vi "Lab Panel V4.4.vi"() -> ()   [LabVIEW 2013]
uses:
  <vilib>/Platform/TimedLoop/XDataNode/timing_clust.ctl
  <vilib>/Platform/TimedLoop/XDataNode/nitl_modes.ctl
  <vilib>/Platform/TimedLoop/XDataNode/wakeup.ctl
  Global 1.vi
  <vilib>/platform/TimedLoop/XDataNode/XDataNode.xnode
  <vilib>/Platform/TimedLoop/XDataNode/XDNodeRunTimeDep.lvlib
panel:
  in  "ADMIN PAGE":bool
  out "TEMP update":bool
  out "AI update":bool
  in  "Tab Control 2":T1(tab)
  out "SIG LAB05-2":T2 {"PF" format="%.2f"; "AMPS" format="%.1f"}
  out "SIG LAB05-1":T2 {"PF" format="%.2f"; "AMPS" format="%.1f"}
  out "SIG LAB04-2":T2 {"PF" format="%.2f"; "AMPS" format="%.1f"}
  out "SIG LAB04-1":T2 {"PF" format="%.2f"; "AMPS" format="%.1f"}
  out "SIG LAB03-2":T2 {"PF" format="%.2f"; "AMPS" format="%.1f"}
  out "SIG LAB03-1":T2 {"PF" format="%.2f"; "AMPS" format="%.1f"}
  out "SIG LAB02-2":T2 {"PF" format="%.2f"; "AMPS" format="%.1f"}
  in  "RUN LAB01-1":bool
  in  "O/I  LAB05-1":bool
  in  "O/I  LAB05-2":bool
  in  "O/I  LAB04-1":bool
  in  "O/I  LAB04-2":bool
  in  "O/I  LAB02-1":bool
  in  "O/I  LAB02-2":bool
  in  "O/I  LAB01-2":bool
  in  "O/I  LAB01-1":bool
  in  "O/I  LAB03-1":bool
  in  "RUN LAB05-2":bool
  in  "RUN LAB05-1":bool
  in  "RUN LAB04-2":bool
  in  "RUN LAB04-1":bool
  in  "RUN LAB03-2":bool
  in  "RUN LAB03-1":bool
  in  "RUN LAB02-2":bool
  in  "RUN LAB02-1":bool
  in  "RUN LAB01-2":bool
  in  "SELECT LAB05-2":T3(radio)
  in  "SELECT LAB05-1":T3(radio)
  in  "SELECT LAB04-2":T3(radio)
  in  "SELECT LAB04-1":T3(radio)
  in  "SELECT LAB03-2":T3(radio)
  in  "SELECT LAB03-1":T3(radio)
  in  "SELECT LAB02-2":T3(radio)
  in  "SELECT LAB02-1":T3(radio)
  in  "SELECT LAB01-2":T3(radio)
  in  "SELECT LAB01-1":T3(radio)
  in  "O/I  LAB03-2":bool
  out "SIG LAB01-1":T2 {"PF" format="%.2f"; "AMPS" format="%.1f"}
  out "SIG LAB01-2":T2 {"PF" format="%.2f"; "AMPS" format="%.1f"}
  out "SIG LAB02-1":T2 {"PF" format="%.2f"; "AMPS" format="%.1f"}
  out "DISP LAB05-2":T4 {"MINS" format="%.2g"}
  out "DISP LAB05-1":T4 {"MINS" format="%.2g"}
  out "DISP LAB04-2":T4 {"MINS" format="%.2g"}
  out "DISP LAB04-1":T4 {"MINS" format="%.2g"}
  out "DISP LAB03-2":T4 {"MINS" format="%.2g"}
  out "DISP LAB03-1":T4 {"MINS" format="%.2g"}
  in  "SET LAB05-2":T5={"NAME"="", "DESCRIPTION"="", "CYCLES"=5.0, "T-RISE mins"=0.0, "T-RISE deg C"=0.0} {"CYCLES" min=5.0 step=1.0}
  in  "SET LAB05-1":T5={"NAME"="", "DESCRIPTION"="", "CYCLES"=5.0, "T-RISE mins"=0.0, "T-RISE deg C"=0.0} {"CYCLES" min=5.0 step=1.0}
  in  "SET LAB04-2":T5={"NAME"="", "DESCRIPTION"="", "CYCLES"=5.0, "T-RISE mins"=0.0, "T-RISE deg C"=0.0} {"CYCLES" min=5.0 step=1.0}
  in  "SET LAB04-1":T5={"NAME"="", "DESCRIPTION"="", "CYCLES"=5.0, "T-RISE mins"=0.0, "T-RISE deg C"=0.0} {"CYCLES" min=5.0 step=1.0}
  in  "SET LAB03-2":T5={"NAME"="", "DESCRIPTION"="", "CYCLES"=5.0, "T-RISE mins"=0.0, "T-RISE deg C"=0.0} {"CYCLES" min=5.0 step=1.0}
  in  "SET LAB03-1":T5={"NAME"="", "DESCRIPTION"="", "CYCLES"=5.0, "T-RISE mins"=0.0, "T-RISE deg C"=0.0} {"CYCLES" min=5.0 step=1.0}
  out "DISP LAB02-2":T4 {"MINS" format="%.2g"}
  out "DISP LAB02-1":T4 {"MINS" format="%.2g"}
  in  "SET LAB02-2":T5={"NAME"="", "DESCRIPTION"="", "CYCLES"=5.0, "T-RISE mins"=0.0, "T-RISE deg C"=0.0} {"CYCLES" min=5.0 step=1.0}
  in  "SET LAB02-1":T5={"NAME"="", "DESCRIPTION"="", "CYCLES"=5.0, "T-RISE mins"=0.0, "T-RISE deg C"=0.0} {"CYCLES" min=5.0 step=1.0}
  out "RESULT LAB05-2":bool
  out "RESULT LAB05-1":bool
  out "RESULT LAB04-2":bool
  out "RESULT LAB04-1":bool
  out "RESULT LAB03-2":bool
  out "RESULT LAB03-1":bool
  out "RESULT LAB02-2":bool
  out "RESULT LAB02-1":bool
  out "RESULT LAB01-2":bool
  out "RESULT LAB01-1":bool
  in  "SET LAB01-1":T5={"NAME"="", "DESCRIPTION"="", "CYCLES"=5.0, "T-RISE mins"=0.0, "T-RISE deg C"=0.0} {"CYCLES" min=5.0 step=1.0}
  in  "SET LAB01-2":T5={"NAME"="", "DESCRIPTION"="", "CYCLES"=5.0, "T-RISE mins"=0.0, "T-RISE deg C"=0.0} {"CYCLES" min=5.0 step=1.0}
  out "DISP LAB01-1":T4 {"MINS" format="%.2g"}
  out "DISP LAB01-2":T4 {"MINS" format="%.2f"}
  out "TEMP RISE LAB05-2":cluster{"TL":dbl, "TN":dbl}
  out "TEMP RISE LAB05-1":cluster{"TL":dbl, "TN":dbl}
  out "TEMP RISE LAB04-2":cluster{"TL":dbl, "TN":dbl}
  out "TEMP RISE LAB04-1":cluster{"TL":dbl, "TN":dbl}
  out "TEMP RISE LAB03-2":cluster{"TL":dbl, "TN":dbl}
  out "TEMP RISE LAB03-1":cluster{"TL":dbl, "TN":dbl}
  out "TEMP RISE LAB02-2":cluster{"TL":dbl, "TN":dbl}
  out "TEMP RISE LAB02-1":cluster{"TL":dbl, "TN":dbl}
  out "TEMP RISE LAB01-2":cluster{"TL":dbl, "TN":dbl}
  out "TEMP RISE LAB01-1":cluster{"TL":dbl, "TN":dbl}
  in  "JIG OFF TIME (S)":dbl=2.0 min=2.0 max=10.0 step=0.5 format="%.1g"
  in  "JIG ON TIME (S)":dbl=1.0 min=1.0 max=10.0 step=0.5 format="%.1g"
  out "JIG LAB05-2":bool
  out "JIG LAB05-1":bool
  out "JIG LAB04-2":bool
  out "JIG LAB04-1":bool
  out "JIG LAB03-2":bool
  out "JIG LAB03-1":bool
  out "JIG LAB02-2":bool
  out "JIG LAB02-1":bool
  out "JIG LAB01-2":bool
  out "JIG LAB01-1":bool
  out "TEMP START LAB01-1":cluster{"TL":dbl, "TN":dbl}
  out "TEMP START LAB02-1":cluster{"TL":dbl, "TN":dbl}
  out "TEMP START LAB03-1":cluster{"TL":dbl, "TN":dbl}
  out "TEMP START LAB04-1":cluster{"TL":dbl, "TN":dbl}
  out "TEMP START LAB01-2":cluster{"TL":dbl, "TN":dbl}
  out "TEMP START LAB02-2":cluster{"TL":dbl, "TN":dbl}
  out "TEMP START LAB03-2":cluster{"TL":dbl, "TN":dbl}
  out "TEMP START LAB04-2":cluster{"TL":dbl, "TN":dbl}
  out "TEMP START LAB05-2":cluster{"TL":dbl, "TN":dbl}
  out "TEMP START LAB05-1":cluster{"TL":dbl, "TN":dbl}
  in  "MAIL SETTINGS":T6
  out "MAIL REPORT":string
  in  "TO (string):":string
  in  "Send Mail Now":bool
  in  "Auto Mail Send":bool
  in  "Network Directory":path
  out "CAL LAB01":T7 {"2 (TN) cal" min=0.0 step=0.01 format="%.2f"; "2 (TL) cal" min=0.0 step=0.01 format="%.2f"; "2 (PF) cal" min=0.0 step=0.01 format="%.2f"; "2 (V) cal" min=0.0 step=0.01 format="%.2f"; "2 (A) cal" min=0.0 step=0.01 format="%.2f"; "1 (TN) cal" min=0.0 step=0.01 format="%.2f"; "1 (TL) cal" min=0.0 step=0.01 format="%.2f"; "1 (PF) cal" min=0.0 step=0.01 format="%.2f"; "1 (V) cal" min=0.0 step=0.01 format="%.2f"; "1  (A) cal" min=0.0 step=0.01 format="%.2f"}
  out "CAL LAB03":T7 {"2 (TN) cal" min=0.0 step=0.01 format="%.2f"; "2 (TL) cal" min=0.0 step=0.01 format="%.2f"; "2 (PF) cal" min=0.0 step=0.01 format="%.2f"; "2 (V) cal" min=0.0 step=0.01 format="%.2f"; "2 (A) cal" min=0.0 step=0.01 format="%.2f"; "1 (TN) cal" min=0.0 step=0.01 format="%.2f"; "1 (TL) cal" min=0.0 step=0.01 format="%.2f"; "1 (PF) cal" min=0.0 step=0.01 format="%.2f"; "1 (V) cal" min=0.0 step=0.01 format="%.2f"; "1  (A) cal" min=0.0 step=0.01 format="%.2f"}
  out "CAL LAB02":T8 {"2 (TN) cal" min=0.0 step=0.01 format="%.2f"; "2 (TL) cal" min=0.0 step=0.01 format="%.2f"; "2 (PF) cal" min=0.0 step=0.01 format="%.2f"; "2 (V) cal" min=0.0 step=0.01 format="%.2f"; "2 (A) cal" min=0.0 step=0.01 format="%.2f"; "1 (TN) cal" min=0.0 step=0.01 format="%.2f"; "1 (TL) cal" min=0.0 step=0.01 format="%.2f"; "1 (PF) cal" min=0.0 step=0.01 format="%.2f"; "1 (V) cal" min=0.0 step=0.01 format="%.2f"; "1 (A) cal" min=0.0 step=0.01 format="%.2f"}
  out "CAL LAB05":T7 {"2 (TN) cal" min=0.0 step=0.01 format="%.2f"; "2 (TL) cal" min=0.0 step=0.01 format="%.2f"; "2 (PF) cal" min=0.0 step=0.01 format="%.2f"; "2 (V) cal" min=0.0 step=0.01 format="%.2f"; "2 (A) cal" min=0.0 step=0.01 format="%.2f"; "1 (TN) cal" min=0.0 step=0.01 format="%.2f"; "1 (TL) cal" min=0.0 step=0.01 format="%.2f"; "1 (PF) cal" min=0.0 step=0.01 format="%.2f"; "1 (V) cal" min=0.0 step=0.01 format="%.2f"; "1  (A) cal" min=0.0 step=0.01 format="%.2f"}
  out "CAL LAB04":T7 {"2 (TN) cal" min=0.0 step=0.01 format="%.2f"; "2 (TL) cal" min=0.0 step=0.01 format="%.2f"; "2 (PF) cal" min=0.0 step=0.01 format="%.2f"; "2 (V) cal" min=0.0 step=0.01 format="%.2f"; "2 (A) cal" min=0.0 step=0.01 format="%.2f"; "1 (TN) cal" min=0.0 step=0.01 format="%.2f"; "1 (TL) cal" min=0.0 step=0.01 format="%.2f"; "1 (PF) cal" min=0.0 step=0.01 format="%.2f"; "1 (V) cal" min=0.0 step=0.01 format="%.2f"; "1  (A) cal" min=0.0 step=0.01 format="%.2f"}
  out "calibration file error out":errorcluster
  in  "CALIBRATE":bool
  out "ON L05-2":cluster{"amps":dbl, "volts":dbl, "pf":dbl}
  out "ON L05-1":cluster{"amps":dbl, "volts":dbl, "pf":dbl}
  out "FAIL LAB05-2":cluster{"LO":dbl, "HI":dbl}
  out "FAIL LAB05-1":cluster{"LO":dbl, "HI":dbl}
  out "FAIL LAB04-2":cluster{"LO":dbl, "HI":dbl}
  out "FAIL LAB04-1":cluster{"LO":dbl, "HI":dbl}
  out "FAIL LAB03-2":cluster{"LO":dbl, "HI":dbl}
  out "FAIL LAB03-1":cluster{"LO":dbl, "HI":dbl}
  out "FAIL LAB02-2":cluster{"LO":dbl, "HI":dbl}
  out "FAIL LAB02-1":cluster{"LO":dbl, "HI":dbl}
  out "FAIL LAB01-2":cluster{"LO":dbl, "HI":dbl}
  out "FAIL LAB01-1":cluster{"LO":dbl, "HI":dbl}
  out "ON L01-1":cluster{"amps":dbl, "volts":dbl, "pf":dbl}
  out "ON L01-2":cluster{"amps":dbl, "volts":dbl, "pf":dbl}
  out "ON L02-1":cluster{"amps":dbl, "volts":dbl, "pf":dbl}
  out "ON L02-2":cluster{"amps":dbl, "volts":dbl, "pf":dbl}
  out "ON L03-1":cluster{"amps":dbl, "volts":dbl, "pf":dbl}
  out "ON L03-2":cluster{"amps":dbl, "volts":dbl, "pf":dbl}
  out "ON L04-1":cluster{"amps":dbl, "volts":dbl, "pf":dbl}
  out "ON L04-2":cluster{"amps":dbl, "volts":dbl, "pf":dbl}
  out "TEST VOLTS CHART":T9(graph)
  in  "Select  Cycle":enum32{"ON CYCLE", "OFF CYCLE"}(radio)
  out "TEST AMPS CHART":T9(graph)
  in  "JIG TEST":T10
  in  "C drive data root dir":path
  out "run lab05-2":bool
  out "run lab05-1":bool
  out "run lab04-2":bool
  out "run lab04-1":bool
  out "run lab03-2":bool
  out "run lab03-1":bool
  out "run lab02-2":bool
  out "run lab02-1":bool
  out "run lab01-2":bool
  out "run lab01-1":bool
  out "stop2":bool
  in  "Tab Control":T11(tab)
  out "LAB01-2 (GRAPH)":dynamicdata(graph)
  out "LAB01-1 (GRAPH)":dynamicdata(graph)
  out "LAB02-2 (GRAPH)":dynamicdata(graph)
  out "LAB02-1 (GRAPH)":dynamicdata(graph)
  out "LAB03-2 (GRAPH)":dynamicdata(graph)
  out "LAB03-1 (GRAPH)":dynamicdata(graph)
  out "LAB04-2 (GRAPH)":dynamicdata(graph)
  out "LAB04-1 (GRAPH)":dynamicdata(graph)
  out "LAB05-2 (GRAPH)":dynamicdata(graph)
  out "LAB05-1 (GRAPH)":dynamicdata(graph)
  out "LAB05 TEMP":T12
  out "LAB04 TEMP":T12
  out "LAB02 TEMP":T12
  out "LAB01 TEMP":T12
  out "LAB03 TEMP":T12
  out "Analog Error Array":errorcluster[](array[cluster])
  out "AI loop time":dbl format="%.6g"
  out "loops":dbl
  in  "loop  delay(mS)":dbl
  out "on loops":dbl
  out "off loops":dbl
  out "jig cycle":dbl
  out "TDMS LAB01-1":refnum<k34>
  out "data file error":errorcluster
  out "TDMS LAB02-1":refnum<k34>
  out "TDMS LAB01-2":refnum<k34>
  out "TDMS LAB02-2":refnum<k34>
  out "TDMS LAB03-1":refnum<k34>
  out "TDMS LAB03-2":refnum<k34>
  out "TDMS LAB04-1":refnum<k34>
  out "TDMS LAB04-2":refnum<k34>
  out "TDMS LAB05-1":refnum<k34>
  out "TDMS LAB05-2":refnum<k34>
  out "mail control":string
  out "File Time Stamp":timestamp
  in  "stop":bool
  # "LAB01"
  # "LAB02"
  # "LAB05"
  # "LAB03"
  # "LAB04"
  # "LAB01"
  # "LAB02"
  # "LAB03"
  # "LAB04"
  # "LAB05"
  # "JIG SET"
  # "(Enter recipients address seperated by comma)"
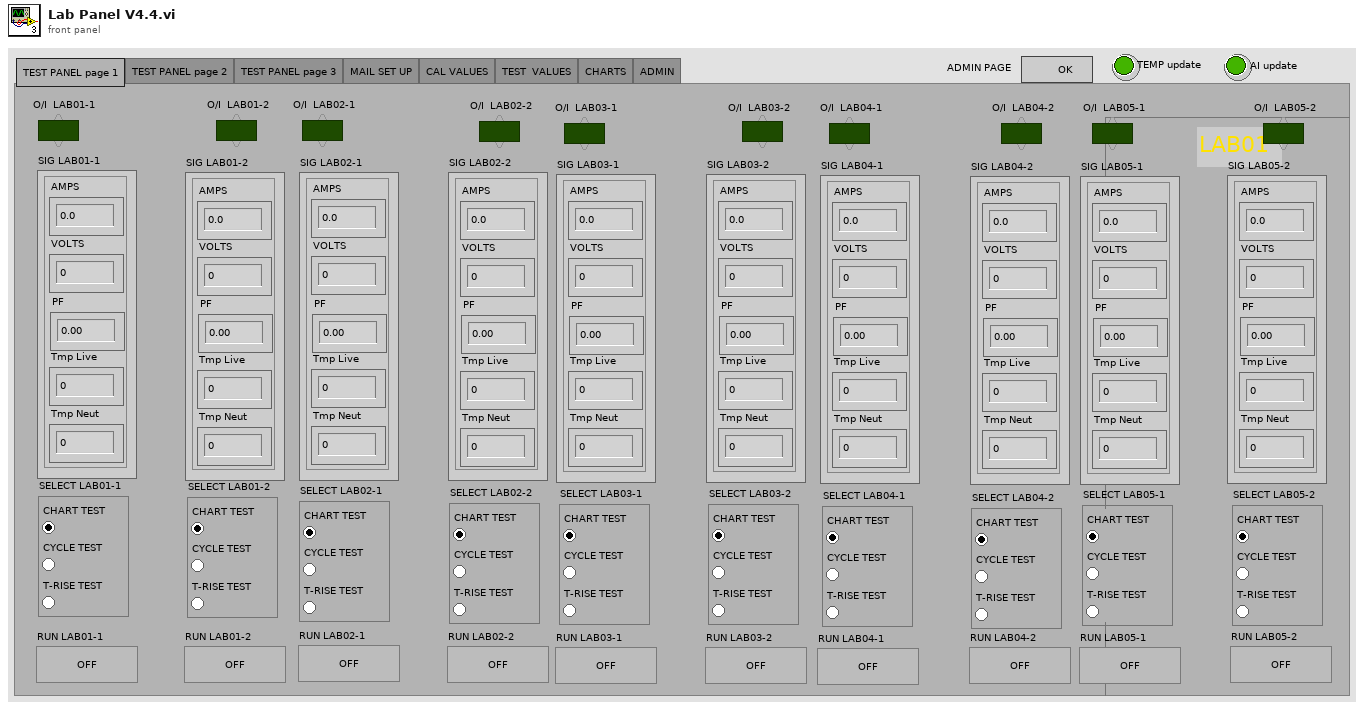
[diagram p1: front panel]
types:
  T1 = enum32{"TEST PANEL page 1", "TEST PANEL page 2", "TEST PANEL page 3", "MAIL SET UP", "CAL VALUES", "TEST  VALUES", "CHARTS", "ADMIN"}
  T2 = cluster{"AMPS":dbl, "VOLTS":dbl, "PF":dbl, "Tmp Live":dbl, "Tmp Neut":dbl}
  T3 = enum32{"CHART TEST", "CYCLE TEST", "T-RISE TEST"}
  T4 = cluster{"CYCLE":dbl, "MINS":dbl, "STATUS":string}
  T5 = cluster{"NAME":string, "DESCRIPTION":string, "CYCLES":dbl, "T-RISE mins":dbl, "T-RISE deg C":dbl}
  T6 = cluster{"OUT SERVER ADDRESS":string, "FROM ACCOUNT":string, "USER NAME":string, "PASSWORD":string, "TEST MAIL":bool, "TEST MAIL STATUS":string, "mail error":errorcluster}
  T7 = cluster{"1  (A) cal":dbl, "1 (V) cal":dbl, "1 (PF) cal":dbl, "1 (TL) cal":dbl, "1 (TN) cal":dbl, "2 (A) cal":dbl, "2 (V) cal":dbl, "2 (PF) cal":dbl, "2 (TL) cal":dbl, "2 (TN) cal":dbl}
  T8 = cluster{"1 (A) cal":dbl, "1 (V) cal":dbl, "1 (PF) cal":dbl, "1 (TL) cal":dbl, "1 (TN) cal":dbl, "2 (A) cal":dbl, "2 (V) cal":dbl, "2 (PF) cal":dbl, "2 (TL) cal":dbl, "2 (TN) cal":dbl}
  T9 = cluster{"AMPS":dbl, "AMPS":dbl, "AMPS":dbl, "AMPS":dbl, "AMPS":dbl, "AMPS":dbl, "AMPS":dbl, "AMPS":dbl, "AMPS":dbl, "AMPS":dbl}
  T10 = cluster{" LAB01-1":bool, " LAB01-2":bool, "LAB02-1":bool, " LAB02-2":bool, "LAB03-1":bool, "LAB03-2":bool, "LAB04-1":bool, "LAB04-2":bool, "LAB05-1":bool, "LAB05-2":bool}
  T11 = enum32{"LAB01", "LAB02", "LAB03", "LAB04", "LAB05", "TEMPERATURE", "ERROR"}
  T12 = cluster{"T1 Live":dbl, "T1 Neut":dbl, "T2 Live":dbl, "T2 Neut":dbl, "ID":dbl, "ER":dbl}
  T13 = enum8{"Enabled", "Disabled", "Disabled and Grayed Out"}
  T14 = typedef "XDNodeRunTimeDep.lvlib/timing_clust.ctl" = cluster{"Expected End [f-1]":u64, "Actual End [f-1]":u64, "Finished Late? [f-1]":bool, "Expected End [i-1]":u64, "Actual End [i-1]":u64, "Finished Late? [i-1]":bool, "Expected Start [i]":u64, "Actual Start [i]":u64, "Expected Start [f]":u64, "Actual Start [f]":u64, "Source Name":string, "Structure Name":string, "Period":i64, "Deadline":i64, "Offset":i64, "Start":i64, "Priority":i32, "Timeout":i32, "Mode":T15, "Wakeup Reason":T16, "Error":errorcluster, "Source Type":string, "Secondary Source Type":string, "Global End Time":u64, "Global Start Time":u64, "Frame Duration":u64, "Iteration Duration":u64, "Assigned CPU":i32, "I/O Scan Engine Mode":u32}
  T15 = typedef "XDNodeRunTimeDep.lvlib/nitl_modes.ctl" = enum32{"No Change", "Process missed periods, maintain original phase", "Discard missed periods, maintain original phase", "Process missed periods, ignore original phase", "Discard missed periods, ignore original phase"}
  T16 = typedef "XDNodeRunTimeDep.lvlib/wakeup.ctl" = enum32{"Normal", "Aborted", "Asynchronous wakeup", "Timing source error", "Timed loop error", "Timeout"}
  T17 = enum16{"open", "open or create", "create or replace", "create", "open (read-only)"}
  T18 = enum16{"open", "replace", "create", "open or create", "replace or create", "replace or create with confirmation"}
  T19 = cluster{"SET LAB01-1":cluster{"NAME":string, "DESCRIPTION":string, "CYCLES":dbl, "T-RISE mins":dbl, "T-RISE deg C":dbl}, "SET LAB01-2":cluster{"NAME":string, "DESCRIPTION":string, "CYCLES":dbl, "T-RISE mins":dbl, "T-RISE deg C":dbl}, "SET LAB02-1":cluster{"NAME":string, "DESCRIPTION":string, "CYCLES":dbl, "T-RISE mins":dbl, "T-RISE deg C":dbl}, "SET LAB02-2":cluster{"NAME":string, "DESCRIPTION":string, "CYCLES":dbl, "T-RISE mins":dbl, "T-RISE deg C":dbl}, "SET LAB03-1":cluster{"NAME":string, "DESCRIPTION":string, "CYCLES":dbl, "T-RISE mins":dbl, "T-RISE deg C":dbl}, "SET LAB03-2":cluster{"NAME":string, "DESCRIPTION":string, "CYCLES":dbl, "T-RISE mins":dbl, "T-RISE deg C":dbl}, "SET LAB04-1":cluster{"NAME":string, "DESCRIPTION":string, "CYCLES":dbl, "T-RISE mins":dbl, "T-RISE deg C":dbl}, "SET LAB04-2":cluster{"NAME":string, "DESCRIPTION":string, "CYCLES":dbl, "T-RISE mins":dbl, "T-RISE deg C":dbl}, "SET LAB05-1":cluster{"NAME":string, "DESCRIPTION":string, "CYCLES":dbl, "T-RISE mins":dbl, "T-RISE deg C":dbl}, "SET LAB05-2":cluster{"NAME":string, "DESCRIPTION":string, "CYCLES":dbl, "T-RISE mins":dbl, "T-RISE deg C":dbl}, "Network Directory":path, "C drive data root dir":path}
  T20 = cluster{"MAIL SETTINGS":cluster{"OUT SERVER ADDRESS":string, "FROM ACCOUNT":string, "USER NAME":string, "PASSWORD":string, "TEST MAIL":bool, "TEST MAIL STATUS":string, "mail error":errorcluster}, "Auto Mail Send":bool, string}
  T21 = cluster{"T1":dbl, "T2":dbl, "T3":dbl, "T4":dbl, "ID":dbl, "ER":dbl}
  T22 = cluster{"LAB01-1 (A)":dbl, "LAB01-1 (V)":dbl, "LAB01-1 (PF)":dbl, "LAB01-2 (A)":dbl, "LAB01-2 (V)":dbl, "LAB01-2 (PF)":dbl}
  T23 = cluster{"LAB02-1 (A)":dbl, "LAB02-1 (V)":dbl, "LAB02-1 (PF)":dbl, "LAB02-2 (A)":dbl, "LAB02-2 (V)":dbl, "LAB02-2 (PF)":dbl}
  T24 = cluster{"LAB03-1 (A)":dbl, "LAB03-1 (V)":dbl, "LAB03-1 (PF)":dbl, "LAB03-2 (A)":dbl, "LAB03-2 (V)":dbl, "LAB03-2 (PF)":dbl}
  T25 = cluster{"LAB04-1 (A)":dbl, "LAB04-1 (V)":dbl, "LAB04-1 (PF)":dbl, "LAB04-2 (A)":dbl, "LAB04-2 (V)":dbl, "LAB04-2 (PF)":dbl}
  T26 = cluster{"LAB05-1 (A)":dbl, "LAB05-1 (V)":dbl, "LAB05-1 (PF)":dbl, "LAB05-2 (A)":dbl, "LAB05-2 (V)":dbl, "LAB05-2 (PF)":dbl}
  T27 = cluster{"VOLTS":dbl, "VOLTS":dbl, "VOLTS":dbl, "VOLTS":dbl, "VOLTS":dbl, "VOLTS":dbl, "VOLTS":dbl, "VOLTS":dbl, "VOLTS":dbl, "VOLTS":dbl}
  T28 = cluster{"FAIL LAB01-1":cluster{"LO":dbl, "HI":dbl}, "SIG LAB01-1":cluster{"AMPS":dbl, "VOLTS":dbl, "PF":dbl, "Tmp Live":dbl, "Tmp Neut":dbl}, "TEMP START LAB01-1":cluster{"TL":dbl, "TN":dbl}, "DISP LAB01-1":cluster{"CYCLE":dbl, "MINS":dbl, "STATUS":string}, "SET LAB01-1":cluster{"NAME":string, "DESCRIPTION":string, "CYCLES":dbl, "T-RISE mins":dbl, "T-RISE deg C":dbl}, "TDMS LAB01-1":refnum<k34>}
  T29 = cluster{"FAIL LAB01-2":cluster{"LO":dbl, "HI":dbl}, "SIG LAB01-2":cluster{"AMPS":dbl, "VOLTS":dbl, "PF":dbl, "Tmp Live":dbl, "Tmp Neut":dbl}, "TEMP START LAB01-2":cluster{"TL":dbl, "TN":dbl}, "DISP LAB01-2":cluster{"CYCLE":dbl, "MINS":dbl, "STATUS":string}, "SET LAB01-2":cluster{"NAME":string, "DESCRIPTION":string, "CYCLES":dbl, "T-RISE mins":dbl, "T-RISE deg C":dbl}, "TDMS LAB01-2":refnum<k34>}
  T30 = cluster{"FAIL LAB02-1":cluster{"LO":dbl, "HI":dbl}, "SIG LAB02-1":cluster{"AMPS":dbl, "VOLTS":dbl, "PF":dbl, "Tmp Live":dbl, "Tmp Neut":dbl}, "TEMP START LAB02-1":cluster{"TL":dbl, "TN":dbl}, "DISP LAB02-1":cluster{"CYCLE":dbl, "MINS":dbl, "STATUS":string}, "SET LAB02-1":cluster{"NAME":string, "DESCRIPTION":string, "CYCLES":dbl, "T-RISE mins":dbl, "T-RISE deg C":dbl}, "TDMS LAB02-1":refnum<k34>}
  T31 = cluster{"FAIL LAB02-2":cluster{"LO":dbl, "HI":dbl}, "SIG LAB02-2":cluster{"AMPS":dbl, "VOLTS":dbl, "PF":dbl, "Tmp Live":dbl, "Tmp Neut":dbl}, "TEMP START LAB02-2":cluster{"TL":dbl, "TN":dbl}, "DISP LAB02-2":cluster{"CYCLE":dbl, "MINS":dbl, "STATUS":string}, "SET LAB02-2":cluster{"NAME":string, "DESCRIPTION":string, "CYCLES":dbl, "T-RISE mins":dbl, "T-RISE deg C":dbl}, "TDMS LAB02-2":refnum<k34>}
  T32 = cluster{"FAIL LAB03-1":cluster{"LO":dbl, "HI":dbl}, "SIG LAB03-1":cluster{"AMPS":dbl, "VOLTS":dbl, "PF":dbl, "Tmp Live":dbl, "Tmp Neut":dbl}, "TEMP START LAB03-1":cluster{"TL":dbl, "TN":dbl}, "DISP LAB03-1":cluster{"CYCLE":dbl, "MINS":dbl, "STATUS":string}, "SET LAB03-1":cluster{"NAME":string, "DESCRIPTION":string, "CYCLES":dbl, "T-RISE mins":dbl, "T-RISE deg C":dbl}, "TDMS LAB03-1":refnum<k34>}
  T33 = cluster{"FAIL LAB03-2":cluster{"LO":dbl, "HI":dbl}, "SIG LAB03-2":cluster{"AMPS":dbl, "VOLTS":dbl, "PF":dbl, "Tmp Live":dbl, "Tmp Neut":dbl}, "TEMP START LAB03-2":cluster{"TL":dbl, "TN":dbl}, "DISP LAB03-2":cluster{"CYCLE":dbl, "MINS":dbl, "STATUS":string}, "SET LAB03-2":cluster{"NAME":string, "DESCRIPTION":string, "CYCLES":dbl, "T-RISE mins":dbl, "T-RISE deg C":dbl}, "TDMS LAB03-2":refnum<k34>}
  T34 = cluster{"FAIL LAB04-1":cluster{"LO":dbl, "HI":dbl}, "SIG LAB04-1":cluster{"AMPS":dbl, "VOLTS":dbl, "PF":dbl, "Tmp Live":dbl, "Tmp Neut":dbl}, "TEMP START LAB04-1":cluster{"TL":dbl, "TN":dbl}, "DISP LAB04-1":cluster{"CYCLE":dbl, "MINS":dbl, "STATUS":string}, "SET LAB04-1":cluster{"NAME":string, "DESCRIPTION":string, "CYCLES":dbl, "T-RISE mins":dbl, "T-RISE deg C":dbl}, "TDMS LAB04-1":refnum<k34>}
  T35 = cluster{"FAIL LAB04-2":cluster{"LO":dbl, "HI":dbl}, "SIG LAB04-2":cluster{"AMPS":dbl, "VOLTS":dbl, "PF":dbl, "Tmp Live":dbl, "Tmp Neut":dbl}, "TEMP START LAB04-2":cluster{"TL":dbl, "TN":dbl}, "DISP LAB04-2":cluster{"CYCLE":dbl, "MINS":dbl, "STATUS":string}, "SET LAB04-2":cluster{"NAME":string, "DESCRIPTION":string, "CYCLES":dbl, "T-RISE mins":dbl, "T-RISE deg C":dbl}, "TDMS LAB04-2":refnum<k34>}
  T36 = cluster{"FAIL LAB05-1":cluster{"LO":dbl, "HI":dbl}, "SIG LAB05-1":cluster{"AMPS":dbl, "VOLTS":dbl, "PF":dbl, "Tmp Live":dbl, "Tmp Neut":dbl}, "TEMP START LAB05-1":cluster{"TL":dbl, "TN":dbl}, "DISP LAB05-1":cluster{"CYCLE":dbl, "MINS":dbl, "STATUS":string}, "SET LAB05-1":cluster{"NAME":string, "DESCRIPTION":string, "CYCLES":dbl, "T-RISE mins":dbl, "T-RISE deg C":dbl}, "TDMS LAB05-1":refnum<k34>}
  T37 = cluster{"FAIL LAB05-2":cluster{"LO":dbl, "HI":dbl}, "SIG LAB05-2":cluster{"AMPS":dbl, "VOLTS":dbl, "PF":dbl, "Tmp Live":dbl, "Tmp Neut":dbl}, "TEMP START LAB05-2":cluster{"TL":dbl, "TN":dbl}, "DISP LAB05-2":cluster{"CYCLE":dbl, "MINS":dbl, "STATUS":string}, "SET LAB05-2":cluster{"NAME":string, "DESCRIPTION":string, "CYCLES":dbl, "T-RISE mins":dbl, "T-RISE deg C":dbl}, "TDMS LAB05-2":refnum<k34>}
  T38 = cluster{"MAIL SETTINGS":cluster{"OUT SERVER ADDRESS":string, "FROM ACCOUNT":string, "USER NAME":string, "PASSWORD":string, "TEST MAIL":bool, "TEST MAIL STATUS":string, "mail error":errorcluster}, "Auto Mail Send":bool, "TO (string):":string}
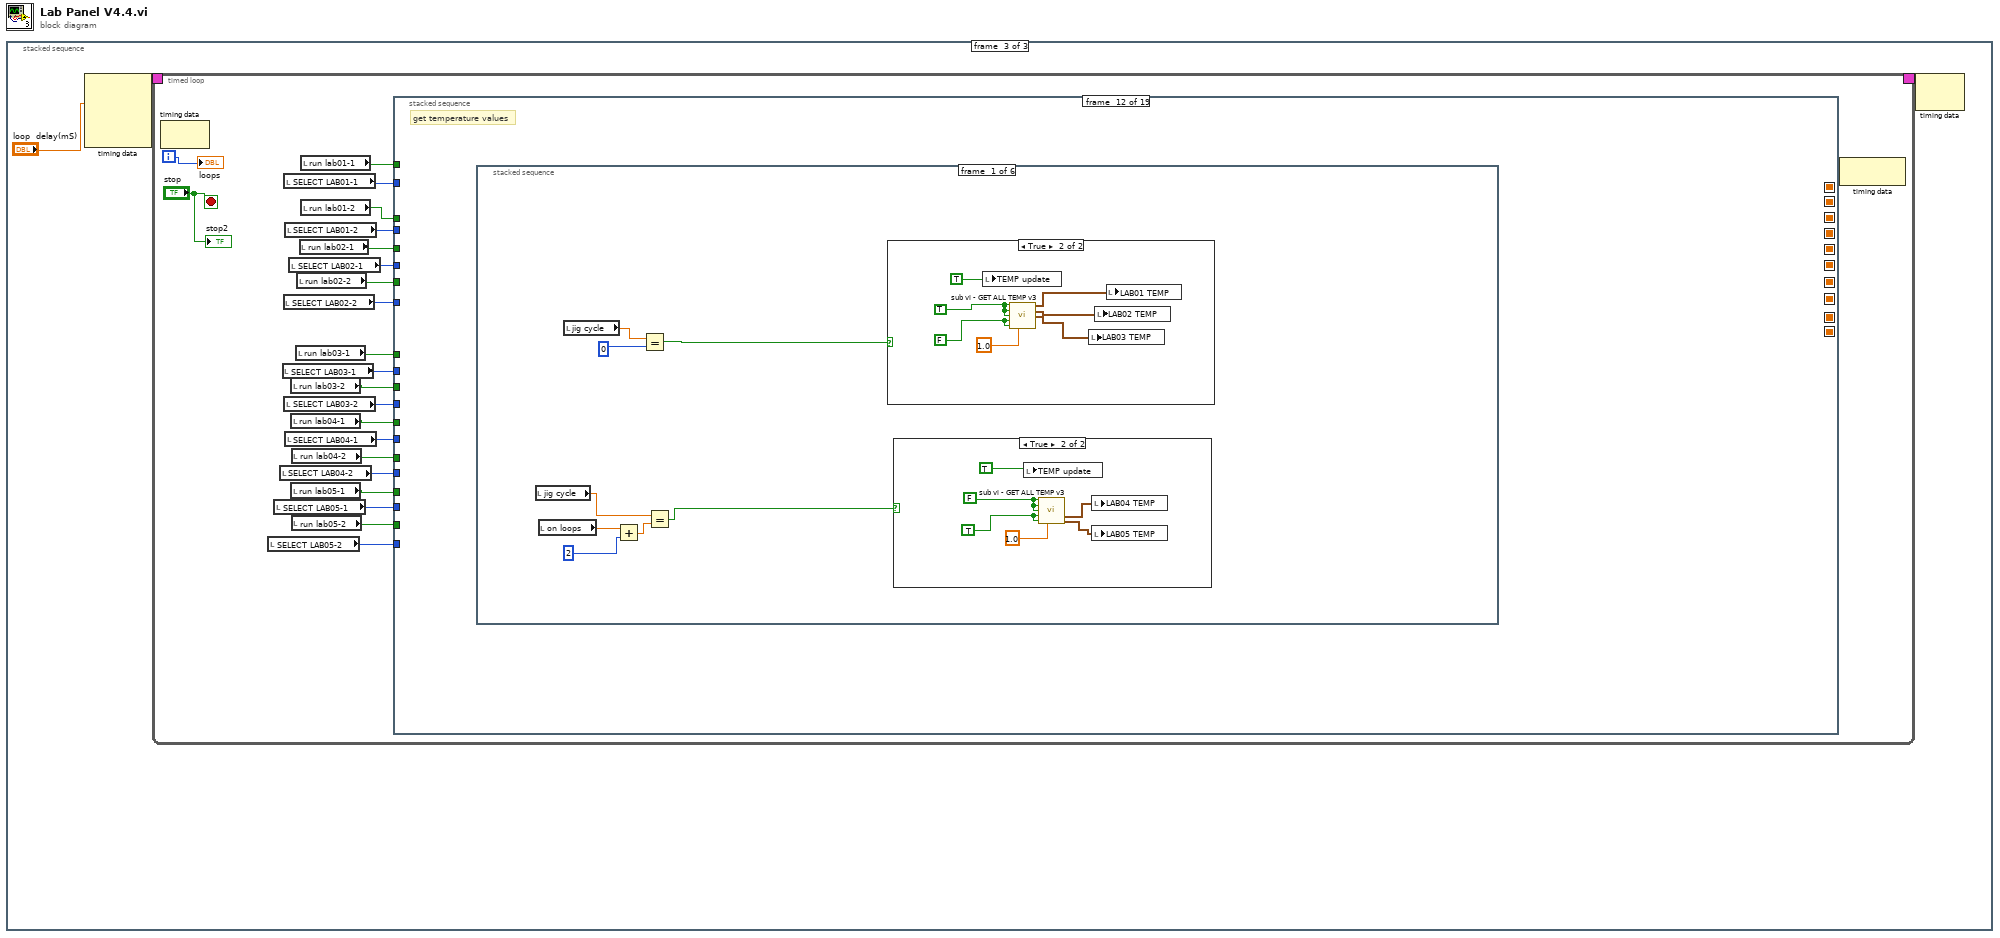
[diagram p0: block diagram]
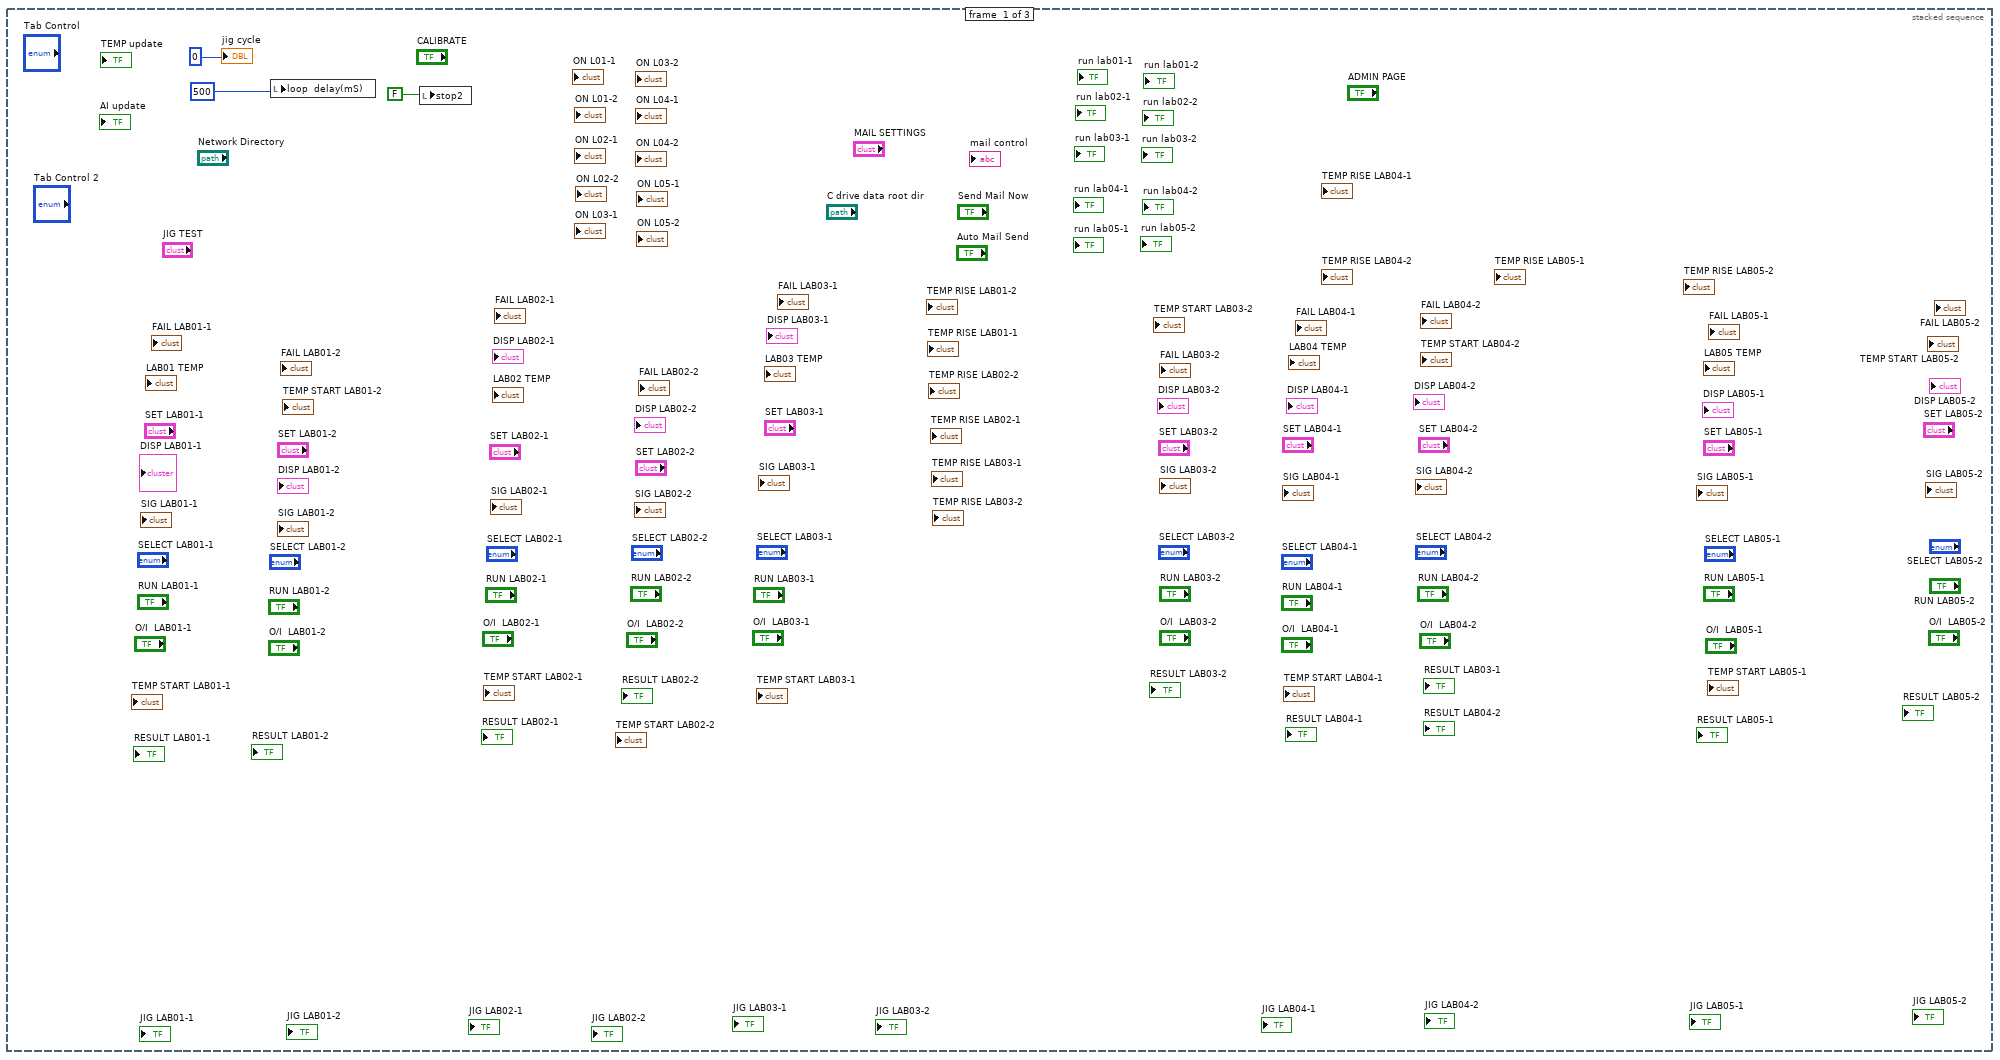
[diagram p2: hidden frame]
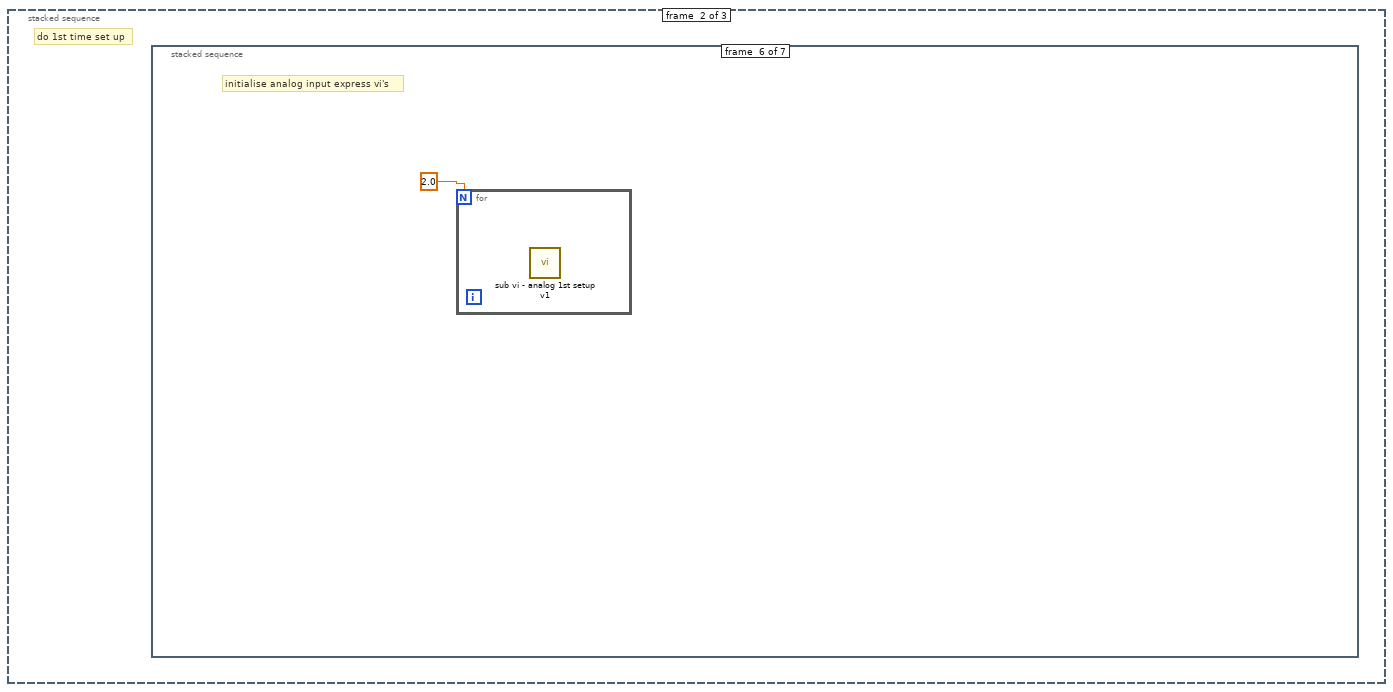
[diagram p3: hidden frame]
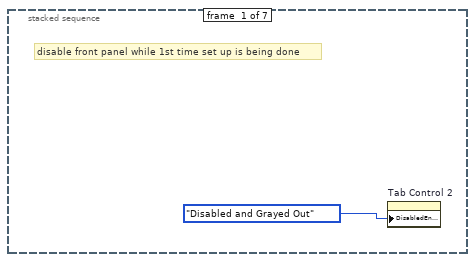
[diagram p4: hidden frame]
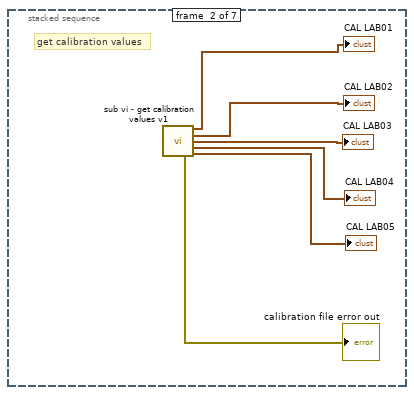
[diagram p5: hidden frame]
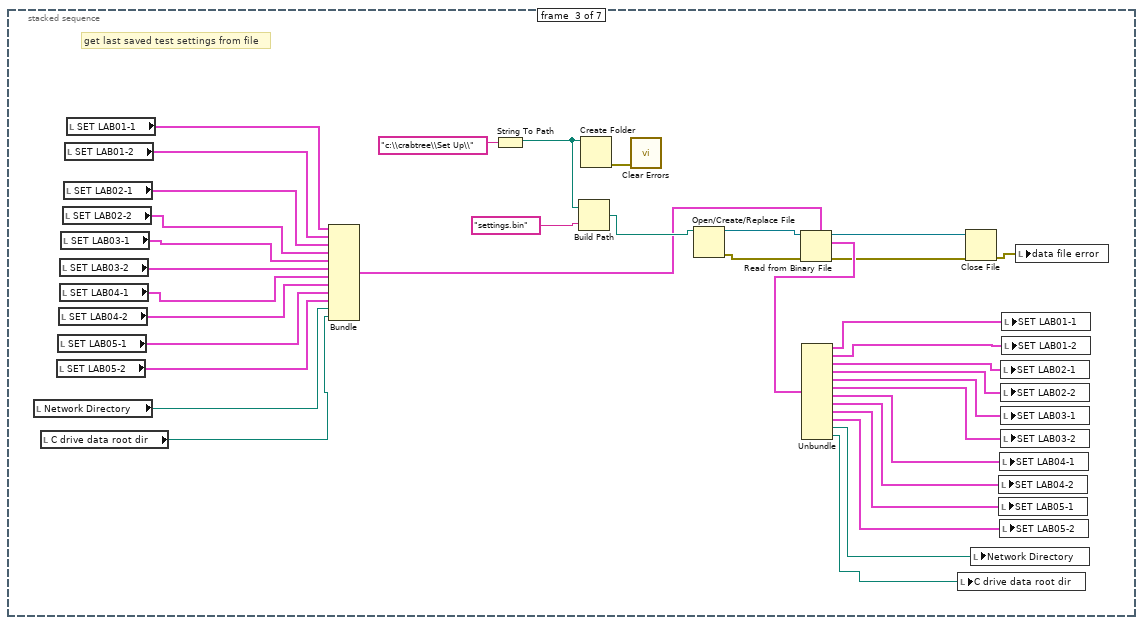
[diagram p6: hidden frame]
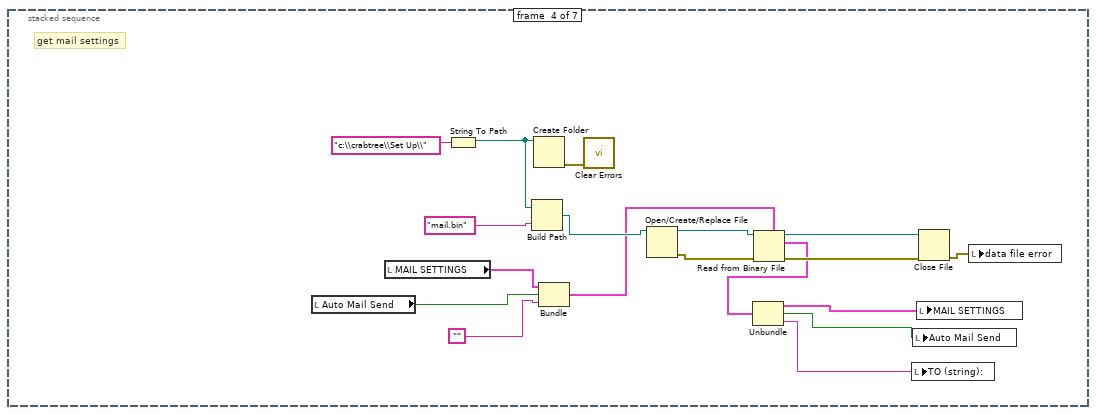
[diagram p7: hidden frame]
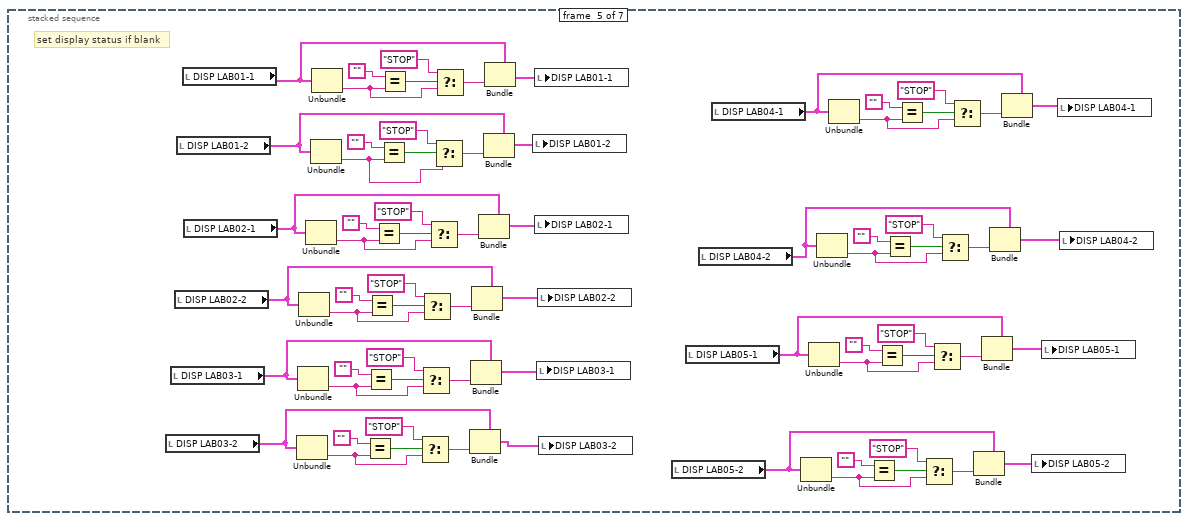
[diagram p8: hidden frame]
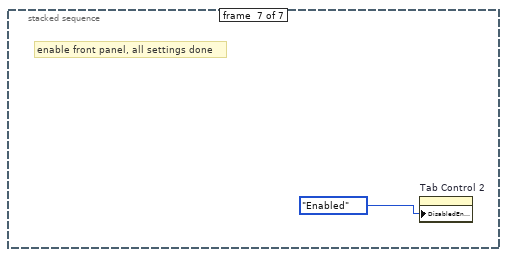
[diagram p9: hidden frame]
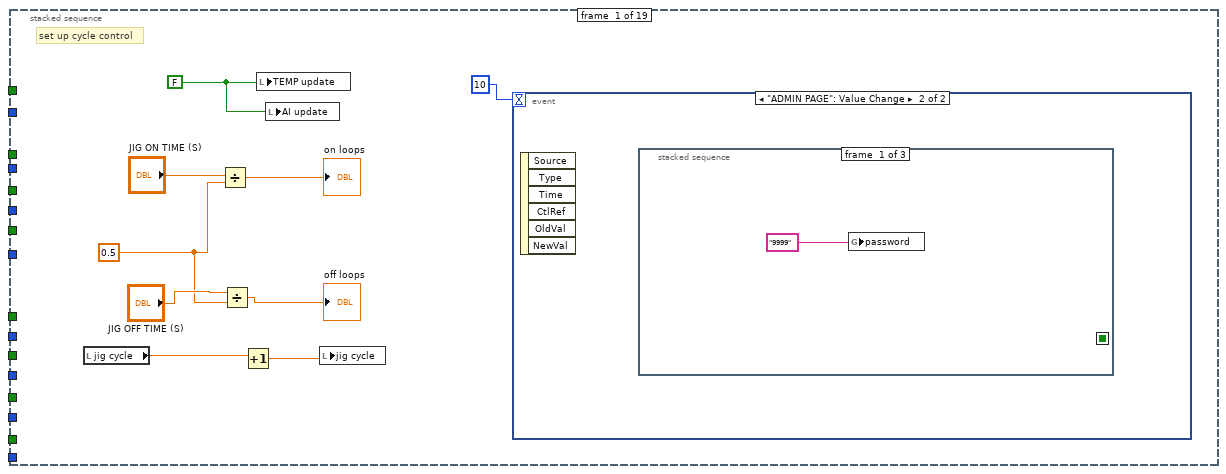
[diagram p10: hidden frame]
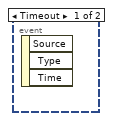
[diagram p11: hidden frame]
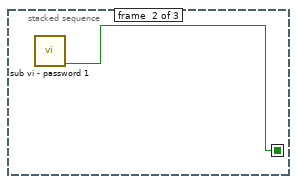
[diagram p12: hidden frame]
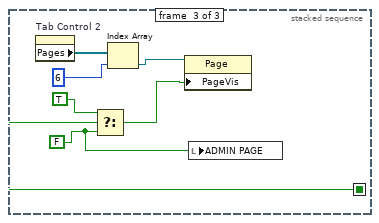
[diagram p13: hidden frame]
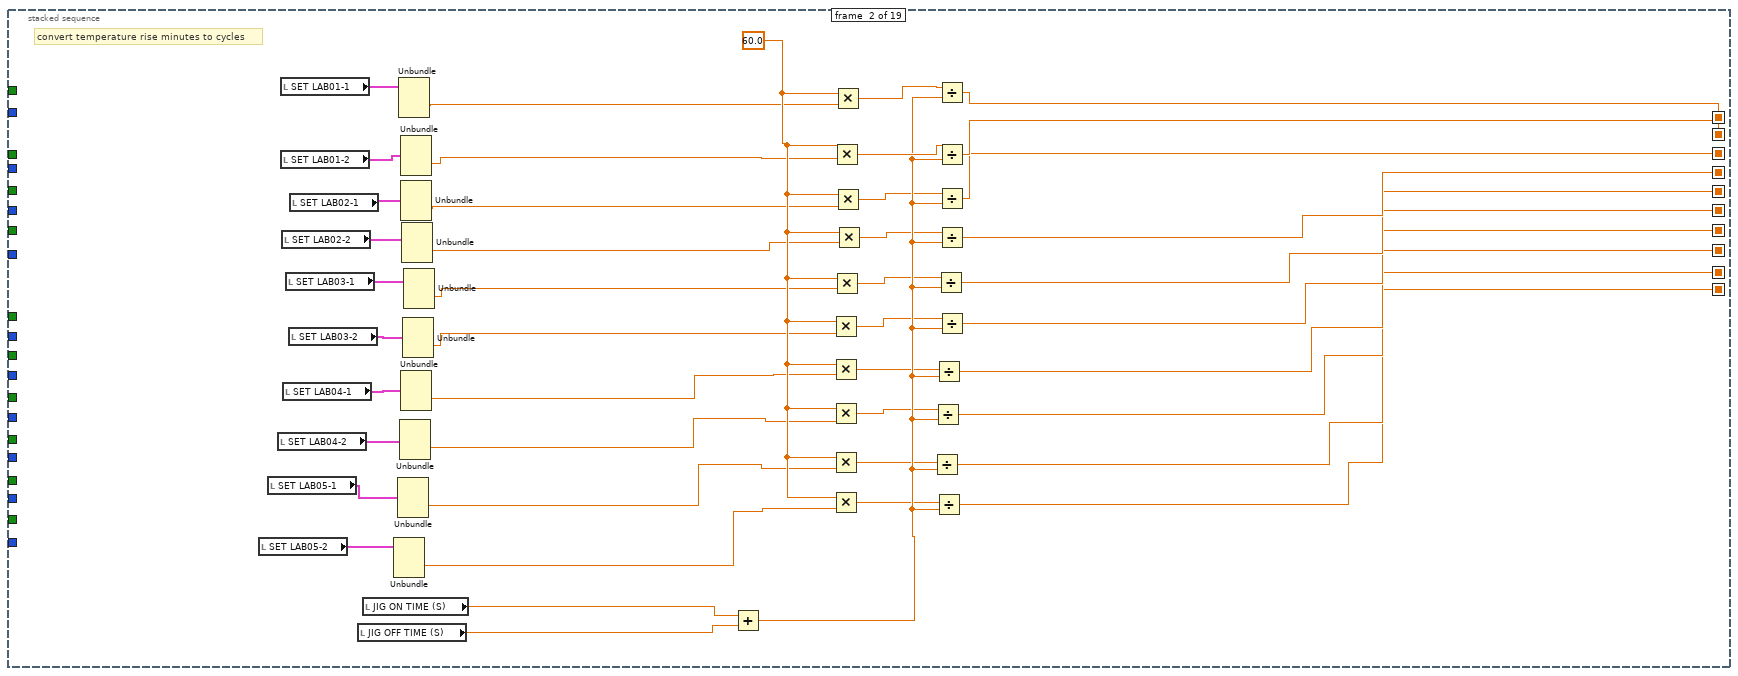
[diagram p14: hidden frame]
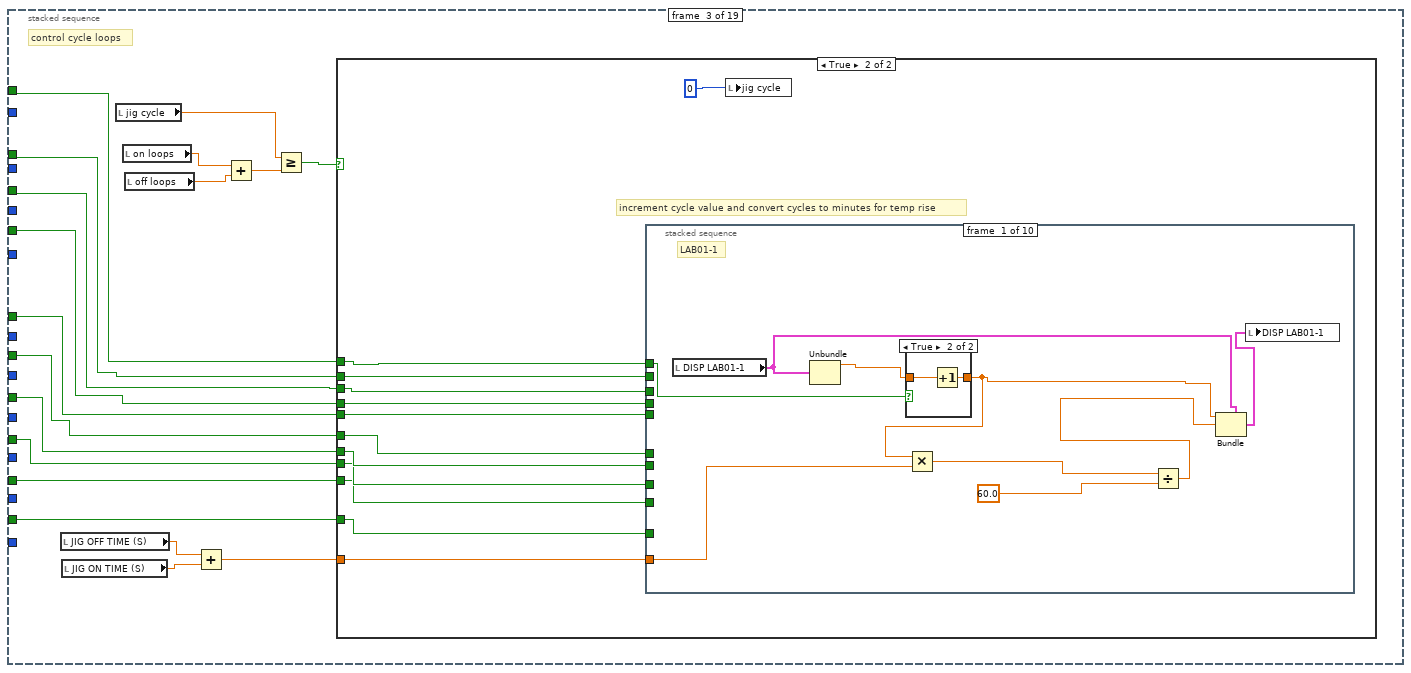
[diagram p15: hidden frame]
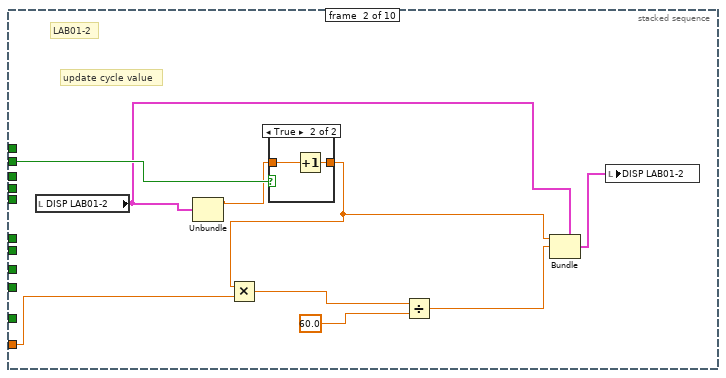
[diagram p18: hidden frame]
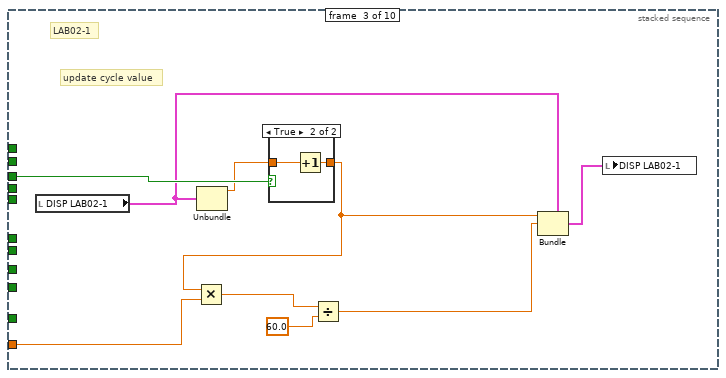
[diagram p20: hidden frame]
diagram:
  n1 = stacked-sequence {
    frame #0 {
      n2 = local write "loop  delay(mS)"(500) -> ()
      n3 = local write "stop2"(FALSE) -> ()
      "jig cycle" <- 0
    }
    frame #1 {
      # "do 1st time set up"
      n4 = stacked-sequence {
        frame #0 {
          # "disable front panel while 1st time set up is being done"
          n5 = property on="Tab Control 2" class="TabCtl (strict)"("DisabledEnum"=T13."Disabled and Grayed Out" ("Disabled")) -> ()  [unwired: 2 in, 2 out]
        }
        frame #1 {
          # "get calibration values"
          n6 = call "sub vi - get calibration values v1.vi"() -> ("LAB01 (CAL)"=→"CAL LAB01":T7, "LAB02 (CAL)"=→"CAL LAB02":T8, "LAB03 (CAL)"=→"CAL LAB03":T7, "LAB04 (CAL)"=→"CAL LAB04":T7, "calibration file error out"=→"calibration file error out":errorcluster, "LAB05 (CAL)"=→"CAL LAB05":T7)  [unwired: 10 in]
        }
        frame #2 {
          # "get last saved test settings from file"
          n7 = local read "Network Directory"() -> (w13:path)
          n8 = local read "C drive data root dir"() -> (w11:path)
          n9 = local read "SET LAB05-2"() -> (w43:T5)
          n10 = local read "SET LAB05-1"() -> (w44:T5)
          n11 = local read "SET LAB04-2"() -> (w45:T5)
          n12 = local read "SET LAB03-2"() -> (w42:T5)
          n13 = local read "SET LAB04-1"() -> (w46:T5)
          n14 = local read "SET LAB03-1"() -> (w41:T5)
          n15 = local read "SET LAB02-2"() -> (w40:T5)
          n16 = local read "SET LAB02-1"() -> (w39:T5)
          n17 = local read "SET LAB01-2"() -> (w38:T5)
          n18 = local read "SET LAB01-1"() -> (w37:T5)
          n19 = Bundle("SET LAB01-1"=w37, "SET LAB01-2"=w38, "SET LAB02-1"=w39, "SET LAB02-2"=w40, "SET LAB03-1"=w41, "SET LAB03-2"=w42, "SET LAB04-1"=w46, "SET LAB04-2"=w45, "SET LAB05-1"=w44, "SET LAB05-2"=w43, "Network Directory"=w13, "C drive data root dir"=w11) -> (w30:T19)  [unwired: 1 in]
          n20 = String To Path(string="c:\\crabtree\\Set Up\\") -> (path=w34:path)
          n21 = Build Path(base path=w34, name or relative path="settings.bin") -> (appended path=w32:path)
          n22 = Create Folder(path (use dialog)=w34) -> (error out=w36:errorcluster)  [unwired: 2 in, 2 out]
          n23 = call <vilib>:"Clear Errors.vi"("error in (no error)"=w36) -> ()  [unwired: 6 in, 1 out]
          n24 = Open/Create/Replace File(file path (use dialog)=w32) -> (refnum out=w29:refnum<file>, error out=w31:errorcluster)  [unwired: 5 in, 1 out]
          n25 = Read from Binary File(5:w30, 8:w31, 11:w29) -> (0:w26:errorcluster, 2:w28:T19, 3:w27:refnum<file>)  [unwired: 3 in, 1 out]
          n26 = Unbundle(w28) -> ("SET LAB01-1"=w24:T5, "SET LAB01-2"=w23:T5, "SET LAB02-1"=w22:T5, "SET LAB02-2"=w21:T5, "SET LAB03-1"=w20:T5, "SET LAB03-2"=w19:T5, "SET LAB04-1"=w18:T5, "SET LAB04-2"=w17:T5, "SET LAB05-1"=w16:T5, "SET LAB05-2"=w15:T5, "Network Directory"=w14:path, "C drive data root dir"=w12:path)
          n27 = local write "C drive data root dir"(w12) -> ()
          n28 = Close File(refnum=w27, error in=w26) -> (error out=w25:errorcluster)  [unwired: 1 out]
          n29 = local write "Network Directory"(w14) -> ()
          n30 = local write "SET LAB04-2"(w17) -> ()
          n31 = local write "SET LAB05-1"(w16) -> ()
          n32 = local write "SET LAB04-1"(w18) -> ()
          n33 = local write "SET LAB05-2"(w15) -> ()
          n34 = local write "SET LAB02-1"(w22) -> ()
          n35 = local write "SET LAB02-2"(w21) -> ()
          n36 = local write "SET LAB03-1"(w20) -> ()
          n37 = local write "SET LAB03-2"(w19) -> ()
          n38 = local write "SET LAB01-1"(w24) -> ()
          n39 = local write "SET LAB01-2"(w23) -> ()
          n40 = local write "data file error"(w25) -> ()
        }
        frame #3 {
          # "get mail settings"
          n41 = local read "Auto Mail Send"() -> (w50:bool)
          n42 = local read "MAIL SETTINGS"() -> (w54:T6)
          n43 = String To Path(string="c:\\crabtree\\Set Up\\") -> (path=w62:path)
          n44 = Build Path(base path=w62, name or relative path="mail.bin") -> (appended path=w60:path)
          n45 = Create Folder(path (use dialog)=w62) -> (error out=w64:errorcluster)  [unwired: 2 in, 2 out]
          n46 = Bundle("MAIL SETTINGS"=w54, "Auto Mail Send"=w50, "") -> (w53:T20)  [unwired: 1 in]
          n47 = call <vilib>:"Clear Errors.vi"("error in (no error)"=w64) -> ()  [unwired: 6 in, 1 out]
          n48 = Open/Create/Replace File(file path (use dialog)=w60) -> (refnum out=w58:refnum<file>, error out=w59:errorcluster)  [unwired: 5 in, 1 out]
          n49 = Read from Binary File(5:w53, 8:w59, 11:w58) -> (0:w56:errorcluster, 2:w52:T20, 3:w57:refnum<file>)  [unwired: 3 in, 1 out]
          n50 = Unbundle(w52) -> ("MAIL SETTINGS"=w51:T6, "Auto Mail Send"=w49:bool, w48:string)
          n51 = local write "TO (string):"(w48) -> ()
          n52 = local write "Auto Mail Send"(w49) -> ()
          n53 = local write "MAIL SETTINGS"(w51) -> ()
          n54 = Close File(refnum=w57, error in=w56) -> (error out=w55:errorcluster)  [unwired: 1 out]
          n55 = local write "data file error"(w55) -> ()
        }
        frame #4 {
          # "set display status if blank"
          n56 = local read "DISP LAB03-2"() -> (w94:T4)
          n57 = local read "DISP LAB03-1"() -> (w101:T4)
          n58 = local read "DISP LAB02-2"() -> (w108:T4)
          n59 = local read "DISP LAB01-2"() -> (w121:T4)
          n60 = local read "DISP LAB01-1"() -> (w130:T4)
          n61 = local read "DISP LAB02-1"() -> (w115:T4)
          n62 = Unbundle(w94) -> ("STATUS"=w96:string)  [unwired: 2 out]
          n63 = Unbundle(w101) -> ("STATUS"=w103:string)  [unwired: 2 out]
          n64 = Unbundle(w108) -> ("STATUS"=w110:string)  [unwired: 2 out]
          n65 = Unbundle(w115) -> ("STATUS"=w117:string)  [unwired: 2 out]
          n66 = Unbundle(w121) -> ("STATUS"=w124:string)  [unwired: 2 out]
          n67 = Unbundle(w130) -> ("STATUS"=w131:string)  [unwired: 2 out]
          n68 = Equal?(x="", y=w96) -> (x = y?=w98:bool)
          n69 = Equal?(x="", y=w103) -> (x = y?=w105:bool)
          n70 = Equal?(x="", y=w110) -> (x = y?=w112:bool)
          n71 = Equal?(x="", y=w117) -> (x = y?=w119:bool)
          n72 = Equal?(x="", y=w124) -> (x = y?=w126:bool)
          n73 = Equal?(x="", y=w131) -> (x = y?=w133:bool)
          n74 = Select(t="STOP", s=w98, f=w96) -> (s? t:f=w95:string)
          n75 = Select(t="STOP", s=w105, f=w103) -> (s? t:f=w102:string)
          n76 = Select(t="STOP", s=w112, f=w110) -> (s? t:f=w109:string)
          n77 = Select(t="STOP", s=w119, f=w117) -> (s? t:f=w116:string)
          n78 = Select(t="STOP", s=w126, f=w124) -> (s? t:f=w123:string)
          n79 = Select(t="STOP", s=w133, f=w131) -> (s? t:f=w129:string)
          n80 = Bundle(cluster=w94, "STATUS"=w95) -> (w93:T4)  [unwired: 2 in]
          n81 = Bundle(cluster=w101, "STATUS"=w102) -> (w100:T4)  [unwired: 2 in]
          n82 = Bundle(cluster=w108, "STATUS"=w109) -> (w107:T4)  [unwired: 2 in]
          n83 = Bundle(cluster=w115, "STATUS"=w116) -> (w114:T4)  [unwired: 2 in]
          n84 = Bundle(cluster=w121, "STATUS"=w123) -> (w122:T4)  [unwired: 2 in]
          n85 = Bundle(cluster=w130, "STATUS"=w129) -> (w128:T4)  [unwired: 2 in]
          n86 = local write "DISP LAB01-2"(w122) -> ()
          n87 = local write "DISP LAB01-1"(w128) -> ()
          n88 = local write "DISP LAB02-1"(w114) -> ()
          n89 = local write "DISP LAB03-1"(w100) -> ()
          n90 = local write "DISP LAB02-2"(w107) -> ()
          n91 = local write "DISP LAB03-2"(w93) -> ()
          n92 = local read "DISP LAB05-2"() -> (w66:T4)
          n93 = local read "DISP LAB05-1"() -> (w73:T4)
          n94 = local read "DISP LAB04-2"() -> (w75:T4)
          n95 = local read "DISP LAB04-1"() -> (w77:T4)
          n96 = Unbundle(w66) -> ("STATUS"=w68:string)  [unwired: 2 out]
          n97 = Unbundle(w73) -> ("STATUS"=w79:string)  [unwired: 2 out]
          n98 = Unbundle(w75) -> ("STATUS"=w84:string)  [unwired: 2 out]
          n99 = Unbundle(w77) -> ("STATUS"=w89:string)  [unwired: 2 out]
          n100 = Equal?(x="", y=w68) -> (x = y?=w70:bool)
          n101 = Equal?(x="", y=w79) -> (x = y?=w81:bool)
          n102 = Equal?(x="", y=w84) -> (x = y?=w86:bool)
          n103 = Equal?(x="", y=w89) -> (x = y?=w91:bool)
          n104 = Select(t="STOP", s=w70, f=w68) -> (s? t:f=w67:string)
          n105 = Select(t="STOP", s=w81, f=w79) -> (s? t:f=w78:string)
          n106 = Select(t="STOP", s=w86, f=w84) -> (s? t:f=w83:string)
          n107 = Select(t="STOP", s=w91, f=w89) -> (s? t:f=w88:string)
          n108 = Bundle(cluster=w66, "STATUS"=w67) -> (w65:T4)  [unwired: 2 in]
          n109 = Bundle(cluster=w73, "STATUS"=w78) -> (w72:T4)  [unwired: 2 in]
          n110 = Bundle(cluster=w75, "STATUS"=w83) -> (w74:T4)  [unwired: 2 in]
          n111 = Bundle(cluster=w77, "STATUS"=w88) -> (w76:T4)  [unwired: 2 in]
          n112 = local write "DISP LAB05-2"(w65) -> ()
          n113 = local write "DISP LAB05-1"(w72) -> ()
          n114 = local write "DISP LAB04-1"(w76) -> ()
          n115 = local write "DISP LAB04-2"(w74) -> ()
        }
        frame #5 {
          # "initialise analog input express vi's"
          n116 = for {
            N: 2.0 -> [_]
            n117 = call "sub vi - analog 1st setup v1.vi"() -> ()  [unwired: 11 in, 5 out]
          }
        }
        frame #6 {
          # "enable front panel, all settings done"
          n118 = property on="Tab Control 2" class="TabCtl (strict)"("DisabledEnum"=T13."Enabled" ("Disabled")) -> ()  [unwired: 2 in, 2 out]
        }
      }
    }
    frame #2 {
      n119 = node-c288("loop  delay(mS)") -> (w139:T14)  [unwired: 3 in]
      n120 = timed-loop {
        timing: w139 -> [_]
        timing-out: [_] -> w138
        i -> [w161]
        stop <- "stop" stop-if-true
        n121 = node-c288() -> ()  [unwired: 1 in, 1 out]
        n122 = local read "SELECT LAB05-2"() -> (w141:T3)
        n123 = local read "SELECT LAB05-1"() -> (w142:T3)
        n124 = local read "SELECT LAB04-2"() -> (w143:T3)
        n125 = local read "SELECT LAB03-1"() -> (w146:T3)
        n126 = local read "SELECT LAB02-2"() -> (w147:T3)
        n127 = local read "SELECT LAB01-1"() -> (w150:T3)
        n128 = local read "SELECT LAB03-2"() -> (w145:T3)
        n129 = local read "SELECT LAB01-2"() -> (w149:T3)
        n130 = local read "SELECT LAB04-1"() -> (w144:T3)
        n131 = local read "SELECT LAB02-1"() -> (w148:T3)
        n132 = local read "run lab03-2"() -> (w155:bool)
        n133 = local read "run lab04-1"() -> (w154:bool)
        n134 = local read "run lab05-1"() -> (w152:bool)
        n135 = local read "run lab04-2"() -> (w153:bool)
        n136 = local read "run lab05-2"() -> (w151:bool)
        n137 = local read "run lab03-1"() -> (w156:bool)
        n138 = local read "run lab02-2"() -> (w157:bool)
        n139 = local read "run lab02-1"() -> (w158:bool)
        n140 = local read "run lab01-1"() -> (w160:bool)
        n141 = local read "run lab01-2"() -> (w159:bool)
        n142 = stacked-sequence {
          seq-local: [_ w223 _ _ _ _ _ _ _ _ _ _ _ _ _ _ _ _ _] -> [_ _ _ _ _ w1758 _ _ _ _ _ _ _ _ _ _ _ _ _]
          seq-local: [_ w222 _ _ _ _ _ _ _ _ _ _ _ _ _ _ _ _ _] -> [_ _ _ _ _ w1757 _ _ _ _ _ _ _ _ _ _ _ _ _]
          seq-local: [_ w209 _ _ _ _ _ _ _ _ _ _ _ _ _ _ _ _ _] -> [_ _ _ _ _ w1756 _ _ _ _ _ _ _ _ _ _ _ _ _]
          seq-local: [_ w208 _ _ _ _ _ _ _ _ _ _ _ _ _ _ _ _ _] -> [_ _ _ _ _ w1755 _ _ _ _ _ _ _ _ _ _ _ _ _]
          seq-local: [_ w207 _ _ _ _ _ _ _ _ _ _ _ _ _ _ _ _ _] -> [_ _ _ _ _ w1754 _ _ _ _ _ _ _ _ _ _ _ _ _]
          seq-local: [_ w206 _ _ _ _ _ _ _ _ _ _ _ _ _ _ _ _ _] -> [_ _ _ _ _ w1753 _ _ _ _ _ _ _ _ _ _ _ _ _]
          seq-local: [_ w205 _ _ _ _ _ _ _ _ _ _ _ _ _ _ _ _ _] -> [_ _ _ _ _ w1752 _ _ _ _ _ _ _ _ _ _ _ _ _]
          seq-local: [_ w204 _ _ _ _ _ _ _ _ _ _ _ _ _ _ _ _ _] -> [_ _ _ _ _ w1751 _ _ _ _ _ _ _ _ _ _ _ _ _]
          seq-local: [_ w203 _ _ _ _ _ _ _ _ _ _ _ _ _ _ _ _ _] -> [_ _ _ _ _ w1750 _ _ _ _ _ _ _ _ _ _ _ _ _]
          seq-local: [_ w202 _ _ _ _ _ _ _ _ _ _ _ _ _ _ _ _ _] -> [_ _ _ _ _ w1749 _ _ _ _ _ _ _ _ _ _ _ _ _]
          tunnel: w160 -> [_ _ w239 w404 w1348 w1778 w2088 w2333 _ _ _ _ _ w2806 _ w3671 _ _ w3946]
          tunnel: w159 -> [_ _ w238 w402 w1347 w1777 w2089 w2332 _ _ _ _ _ w2805 _ w3669 _ _ w3945]
          tunnel: w158 -> [_ _ w237 w400 w1346 w1776 w2087 w2331 _ _ _ _ _ w2804 _ w3667 _ _ w3944]
          tunnel: w157 -> [_ _ w236 w398 w1345 w1775 w2086 w2330 _ _ _ _ _ w2803 _ w3665 _ _ w3943]
          tunnel: w156 -> [_ _ w235 w396 w1344 w1774 w2085 w2329 _ _ _ _ _ w2802 _ w3663 _ _ w3942]
          tunnel: w155 -> [_ _ w234 w394 w1343 w1773 w2084 w2328 _ _ _ _ _ w2801 _ w3661 _ _ w3941]
          tunnel: w154 -> [_ _ w233 w392 w1342 w1772 w2083 w2327 _ _ _ _ _ w2800 _ w3659 _ _ w3940]
          tunnel: w153 -> [_ _ w232 w390 w1341 w1771 w2082 w2326 _ _ _ _ _ w2799 _ w3657 _ _ w3939]
          tunnel: w152 -> [_ _ w231 w388 w1340 w1770 w2081 w2325 _ _ _ _ _ w2798 _ w3655 _ _ w3938]
          tunnel: w151 -> [_ _ w230 w386 w1339 w1769 w2080 w2324 _ _ _ _ _ w2797 _ w3653 _ _ w3937]
          tunnel: w150 -> [_ _ _ w403 w1338 w1768 _ _ _ _ _ _ _ _ _ w3673 _ _ _]
          tunnel: w149 -> [_ _ _ w401 w1337 w1767 _ _ _ _ _ _ _ _ _ w3668 _ _ _]
          tunnel: w148 -> [_ _ _ w399 w1336 w1766 _ _ _ _ _ _ _ _ _ w3666 _ _ _]
          tunnel: w147 -> [_ _ _ w397 w1335 w1765 _ _ _ _ _ _ _ _ _ w3664 _ _ _]
          tunnel: w146 -> [_ _ _ w395 w1334 w1764 _ _ _ _ _ _ _ _ _ w3662 _ _ _]
          tunnel: w145 -> [_ _ _ w393 w1333 w1763 _ _ _ _ _ _ _ _ _ w3660 _ _ _]
          tunnel: w144 -> [_ _ _ w391 w1332 w1762 _ _ _ _ _ _ _ _ _ w3658 _ _ _]
          tunnel: w143 -> [_ _ _ w389 w1331 w1761 _ _ _ _ _ _ _ _ _ w3656 _ _ _]
          tunnel: w142 -> [_ _ _ w387 w1330 w1760 _ _ _ _ _ _ _ _ _ w3654 _ _ _]
          tunnel: w141 -> [_ _ _ w385 w1329 w1759 _ _ _ _ _ _ _ _ _ w3652 _ _ _]
          frame #0 {
            w165 = FALSE
            w170 = 0.5
            # "set up cycle control"
            n143 = local read "jig cycle"() -> (w169:dbl)
            n144 = Divide(x="JIG ON TIME (S)", y=w170) -> (x/y=→"on loops":dbl)
            n145 = Divide(x="JIG OFF TIME (S)", y=w170) -> (x/y=→"off loops":dbl)
            n146 = Increment(x=w169) -> (x+1=w168:dbl)
            n147 = local write "TEMP update"(w165) -> ()
            n148 = local write "AI update"(w165) -> ()
            n149 = local write "jig cycle"(w168) -> ()
            n150 = event shown="[1] \"ADMIN PAGE\": Value Change" {
              selector: _ -> [_ _]
              dyn-events: _ -> [_ _]
              timeout: 10 -> [_ _]
              event Timeout {
                n151 = event-data() -> ()  [unwired: 1 in, 3 out]
              }
              event "ADMIN PAGE": Value Change {
                n152 = event-data() -> ()  [unwired: 1 in, 6 out]
                n153 = stacked-sequence {
                  seq-local: [_ w174 _] -> [_ _ w175]
                  frame #0 {
                    n154 = global write "Global 1.vi" "password"("9999") -> ()
                  }
                  frame #1 {
                    n155 = call "sub vi - password 1.vi"() -> ("RESULT"=w174:bool)  [unwired: 11 in]
                  }
                  frame #2 {
                    w177 = FALSE
                    n156 = property on="Tab Control 2" class="TabCtl (strict)"() -> ("Pages"=w181:refnum<vi>[])  [unwired: 2 in, 2 out]
                    n157 = Select(t=TRUE, s=w175, f=w177) -> (s? t:f=w176:bool)
                    n158 = Index Array(array=w181, index=6) -> (element=w179:refnum<vi>)
                    n159 = property class="Page"(reference=w179, "PageVis"=w176) -> ()  [unwired: 1 in, 2 out]
                    n160 = local write "ADMIN PAGE"(w177) -> ()
                  }
                }
              }
            }
          }
          frame #1 {
            w219 = 60.0
            # "convert temperature rise minutes to cycles"
            n161 = local read "SET LAB05-2"() -> (w183:T5)
            n162 = local read "SET LAB05-1"() -> (w185:T5)
            n163 = local read "SET LAB04-2"() -> (w187:T5)
            n164 = local read "SET LAB01-1"() -> (w201:T5)
            n165 = local read "SET LAB01-2"() -> (w199:T5)
            n166 = local read "SET LAB02-2"() -> (w195:T5)
            n167 = local read "SET LAB04-1"() -> (w189:T5)
            n168 = local read "SET LAB03-1"() -> (w193:T5)
            n169 = local read "SET LAB03-2"() -> (w191:T5)
            n170 = local read "SET LAB02-1"() -> (w197:T5)
            n171 = local read "JIG OFF TIME (S)"() -> (w224:dbl)
            n172 = local read "JIG ON TIME (S)"() -> (w225:dbl)
            n173 = Unbundle(w183) -> ("T-RISE mins"=w182:dbl)  [unwired: 4 out]
            n174 = Unbundle(w185) -> ("T-RISE mins"=w184:dbl)  [unwired: 4 out]
            n175 = Unbundle(w201) -> ("T-RISE mins"=w200:dbl)  [unwired: 4 out]
            n176 = Unbundle(w187) -> ("T-RISE mins"=w186:dbl)  [unwired: 4 out]
            n177 = Unbundle(w199) -> ("T-RISE mins"=w198:dbl)  [unwired: 4 out]
            n178 = Unbundle(w197) -> ("T-RISE mins"=w196:dbl)  [unwired: 4 out]
            n179 = Unbundle(w189) -> ("T-RISE mins"=w188:dbl)  [unwired: 4 out]
            n180 = Unbundle(w195) -> ("T-RISE mins"=w194:dbl)  [unwired: 4 out]
            n181 = Unbundle(w191) -> ("T-RISE mins"=w190:dbl)  [unwired: 4 out]
            n182 = Unbundle(w193) -> ("T-RISE mins"=w192:dbl)  [unwired: 4 out]
            n183 = Add(x=w225, y=w224) -> (x+y=w218:dbl)
            n184 = Multiply(x=w219, y=w190) -> (x*y=w214:dbl)
            n185 = Multiply(x=w219, y=w188) -> (x*y=w213:dbl)
            n186 = Multiply(x=w219, y=w186) -> (x*y=w212:dbl)
            n187 = Multiply(x=w219, y=w184) -> (x*y=w211:dbl)
            n188 = Multiply(x=w219, y=w182) -> (x*y=w210:dbl)
            n189 = Multiply(x=w219, y=w198) -> (x*y=w220:dbl)
            n190 = Multiply(x=w219, y=w192) -> (x*y=w215:dbl)
            n191 = Multiply(x=w219, y=w200) -> (x*y=w221:dbl)
            n192 = Multiply(x=w219, y=w196) -> (x*y=w217:dbl)
            n193 = Multiply(x=w219, y=w194) -> (x*y=w216:dbl)
            n194 = Divide(x=w211, y=w218) -> (x/y=w203:dbl)
            n195 = Divide(x=w212, y=w218) -> (x/y=w204:dbl)
            n196 = Divide(x=w213, y=w218) -> (x/y=w205:dbl)
            n197 = Divide(x=w210, y=w218) -> (x/y=w202:dbl)
            n198 = Divide(x=w215, y=w218) -> (x/y=w207:dbl)
            n199 = Divide(x=w221, y=w218) -> (x/y=w223:dbl)
            n200 = Divide(x=w220, y=w218) -> (x/y=w222:dbl)
            n201 = Divide(x=w217, y=w218) -> (x/y=w209:dbl)
            n202 = Divide(x=w216, y=w218) -> (x/y=w208:dbl)
            n203 = Divide(x=w214, y=w218) -> (x/y=w206:dbl)
          }
          frame #2 {
            # "control cycle loops"
            n204 = local read "JIG OFF TIME (S)"() -> (w228:dbl)
            n205 = local read "JIG ON TIME (S)"() -> (w227:dbl)
            n206 = local read "jig cycle"() -> (w241:dbl)
            n207 = local read "on loops"() -> (w243:dbl)
            n208 = local read "off loops"() -> (w242:dbl)
            n209 = Add(x=w228, y=w227) -> (x+y=w226:dbl)
            n210 = Add(x=w243, y=w242) -> (x+y=w229:dbl)
            n211 = Greater Or Equal?(x=w241, y=w229) -> (x >= y?=w240:bool)
            n212 = case shown="True" w240 {
              tunnel: w239 -> [_ w254]
              tunnel: w238 -> [_ w253]
              tunnel: w237 -> [_ w252]
              tunnel: w236 -> [_ w251]
              tunnel: w235 -> [_ w250]
              tunnel: w234 -> [_ w249]
              tunnel: w233 -> [_ w248]
              tunnel: w232 -> [_ w247]
              tunnel: w231 -> [_ w246]
              tunnel: w230 -> [_ w245]
              tunnel: w226 -> [_ w244]
              frame False {
              }
              frame True {
                # "increment cycle value and convert cycles to minutes for temp rise"
                n213 = stacked-sequence {
                  tunnel: w254 -> [w264 _ _ _ _ _ _ _ _ _]
                  tunnel: w253 -> [_ w276 _ _ _ _ _ _ _ _]
                  tunnel: w252 -> [_ _ w288 _ _ _ _ _ _ _]
                  tunnel: w251 -> [_ _ _ w300 _ _ _ _ _ _]
                  tunnel: w250 -> [_ _ _ _ w312 _ _ _ _ _]
                  tunnel: w249 -> [_ _ _ _ _ w324 _ _ _ _]
                  tunnel: w248 -> [_ _ _ _ _ _ w336 _ _ _]
                  tunnel: w247 -> [_ _ _ _ _ _ _ w348 _ _]
                  tunnel: w246 -> [_ _ _ _ _ _ _ _ w360 _]
                  tunnel: w245 -> [_ _ _ _ _ _ _ _ _ w372]
                  tunnel: w244 -> [w261 w273 w285 w297 w309 w321 w333 w345 w357 w369]
                  frame #0 {
                    # "LAB01-1"
                    n214 = local read "DISP LAB01-1"() -> (w259:T4)
                    n215 = Unbundle(w259) -> ("CYCLE"=w260:dbl)  [unwired: 2 out]
                    n216 = case shown="True" w264 {
                      tunnel: w260 -> [w265 w267]
                      tunnel: [w265 w266] -> w258
                      frame False {
                      }
                      frame True {
                        n217 = Increment(x=w267) -> (x+1=w266:dbl)
                      }
                    }
                    n218 = Multiply(x=w258, y=w261) -> (x*y=w262:dbl)
                    n219 = Divide(x=w262, y=60.0) -> (x/y=w257:dbl)
                    n220 = Bundle(cluster=w259, "CYCLE"=w258, "MINS"=w257) -> (w256:T4)  [unwired: 1 in]
                    n221 = local write "DISP LAB01-1"(w256) -> ()
                  }
                  frame #1 {
                    # "update cycle value"
                    # "LAB01-2"
                    n222 = local read "DISP LAB01-2"() -> (w271:T4)
                    n223 = Unbundle(w271) -> ("CYCLE"=w272:dbl)  [unwired: 2 out]
                    n224 = case shown="True" w276 {
                      tunnel: w272 -> [w277 w279]
                      tunnel: [w277 w278] -> w269
                      frame False {
                      }
                      frame True {
                        n225 = Increment(x=w279) -> (x+1=w278:dbl)
                      }
                    }
                    n226 = Multiply(x=w269, y=w273) -> (x*y=w274:dbl)
                    n227 = Divide(x=w274, y=60.0) -> (x/y=w268:dbl)
                    n228 = Bundle(cluster=w271, "CYCLE"=w269, "MINS"=w268) -> (w270:T4)  [unwired: 1 in]
                    n229 = local write "DISP LAB01-2"(w270) -> ()
                  }
                  frame #2 {
                    # "update cycle value"
                    # "LAB02-1"
                    n230 = local read "DISP LAB02-1"() -> (w283:T4)
                    n231 = Unbundle(w283) -> ("CYCLE"=w284:dbl)  [unwired: 2 out]
                    n232 = case shown="True" w288 {
                      tunnel: [w289 w291] -> w281
                      tunnel: w284 -> [w289 w290]
                      frame False {
                      }
                      frame True {
                        n233 = Increment(x=w290) -> (x+1=w291:dbl)
                      }
                    }
                    n234 = Multiply(x=w281, y=w285) -> (x*y=w286:dbl)
                    n235 = Divide(x=w286, y=60.0) -> (x/y=w280:dbl)
                    n236 = Bundle(cluster=w283, "CYCLE"=w281, "MINS"=w280) -> (w282:T4)  [unwired: 1 in]
                    n237 = local write "DISP LAB02-1"(w282) -> ()
                  }
                  frame #3 {
                    # "update cycle value"
                    # "LAB02-2"
                    n238 = local read "DISP LAB02-2"() -> (w295:T4)
                    n239 = Unbundle(w295) -> ("CYCLE"=w296:dbl)  [unwired: 2 out]
                    n240 = case shown="True" w300 {
                      tunnel: [w301 w303] -> w294
                      tunnel: w296 -> [w301 w302]
                      frame False {
                      }
                      frame True {
                        n241 = Increment(x=w302) -> (x+1=w303:dbl)
                      }
                    }
                    n242 = Multiply(x=w294, y=w297) -> (x*y=w298:dbl)
                    n243 = Divide(x=w298, y=60.0) -> (x/y=w293:dbl)
                    n244 = Bundle(cluster=w295, "CYCLE"=w294, "MINS"=w293) -> (w292:T4)  [unwired: 1 in]
                    n245 = local write "DISP LAB02-2"(w292) -> ()
                  }
                  frame #4 {
                    # "update cycle value"
                    # "LAB03-1"
                    n246 = local read "DISP LAB03-1"() -> (w307:T4)
                    n247 = Unbundle(w307) -> ("CYCLE"=w308:dbl)  [unwired: 2 out]
                    n248 = case shown="True" w312 {
                      tunnel: [w313 w315] -> w304
                      tunnel: w308 -> [w313 w314]
                      frame False {
                      }
                      frame True {
                        n249 = Increment(x=w314) -> (x+1=w315:dbl)
                      }
                    }
                    n250 = Multiply(x=w304, y=w309) -> (x*y=w310:dbl)
                    n251 = Divide(x=w310, y=60.0) -> (x/y=w305:dbl)
                    n252 = Bundle(cluster=w307, "CYCLE"=w304, "MINS"=w305) -> (w306:T4)  [unwired: 1 in]
                    n253 = local write "DISP LAB03-1"(w306) -> ()
                  }
                  frame #5 {
                    # "update cycle value"
                    # "LAB03-2"
                    n254 = local read "DISP LAB03-2"() -> (w319:T4)
                    n255 = Unbundle(w319) -> ("CYCLE"=w320:dbl)  [unwired: 2 out]
                    n256 = case shown="False" w324 {
                      tunnel: [w325 w327] -> w318
                      tunnel: w320 -> [w325 w326]
                      frame False {
                      }
                      frame True {
                        n257 = Increment(x=w326) -> (x+1=w327:dbl)
                      }
                    }
                    n258 = Multiply(x=w318, y=w321) -> (x*y=w322:dbl)
                    n259 = Divide(x=w322, y=60.0) -> (x/y=w317:dbl)
                    n260 = Bundle(cluster=w319, "CYCLE"=w318, "MINS"=w317) -> (w316:T4)  [unwired: 1 in]
                    n261 = local write "DISP LAB03-2"(w316) -> ()
                  }
                  frame #6 {
                    # "update cycle value"
                    # "LAB04-1"
                    n262 = local read "DISP LAB04-1"() -> (w331:T4)
                    n263 = Unbundle(w331) -> ("CYCLE"=w332:dbl)  [unwired: 2 out]
                    n264 = case shown="True" w336 {
                      tunnel: [w337 w339] -> w329
                      tunnel: w332 -> [w337 w338]
                      frame False {
                      }
                      frame True {
                        n265 = Increment(x=w338) -> (x+1=w339:dbl)
                      }
                    }
                    n266 = Multiply(x=w329, y=w333) -> (x*y=w334:dbl)
                    n267 = Divide(x=w334, y=60.0) -> (x/y=w328:dbl)
                    n268 = Bundle(cluster=w331, "CYCLE"=w329, "MINS"=w328) -> (w330:T4)  [unwired: 1 in]
                    n269 = local write "DISP LAB04-1"(w330) -> ()
                  }
                  frame #7 {
                    # "update cycle value"
                    # "LAB04-2"
                    n270 = local read "DISP LAB04-2"() -> (w343:T4)
                    n271 = Unbundle(w343) -> ("CYCLE"=w344:dbl)  [unwired: 2 out]
                    n272 = case shown="True" w348 {
                      tunnel: [w349 w351] -> w341
                      tunnel: w344 -> [w349 w350]
                      frame False {
                      }
                      frame True {
                        n273 = Increment(x=w350) -> (x+1=w351:dbl)
                      }
                    }
                    n274 = Multiply(x=w341, y=w345) -> (x*y=w347:dbl)
                    n275 = Divide(x=w347, y=60.0) -> (x/y=w340:dbl)
                    n276 = Bundle(cluster=w343, "CYCLE"=w341, "MINS"=w340) -> (w342:T4)  [unwired: 1 in]
                    n277 = local write "DISP LAB04-2"(w342) -> ()
                  }
                  frame #8 {
                    # "update cycle value"
                    # "LAB05-1"
                    n278 = local read "DISP LAB05-1"() -> (w355:T4)
                    n279 = Unbundle(w355) -> ("CYCLE"=w356:dbl)  [unwired: 2 out]
                    n280 = case shown="True" w360 {
                      tunnel: [w361 w363] -> w353
                      tunnel: w356 -> [w361 w362]
                      frame False {
                      }
                      frame True {
                        n281 = Increment(x=w362) -> (x+1=w363:dbl)
                      }
                    }
                    n282 = Multiply(x=w353, y=w357) -> (x*y=w358:dbl)
                    n283 = Divide(x=w358, y=60.0) -> (x/y=w352:dbl)
                    n284 = Bundle(cluster=w355, "CYCLE"=w353, "MINS"=w352) -> (w354:T4)  [unwired: 1 in]
                    n285 = local write "DISP LAB05-1"(w354) -> ()
                  }
                  frame #9 {
                    # "update cycle value"
                    # "LAB05-2"
                    n286 = local read "DISP LAB05-2"() -> (w368:T4)
                    n287 = Unbundle(w368) -> ("CYCLE"=w367:dbl)  [unwired: 2 out]
                    n288 = case shown="True" w372 {
                      tunnel: [w373 w375] -> w366
                      tunnel: w367 -> [w373 w374]
                      frame False {
                      }
                      frame True {
                        n289 = Increment(x=w374) -> (x+1=w375:dbl)
                      }
                    }
                    n290 = Multiply(x=w366, y=w369) -> (x*y=w370:dbl)
                    n291 = Divide(x=w370, y=60.0) -> (x/y=w365:dbl)
                    n292 = Bundle(cluster=w368, "CYCLE"=w366, "MINS"=w365) -> (w364:T4)  [unwired: 1 in]
                    n293 = local write "DISP LAB05-2"(w364) -> ()
                  }
                }
                n294 = local write "jig cycle"(0) -> ()
              }
            }
          }
          frame #3 {
            # "START & STOP test RUN switch change, start test if true and stop test if false"
            n295 = Get Date/Time In Seconds() -> (seconds since 1Jan1904=w383:timestamp)
            n296 = local read "C drive data root dir"() -> (w376:path)
            n297 = Format Date/Time String(time format string (%c)="%b\\%a%d", seconds (now)=w383) -> (date/time string=w407:string)  [unwired: 1 in]
            n298 = Format Date/Time String(time format string (%c)="%H%M", seconds (now)=w383) -> (date/time string=w405:string)  [unwired: 1 in]
            n299 = Format Date/Time String(time format string (%c)="LabPanel%Y", seconds (now)=w383) -> (date/time string=w382:string)  [unwired: 1 in]
            n300 = Path To String(path=w376) -> (string=w379:string)
            n301 = global write "Global 1.vi" "C drive root path"(w376) -> ()
            n302 = Concatenate Strings(w379, "\\") -> (w377:string)
            n303 = event shown="[2] \"RUN LAB01-2\": Value Change" {
              selector: _ -> [_ _ _ _ _ _ _ _ _ _ _]
              dyn-events: _ -> [_ _ _ _ _ _ _ _ _ _ _]
              timeout: 10 -> [_ _ _ _ _ _ _ _ _ _ _]
              tunnel: w377 -> [_ w415 w507 w599 w691 w783 w875 w967 w1059 w1151 w1243]
              tunnel: w407 -> [_ w414 w506 w598 w690 w782 w874 w966 w1058 w1150 w1242]
              tunnel: w405 -> [_ w412 w505 w597 w689 w781 w873 w965 w1057 w1149 w1241]
              tunnel: w403 -> [_ w413 _ _ _ _ _ _ _ _ _]
              tunnel: w404 -> [_ _ _ _ _ _ _ _ _ _ _]
              tunnel: w402 -> [_ _ _ _ _ _ _ _ _ _ _]
              tunnel: w401 -> [_ _ w504 _ _ _ _ _ _ _ _]
              tunnel: w400 -> [_ _ _ _ _ _ _ _ _ _ _]
              tunnel: w399 -> [_ _ _ w596 _ _ _ _ _ _ _]
              tunnel: w398 -> [_ _ _ _ _ _ _ _ _ _ _]
              tunnel: w397 -> [_ _ _ _ w688 _ _ _ _ _ _]
              tunnel: w396 -> [_ _ _ _ _ _ _ _ _ _ _]
              tunnel: w395 -> [_ _ _ _ _ w780 _ _ _ _ _]
              tunnel: w394 -> [_ _ _ _ _ _ _ _ _ _ _]
              tunnel: w393 -> [_ _ _ _ _ _ w872 _ _ _ _]
              tunnel: w392 -> [_ _ _ _ _ _ _ _ _ _ _]
              tunnel: w391 -> [_ _ _ _ _ _ _ w964 _ _ _]
              tunnel: w390 -> [_ _ _ _ _ _ _ _ _ _ _]
              tunnel: w389 -> [_ _ _ _ _ _ _ _ w1056 _ _]
              tunnel: w388 -> [_ _ _ _ _ _ _ _ _ _ _]
              tunnel: w387 -> [_ _ _ _ _ _ _ _ _ w1148 _]
              tunnel: w386 -> [_ _ _ _ _ _ _ _ _ _ _]
              tunnel: w385 -> [_ _ _ _ _ _ _ _ _ _ w1240]
              tunnel: w382 -> [_ w411 w503 w595 w687 w779 w871 w963 w1055 w1147 w1239]
              tunnel: [_ w410 w502 w594 w686 w778 w870 w962 w1054 w1146 w1238] -> w380
              event Timeout {
                n304 = event-data() -> ()  [unwired: 1 in, 3 out]
              }
              event "RUN LAB01-1": Value Change {
                n305 = event-data() -> ("NewVal"=w409:bool)  [unwired: 1 in, 5 out]
                n306 = local write "run lab01-1"(w409) -> ()
                n307 = case shown="True" w409 {
                  tunnel: w415 -> [_ w448]
                  tunnel: w414 -> [_ w447]
                  tunnel: w413 -> [w417 w446]
                  tunnel: w412 -> [_ w445]
                  tunnel: w411 -> [_ w444]
                  tunnel: [w416 w443] -> w410
                  frame False {
                    # "stop test"
                    n308 = stacked-sequence {
                      tunnel: w417 -> [_ w429 _ _]
                      tunnel: [_ w421 _ _] -> w416
                      frame #0 {
                        n309 = local read "DISP LAB01-1"() -> (w420:T4)
                        n310 = Bundle(cluster=w420, "STATUS"="STOP") -> (w418:T4)  [unwired: 2 in]
                        n311 = local write "DISP LAB01-1"(w418) -> ()
                      }
                      frame #1 {
                        n312 = local read "DISP LAB01-1"() -> (w428:T4)
                        n313 = Unbundle(w428) -> ("CYCLE"=w426:dbl, "MINS"=w427:dbl)  [unwired: 1 out]
                        n314 = case shown="\"CYCLE TEST\"" w429 {
                          tunnel: w427 -> [_ _ w436]
                          tunnel: w426 -> [w434 w435 _]
                          tunnel: [w434 w435 w436] -> w425
                          frame "CHART TEST", Default {
                          }
                          frame "CYCLE TEST" {
                          }
                          frame "T-RISE TEST" {
                          }
                        }
                        n315 = local read "TDMS LAB01-1"() -> (w433:refnum<k34>)
                        n316 = Build Array("STOPPED") -> (w430:string[])
                        n317 = Build Array(w425) -> (w424:dbl[])
                        n318 = TDMS Write(0:w433, 5:"TEST RESULT", 7:w430, 9:w424) -> (4:w422:refnum<k34>, 15:w423:errorcluster)  [unwired: 2 in, 2 out]
                        n319 = TDMS Close(8:w423, 11:w422) -> (0:w421:errorcluster)  [unwired: 1 out]
                      }
                      frame #2 {
                        n320 = stacked-sequence {
                          tunnel: "LAB01-1" -> [w439 w441]
                          frame #0 {
                            n321 = call "sub vi - defrag tdms v1.vi"("panel id"=w439) -> ("error out"=w438:errorcluster)  [unwired: 10 in]
                            n322 = local write "data file error"(w438) -> ()
                          }
                          frame #1 {
                            n323 = call "Save data file to network drive v1.vi"("panel id"=w441) -> ("network file save error"=w440:errorcluster)  [unwired: 9 in, 1 out]
                            n324 = local write "RESULT LAB01-1"(FALSE) -> ()
                            n325 = local write "data file error"(w440) -> ()
                          }
                        }
                      }
                      frame #3 {
                      }
                    }
                  }
                  frame True {
                    # "start new test and create test file"
                    n326 = stacked-sequence {
                      seq-local: [w449 _ _ _ _] -> [_ w470 _ _ _]
                      tunnel: w448 -> [w454 _ _ _ _]
                      tunnel: w447 -> [w450 _ _ _ _]
                      tunnel: w446 -> [w464 _ _ _ _]
                      tunnel: w445 -> [w457 _ _ _ _]
                      tunnel: w444 -> [w452 _ _ _ _]
                      tunnel: [_ w471 _ _ _] -> w443
                      frame #0 {
                        w451 = "\\"
                        n327 = case shown="\"CHART TEST\", Default" w464 {
                          tunnel: ["L01-1-CHART TEST-" "L01-1-CYCLE TEST-" "L01-1-T-RISE TEST-"] -> w460
                          frame "CHART TEST", Default {
                          }
                          frame "CYCLE TEST" {
                          }
                          frame "T-RISE TEST" {
                          }
                        }
                        n328 = local read "SET LAB01-1"() -> (w459:T5)
                        n329 = Unbundle(w459) -> ("DESCRIPTION"=w458:string)  [unwired: 4 out]
                        n330 = Concatenate Strings(w454, "\\", w452, w451, w450, w451) -> (w461:string)
                        n331 = String To Path(string=w461) -> (path=w463:path)
                        n332 = Concatenate Strings(w461, w460, w458, "-", w457, ".tdms") -> (w449:string)
                        n333 = Create Folder(path (use dialog)=w463) -> (error out=w462:errorcluster)  [unwired: 2 in, 2 out]
                        n334 = call <vilib>:"Clear Errors.vi"("error in (no error)"=w462) -> ()  [unwired: 6 in, 1 out]
                        n335 = global write "Global 1.vi" "LAB01-1 FILE"(w449) -> ()
                      }
                      frame #1 {
                        n336 = String To Path(string=w470) -> (path=w468:path)
                        n337 = TDMS Open(5:FALSE, 6:FALSE, 10:T17."create or replace" ("operation (0:open)"), 11:w468) -> (0:w471:errorcluster, 3:→"TDMS LAB01-1":refnum<k34>)  [unwired: 3 in]
                      }
                      frame #2 {
                        n338 = local read "TDMS LAB01-1"() -> (w491:refnum<k34>)
                        n339 = local read "SET LAB01-1"() -> (w480:T5)
                        n340 = Build Array("Testers Name", "Description", "Set Test Cycles", "T-Rise minutes", "T-Rise Deg C") -> (w481:string[])
                        n341 = Unbundle(w480) -> ("NAME"=w479:string, "DESCRIPTION"=w478:string, "CYCLES"=w477:dbl, "T-RISE mins"=w476:dbl, "T-RISE deg C"=w475:dbl)
                        n342 = Number To Decimal String(number=w477) -> (decimal integer string=w490:string)  [unwired: 1 in]
                        n343 = Number To Decimal String(number=w476) -> (decimal integer string=w489:string)  [unwired: 1 in]
                        n344 = Number To Decimal String(number=w475) -> (decimal integer string=w488:string)  [unwired: 1 in]
                        n345 = Build Array(w479, w478, w490, w489, w488) -> (w487:string[])
                        n346 = TDMS Set Properties(5:w487, 7:w481, 11:w491) -> ()  [unwired: 3 in, 4 out]
                      }
                      frame #3 {
                        w492 = 0.0
                        n347 = local read "DISP LAB01-1"() -> (w495:T4)
                        n348 = Bundle(cluster=w495, "CYCLE"=w492, "MINS"=w492, "STATUS"="RUN") -> (w494:T4)
                        n349 = local write "DISP LAB01-1"(w494) -> ()
                      }
                      frame #4 {
                        n350 = local read "SIG LAB01-1"() -> (w498:T2)
                        n351 = local read "TEMP START LAB01-1"() -> (w500:cluster{"TL":dbl, "TN":dbl})
                        n352 = Unbundle(w498) -> ("Tmp Live"=w497:dbl, "Tmp Neut"=w496:dbl)  [unwired: 3 out]
                        n353 = Bundle(cluster=w500, "TL"=w497, "TN"=w496) -> (w499:cluster{"TL":dbl, "TN":dbl})
                        n354 = local write "TEMP START LAB01-1"(w499) -> ()
                      }
                    }
                  }
                }
              }
              event "RUN LAB01-2": Value Change {
                n355 = event-data() -> ("NewVal"=w501:bool)  [unwired: 1 in, 5 out]
                n356 = local write "run lab01-2"(w501) -> ()
                n357 = case shown="True" w501 {
                  tunnel: w507 -> [_ w540]
                  tunnel: w506 -> [_ w539]
                  tunnel: w504 -> [w509 w538]
                  tunnel: w505 -> [_ w537]
                  tunnel: w503 -> [_ w536]
                  tunnel: [w508 w535] -> w502
                  frame False {
                    # "stop test"
                    n358 = stacked-sequence {
                      tunnel: w509 -> [w518 _]
                      tunnel: [w510 _] -> w508
                      frame #0 {
                        n359 = local read "DISP LAB01-2"() -> (w517:T4)
                        n360 = Unbundle(w517) -> ("CYCLE"=w515:dbl, "MINS"=w516:dbl)  [unwired: 1 out]
                        n361 = case shown="\"CHART TEST\", Default" w518 {
                          tunnel: w516 -> [_ _ w525]
                          tunnel: w515 -> [w523 w524 _]
                          tunnel: [w523 w524 w525] -> w514
                          frame "CHART TEST", Default {
                          }
                          frame "CYCLE TEST" {
                          }
                          frame "T-RISE TEST" {
                          }
                        }
                        n362 = local read "TDMS LAB01-2"() -> (w522:refnum<k34>)
                        n363 = Build Array("STOPPED") -> (w519:string[])
                        n364 = Build Array(w514) -> (w513:dbl[])
                        n365 = TDMS Write(0:w522, 5:"TEST RESULT", 7:w519, 9:w513) -> (4:w511:refnum<k34>, 15:w512:errorcluster)  [unwired: 2 in, 2 out]
                        n366 = TDMS Close(8:w512, 11:w511) -> (0:w510:errorcluster)  [unwired: 1 out]
                      }
                      frame #1 {
                        n367 = local read "DISP LAB01-2"() -> (w529:T4)
                        n368 = stacked-sequence {
                          tunnel: "LAB01-2" -> [w531 w533]
                          frame #0 {
                            n369 = call "sub vi - defrag tdms v1.vi"("panel id"=w531) -> ("error out"=w530:errorcluster)  [unwired: 10 in]
                            n370 = local write "data file error"(w530) -> ()
                          }
                          frame #1 {
                            n371 = call "Save data file to network drive v1.vi"("panel id"=w533) -> ("network file save error"=w532:errorcluster)  [unwired: 9 in, 1 out]
                            n372 = local write "RESULT LAB01-2"(FALSE) -> ()
                            n373 = local write "data file error"(w532) -> ()
                          }
                        }
                        n374 = Bundle(cluster=w529, "STATUS"="STOP") -> (w527:T4)  [unwired: 2 in]
                        n375 = local write "DISP LAB01-2"(w527) -> ()
                      }
                    }
                  }
                  frame True {
                    # "start new test and create test file"
                    n376 = stacked-sequence {
                      seq-local: [w541 _ _ _ _] -> [_ w566 _ _ _]
                      tunnel: w540 -> [w546 _ _ _ _]
                      tunnel: w539 -> [w543 _ _ _ _]
                      tunnel: w538 -> [w556 _ _ _ _]
                      tunnel: w537 -> [w549 _ _ _ _]
                      tunnel: w536 -> [w544 _ _ _ _]
                      tunnel: [_ w560 _ _ _] -> w535
                      frame #0 {
                        w542 = "\\"
                        n377 = local read "SET LAB01-2"() -> (w551:T5)
                        n378 = case shown="\"CYCLE TEST\"" w556 {
                          tunnel: ["L01-2-CHART TEST-" "L01-2-CYCLE TEST-" "L01-2-T-RISE TEST-"] -> w552
                          frame "CHART TEST", Default {
                          }
                          frame "CYCLE TEST" {
                          }
                          frame "T-RISE TEST" {
                          }
                        }
                        n379 = Unbundle(w551) -> ("DESCRIPTION"=w550:string)  [unwired: 4 out]
                        n380 = Concatenate Strings(w546, "\\", w544, w542, w543, w542) -> (w553:string)
                        n381 = String To Path(string=w553) -> (path=w555:path)
                        n382 = Concatenate Strings(w553, w552, w550, "-", w549, ".tdms") -> (w541:string)
                        n383 = Create Folder(path (use dialog)=w555) -> (error out=w554:errorcluster)  [unwired: 2 in, 2 out]
                        n384 = global write "Global 1.vi" "LAB01-2 FILE"(w541) -> ()
                        n385 = call <vilib>:"Clear Errors.vi"("error in (no error)"=w554) -> ()  [unwired: 6 in, 1 out]
                      }
                      frame #1 {
                        n386 = String To Path(string=w566) -> (path=w561:path)
                        n387 = TDMS Open(5:FALSE, 6:FALSE, 10:T17."create or replace" ("operation (0:open)"), 11:w561) -> (0:w560:errorcluster, 3:→"TDMS LAB01-2":refnum<k34>)  [unwired: 3 in]
                      }
                      frame #2 {
                        n388 = local read "SET LAB01-2"() -> (w572:T5)
                        n389 = local read "TDMS LAB01-2"() -> (w583:refnum<k34>)
                        n390 = Build Array("Testers Name", "Description", "Set Test Cycles", "T-Rise minutes", "T-Rise Deg C") -> (w573:string[])
                        n391 = Unbundle(w572) -> ("NAME"=w571:string, "DESCRIPTION"=w570:string, "CYCLES"=w569:dbl, "T-RISE mins"=w568:dbl, "T-RISE deg C"=w567:dbl)
                        n392 = Number To Decimal String(number=w569) -> (decimal integer string=w582:string)  [unwired: 1 in]
                        n393 = Number To Decimal String(number=w568) -> (decimal integer string=w581:string)  [unwired: 1 in]
                        n394 = Number To Decimal String(number=w567) -> (decimal integer string=w580:string)  [unwired: 1 in]
                        n395 = Build Array(w571, w570, w582, w581, w580) -> (w579:string[])
                        n396 = TDMS Set Properties(5:w579, 7:w573, 11:w583) -> ()  [unwired: 3 in, 4 out]
                      }
                      frame #3 {
                        w585 = 0.0
                        n397 = local read "DISP LAB01-2"() -> (w587:T4)
                        n398 = Bundle(cluster=w587, "CYCLE"=w585, "MINS"=w585, "STATUS"="RUN") -> (w586:T4)
                        n399 = local write "DISP LAB01-2"(w586) -> ()
                      }
                      frame #4 {
                        n400 = local read "SIG LAB01-2"() -> (w590:T2)
                        n401 = local read "TEMP START LAB01-2"() -> (w592:cluster{"TL":dbl, "TN":dbl})
                        n402 = Unbundle(w590) -> ("Tmp Live"=w589:dbl, "Tmp Neut"=w588:dbl)  [unwired: 3 out]
                        n403 = Bundle(cluster=w592, "TL"=w589, "TN"=w588) -> (w591:cluster{"TL":dbl, "TN":dbl})
                        n404 = local write "TEMP START LAB01-2"(w591) -> ()
                      }
                    }
                  }
                }
              }
              event "RUN LAB02-1": Value Change {
                n405 = event-data() -> ("NewVal"=w593:bool)  [unwired: 1 in, 5 out]
                n406 = local write "run lab02-1"(w593) -> ()
                n407 = case shown="True" w593 {
                  tunnel: w599 -> [_ w632]
                  tunnel: w598 -> [_ w631]
                  tunnel: w596 -> [w601 w630]
                  tunnel: w597 -> [_ w629]
                  tunnel: w595 -> [_ w628]
                  tunnel: [w600 w627] -> w594
                  frame False {
                    # "stop test"
                    n408 = stacked-sequence {
                      tunnel: w601 -> [w610 _]
                      tunnel: [w602 _] -> w600
                      frame #0 {
                        n409 = local read "DISP LAB02-1"() -> (w609:T4)
                        n410 = Unbundle(w609) -> ("CYCLE"=w607:dbl, "MINS"=w608:dbl)  [unwired: 1 out]
                        n411 = case shown="\"CYCLE TEST\"" w610 {
                          tunnel: w608 -> [_ _ w617]
                          tunnel: w607 -> [w615 w616 _]
                          tunnel: [w615 w616 w617] -> w606
                          frame "CHART TEST", Default {
                          }
                          frame "CYCLE TEST" {
                          }
                          frame "T-RISE TEST" {
                          }
                        }
                        n412 = local read "TDMS LAB02-1"() -> (w614:refnum<k34>)
                        n413 = Build Array("STOPPED") -> (w611:string[])
                        n414 = Build Array(w606) -> (w605:dbl[])
                        n415 = TDMS Write(0:w614, 5:"TEST RESULT", 7:w611, 9:w605) -> (4:w603:refnum<k34>, 15:w604:errorcluster)  [unwired: 2 in, 2 out]
                        n416 = TDMS Close(8:w604, 11:w603) -> (0:w602:errorcluster)  [unwired: 1 out]
                      }
                      frame #1 {
                        n417 = local read "DISP LAB02-1"() -> (w621:T4)
                        n418 = stacked-sequence {
                          tunnel: "LAB02-1" -> [w623 w625]
                          frame #0 {
                            n419 = call "sub vi - defrag tdms v1.vi"("panel id"=w623) -> ("error out"=w622:errorcluster)  [unwired: 10 in]
                            n420 = local write "data file error"(w622) -> ()
                          }
                          frame #1 {
                            n421 = local write "RESULT LAB02-1"(FALSE) -> ()
                            n422 = call "Save data file to network drive v1.vi"("panel id"=w625) -> ("network file save error"=w624:errorcluster)  [unwired: 9 in, 1 out]
                            n423 = local write "data file error"(w624) -> ()
                          }
                        }
                        n424 = Bundle(cluster=w621, "STATUS"="STOP") -> (w619:T4)  [unwired: 2 in]
                        n425 = local write "DISP LAB02-1"(w619) -> ()
                      }
                    }
                  }
                  frame True {
                    # "start new test and create test file"
                    n426 = stacked-sequence {
                      seq-local: [w633 _ _ _ _] -> [_ w658 _ _ _]
                      tunnel: w632 -> [w638 _ _ _ _]
                      tunnel: w631 -> [w635 _ _ _ _]
                      tunnel: w630 -> [w648 _ _ _ _]
                      tunnel: w629 -> [w641 _ _ _ _]
                      tunnel: w628 -> [w636 _ _ _ _]
                      tunnel: [_ w652 _ _ _] -> w627
                      frame #0 {
                        w634 = "\\"
                        n427 = local read "SET LAB02-1"() -> (w643:T5)
                        n428 = case shown="\"CYCLE TEST\"" w648 {
                          tunnel: ["L02-1-CHART TEST-" "L02-1-CYCLE TEST-" "L02-1-T-RISE TEST-"] -> w644
                          frame "CHART TEST", Default {
                          }
                          frame "CYCLE TEST" {
                          }
                          frame "T-RISE TEST" {
                          }
                        }
                        n429 = Unbundle(w643) -> ("DESCRIPTION"=w642:string)  [unwired: 4 out]
                        n430 = Concatenate Strings(w638, "\\", w636, w634, w635, w634) -> (w645:string)
                        n431 = String To Path(string=w645) -> (path=w647:path)
                        n432 = Concatenate Strings(w645, w644, w642, "-", w641, ".tdms") -> (w633:string)
                        n433 = Create Folder(path (use dialog)=w647) -> (error out=w646:errorcluster)  [unwired: 2 in, 2 out]
                        n434 = global write "Global 1.vi" "LAB02-1 FILE"(w633) -> ()
                        n435 = call <vilib>:"Clear Errors.vi"("error in (no error)"=w646) -> ()  [unwired: 6 in, 1 out]
                      }
                      frame #1 {
                        n436 = String To Path(string=w658) -> (path=w653:path)
                        n437 = TDMS Open(5:FALSE, 6:FALSE, 10:T17."create or replace" ("operation (0:open)"), 11:w653) -> (0:w652:errorcluster, 3:→"TDMS LAB02-1":refnum<k34>)  [unwired: 3 in]
                      }
                      frame #2 {
                        n438 = local read "SET LAB02-1"() -> (w664:T5)
                        n439 = local read "TDMS LAB02-1"() -> (w675:refnum<k34>)
                        n440 = Build Array("Testers Name", "Description", "Set Test Cycles", "T-Rise minutes", "T-Rise Deg C") -> (w665:string[])
                        n441 = Unbundle(w664) -> ("NAME"=w663:string, "DESCRIPTION"=w662:string, "CYCLES"=w661:dbl, "T-RISE mins"=w660:dbl, "T-RISE deg C"=w659:dbl)
                        n442 = Number To Decimal String(number=w661) -> (decimal integer string=w674:string)  [unwired: 1 in]
                        n443 = Number To Decimal String(number=w660) -> (decimal integer string=w673:string)  [unwired: 1 in]
                        n444 = Number To Decimal String(number=w659) -> (decimal integer string=w672:string)  [unwired: 1 in]
                        n445 = Build Array(w663, w662, w674, w673, w672) -> (w671:string[])
                        n446 = TDMS Set Properties(5:w671, 7:w665, 11:w675) -> ()  [unwired: 3 in, 4 out]
                      }
                      frame #3 {
                        w677 = 0.0
                        n447 = local read "DISP LAB02-1"() -> (w679:T4)
                        n448 = Bundle(cluster=w679, "CYCLE"=w677, "MINS"=w677, "STATUS"="RUN") -> (w678:T4)
                        n449 = local write "DISP LAB02-1"(w678) -> ()
                      }
                      frame #4 {
                        n450 = local read "SIG LAB02-1"() -> (w682:T2)
                        n451 = local read "TEMP START LAB02-1"() -> (w684:cluster{"TL":dbl, "TN":dbl})
                        n452 = Unbundle(w682) -> ("Tmp Live"=w681:dbl, "Tmp Neut"=w680:dbl)  [unwired: 3 out]
                        n453 = Bundle(cluster=w684, "TL"=w681, "TN"=w680) -> (w683:cluster{"TL":dbl, "TN":dbl})
                        n454 = local write "TEMP START LAB02-1"(w683) -> ()
                      }
                    }
                  }
                }
              }
              event "RUN LAB02-2": Value Change {
                n455 = event-data() -> ("NewVal"=w685:bool)  [unwired: 1 in, 5 out]
                n456 = local write "run lab02-2"(w685) -> ()
                n457 = case shown="True" w685 {
                  tunnel: w691 -> [_ w724]
                  tunnel: w690 -> [_ w723]
                  tunnel: w688 -> [w693 w722]
                  tunnel: w689 -> [_ w721]
                  tunnel: w687 -> [_ w720]
                  tunnel: [w692 w719] -> w686
                  frame False {
                    # "stop test"
                    n458 = stacked-sequence {
                      tunnel: w693 -> [w702 _]
                      tunnel: [w694 _] -> w692
                      frame #0 {
                        n459 = local read "DISP LAB02-2"() -> (w701:T4)
                        n460 = Unbundle(w701) -> ("CYCLE"=w699:dbl, "MINS"=w700:dbl)  [unwired: 1 out]
                        n461 = case shown="\"CYCLE TEST\"" w702 {
                          tunnel: w700 -> [_ _ w709]
                          tunnel: w699 -> [w707 w708 _]
                          tunnel: [w707 w708 w709] -> w698
                          frame "CHART TEST", Default {
                          }
                          frame "CYCLE TEST" {
                          }
                          frame "T-RISE TEST" {
                          }
                        }
                        n462 = local read "TDMS LAB02-2"() -> (w706:refnum<k34>)
                        n463 = Build Array("STOPPED") -> (w703:string[])
                        n464 = Build Array(w698) -> (w697:dbl[])
                        n465 = TDMS Write(0:w706, 5:"TEST RESULT", 7:w703, 9:w697) -> (4:w695:refnum<k34>, 15:w696:errorcluster)  [unwired: 2 in, 2 out]
                        n466 = TDMS Close(8:w696, 11:w695) -> (0:w694:errorcluster)  [unwired: 1 out]
                      }
                      frame #1 {
                        n467 = local read "DISP LAB02-2"() -> (w713:T4)
                        n468 = stacked-sequence {
                          tunnel: "LAB02-2" -> [w715 w717]
                          frame #0 {
                            n469 = call "sub vi - defrag tdms v1.vi"("panel id"=w715) -> ("error out"=w714:errorcluster)  [unwired: 10 in]
                            n470 = local write "data file error"(w714) -> ()
                          }
                          frame #1 {
                            n471 = call "Save data file to network drive v1.vi"("panel id"=w717) -> ("network file save error"=w716:errorcluster)  [unwired: 9 in, 1 out]
                            n472 = local write "RESULT LAB02-2"(FALSE) -> ()
                            n473 = local write "data file error"(w716) -> ()
                          }
                        }
                        n474 = Bundle(cluster=w713, "STATUS"="STOP") -> (w711:T4)  [unwired: 2 in]
                        n475 = local write "DISP LAB02-2"(w711) -> ()
                      }
                    }
                  }
                  frame True {
                    # "start new test and create test file"
                    n476 = stacked-sequence {
                      seq-local: [w725 _ _ _ _] -> [_ w750 _ _ _]
                      tunnel: w724 -> [w730 _ _ _ _]
                      tunnel: w723 -> [w727 _ _ _ _]
                      tunnel: w722 -> [w740 _ _ _ _]
                      tunnel: w721 -> [w733 _ _ _ _]
                      tunnel: w720 -> [w728 _ _ _ _]
                      tunnel: [_ w744 _ _ _] -> w719
                      frame #0 {
                        w726 = "\\"
                        n477 = local read "SET LAB02-2"() -> (w735:T5)
                        n478 = case shown="\"CYCLE TEST\"" w740 {
                          tunnel: ["L02-2-CHART TEST-" "L02-2-CYCLE TEST-" "L02-2-T-RISE TEST-"] -> w736
                          frame "CHART TEST", Default {
                          }
                          frame "CYCLE TEST" {
                          }
                          frame "T-RISE TEST" {
                          }
                        }
                        n479 = Unbundle(w735) -> ("DESCRIPTION"=w734:string)  [unwired: 4 out]
                        n480 = Concatenate Strings(w730, "\\", w728, w726, w727, w726) -> (w737:string)
                        n481 = String To Path(string=w737) -> (path=w739:path)
                        n482 = Concatenate Strings(w737, w736, w734, "-", w733, ".tdms") -> (w725:string)
                        n483 = Create Folder(path (use dialog)=w739) -> (error out=w738:errorcluster)  [unwired: 2 in, 2 out]
                        n484 = global write "Global 1.vi" "LAB02-2 FILE"(w725) -> ()
                        n485 = call <vilib>:"Clear Errors.vi"("error in (no error)"=w738) -> ()  [unwired: 6 in, 1 out]
                      }
                      frame #1 {
                        n486 = String To Path(string=w750) -> (path=w745:path)
                        n487 = TDMS Open(5:FALSE, 6:FALSE, 10:T17."create or replace" ("operation (0:open)"), 11:w745) -> (0:w744:errorcluster, 3:→"TDMS LAB02-2":refnum<k34>)  [unwired: 3 in]
                      }
                      frame #2 {
                        n488 = local read "SET LAB02-2"() -> (w756:T5)
                        n489 = local read "TDMS LAB02-2"() -> (w767:refnum<k34>)
                        n490 = Build Array("Testers Name", "Description", "Set Test Cycles", "T-Rise minutes", "T-Rise Deg C") -> (w757:string[])
                        n491 = Unbundle(w756) -> ("NAME"=w755:string, "DESCRIPTION"=w754:string, "CYCLES"=w753:dbl, "T-RISE mins"=w752:dbl, "T-RISE deg C"=w751:dbl)
                        n492 = Number To Decimal String(number=w753) -> (decimal integer string=w766:string)  [unwired: 1 in]
                        n493 = Number To Decimal String(number=w752) -> (decimal integer string=w765:string)  [unwired: 1 in]
                        n494 = Number To Decimal String(number=w751) -> (decimal integer string=w764:string)  [unwired: 1 in]
                        n495 = Build Array(w755, w754, w766, w765, w764) -> (w763:string[])
                        n496 = TDMS Set Properties(5:w763, 7:w757, 11:w767) -> ()  [unwired: 3 in, 4 out]
                      }
                      frame #3 {
                        w769 = 0.0
                        n497 = local read "DISP LAB02-2"() -> (w771:T4)
                        n498 = Bundle(cluster=w771, "CYCLE"=w769, "MINS"=w769, "STATUS"="RUN") -> (w770:T4)
                        n499 = local write "DISP LAB02-2"(w770) -> ()
                      }
                      frame #4 {
                        n500 = local read "SIG LAB02-2"() -> (w774:T2)
                        n501 = local read "TEMP START LAB02-2"() -> (w776:cluster{"TL":dbl, "TN":dbl})
                        n502 = Unbundle(w774) -> ("Tmp Live"=w773:dbl, "Tmp Neut"=w772:dbl)  [unwired: 3 out]
                        n503 = Bundle(cluster=w776, "TL"=w773, "TN"=w772) -> (w775:cluster{"TL":dbl, "TN":dbl})
                        n504 = local write "TEMP START LAB02-2"(w775) -> ()
                      }
                    }
                  }
                }
              }
              event "RUN LAB03-1": Value Change {
                n505 = event-data() -> ("NewVal"=w777:bool)  [unwired: 1 in, 5 out]
                n506 = local write "run lab03-1"(w777) -> ()
                n507 = case shown="True" w777 {
                  tunnel: w783 -> [_ w816]
                  tunnel: w782 -> [_ w815]
                  tunnel: w780 -> [w785 w814]
                  tunnel: w781 -> [_ w813]
                  tunnel: w779 -> [_ w812]
                  tunnel: [w784 w811] -> w778
                  frame False {
                    # "stop test"
                    n508 = stacked-sequence {
                      tunnel: w785 -> [w794 _]
                      tunnel: [w786 _] -> w784
                      frame #0 {
                        n509 = local read "DISP LAB03-1"() -> (w793:T4)
                        n510 = Unbundle(w793) -> ("CYCLE"=w791:dbl, "MINS"=w792:dbl)  [unwired: 1 out]
                        n511 = case shown="\"CYCLE TEST\"" w794 {
                          tunnel: w792 -> [_ _ w801]
                          tunnel: w791 -> [w799 w800 _]
                          tunnel: [w799 w800 w801] -> w790
                          frame "CHART TEST", Default {
                          }
                          frame "CYCLE TEST" {
                          }
                          frame "T-RISE TEST" {
                          }
                        }
                        n512 = local read "TDMS LAB03-1"() -> (w798:refnum<k34>)
                        n513 = Build Array("STOPPED") -> (w795:string[])
                        n514 = Build Array(w790) -> (w789:dbl[])
                        n515 = TDMS Write(0:w798, 5:"TEST RESULT", 7:w795, 9:w789) -> (4:w787:refnum<k34>, 15:w788:errorcluster)  [unwired: 2 in, 2 out]
                        n516 = TDMS Close(8:w788, 11:w787) -> (0:w786:errorcluster)  [unwired: 1 out]
                      }
                      frame #1 {
                        n517 = local read "DISP LAB03-1"() -> (w805:T4)
                        n518 = stacked-sequence {
                          tunnel: "LAB03-1" -> [w807 w809]
                          frame #0 {
                            n519 = call "sub vi - defrag tdms v1.vi"("panel id"=w807) -> ("error out"=w806:errorcluster)  [unwired: 10 in]
                            n520 = local write "data file error"(w806) -> ()
                          }
                          frame #1 {
                            n521 = call "Save data file to network drive v1.vi"("panel id"=w809) -> ("network file save error"=w808:errorcluster)  [unwired: 9 in, 1 out]
                            n522 = local write "RESULT LAB03-1"(FALSE) -> ()
                            n523 = local write "data file error"(w808) -> ()
                          }
                        }
                        n524 = Bundle(cluster=w805, "STATUS"="STOP") -> (w803:T4)  [unwired: 2 in]
                        n525 = local write "DISP LAB03-1"(w803) -> ()
                      }
                    }
                  }
                  frame True {
                    # "start new test and create test file"
                    n526 = stacked-sequence {
                      seq-local: [w817 _ _ _ _] -> [_ w842 _ _ _]
                      tunnel: w816 -> [w822 _ _ _ _]
                      tunnel: w815 -> [w819 _ _ _ _]
                      tunnel: w814 -> [w832 _ _ _ _]
                      tunnel: w813 -> [w825 _ _ _ _]
                      tunnel: w812 -> [w820 _ _ _ _]
                      tunnel: [_ w836 _ _ _] -> w811
                      frame #0 {
                        w818 = "\\"
                        n527 = local read "SET LAB03-1"() -> (w827:T5)
                        n528 = case shown="\"T-RISE TEST\"" w832 {
                          tunnel: ["L03-1-CHART TEST-" "L03-1-CYCLE TEST-" "L03-1-T-RISE TEST-"] -> w828
                          frame "CHART TEST", Default {
                          }
                          frame "CYCLE TEST" {
                          }
                          frame "T-RISE TEST" {
                          }
                        }
                        n529 = Unbundle(w827) -> ("DESCRIPTION"=w826:string)  [unwired: 4 out]
                        n530 = Concatenate Strings(w822, "\\", w820, w818, w819, w818) -> (w829:string)
                        n531 = String To Path(string=w829) -> (path=w831:path)
                        n532 = Concatenate Strings(w829, w828, w826, "-", w825, ".tdms") -> (w817:string)
                        n533 = Create Folder(path (use dialog)=w831) -> (error out=w830:errorcluster)  [unwired: 2 in, 2 out]
                        n534 = global write "Global 1.vi" "LAB03-1 FILE"(w817) -> ()
                        n535 = call <vilib>:"Clear Errors.vi"("error in (no error)"=w830) -> ()  [unwired: 6 in, 1 out]
                      }
                      frame #1 {
                        n536 = String To Path(string=w842) -> (path=w837:path)
                        n537 = TDMS Open(5:FALSE, 6:FALSE, 10:T17."create or replace" ("operation (0:open)"), 11:w837) -> (0:w836:errorcluster, 3:→"TDMS LAB03-1":refnum<k34>)  [unwired: 3 in]
                      }
                      frame #2 {
                        n538 = local read "SET LAB03-1"() -> (w848:T5)
                        n539 = local read "TDMS LAB03-1"() -> (w859:refnum<k34>)
                        n540 = Build Array("Testers Name", "Description", "Set Test Cycles", "T-Rise minutes", "T-Rise Deg C") -> (w849:string[])
                        n541 = Unbundle(w848) -> ("NAME"=w847:string, "DESCRIPTION"=w846:string, "CYCLES"=w845:dbl, "T-RISE mins"=w844:dbl, "T-RISE deg C"=w843:dbl)
                        n542 = Number To Decimal String(number=w845) -> (decimal integer string=w858:string)  [unwired: 1 in]
                        n543 = Number To Decimal String(number=w844) -> (decimal integer string=w857:string)  [unwired: 1 in]
                        n544 = Number To Decimal String(number=w843) -> (decimal integer string=w856:string)  [unwired: 1 in]
                        n545 = Build Array(w847, w846, w858, w857, w856) -> (w855:string[])
                        n546 = TDMS Set Properties(5:w855, 7:w849, 11:w859) -> ()  [unwired: 3 in, 4 out]
                      }
                      frame #3 {
                        w861 = 0.0
                        n547 = local read "DISP LAB03-1"() -> (w863:T4)
                        n548 = Bundle(cluster=w863, "CYCLE"=w861, "MINS"=w861, "STATUS"="RUN") -> (w862:T4)
                        n549 = local write "DISP LAB03-1"(w862) -> ()
                      }
                      frame #4 {
                        n550 = local read "SIG LAB03-1"() -> (w866:T2)
                        n551 = local read "TEMP START LAB03-1"() -> (w868:cluster{"TL":dbl, "TN":dbl})
                        n552 = Unbundle(w866) -> ("Tmp Live"=w865:dbl, "Tmp Neut"=w864:dbl)  [unwired: 3 out]
                        n553 = Bundle(cluster=w868, "TL"=w865, "TN"=w864) -> (w867:cluster{"TL":dbl, "TN":dbl})
                        n554 = local write "TEMP START LAB03-1"(w867) -> ()
                      }
                    }
                  }
                }
              }
              event "RUN LAB03-2": Value Change {
                n555 = event-data() -> ("NewVal"=w869:bool)  [unwired: 1 in, 5 out]
                n556 = local write "run lab03-2"(w869) -> ()
                n557 = case shown="True" w869 {
                  tunnel: w875 -> [_ w908]
                  tunnel: w874 -> [_ w907]
                  tunnel: w872 -> [w877 w906]
                  tunnel: w873 -> [_ w905]
                  tunnel: w871 -> [_ w904]
                  tunnel: [w876 w903] -> w870
                  frame False {
                    # "stop test"
                    n558 = stacked-sequence {
                      tunnel: w877 -> [w886 _]
                      tunnel: [w878 _] -> w876
                      frame #0 {
                        n559 = local read "DISP LAB03-2"() -> (w885:T4)
                        n560 = Unbundle(w885) -> ("CYCLE"=w883:dbl, "MINS"=w884:dbl)  [unwired: 1 out]
                        n561 = case shown="\"CYCLE TEST\"" w886 {
                          tunnel: w884 -> [_ _ w893]
                          tunnel: w883 -> [w891 w892 _]
                          tunnel: [w891 w892 w893] -> w882
                          frame "CHART TEST", Default {
                          }
                          frame "CYCLE TEST" {
                          }
                          frame "T-RISE TEST" {
                          }
                        }
                        n562 = local read "TDMS LAB03-2"() -> (w890:refnum<k34>)
                        n563 = Build Array("STOPPED") -> (w887:string[])
                        n564 = Build Array(w882) -> (w881:dbl[])
                        n565 = TDMS Write(0:w890, 5:"TEST RESULT", 7:w887, 9:w881) -> (4:w879:refnum<k34>, 15:w880:errorcluster)  [unwired: 2 in, 2 out]
                        n566 = TDMS Close(8:w880, 11:w879) -> (0:w878:errorcluster)  [unwired: 1 out]
                      }
                      frame #1 {
                        n567 = local read "DISP LAB03-2"() -> (w897:T4)
                        n568 = stacked-sequence {
                          tunnel: "LAB03-2" -> [w899 w901]
                          frame #0 {
                            n569 = call "sub vi - defrag tdms v1.vi"("panel id"=w899) -> ("error out"=w898:errorcluster)  [unwired: 10 in]
                            n570 = local write "data file error"(w898) -> ()
                          }
                          frame #1 {
                            n571 = call "Save data file to network drive v1.vi"("panel id"=w901) -> ("network file save error"=w900:errorcluster)  [unwired: 9 in, 1 out]
                            n572 = local write "RESULT LAB03-2"(FALSE) -> ()
                            n573 = local write "data file error"(w900) -> ()
                          }
                        }
                        n574 = Bundle(cluster=w897, "STATUS"="STOP") -> (w895:T4)  [unwired: 2 in]
                        n575 = local write "DISP LAB03-2"(w895) -> ()
                      }
                    }
                  }
                  frame True {
                    # "start new test and create test file"
                    n576 = stacked-sequence {
                      seq-local: [w909 _ _ _ _] -> [_ w934 _ _ _]
                      tunnel: w908 -> [w914 _ _ _ _]
                      tunnel: w907 -> [w911 _ _ _ _]
                      tunnel: w906 -> [w924 _ _ _ _]
                      tunnel: w905 -> [w917 _ _ _ _]
                      tunnel: w904 -> [w912 _ _ _ _]
                      tunnel: [_ w928 _ _ _] -> w903
                      frame #0 {
                        w910 = "\\"
                        n577 = local read "SET LAB03-2"() -> (w919:T5)
                        n578 = case shown="\"T-RISE TEST\"" w924 {
                          tunnel: ["L03-2-CHART TEST-" "L03-2-CYCLE TEST-" "L03-2-T-RISE TEST-"] -> w920
                          frame "CHART TEST", Default {
                          }
                          frame "CYCLE TEST" {
                          }
                          frame "T-RISE TEST" {
                          }
                        }
                        n579 = Unbundle(w919) -> ("DESCRIPTION"=w918:string)  [unwired: 4 out]
                        n580 = Concatenate Strings(w914, "\\", w912, w910, w911, w910) -> (w921:string)
                        n581 = String To Path(string=w921) -> (path=w923:path)
                        n582 = Concatenate Strings(w921, w920, w918, "-", w917, ".tdms") -> (w909:string)
                        n583 = Create Folder(path (use dialog)=w923) -> (error out=w922:errorcluster)  [unwired: 2 in, 2 out]
                        n584 = global write "Global 1.vi" "LAB03-2 FILE"(w909) -> ()
                        n585 = call <vilib>:"Clear Errors.vi"("error in (no error)"=w922) -> ()  [unwired: 6 in, 1 out]
                      }
                      frame #1 {
                        n586 = String To Path(string=w934) -> (path=w929:path)
                        n587 = TDMS Open(5:FALSE, 6:FALSE, 10:T17."create or replace" ("operation (0:open)"), 11:w929) -> (0:w928:errorcluster, 3:→"TDMS LAB03-2":refnum<k34>)  [unwired: 3 in]
                      }
                      frame #2 {
                        n588 = local read "SET LAB03-2"() -> (w940:T5)
                        n589 = local read "TDMS LAB03-2"() -> (w951:refnum<k34>)
                        n590 = Build Array("Testers Name", "Description", "Set Test Cycles", "T-Rise minutes", "T-Rise Deg C") -> (w941:string[])
                        n591 = Unbundle(w940) -> ("NAME"=w939:string, "DESCRIPTION"=w938:string, "CYCLES"=w937:dbl, "T-RISE mins"=w936:dbl, "T-RISE deg C"=w935:dbl)
                        n592 = Number To Decimal String(number=w937) -> (decimal integer string=w950:string)  [unwired: 1 in]
                        n593 = Number To Decimal String(number=w936) -> (decimal integer string=w949:string)  [unwired: 1 in]
                        n594 = Number To Decimal String(number=w935) -> (decimal integer string=w948:string)  [unwired: 1 in]
                        n595 = Build Array(w939, w938, w950, w949, w948) -> (w947:string[])
                        n596 = TDMS Set Properties(5:w947, 7:w941, 11:w951) -> ()  [unwired: 3 in, 4 out]
                      }
                      frame #3 {
                        w953 = 0.0
                        n597 = local read "DISP LAB03-2"() -> (w955:T4)
                        n598 = Bundle(cluster=w955, "CYCLE"=w953, "MINS"=w953, "STATUS"="RUN") -> (w954:T4)
                        n599 = local write "DISP LAB03-2"(w954) -> ()
                      }
                      frame #4 {
                        n600 = local read "SIG LAB03-2"() -> (w958:T2)
                        n601 = local read "TEMP START LAB03-2"() -> (w960:cluster{"TL":dbl, "TN":dbl})
                        n602 = Unbundle(w958) -> ("Tmp Live"=w957:dbl, "Tmp Neut"=w956:dbl)  [unwired: 3 out]
                        n603 = Bundle(cluster=w960, "TL"=w957, "TN"=w956) -> (w959:cluster{"TL":dbl, "TN":dbl})
                        n604 = local write "TEMP START LAB03-2"(w959) -> ()
                      }
                    }
                  }
                }
              }
              event "RUN LAB04-1": Value Change {
                n605 = event-data() -> ("NewVal"=w961:bool)  [unwired: 1 in, 5 out]
                n606 = local write "run lab04-1"(w961) -> ()
                n607 = case shown="True" w961 {
                  tunnel: w967 -> [_ w1000]
                  tunnel: w966 -> [_ w999]
                  tunnel: w964 -> [w969 w998]
                  tunnel: w965 -> [_ w997]
                  tunnel: w963 -> [_ w996]
                  tunnel: [w968 w995] -> w962
                  frame False {
                    # "stop test"
                    n608 = stacked-sequence {
                      tunnel: w969 -> [w978 _]
                      tunnel: [w970 _] -> w968
                      frame #0 {
                        n609 = local read "DISP LAB04-1"() -> (w977:T4)
                        n610 = Unbundle(w977) -> ("CYCLE"=w975:dbl, "MINS"=w976:dbl)  [unwired: 1 out]
                        n611 = case shown="\"CYCLE TEST\"" w978 {
                          tunnel: w976 -> [_ _ w985]
                          tunnel: w975 -> [w983 w984 _]
                          tunnel: [w983 w984 w985] -> w974
                          frame "CHART TEST", Default {
                          }
                          frame "CYCLE TEST" {
                          }
                          frame "T-RISE TEST" {
                          }
                        }
                        n612 = local read "TDMS LAB04-1"() -> (w982:refnum<k34>)
                        n613 = Build Array("STOPPED") -> (w979:string[])
                        n614 = Build Array(w974) -> (w973:dbl[])
                        n615 = TDMS Write(0:w982, 5:"TEST RESULT", 7:w979, 9:w973) -> (4:w971:refnum<k34>, 15:w972:errorcluster)  [unwired: 2 in, 2 out]
                        n616 = TDMS Close(8:w972, 11:w971) -> (0:w970:errorcluster)  [unwired: 1 out]
                      }
                      frame #1 {
                        n617 = local read "DISP LAB04-1"() -> (w989:T4)
                        n618 = stacked-sequence {
                          tunnel: "LAB04-1" -> [w991 w993]
                          frame #0 {
                            n619 = call "sub vi - defrag tdms v1.vi"("panel id"=w991) -> ("error out"=w990:errorcluster)  [unwired: 10 in]
                            n620 = local write "data file error"(w990) -> ()
                          }
                          frame #1 {
                            n621 = call "Save data file to network drive v1.vi"("panel id"=w993) -> ("network file save error"=w992:errorcluster)  [unwired: 9 in, 1 out]
                            n622 = local write "RESULT LAB04-1"(FALSE) -> ()
                            n623 = local write "data file error"(w992) -> ()
                          }
                        }
                        n624 = Bundle(cluster=w989, "STATUS"="STOP") -> (w987:T4)  [unwired: 2 in]
                        n625 = local write "DISP LAB04-1"(w987) -> ()
                      }
                    }
                  }
                  frame True {
                    # "start new test and create test file"
                    n626 = stacked-sequence {
                      seq-local: [w1001 _ _ _ _] -> [_ w1026 _ _ _]
                      tunnel: w1000 -> [w1006 _ _ _ _]
                      tunnel: w999 -> [w1002 _ _ _ _]
                      tunnel: w998 -> [w1016 _ _ _ _]
                      tunnel: w997 -> [w1009 _ _ _ _]
                      tunnel: w996 -> [w1004 _ _ _ _]
                      tunnel: [_ w1020 _ _ _] -> w995
                      frame #0 {
                        w1003 = "\\"
                        n627 = local read "SET LAB04-1"() -> (w1011:T5)
                        n628 = case shown="\"CYCLE TEST\"" w1016 {
                          tunnel: ["L04-1-CHART TEST-" "L04-1-CYCLE TEST-" "L04-1-T-RISE TEST-"] -> w1012
                          frame "CHART TEST", Default {
                          }
                          frame "CYCLE TEST" {
                          }
                          frame "T-RISE TEST" {
                          }
                        }
                        n629 = Unbundle(w1011) -> ("DESCRIPTION"=w1010:string)  [unwired: 4 out]
                        n630 = Concatenate Strings(w1006, "\\", w1004, w1003, w1002, w1003) -> (w1013:string)
                        n631 = String To Path(string=w1013) -> (path=w1015:path)
                        n632 = Concatenate Strings(w1013, w1012, w1010, "-", w1009, ".tdms") -> (w1001:string)
                        n633 = Create Folder(path (use dialog)=w1015) -> (error out=w1014:errorcluster)  [unwired: 2 in, 2 out]
                        n634 = global write "Global 1.vi" "LAB04-1 FILE"(w1001) -> ()
                        n635 = call <vilib>:"Clear Errors.vi"("error in (no error)"=w1014) -> ()  [unwired: 6 in, 1 out]
                      }
                      frame #1 {
                        n636 = String To Path(string=w1026) -> (path=w1021:path)
                        n637 = TDMS Open(5:FALSE, 6:FALSE, 10:T17."create or replace" ("operation (0:open)"), 11:w1021) -> (0:w1020:errorcluster, 3:→"TDMS LAB04-1":refnum<k34>)  [unwired: 3 in]
                      }
                      frame #2 {
                        n638 = local read "SET LAB04-1"() -> (w1032:T5)
                        n639 = local read "TDMS LAB04-1"() -> (w1043:refnum<k34>)
                        n640 = Build Array("Testers Name", "Description", "Set Test Cycles", "T-Rise minutes", "T-Rise Deg C") -> (w1033:string[])
                        n641 = Unbundle(w1032) -> ("NAME"=w1031:string, "DESCRIPTION"=w1030:string, "CYCLES"=w1029:dbl, "T-RISE mins"=w1028:dbl, "T-RISE deg C"=w1027:dbl)
                        n642 = Number To Decimal String(number=w1029) -> (decimal integer string=w1042:string)  [unwired: 1 in]
                        n643 = Number To Decimal String(number=w1028) -> (decimal integer string=w1041:string)  [unwired: 1 in]
                        n644 = Number To Decimal String(number=w1027) -> (decimal integer string=w1040:string)  [unwired: 1 in]
                        n645 = Build Array(w1031, w1030, w1042, w1041, w1040) -> (w1039:string[])
                        n646 = TDMS Set Properties(5:w1039, 7:w1033, 11:w1043) -> ()  [unwired: 3 in, 4 out]
                      }
                      frame #3 {
                        w1045 = 0.0
                        n647 = local read "DISP LAB04-1"() -> (w1047:T4)
                        n648 = Bundle(cluster=w1047, "CYCLE"=w1045, "MINS"=w1045, "STATUS"="RUN") -> (w1046:T4)
                        n649 = local write "DISP LAB04-1"(w1046) -> ()
                      }
                      frame #4 {
                        n650 = local read "SIG LAB04-1"() -> (w1050:T2)
                        n651 = local read "TEMP START LAB04-1"() -> (w1052:cluster{"TL":dbl, "TN":dbl})
                        n652 = Unbundle(w1050) -> ("Tmp Live"=w1049:dbl, "Tmp Neut"=w1048:dbl)  [unwired: 3 out]
                        n653 = Bundle(cluster=w1052, "TL"=w1049, "TN"=w1048) -> (w1051:cluster{"TL":dbl, "TN":dbl})
                        n654 = local write "TEMP START LAB04-1"(w1051) -> ()
                      }
                    }
                  }
                }
              }
              event "RUN LAB04-2": Value Change {
                n655 = event-data() -> ("NewVal"=w1053:bool)  [unwired: 1 in, 5 out]
                n656 = local write "run lab04-2"(w1053) -> ()
                n657 = case shown="True" w1053 {
                  tunnel: w1059 -> [_ w1092]
                  tunnel: w1058 -> [_ w1091]
                  tunnel: w1056 -> [w1061 w1090]
                  tunnel: w1057 -> [_ w1089]
                  tunnel: w1055 -> [_ w1088]
                  tunnel: [w1060 w1087] -> w1054
                  frame False {
                    # "stop test"
                    n658 = stacked-sequence {
                      tunnel: w1061 -> [w1070 _]
                      tunnel: [w1062 _] -> w1060
                      frame #0 {
                        n659 = local read "DISP LAB04-2"() -> (w1069:T4)
                        n660 = Unbundle(w1069) -> ("CYCLE"=w1067:dbl, "MINS"=w1068:dbl)  [unwired: 1 out]
                        n661 = case shown="\"CYCLE TEST\"" w1070 {
                          tunnel: w1068 -> [_ _ w1077]
                          tunnel: w1067 -> [w1075 w1076 _]
                          tunnel: [w1075 w1076 w1077] -> w1066
                          frame "CHART TEST", Default {
                          }
                          frame "CYCLE TEST" {
                          }
                          frame "T-RISE TEST" {
                          }
                        }
                        n662 = local read "TDMS LAB04-2"() -> (w1074:refnum<k34>)
                        n663 = Build Array("STOPPED") -> (w1071:string[])
                        n664 = Build Array(w1066) -> (w1065:dbl[])
                        n665 = TDMS Write(0:w1074, 5:"TEST RESULT", 7:w1071, 9:w1065) -> (4:w1063:refnum<k34>, 15:w1064:errorcluster)  [unwired: 2 in, 2 out]
                        n666 = TDMS Close(8:w1064, 11:w1063) -> (0:w1062:errorcluster)  [unwired: 1 out]
                      }
                      frame #1 {
                        n667 = local read "DISP LAB04-2"() -> (w1081:T4)
                        n668 = stacked-sequence {
                          tunnel: "LAB04-2" -> [w1083 w1085]
                          frame #0 {
                            n669 = call "sub vi - defrag tdms v1.vi"("panel id"=w1083) -> ("error out"=w1082:errorcluster)  [unwired: 10 in]
                            n670 = local write "data file error"(w1082) -> ()
                          }
                          frame #1 {
                            n671 = call "Save data file to network drive v1.vi"("panel id"=w1085) -> ("network file save error"=w1084:errorcluster)  [unwired: 9 in, 1 out]
                            n672 = local write "RESULT LAB04-2"(FALSE) -> ()
                            n673 = local write "data file error"(w1084) -> ()
                          }
                        }
                        n674 = Bundle(cluster=w1081, "STATUS"="STOP") -> (w1079:T4)  [unwired: 2 in]
                        n675 = local write "DISP LAB04-2"(w1079) -> ()
                      }
                    }
                  }
                  frame True {
                    # "start new test and create test file"
                    n676 = stacked-sequence {
                      seq-local: [w1093 _ _ _ _] -> [_ w1118 _ _ _]
                      tunnel: w1092 -> [w1098 _ _ _ _]
                      tunnel: w1091 -> [w1094 _ _ _ _]
                      tunnel: w1090 -> [w1108 _ _ _ _]
                      tunnel: w1089 -> [w1101 _ _ _ _]
                      tunnel: w1088 -> [w1096 _ _ _ _]
                      tunnel: [_ w1112 _ _ _] -> w1087
                      frame #0 {
                        w1095 = "\\"
                        n677 = local read "SET LAB04-2"() -> (w1103:T5)
                        n678 = case shown="\"CHART TEST\", Default" w1108 {
                          tunnel: ["L04-2-CHART TEST-" "L04-2-CYCLE TEST-" "L04-2-T-RISE TEST-"] -> w1104
                          frame "CHART TEST", Default {
                          }
                          frame "CYCLE TEST" {
                          }
                          frame "T-RISE TEST" {
                          }
                        }
                        n679 = Unbundle(w1103) -> ("DESCRIPTION"=w1102:string)  [unwired: 4 out]
                        n680 = Concatenate Strings(w1098, "\\", w1096, w1095, w1094, w1095) -> (w1105:string)
                        n681 = String To Path(string=w1105) -> (path=w1107:path)
                        n682 = Concatenate Strings(w1105, w1104, w1102, "-", w1101, ".tdms") -> (w1093:string)
                        n683 = Create Folder(path (use dialog)=w1107) -> (error out=w1106:errorcluster)  [unwired: 2 in, 2 out]
                        n684 = global write "Global 1.vi" "LAB04-2 FILE"(w1093) -> ()
                        n685 = call <vilib>:"Clear Errors.vi"("error in (no error)"=w1106) -> ()  [unwired: 6 in, 1 out]
                      }
                      frame #1 {
                        n686 = String To Path(string=w1118) -> (path=w1113:path)
                        n687 = TDMS Open(5:FALSE, 6:FALSE, 10:T17."create or replace" ("operation (0:open)"), 11:w1113) -> (0:w1112:errorcluster, 3:→"TDMS LAB04-2":refnum<k34>)  [unwired: 3 in]
                      }
                      frame #2 {
                        n688 = local read "SET LAB04-2"() -> (w1124:T5)
                        n689 = local read "TDMS LAB04-2"() -> (w1135:refnum<k34>)
                        n690 = Build Array("Testers Name", "Description", "Set Test Cycles", "T-Rise minutes", "T-Rise Deg C") -> (w1125:string[])
                        n691 = Unbundle(w1124) -> ("NAME"=w1123:string, "DESCRIPTION"=w1122:string, "CYCLES"=w1121:dbl, "T-RISE mins"=w1120:dbl, "T-RISE deg C"=w1119:dbl)
                        n692 = Number To Decimal String(number=w1121) -> (decimal integer string=w1134:string)  [unwired: 1 in]
                        n693 = Number To Decimal String(number=w1120) -> (decimal integer string=w1133:string)  [unwired: 1 in]
                        n694 = Number To Decimal String(number=w1119) -> (decimal integer string=w1132:string)  [unwired: 1 in]
                        n695 = Build Array(w1123, w1122, w1134, w1133, w1132) -> (w1131:string[])
                        n696 = TDMS Set Properties(5:w1131, 7:w1125, 11:w1135) -> ()  [unwired: 3 in, 4 out]
                      }
                      frame #3 {
                        w1137 = 0.0
                        n697 = local read "DISP LAB04-2"() -> (w1139:T4)
                        n698 = Bundle(cluster=w1139, "CYCLE"=w1137, "MINS"=w1137, "STATUS"="RUN") -> (w1138:T4)
                        n699 = local write "DISP LAB04-2"(w1138) -> ()
                      }
                      frame #4 {
                        n700 = local read "SIG LAB04-2"() -> (w1142:T2)
                        n701 = local read "TEMP START LAB04-2"() -> (w1144:cluster{"TL":dbl, "TN":dbl})
                        n702 = Unbundle(w1142) -> ("Tmp Live"=w1141:dbl, "Tmp Neut"=w1140:dbl)  [unwired: 3 out]
                        n703 = Bundle(cluster=w1144, "TL"=w1141, "TN"=w1140) -> (w1143:cluster{"TL":dbl, "TN":dbl})
                        n704 = local write "TEMP START LAB04-2"(w1143) -> ()
                      }
                    }
                  }
                }
              }
              event "RUN LAB05-1": Value Change {
                n705 = event-data() -> ("NewVal"=w1145:bool)  [unwired: 1 in, 5 out]
                n706 = local write "run lab05-1"(w1145) -> ()
                n707 = case shown="True" w1145 {
                  tunnel: w1151 -> [_ w1184]
                  tunnel: w1150 -> [_ w1183]
                  tunnel: w1148 -> [w1153 w1182]
                  tunnel: w1149 -> [_ w1181]
                  tunnel: w1147 -> [_ w1180]
                  tunnel: [w1152 w1179] -> w1146
                  frame False {
                    # "stop test"
                    n708 = stacked-sequence {
                      tunnel: w1153 -> [w1162 _]
                      tunnel: [w1154 _] -> w1152
                      frame #0 {
                        n709 = local read "DISP LAB05-1"() -> (w1161:T4)
                        n710 = Unbundle(w1161) -> ("CYCLE"=w1159:dbl, "MINS"=w1160:dbl)  [unwired: 1 out]
                        n711 = case shown="\"CYCLE TEST\"" w1162 {
                          tunnel: w1160 -> [_ _ w1169]
                          tunnel: w1159 -> [w1167 w1168 _]
                          tunnel: [w1167 w1168 w1169] -> w1158
                          frame "CHART TEST", Default {
                          }
                          frame "CYCLE TEST" {
                          }
                          frame "T-RISE TEST" {
                          }
                        }
                        n712 = local read "TDMS LAB05-1"() -> (w1166:refnum<k34>)
                        n713 = Build Array("STOPPED") -> (w1163:string[])
                        n714 = Build Array(w1158) -> (w1157:dbl[])
                        n715 = TDMS Write(0:w1166, 5:"TEST RESULT", 7:w1163, 9:w1157) -> (4:w1155:refnum<k34>, 15:w1156:errorcluster)  [unwired: 2 in, 2 out]
                        n716 = TDMS Close(8:w1156, 11:w1155) -> (0:w1154:errorcluster)  [unwired: 1 out]
                      }
                      frame #1 {
                        n717 = local read "DISP LAB05-1"() -> (w1173:T4)
                        n718 = stacked-sequence {
                          tunnel: "LAB05-1" -> [w1175 w1177]
                          frame #0 {
                            n719 = call "sub vi - defrag tdms v1.vi"("panel id"=w1175) -> ("error out"=w1174:errorcluster)  [unwired: 10 in]
                            n720 = local write "data file error"(w1174) -> ()
                          }
                          frame #1 {
                            n721 = call "Save data file to network drive v1.vi"("panel id"=w1177) -> ("network file save error"=w1176:errorcluster)  [unwired: 9 in, 1 out]
                            n722 = local write "RESULT LAB05-1"(FALSE) -> ()
                            n723 = local write "data file error"(w1176) -> ()
                          }
                        }
                        n724 = Bundle(cluster=w1173, "STATUS"="STOP") -> (w1171:T4)  [unwired: 2 in]
                        n725 = local write "DISP LAB05-1"(w1171) -> ()
                      }
                    }
                  }
                  frame True {
                    # "start new test and create test file"
                    n726 = stacked-sequence {
                      seq-local: [w1185 _ _ _ _] -> [_ w1210 _ _ _]
                      tunnel: w1184 -> [w1190 _ _ _ _]
                      tunnel: w1183 -> [w1186 _ _ _ _]
                      tunnel: w1182 -> [w1200 _ _ _ _]
                      tunnel: w1181 -> [w1193 _ _ _ _]
                      tunnel: w1180 -> [w1188 _ _ _ _]
                      tunnel: [_ w1204 _ _ _] -> w1179
                      frame #0 {
                        w1187 = "\\"
                        n727 = local read "SET LAB05-1"() -> (w1195:T5)
                        n728 = case shown="\"CYCLE TEST\"" w1200 {
                          tunnel: ["L05-1-CHART TEST-" "L05-1-CYCLE TEST-" "L05-1-T-RISE TEST-"] -> w1196
                          frame "CHART TEST", Default {
                          }
                          frame "CYCLE TEST" {
                          }
                          frame "T-RISE TEST" {
                          }
                        }
                        n729 = Unbundle(w1195) -> ("DESCRIPTION"=w1194:string)  [unwired: 4 out]
                        n730 = Concatenate Strings(w1190, "\\", w1188, w1187, w1186, w1187) -> (w1197:string)
                        n731 = String To Path(string=w1197) -> (path=w1199:path)
                        n732 = Concatenate Strings(w1197, w1196, w1194, "-", w1193, ".tdms") -> (w1185:string)
                        n733 = Create Folder(path (use dialog)=w1199) -> (error out=w1198:errorcluster)  [unwired: 2 in, 2 out]
                        n734 = global write "Global 1.vi" "LAB05-1 FILE"(w1185) -> ()
                        n735 = call <vilib>:"Clear Errors.vi"("error in (no error)"=w1198) -> ()  [unwired: 6 in, 1 out]
                      }
                      frame #1 {
                        n736 = String To Path(string=w1210) -> (path=w1205:path)
                        n737 = TDMS Open(5:FALSE, 6:FALSE, 10:T17."create or replace" ("operation (0:open)"), 11:w1205) -> (0:w1204:errorcluster, 3:→"TDMS LAB05-1":refnum<k34>)  [unwired: 3 in]
                      }
                      frame #2 {
                        n738 = local read "SET LAB05-1"() -> (w1216:T5)
                        n739 = local read "TDMS LAB05-1"() -> (w1227:refnum<k34>)
                        n740 = Build Array("Testers Name", "Description", "Set Test Cycles", "T-Rise minutes", "T-Rise Deg C") -> (w1217:string[])
                        n741 = Unbundle(w1216) -> ("NAME"=w1215:string, "DESCRIPTION"=w1214:string, "CYCLES"=w1213:dbl, "T-RISE mins"=w1212:dbl, "T-RISE deg C"=w1211:dbl)
                        n742 = Number To Decimal String(number=w1213) -> (decimal integer string=w1226:string)  [unwired: 1 in]
                        n743 = Number To Decimal String(number=w1212) -> (decimal integer string=w1225:string)  [unwired: 1 in]
                        n744 = Number To Decimal String(number=w1211) -> (decimal integer string=w1224:string)  [unwired: 1 in]
                        n745 = Build Array(w1215, w1214, w1226, w1225, w1224) -> (w1223:string[])
                        n746 = TDMS Set Properties(5:w1223, 7:w1217, 11:w1227) -> ()  [unwired: 3 in, 4 out]
                      }
                      frame #3 {
                        w1229 = 0.0
                        n747 = local read "DISP LAB05-1"() -> (w1231:T4)
                        n748 = Bundle(cluster=w1231, "CYCLE"=w1229, "MINS"=w1229, "STATUS"="RUN") -> (w1230:T4)
                        n749 = local write "DISP LAB05-1"(w1230) -> ()
                      }
                      frame #4 {
                        n750 = local read "SIG LAB05-1"() -> (w1234:T2)
                        n751 = local read "TEMP START LAB05-1"() -> (w1236:cluster{"TL":dbl, "TN":dbl})
                        n752 = Unbundle(w1234) -> ("Tmp Live"=w1233:dbl, "Tmp Neut"=w1232:dbl)  [unwired: 3 out]
                        n753 = Bundle(cluster=w1236, "TL"=w1233, "TN"=w1232) -> (w1235:cluster{"TL":dbl, "TN":dbl})
                        n754 = local write "TEMP START LAB05-1"(w1235) -> ()
                      }
                    }
                  }
                }
              }
              event "RUN LAB05-2": Value Change {
                n755 = event-data() -> ("NewVal"=w1237:bool)  [unwired: 1 in, 5 out]
                n756 = local write "run lab05-2"(w1237) -> ()
                n757 = case shown="True" w1237 {
                  tunnel: w1243 -> [_ w1276]
                  tunnel: w1242 -> [_ w1275]
                  tunnel: w1240 -> [w1245 w1274]
                  tunnel: w1241 -> [_ w1273]
                  tunnel: w1239 -> [_ w1272]
                  tunnel: [w1244 w1271] -> w1238
                  frame False {
                    # "stop test"
                    n758 = stacked-sequence {
                      tunnel: w1245 -> [w1254 _]
                      tunnel: [w1246 _] -> w1244
                      frame #0 {
                        n759 = local read "DISP LAB05-2"() -> (w1253:T4)
                        n760 = Unbundle(w1253) -> ("CYCLE"=w1251:dbl, "MINS"=w1252:dbl)  [unwired: 1 out]
                        n761 = case shown="\"CYCLE TEST\"" w1254 {
                          tunnel: w1252 -> [_ _ w1261]
                          tunnel: w1251 -> [w1259 w1260 _]
                          tunnel: [w1259 w1260 w1261] -> w1250
                          frame "CHART TEST", Default {
                          }
                          frame "CYCLE TEST" {
                          }
                          frame "T-RISE TEST" {
                          }
                        }
                        n762 = local read "TDMS LAB05-2"() -> (w1258:refnum<k34>)
                        n763 = Build Array("STOPPED") -> (w1255:string[])
                        n764 = Build Array(w1250) -> (w1249:dbl[])
                        n765 = TDMS Write(0:w1258, 5:"TEST RESULT", 7:w1255, 9:w1249) -> (4:w1247:refnum<k34>, 15:w1248:errorcluster)  [unwired: 2 in, 2 out]
                        n766 = TDMS Close(8:w1248, 11:w1247) -> (0:w1246:errorcluster)  [unwired: 1 out]
                      }
                      frame #1 {
                        n767 = local read "DISP LAB05-2"() -> (w1265:T4)
                        n768 = stacked-sequence {
                          tunnel: "LAB05-2" -> [w1267 w1269]
                          frame #0 {
                            n769 = call "sub vi - defrag tdms v1.vi"("panel id"=w1267) -> ("error out"=w1266:errorcluster)  [unwired: 10 in]
                            n770 = local write "data file error"(w1266) -> ()
                          }
                          frame #1 {
                            n771 = local write "RESULT LAB05-2"(FALSE) -> ()
                            n772 = call "Save data file to network drive v1.vi"("panel id"=w1269) -> ("network file save error"=w1268:errorcluster)  [unwired: 9 in, 1 out]
                            n773 = local write "data file error"(w1268) -> ()
                          }
                        }
                        n774 = Bundle(cluster=w1265, "STATUS"="STOP") -> (w1263:T4)  [unwired: 2 in]
                        n775 = local write "DISP LAB05-2"(w1263) -> ()
                      }
                    }
                  }
                  frame True {
                    # "start new test and create test file"
                    n776 = stacked-sequence {
                      seq-local: [w1277 _ _ _ _] -> [_ w1302 _ _ _]
                      tunnel: w1276 -> [w1282 _ _ _ _]
                      tunnel: w1275 -> [w1278 _ _ _ _]
                      tunnel: w1274 -> [w1292 _ _ _ _]
                      tunnel: w1273 -> [w1285 _ _ _ _]
                      tunnel: w1272 -> [w1280 _ _ _ _]
                      tunnel: [_ w1296 _ _ _] -> w1271
                      frame #0 {
                        w1279 = "\\"
                        n777 = local read "SET LAB05-2"() -> (w1287:T5)
                        n778 = case shown="\"CYCLE TEST\"" w1292 {
                          tunnel: ["L05-2-CHART TEST-" "L05-2-CYCLE TEST-" "L05-2-T-RISE TEST-"] -> w1288
                          frame "CHART TEST", Default {
                          }
                          frame "CYCLE TEST" {
                          }
                          frame "T-RISE TEST" {
                          }
                        }
                        n779 = Unbundle(w1287) -> ("DESCRIPTION"=w1286:string)  [unwired: 4 out]
                        n780 = Concatenate Strings(w1282, "\\", w1280, w1279, w1278, w1279) -> (w1289:string)
                        n781 = String To Path(string=w1289) -> (path=w1291:path)
                        n782 = Concatenate Strings(w1289, w1288, w1286, "-", w1285, ".tdms") -> (w1277:string)
                        n783 = Create Folder(path (use dialog)=w1291) -> (error out=w1290:errorcluster)  [unwired: 2 in, 2 out]
                        n784 = global write "Global 1.vi" "LAB05-2 FILE"(w1277) -> ()
                        n785 = call <vilib>:"Clear Errors.vi"("error in (no error)"=w1290) -> ()  [unwired: 6 in, 1 out]
                      }
                      frame #1 {
                        n786 = String To Path(string=w1302) -> (path=w1297:path)
                        n787 = TDMS Open(5:FALSE, 6:FALSE, 10:T17."create or replace" ("operation (0:open)"), 11:w1297) -> (0:w1296:errorcluster, 3:→"TDMS LAB05-2":refnum<k34>)  [unwired: 3 in]
                      }
                      frame #2 {
                        n788 = local read "SET LAB05-2"() -> (w1308:T5)
                        n789 = local read "TDMS LAB05-2"() -> (w1319:refnum<k34>)
                        n790 = Build Array("Testers Name", "Description", "Set Test Cycles", "T-Rise minutes", "T-Rise Deg C") -> (w1309:string[])
                        n791 = Unbundle(w1308) -> ("NAME"=w1307:string, "DESCRIPTION"=w1306:string, "CYCLES"=w1305:dbl, "T-RISE mins"=w1304:dbl, "T-RISE deg C"=w1303:dbl)
                        n792 = Number To Decimal String(number=w1305) -> (decimal integer string=w1318:string)  [unwired: 1 in]
                        n793 = Number To Decimal String(number=w1304) -> (decimal integer string=w1317:string)  [unwired: 1 in]
                        n794 = Number To Decimal String(number=w1303) -> (decimal integer string=w1316:string)  [unwired: 1 in]
                        n795 = Build Array(w1307, w1306, w1318, w1317, w1316) -> (w1315:string[])
                        n796 = TDMS Set Properties(5:w1315, 7:w1309, 11:w1319) -> ()  [unwired: 3 in, 4 out]
                      }
                      frame #3 {
                        w1321 = 0.0
                        n797 = local read "DISP LAB05-2"() -> (w1323:T4)
                        n798 = Bundle(cluster=w1323, "CYCLE"=w1321, "MINS"=w1321, "STATUS"="RUN") -> (w1322:T4)
                        n799 = local write "DISP LAB05-2"(w1322) -> ()
                      }
                      frame #4 {
                        n800 = local read "SIG LAB05-2"() -> (w1326:T2)
                        n801 = local read "TEMP START LAB05-2"() -> (w1328:cluster{"TL":dbl, "TN":dbl})
                        n802 = Unbundle(w1326) -> ("Tmp Live"=w1325:dbl, "Tmp Neut"=w1324:dbl)  [unwired: 3 out]
                        n803 = Bundle(cluster=w1328, "TL"=w1325, "TN"=w1324) -> (w1327:cluster{"TL":dbl, "TN":dbl})
                        n804 = local write "TEMP START LAB05-2"(w1327) -> ()
                      }
                    }
                  }
                }
              }
            }
            n805 = local write "data file error"(w380) -> ()
          }
          frame #4 {
            # "check if test cycles reached for cycle tests, if so then test pass"
            n806 = stacked-sequence {
              tunnel: w1348 -> [_ _ _ _ _ _ _ _ _ _]
              tunnel: w1347 -> [_ _ _ _ _ _ _ _ _ _]
              tunnel: w1346 -> [_ _ _ _ _ _ _ _ _ _]
              tunnel: w1345 -> [_ _ _ _ _ _ _ _ _ _]
              tunnel: w1344 -> [_ _ _ _ _ _ _ _ _ _]
              tunnel: w1343 -> [_ _ _ _ _ _ _ _ _ _]
              tunnel: w1342 -> [_ _ _ _ _ _ _ _ _ _]
              tunnel: w1341 -> [_ _ _ _ _ _ _ _ _ _]
              tunnel: w1340 -> [_ _ _ _ _ _ _ _ _ _]
              tunnel: w1339 -> [_ _ _ _ _ _ _ _ _ _]
              tunnel: w1338 -> [w1354 _ _ _ _ _ _ _ _ _]
              tunnel: w1337 -> [_ w1389 _ _ _ _ _ _ _ _]
              tunnel: w1336 -> [_ _ w1429 _ _ _ _ _ _ _]
              tunnel: w1335 -> [_ _ _ w1469 _ _ _ _ _ _]
              tunnel: w1334 -> [_ _ _ _ w1509 _ _ _ _ _]
              tunnel: w1333 -> [_ _ _ _ _ w1549 _ _ _ _]
              tunnel: w1332 -> [_ _ _ _ _ _ w1589 _ _ _]
              tunnel: w1331 -> [_ _ _ _ _ _ _ w1629 _ _]
              tunnel: w1330 -> [_ _ _ _ _ _ _ _ w1669 _]
              tunnel: w1329 -> [_ _ _ _ _ _ _ _ _ w1709]
              frame #0 {
                # "LAB01-1"
                n807 = Less?(x=w1354, y=2) -> (x < y?=w1352:bool)
                n808 = local read "DISP LAB01-1"() -> (w1355:T4)
                n809 = Unbundle(w1355) -> ("STATUS"=w1349:string)  [unwired: 2 out]
                n810 = Equal?(x=w1349, y="RUN") -> (x = y?=w1351:bool)
                n811 = And(x=w1351, y=w1352) -> (x .and. y?=w1350:bool)
                n812 = case shown="True" w1350 {
                  tunnel: w1355 -> [_ w1360]
                  tunnel: w1354 -> [_ w1364]
                  frame False {
                  }
                  frame True {
                    n813 = local read "SET LAB01-1"() -> (w1366:T5)
                    n814 = local read "TDMS LAB01-1"() -> (w1359:refnum<k34>)
                    n815 = Unbundle(w1366) -> ("CYCLES"=w1357:dbl, "T-RISE mins"=w1363:dbl)  [unwired: 3 out]
                    n816 = case shown="\"CYCLE TEST\"" w1364 {
                      tunnel: w1363 -> [_ _ w1373]
                      tunnel: [w1368 w1370 w1373] -> w1362
                      tunnel: w1357 -> [w1368 w1370 _]
                      tunnel: ["CHART PASS" "CYCLE PASS" "T-RISE PASS"] -> w1361
                      frame "CHART TEST", Default {
                      }
                      frame "CYCLE TEST" {
                      }
                      frame "T-RISE TEST" {
                      }
                    }
                    n817 = Unbundle(w1360) -> ("CYCLE"=w1365:dbl)  [unwired: 2 out]
                    n818 = Increment(x=w1357) -> (x+1=w1358:dbl)
                    n819 = Greater Or Equal?(x=w1365, y=w1358) -> (x >= y?=w1367:bool)
                    n820 = case shown="True" w1367 {
                      tunnel: w1362 -> [w1377 _]
                      tunnel: w1361 -> [w1376 _]
                      tunnel: w1360 -> [w1375 _]
                      tunnel: w1359 -> [w1374 _]
                      frame True {
                        n821 = stacked-sequence {
                          tunnel: w1377 -> [w1381 _]
                          tunnel: w1376 -> [w1379 w1385]
                          tunnel: w1375 -> [_ w1388]
                          tunnel: w1374 -> [w1378 _]
                          frame #0 {
                            n822 = Build Array(w1379) -> (w1382:string[])
                            n823 = Build Array(w1381) -> (w1380:dbl[])
                            n824 = TDMS Write(0:w1378, 5:"TEST PASS", 7:w1382, 9:w1380) -> (15:w1384:errorcluster)  [unwired: 2 in, 3 out]
                            n825 = local write "data file error"(w1384) -> ()
                          }
                          frame #1 {
                            n826 = Bundle(cluster=w1388, "STATUS"=w1385) -> (w1386:T4)  [unwired: 2 in]
                            n827 = local write "RESULT LAB01-1"(TRUE) -> ()
                            n828 = local write "DISP LAB01-1"(w1386) -> ()
                          }
                        }
                      }
                      frame False {
                      }
                    }
                  }
                }
              }
              frame #1 {
                # "LAB01-2"
                n829 = Less?(x=w1389, y=2) -> (x < y?=w1392:bool)
                n830 = local read "DISP LAB01-2"() -> (w1394:T4)
                n831 = Unbundle(w1394) -> ("STATUS"=w1395:string)  [unwired: 2 out]
                n832 = Equal?(x=w1395, y="RUN") -> (x = y?=w1391:bool)
                n833 = And(x=w1391, y=w1392) -> (x .and. y?=w1390:bool)
                n834 = case shown="True" w1390 {
                  tunnel: w1394 -> [_ w1400]
                  tunnel: w1389 -> [_ w1404]
                  frame False {
                  }
                  frame True {
                    n835 = local read "SET LAB01-2"() -> (w1406:T5)
                    n836 = local read "TDMS LAB01-2"() -> (w1399:refnum<k34>)
                    n837 = Unbundle(w1406) -> ("CYCLES"=w1397:dbl, "T-RISE mins"=w1403:dbl)  [unwired: 3 out]
                    n838 = case shown="\"T-RISE TEST\"" w1404 {
                      tunnel: w1403 -> [_ _ w1413]
                      tunnel: [w1408 w1410 w1413] -> w1402
                      tunnel: w1397 -> [w1408 w1410 _]
                      tunnel: ["CHART PASS" "CYCLE PASS" "T-RISE PASS"] -> w1401
                      frame "CHART TEST", Default {
                      }
                      frame "CYCLE TEST" {
                      }
                      frame "T-RISE TEST" {
                      }
                    }
                    n839 = Unbundle(w1400) -> ("CYCLE"=w1405:dbl)  [unwired: 2 out]
                    n840 = Increment(x=w1397) -> (x+1=w1398:dbl)
                    n841 = Greater Or Equal?(x=w1405, y=w1398) -> (x >= y?=w1407:bool)
                    n842 = case shown="True" w1407 {
                      tunnel: w1402 -> [w1417 _]
                      tunnel: w1401 -> [w1416 _]
                      tunnel: w1400 -> [w1415 _]
                      tunnel: w1399 -> [w1414 _]
                      frame True {
                        n843 = stacked-sequence {
                          tunnel: w1417 -> [w1421 _]
                          tunnel: w1416 -> [w1419 w1425]
                          tunnel: w1415 -> [_ w1428]
                          tunnel: w1414 -> [w1418 _]
                          frame #0 {
                            n844 = Build Array(w1419) -> (w1422:string[])
                            n845 = Build Array(w1421) -> (w1420:dbl[])
                            n846 = TDMS Write(0:w1418, 5:"TEST PASS", 7:w1422, 9:w1420) -> (15:w1424:errorcluster)  [unwired: 2 in, 3 out]
                            n847 = local write "data file error"(w1424) -> ()
                          }
                          frame #1 {
                            n848 = Bundle(cluster=w1428, "STATUS"=w1425) -> (w1426:T4)  [unwired: 2 in]
                            n849 = local write "RESULT LAB01-2"(TRUE) -> ()
                            n850 = local write "DISP LAB01-2"(w1426) -> ()
                          }
                        }
                      }
                      frame False {
                      }
                    }
                  }
                }
              }
              frame #2 {
                # "LAB02-1"
                n851 = Less?(x=w1429, y=2) -> (x < y?=w1432:bool)
                n852 = local read "DISP LAB02-1"() -> (w1434:T4)
                n853 = Unbundle(w1434) -> ("STATUS"=w1435:string)  [unwired: 2 out]
                n854 = Equal?(x=w1435, y="RUN") -> (x = y?=w1431:bool)
                n855 = And(x=w1431, y=w1432) -> (x .and. y?=w1430:bool)
                n856 = case shown="True" w1430 {
                  tunnel: w1434 -> [_ w1440]
                  tunnel: w1429 -> [_ w1444]
                  frame False {
                  }
                  frame True {
                    n857 = local read "SET LAB02-1"() -> (w1446:T5)
                    n858 = local read "TDMS LAB02-1"() -> (w1439:refnum<k34>)
                    n859 = Unbundle(w1440) -> ("CYCLE"=w1445:dbl)  [unwired: 2 out]
                    n860 = Unbundle(w1446) -> ("CYCLES"=w1437:dbl, "T-RISE mins"=w1443:dbl)  [unwired: 3 out]
                    n861 = case shown="\"T-RISE TEST\"" w1444 {
                      tunnel: w1443 -> [_ _ w1453]
                      tunnel: [w1448 w1450 w1453] -> w1442
                      tunnel: w1437 -> [w1448 w1450 _]
                      tunnel: ["CHART PASS" "CYCLE PASS" "T-RISE PASS"] -> w1441
                      frame "CHART TEST", Default {
                      }
                      frame "CYCLE TEST" {
                      }
                      frame "T-RISE TEST" {
                      }
                    }
                    n862 = Increment(x=w1437) -> (x+1=w1438:dbl)
                    n863 = Greater Or Equal?(x=w1445, y=w1438) -> (x >= y?=w1447:bool)
                    n864 = case shown="True" w1447 {
                      tunnel: w1442 -> [w1457 _]
                      tunnel: w1441 -> [w1456 _]
                      tunnel: w1440 -> [w1455 _]
                      tunnel: w1439 -> [w1454 _]
                      frame True {
                        n865 = stacked-sequence {
                          tunnel: w1457 -> [w1461 _]
                          tunnel: w1456 -> [w1459 w1465]
                          tunnel: w1455 -> [_ w1468]
                          tunnel: w1454 -> [w1458 _]
                          frame #0 {
                            n866 = Build Array(w1459) -> (w1462:string[])
                            n867 = Build Array(w1461) -> (w1460:dbl[])
                            n868 = TDMS Write(0:w1458, 5:"TEST PASS", 7:w1462, 9:w1460) -> (15:w1464:errorcluster)  [unwired: 2 in, 3 out]
                            n869 = local write "data file error"(w1464) -> ()
                          }
                          frame #1 {
                            n870 = Bundle(cluster=w1468, "STATUS"=w1465) -> (w1466:T4)  [unwired: 2 in]
                            n871 = local write "RESULT LAB02-1"(TRUE) -> ()
                            n872 = local write "DISP LAB02-1"(w1466) -> ()
                          }
                        }
                      }
                      frame False {
                      }
                    }
                  }
                }
              }
              frame #3 {
                # "LAB02-2"
                n873 = Less?(x=w1469, y=2) -> (x < y?=w1472:bool)
                n874 = local read "DISP LAB02-2"() -> (w1474:T4)
                n875 = Unbundle(w1474) -> ("STATUS"=w1475:string)  [unwired: 2 out]
                n876 = Equal?(x=w1475, y="RUN") -> (x = y?=w1471:bool)
                n877 = And(x=w1471, y=w1472) -> (x .and. y?=w1470:bool)
                n878 = case shown="True" w1470 {
                  tunnel: w1474 -> [_ w1480]
                  tunnel: w1469 -> [_ w1484]
                  frame False {
                  }
                  frame True {
                    n879 = local read "SET LAB02-2"() -> (w1486:T5)
                    n880 = local read "TDMS LAB02-2"() -> (w1479:refnum<k34>)
                    n881 = Unbundle(w1480) -> ("CYCLE"=w1485:dbl)  [unwired: 2 out]
                    n882 = Unbundle(w1486) -> ("CYCLES"=w1477:dbl, "T-RISE mins"=w1483:dbl)  [unwired: 3 out]
                    n883 = case shown="\"T-RISE TEST\"" w1484 {
                      tunnel: w1483 -> [_ _ w1493]
                      tunnel: [w1488 w1490 w1493] -> w1482
                      tunnel: w1477 -> [w1488 w1490 _]
                      tunnel: ["CHART PASS" "CYCLE PASS" "T-RISE PASS"] -> w1481
                      frame "CHART TEST", Default {
                      }
                      frame "CYCLE TEST" {
                      }
                      frame "T-RISE TEST" {
                      }
                    }
                    n884 = Increment(x=w1477) -> (x+1=w1478:dbl)
                    n885 = Greater Or Equal?(x=w1485, y=w1478) -> (x >= y?=w1487:bool)
                    n886 = case shown="True" w1487 {
                      tunnel: w1482 -> [w1497 _]
                      tunnel: w1481 -> [w1496 _]
                      tunnel: w1480 -> [w1495 _]
                      tunnel: w1479 -> [w1494 _]
                      frame True {
                        n887 = stacked-sequence {
                          tunnel: w1497 -> [w1501 _]
                          tunnel: w1496 -> [w1499 w1505]
                          tunnel: w1495 -> [_ w1508]
                          tunnel: w1494 -> [w1498 _]
                          frame #0 {
                            n888 = Build Array(w1499) -> (w1502:string[])
                            n889 = Build Array(w1501) -> (w1500:dbl[])
                            n890 = TDMS Write(0:w1498, 5:"TEST PASS", 7:w1502, 9:w1500) -> (15:w1504:errorcluster)  [unwired: 2 in, 3 out]
                            n891 = local write "data file error"(w1504) -> ()
                          }
                          frame #1 {
                            n892 = Bundle(cluster=w1508, "STATUS"=w1505) -> (w1506:T4)  [unwired: 2 in]
                            n893 = local write "RESULT LAB02-2"(TRUE) -> ()
                            n894 = local write "DISP LAB02-2"(w1506) -> ()
                          }
                        }
                      }
                      frame False {
                      }
                    }
                  }
                }
              }
              frame #4 {
                # "LAB03-1"
                n895 = Less?(x=w1509, y=2) -> (x < y?=w1512:bool)
                n896 = local read "DISP LAB03-1"() -> (w1514:T4)
                n897 = Unbundle(w1514) -> ("STATUS"=w1515:string)  [unwired: 2 out]
                n898 = Equal?(x=w1515, y="RUN") -> (x = y?=w1511:bool)
                n899 = And(x=w1511, y=w1512) -> (x .and. y?=w1510:bool)
                n900 = case shown="True" w1510 {
                  tunnel: w1514 -> [_ w1520]
                  tunnel: w1509 -> [_ w1524]
                  frame False {
                  }
                  frame True {
                    n901 = local read "SET LAB03-1"() -> (w1526:T5)
                    n902 = local read "TDMS LAB03-1"() -> (w1519:refnum<k34>)
                    n903 = Unbundle(w1520) -> ("CYCLE"=w1525:dbl)  [unwired: 2 out]
                    n904 = Unbundle(w1526) -> ("CYCLES"=w1517:dbl, "T-RISE mins"=w1523:dbl)  [unwired: 3 out]
                    n905 = case shown="\"T-RISE TEST\"" w1524 {
                      tunnel: w1523 -> [_ _ w1533]
                      tunnel: [w1528 w1530 w1533] -> w1522
                      tunnel: w1517 -> [w1528 w1530 _]
                      tunnel: ["CHART PASS" "CYCLE PASS" "T-RISE PASS"] -> w1521
                      frame "CHART TEST", Default {
                      }
                      frame "CYCLE TEST" {
                      }
                      frame "T-RISE TEST" {
                      }
                    }
                    n906 = Increment(x=w1517) -> (x+1=w1518:dbl)
                    n907 = Greater Or Equal?(x=w1525, y=w1518) -> (x >= y?=w1527:bool)
                    n908 = case shown="True" w1527 {
                      tunnel: w1522 -> [w1537 _]
                      tunnel: w1521 -> [w1536 _]
                      tunnel: w1520 -> [w1535 _]
                      tunnel: w1519 -> [w1534 _]
                      frame True {
                        n909 = stacked-sequence {
                          tunnel: w1537 -> [w1541 _]
                          tunnel: w1536 -> [w1539 w1545]
                          tunnel: w1535 -> [_ w1548]
                          tunnel: w1534 -> [w1538 _]
                          frame #0 {
                            n910 = Build Array(w1539) -> (w1542:string[])
                            n911 = Build Array(w1541) -> (w1540:dbl[])
                            n912 = TDMS Write(0:w1538, 5:"TEST PASS", 7:w1542, 9:w1540) -> (15:w1544:errorcluster)  [unwired: 2 in, 3 out]
                            n913 = local write "data file error"(w1544) -> ()
                          }
                          frame #1 {
                            n914 = Bundle(cluster=w1548, "STATUS"=w1545) -> (w1546:T4)  [unwired: 2 in]
                            n915 = local write "RESULT LAB03-1"(TRUE) -> ()
                            n916 = local write "DISP LAB03-1"(w1546) -> ()
                          }
                        }
                      }
                      frame False {
                      }
                    }
                  }
                }
              }
              frame #5 {
                # "LAB03-2"
                n917 = Less?(x=w1549, y=2) -> (x < y?=w1552:bool)
                n918 = local read "DISP LAB03-2"() -> (w1554:T4)
                n919 = Unbundle(w1554) -> ("STATUS"=w1555:string)  [unwired: 2 out]
                n920 = Equal?(x=w1555, y="RUN") -> (x = y?=w1551:bool)
                n921 = And(x=w1551, y=w1552) -> (x .and. y?=w1550:bool)
                n922 = case shown="True" w1550 {
                  tunnel: w1554 -> [_ w1560]
                  tunnel: w1549 -> [_ w1564]
                  frame False {
                  }
                  frame True {
                    n923 = local read "SET LAB03-2"() -> (w1566:T5)
                    n924 = local read "TDMS LAB03-2"() -> (w1559:refnum<k34>)
                    n925 = Unbundle(w1560) -> ("CYCLE"=w1565:dbl)  [unwired: 2 out]
                    n926 = Unbundle(w1566) -> ("CYCLES"=w1557:dbl, "T-RISE mins"=w1563:dbl)  [unwired: 3 out]
                    n927 = case shown="\"T-RISE TEST\"" w1564 {
                      tunnel: w1563 -> [_ _ w1573]
                      tunnel: [w1568 w1570 w1573] -> w1562
                      tunnel: w1557 -> [w1568 w1570 _]
                      tunnel: ["CHART PASS" "CYCLE PASS" "T-RISE PASS"] -> w1561
                      frame "CHART TEST", Default {
                      }
                      frame "CYCLE TEST" {
                      }
                      frame "T-RISE TEST" {
                      }
                    }
                    n928 = Increment(x=w1557) -> (x+1=w1558:dbl)
                    n929 = Greater Or Equal?(x=w1565, y=w1558) -> (x >= y?=w1567:bool)
                    n930 = case shown="True" w1567 {
                      tunnel: w1562 -> [w1577 _]
                      tunnel: w1561 -> [w1576 _]
                      tunnel: w1560 -> [w1575 _]
                      tunnel: w1559 -> [w1574 _]
                      frame True {
                        n931 = stacked-sequence {
                          tunnel: w1577 -> [w1581 _]
                          tunnel: w1576 -> [w1579 w1585]
                          tunnel: w1575 -> [_ w1588]
                          tunnel: w1574 -> [w1578 _]
                          frame #0 {
                            n932 = Build Array(w1579) -> (w1582:string[])
                            n933 = Build Array(w1581) -> (w1580:dbl[])
                            n934 = TDMS Write(0:w1578, 5:"TEST PASS", 7:w1582, 9:w1580) -> (15:w1584:errorcluster)  [unwired: 2 in, 3 out]
                            n935 = local write "data file error"(w1584) -> ()
                          }
                          frame #1 {
                            n936 = Bundle(cluster=w1588, "STATUS"=w1585) -> (w1586:T4)  [unwired: 2 in]
                            n937 = local write "RESULT LAB03-2"(TRUE) -> ()
                            n938 = local write "DISP LAB03-2"(w1586) -> ()
                          }
                        }
                      }
                      frame False {
                      }
                    }
                  }
                }
              }
              frame #6 {
                # "LAB04-1"
                n939 = Less?(x=w1589, y=2) -> (x < y?=w1592:bool)
                n940 = local read "DISP LAB04-1"() -> (w1594:T4)
                n941 = Unbundle(w1594) -> ("STATUS"=w1595:string)  [unwired: 2 out]
                n942 = Equal?(x=w1595, y="RUN") -> (x = y?=w1591:bool)
                n943 = And(x=w1591, y=w1592) -> (x .and. y?=w1590:bool)
                n944 = case shown="True" w1590 {
                  tunnel: w1594 -> [_ w1600]
                  tunnel: w1589 -> [_ w1604]
                  frame False {
                  }
                  frame True {
                    n945 = local read "SET LAB04-1"() -> (w1606:T5)
                    n946 = local read "TDMS LAB04-1"() -> (w1599:refnum<k34>)
                    n947 = Unbundle(w1600) -> ("CYCLE"=w1605:dbl)  [unwired: 2 out]
                    n948 = Unbundle(w1606) -> ("CYCLES"=w1597:dbl, "T-RISE mins"=w1603:dbl)  [unwired: 3 out]
                    n949 = case shown="\"T-RISE TEST\"" w1604 {
                      tunnel: w1603 -> [_ _ w1613]
                      tunnel: [w1608 w1610 w1613] -> w1602
                      tunnel: w1597 -> [w1608 w1610 _]
                      tunnel: ["CHART PASS" "CYCLE PASS" "T-RISE PASS"] -> w1601
                      frame "CHART TEST", Default {
                      }
                      frame "CYCLE TEST" {
                      }
                      frame "T-RISE TEST" {
                      }
                    }
                    n950 = Increment(x=w1597) -> (x+1=w1598:dbl)
                    n951 = Greater Or Equal?(x=w1605, y=w1598) -> (x >= y?=w1607:bool)
                    n952 = case shown="True" w1607 {
                      tunnel: w1602 -> [w1617 _]
                      tunnel: w1601 -> [w1616 _]
                      tunnel: w1600 -> [w1615 _]
                      tunnel: w1599 -> [w1614 _]
                      frame True {
                        n953 = stacked-sequence {
                          tunnel: w1617 -> [w1621 _]
                          tunnel: w1616 -> [w1619 w1625]
                          tunnel: w1615 -> [_ w1628]
                          tunnel: w1614 -> [w1618 _]
                          frame #0 {
                            n954 = Build Array(w1619) -> (w1622:string[])
                            n955 = Build Array(w1621) -> (w1620:dbl[])
                            n956 = TDMS Write(0:w1618, 5:"TEST PASS", 7:w1622, 9:w1620) -> (15:w1624:errorcluster)  [unwired: 2 in, 3 out]
                            n957 = local write "data file error"(w1624) -> ()
                          }
                          frame #1 {
                            n958 = Bundle(cluster=w1628, "STATUS"=w1625) -> (w1626:T4)  [unwired: 2 in]
                            n959 = local write "RESULT LAB04-1"(TRUE) -> ()
                            n960 = local write "DISP LAB04-1"(w1626) -> ()
                          }
                        }
                      }
                      frame False {
                      }
                    }
                  }
                }
              }
              frame #7 {
                # "LAB04-2"
                n961 = Less?(x=w1629, y=2) -> (x < y?=w1632:bool)
                n962 = local read "DISP LAB04-2"() -> (w1634:T4)
                n963 = Unbundle(w1634) -> ("STATUS"=w1635:string)  [unwired: 2 out]
                n964 = Equal?(x=w1635, y="RUN") -> (x = y?=w1631:bool)
                n965 = And(x=w1631, y=w1632) -> (x .and. y?=w1630:bool)
                n966 = case shown="True" w1630 {
                  tunnel: w1634 -> [_ w1640]
                  tunnel: w1629 -> [_ w1644]
                  frame False {
                  }
                  frame True {
                    n967 = local read "SET LAB04-2"() -> (w1646:T5)
                    n968 = local read "TDMS LAB04-2"() -> (w1639:refnum<k34>)
                    n969 = Unbundle(w1640) -> ("CYCLE"=w1645:dbl)  [unwired: 2 out]
                    n970 = Unbundle(w1646) -> ("CYCLES"=w1637:dbl, "T-RISE mins"=w1643:dbl)  [unwired: 3 out]
                    n971 = case shown="\"T-RISE TEST\"" w1644 {
                      tunnel: w1643 -> [_ _ w1653]
                      tunnel: [w1648 w1650 w1653] -> w1642
                      tunnel: w1637 -> [w1648 w1650 _]
                      tunnel: ["CHART PASS" "CYCLE PASS" "T-RISE PASS"] -> w1641
                      frame "CHART TEST", Default {
                      }
                      frame "CYCLE TEST" {
                      }
                      frame "T-RISE TEST" {
                      }
                    }
                    n972 = Increment(x=w1637) -> (x+1=w1638:dbl)
                    n973 = Greater Or Equal?(x=w1645, y=w1638) -> (x >= y?=w1647:bool)
                    n974 = case shown="True" w1647 {
                      tunnel: w1642 -> [w1657 _]
                      tunnel: w1641 -> [w1656 _]
                      tunnel: w1640 -> [w1655 _]
                      tunnel: w1639 -> [w1654 _]
                      frame True {
                        n975 = stacked-sequence {
                          tunnel: w1657 -> [w1661 _]
                          tunnel: w1656 -> [w1659 w1665]
                          tunnel: w1655 -> [_ w1668]
                          tunnel: w1654 -> [w1658 _]
                          frame #0 {
                            n976 = Build Array(w1659) -> (w1662:string[])
                            n977 = Build Array(w1661) -> (w1660:dbl[])
                            n978 = TDMS Write(0:w1658, 5:"TEST PASS", 7:w1662, 9:w1660) -> (15:w1664:errorcluster)  [unwired: 2 in, 3 out]
                            n979 = local write "data file error"(w1664) -> ()
                          }
                          frame #1 {
                            n980 = Bundle(cluster=w1668, "STATUS"=w1665) -> (w1666:T4)  [unwired: 2 in]
                            n981 = local write "RESULT LAB04-2"(TRUE) -> ()
                            n982 = local write "DISP LAB04-2"(w1666) -> ()
                          }
                        }
                      }
                      frame False {
                      }
                    }
                  }
                }
              }
              frame #8 {
                # "LAB05-1"
                n983 = Less?(x=w1669, y=2) -> (x < y?=w1672:bool)
                n984 = local read "DISP LAB05-1"() -> (w1674:T4)
                n985 = Unbundle(w1674) -> ("STATUS"=w1675:string)  [unwired: 2 out]
                n986 = Equal?(x=w1675, y="RUN") -> (x = y?=w1671:bool)
                n987 = And(x=w1671, y=w1672) -> (x .and. y?=w1670:bool)
                n988 = case shown="True" w1670 {
                  tunnel: w1674 -> [_ w1680]
                  tunnel: w1669 -> [_ w1684]
                  frame False {
                  }
                  frame True {
                    n989 = local read "SET LAB05-1"() -> (w1686:T5)
                    n990 = local read "TDMS LAB05-1"() -> (w1679:refnum<k34>)
                    n991 = Unbundle(w1680) -> ("CYCLE"=w1685:dbl)  [unwired: 2 out]
                    n992 = Unbundle(w1686) -> ("CYCLES"=w1677:dbl, "T-RISE mins"=w1683:dbl)  [unwired: 3 out]
                    n993 = case shown="\"T-RISE TEST\"" w1684 {
                      tunnel: w1683 -> [_ _ w1693]
                      tunnel: [w1688 w1690 w1693] -> w1682
                      tunnel: w1677 -> [w1688 w1690 _]
                      tunnel: ["CHART PASS" "CYCLE PASS" "T-RISE PASS"] -> w1681
                      frame "CHART TEST", Default {
                      }
                      frame "CYCLE TEST" {
                      }
                      frame "T-RISE TEST" {
                      }
                    }
                    n994 = Increment(x=w1677) -> (x+1=w1678:dbl)
                    n995 = Greater Or Equal?(x=w1685, y=w1678) -> (x >= y?=w1687:bool)
                    n996 = case shown="True" w1687 {
                      tunnel: w1682 -> [w1697 _]
                      tunnel: w1681 -> [w1696 _]
                      tunnel: w1680 -> [w1695 _]
                      tunnel: w1679 -> [w1694 _]
                      frame True {
                        n997 = stacked-sequence {
                          tunnel: w1697 -> [w1701 _]
                          tunnel: w1696 -> [w1699 w1705]
                          tunnel: w1695 -> [_ w1708]
                          tunnel: w1694 -> [w1698 _]
                          frame #0 {
                            n998 = Build Array(w1699) -> (w1702:string[])
                            n999 = Build Array(w1701) -> (w1700:dbl[])
                            n1000 = TDMS Write(0:w1698, 5:"TEST PASS", 7:w1702, 9:w1700) -> (15:w1704:errorcluster)  [unwired: 2 in, 3 out]
                            n1001 = local write "data file error"(w1704) -> ()
                          }
                          frame #1 {
                            n1002 = Bundle(cluster=w1708, "STATUS"=w1705) -> (w1706:T4)  [unwired: 2 in]
                            n1003 = local write "RESULT LAB05-1"(TRUE) -> ()
                            n1004 = local write "DISP LAB05-1"(w1706) -> ()
                          }
                        }
                      }
                      frame False {
                      }
                    }
                  }
                }
              }
              frame #9 {
                # "LAB05-2"
                n1005 = Less?(x=w1709, y=2) -> (x < y?=w1712:bool)
                n1006 = local read "DISP LAB05-2"() -> (w1714:T4)
                n1007 = Unbundle(w1714) -> ("STATUS"=w1715:string)  [unwired: 2 out]
                n1008 = Equal?(x=w1715, y="RUN") -> (x = y?=w1711:bool)
                n1009 = And(x=w1711, y=w1712) -> (x .and. y?=w1710:bool)
                n1010 = case shown="True" w1710 {
                  tunnel: w1714 -> [_ w1720]
                  tunnel: w1709 -> [_ w1724]
                  frame False {
                  }
                  frame True {
                    n1011 = local read "SET LAB05-2"() -> (w1726:T5)
                    n1012 = local read "TDMS LAB05-2"() -> (w1719:refnum<k34>)
                    n1013 = Unbundle(w1720) -> ("CYCLE"=w1725:dbl)  [unwired: 2 out]
                    n1014 = Unbundle(w1726) -> ("CYCLES"=w1717:dbl, "T-RISE mins"=w1723:dbl)  [unwired: 3 out]
                    n1015 = case shown="\"T-RISE TEST\"" w1724 {
                      tunnel: w1723 -> [_ _ w1733]
                      tunnel: [w1728 w1730 w1733] -> w1722
                      tunnel: w1717 -> [w1728 w1730 _]
                      tunnel: ["CHART PASS" "CYCLE PASS" "T-RISE PASS"] -> w1721
                      frame "CHART TEST", Default {
                      }
                      frame "CYCLE TEST" {
                      }
                      frame "T-RISE TEST" {
                      }
                    }
                    n1016 = Increment(x=w1717) -> (x+1=w1718:dbl)
                    n1017 = Greater Or Equal?(x=w1725, y=w1718) -> (x >= y?=w1727:bool)
                    n1018 = case shown="True" w1727 {
                      tunnel: w1722 -> [w1737 _]
                      tunnel: w1721 -> [w1736 _]
                      tunnel: w1720 -> [w1735 _]
                      tunnel: w1719 -> [w1734 _]
                      frame True {
                        n1019 = stacked-sequence {
                          tunnel: w1737 -> [w1741 _]
                          tunnel: w1736 -> [w1739 w1745]
                          tunnel: w1735 -> [_ w1748]
                          tunnel: w1734 -> [w1738 _]
                          frame #0 {
                            n1020 = Build Array(w1739) -> (w1742:string[])
                            n1021 = Build Array(w1741) -> (w1740:dbl[])
                            n1022 = TDMS Write(0:w1738, 5:"TEST PASS", 7:w1742, 9:w1740) -> (15:w1744:errorcluster)  [unwired: 2 in, 3 out]
                            n1023 = local write "data file error"(w1744) -> ()
                          }
                          frame #1 {
                            n1024 = Bundle(cluster=w1748, "STATUS"=w1745) -> (w1746:T4)  [unwired: 2 in]
                            n1025 = local write "RESULT LAB05-2"(TRUE) -> ()
                            n1026 = local write "DISP LAB05-2"(w1746) -> ()
                          }
                        }
                      }
                      frame False {
                      }
                    }
                  }
                }
              }
            }
          }
          frame #5 {
            # "check if test cycles reached for temperature rise test"
            n1027 = stacked-sequence {
              tunnel: w1778 -> [_ _ _ _ _ _ _ _ _ _]
              tunnel: w1777 -> [_ _ _ _ _ _ _ _ _ _]
              tunnel: w1776 -> [_ _ _ _ _ _ _ _ _ _]
              tunnel: w1775 -> [_ _ _ _ _ _ _ _ _ _]
              tunnel: w1774 -> [_ _ _ _ _ _ _ _ _ _]
              tunnel: w1773 -> [_ _ _ _ _ _ _ _ _ _]
              tunnel: w1772 -> [_ _ _ _ _ _ _ _ _ _]
              tunnel: w1771 -> [_ _ _ _ _ _ _ _ _ _]
              tunnel: w1770 -> [_ _ _ _ _ _ _ _ _ _]
              tunnel: w1769 -> [_ _ _ _ _ _ _ _ _ _]
              tunnel: w1768 -> [w1784 _ _ _ _ _ _ _ _ _]
              tunnel: w1758 -> [w1779 _ _ _ _ _ _ _ _ _]
              tunnel: w1767 -> [_ w1810 _ _ _ _ _ _ _ _]
              tunnel: w1766 -> [_ _ w1840 _ _ _ _ _ _ _]
              tunnel: w1765 -> [_ _ _ w1870 _ _ _ _ _ _]
              tunnel: w1764 -> [_ _ _ _ w1900 _ _ _ _ _]
              tunnel: w1763 -> [_ _ _ _ _ w1930 _ _ _ _]
              tunnel: w1762 -> [_ _ _ _ _ _ w1960 _ _ _]
              tunnel: w1761 -> [_ _ _ _ _ _ _ w1990 _ _]
              tunnel: w1760 -> [_ _ _ _ _ _ _ _ w2020 _]
              tunnel: w1759 -> [_ _ _ _ _ _ _ _ _ w2050]
              tunnel: w1757 -> [_ w1809 _ _ _ _ _ _ _ _]
              tunnel: w1756 -> [_ _ w1839 _ _ _ _ _ _ _]
              tunnel: w1755 -> [_ _ _ w1869 _ _ _ _ _ _]
              tunnel: w1754 -> [_ _ _ _ w1899 _ _ _ _ _]
              tunnel: w1753 -> [_ _ _ _ _ w1929 _ _ _ _]
              tunnel: w1752 -> [_ _ _ _ _ _ w1959 _ _ _]
              tunnel: w1751 -> [_ _ _ _ _ _ _ w1989 _ _]
              tunnel: w1750 -> [_ _ _ _ _ _ _ _ w2019 _]
              tunnel: w1749 -> [_ _ _ _ _ _ _ _ _ w2049]
              frame #0 {
                # "LAB01-1"
                n1028 = Equal?(x=w1784, y=2) -> (x = y?=w1782:bool)
                n1029 = local read "DISP LAB01-1"() -> (w1785:T4)
                n1030 = Unbundle(w1785) -> ("STATUS"=w1786:string)  [unwired: 2 out]
                n1031 = Equal?(x=w1786, y="RUN") -> (x = y?=w1781:bool)
                n1032 = And(x=w1781, y=w1782) -> (x .and. y?=w1780:bool)
                n1033 = case shown="True" w1780 {
                  tunnel: w1785 -> [_ w1789]
                  tunnel: w1779 -> [_ w1792]
                  frame False {
                  }
                  frame True {
                    n1034 = local read "SET LAB01-1"() -> (w1791:T5)
                    n1035 = local read "TDMS LAB01-1"() -> (w1788:refnum<k34>)
                    n1036 = Unbundle(w1789) -> ("CYCLE"=w1793:dbl)  [unwired: 2 out]
                    n1037 = Unbundle(w1791) -> ("T-RISE mins"=w1790:dbl)  [unwired: 4 out]
                    n1038 = Greater Or Equal?(x=w1793, y=w1792) -> (x >= y?=w1794:bool)
                    n1039 = case shown="True" w1794 {
                      tunnel: w1790 -> [w1797 _]
                      tunnel: w1789 -> [w1796 _]
                      tunnel: w1788 -> [w1795 _]
                      frame True {
                        n1040 = stacked-sequence {
                          tunnel: w1797 -> [w1800 _]
                          tunnel: w1796 -> [_ w1805]
                          tunnel: w1795 -> [w1798 _]
                          frame #0 {
                            n1041 = Build Array("T-RISE") -> (w1802:string[])
                            n1042 = Build Array(w1800) -> (w1801:dbl[])
                            n1043 = TDMS Write(0:w1798, 5:"TEST PASS", 7:w1802, 9:w1801) -> (15:w1804:errorcluster)  [unwired: 2 in, 3 out]
                            n1044 = local write "data file error"(w1804) -> ()
                          }
                          frame #1 {
                            n1045 = Bundle(cluster=w1805, "STATUS"="T-RISE PASS") -> (w1807:T4)  [unwired: 2 in]
                            n1046 = local write "RESULT LAB01-1"(TRUE) -> ()
                            n1047 = local write "DISP LAB01-1"(w1807) -> ()
                          }
                        }
                      }
                      frame False {
                      }
                    }
                  }
                }
              }
              frame #1 {
                # "LAB01-2"
                n1048 = Equal?(x=w1810, y=2) -> (x = y?=w1813:bool)
                n1049 = local read "DISP LAB01-2"() -> (w1815:T4)
                n1050 = Unbundle(w1815) -> ("STATUS"=w1816:string)  [unwired: 2 out]
                n1051 = Equal?(x=w1816, y="RUN") -> (x = y?=w1812:bool)
                n1052 = And(x=w1812, y=w1813) -> (x .and. y?=w1811:bool)
                n1053 = case shown="True" w1811 {
                  tunnel: w1815 -> [_ w1819]
                  tunnel: w1809 -> [_ w1822]
                  frame False {
                  }
                  frame True {
                    n1054 = local read "SET LAB01-2"() -> (w1821:T5)
                    n1055 = local read "TDMS LAB01-2"() -> (w1818:refnum<k34>)
                    n1056 = Unbundle(w1819) -> ("CYCLE"=w1823:dbl)  [unwired: 2 out]
                    n1057 = Unbundle(w1821) -> ("T-RISE mins"=w1820:dbl)  [unwired: 4 out]
                    n1058 = Greater Or Equal?(x=w1823, y=w1822) -> (x >= y?=w1824:bool)
                    n1059 = case shown="True" w1824 {
                      tunnel: w1820 -> [w1827 _]
                      tunnel: w1819 -> [w1826 _]
                      tunnel: w1818 -> [w1825 _]
                      frame True {
                        n1060 = stacked-sequence {
                          tunnel: w1827 -> [w1830 _]
                          tunnel: w1826 -> [_ w1835]
                          tunnel: w1825 -> [w1828 _]
                          frame #0 {
                            n1061 = Build Array("T-RISE") -> (w1832:string[])
                            n1062 = Build Array(w1830) -> (w1831:dbl[])
                            n1063 = TDMS Write(0:w1828, 5:"TEST PASS", 7:w1832, 9:w1831) -> (15:w1834:errorcluster)  [unwired: 2 in, 3 out]
                            n1064 = local write "data file error"(w1834) -> ()
                          }
                          frame #1 {
                            n1065 = Bundle(cluster=w1835, "STATUS"="T-RISE PASS") -> (w1837:T4)  [unwired: 2 in]
                            n1066 = local write "RESULT LAB01-2"(TRUE) -> ()
                            n1067 = local write "DISP LAB01-2"(w1837) -> ()
                          }
                        }
                      }
                      frame False {
                      }
                    }
                  }
                }
              }
              frame #2 {
                # "LAB02-1"
                n1068 = Equal?(x=w1840, y=2) -> (x = y?=w1843:bool)
                n1069 = local read "DISP LAB02-1"() -> (w1845:T4)
                n1070 = Unbundle(w1845) -> ("STATUS"=w1846:string)  [unwired: 2 out]
                n1071 = Equal?(x=w1846, y="RUN") -> (x = y?=w1842:bool)
                n1072 = And(x=w1842, y=w1843) -> (x .and. y?=w1841:bool)
                n1073 = case shown="True" w1841 {
                  tunnel: w1845 -> [_ w1849]
                  tunnel: w1839 -> [_ w1852]
                  frame False {
                  }
                  frame True {
                    n1074 = local read "SET LAB02-1"() -> (w1851:T5)
                    n1075 = local read "TDMS LAB02-1"() -> (w1848:refnum<k34>)
                    n1076 = Unbundle(w1849) -> ("CYCLE"=w1853:dbl)  [unwired: 2 out]
                    n1077 = Unbundle(w1851) -> ("T-RISE mins"=w1850:dbl)  [unwired: 4 out]
                    n1078 = Greater Or Equal?(x=w1853, y=w1852) -> (x >= y?=w1854:bool)
                    n1079 = case shown="True" w1854 {
                      tunnel: w1850 -> [w1857 _]
                      tunnel: w1849 -> [w1856 _]
                      tunnel: w1848 -> [w1855 _]
                      frame True {
                        n1080 = stacked-sequence {
                          tunnel: w1857 -> [w1860 _]
                          tunnel: w1856 -> [_ w1865]
                          tunnel: w1855 -> [w1858 _]
                          frame #0 {
                            n1081 = Build Array("T-RISE") -> (w1862:string[])
                            n1082 = Build Array(w1860) -> (w1861:dbl[])
                            n1083 = TDMS Write(0:w1858, 5:"TEST PASS", 7:w1862, 9:w1861) -> (15:w1864:errorcluster)  [unwired: 2 in, 3 out]
                            n1084 = local write "data file error"(w1864) -> ()
                          }
                          frame #1 {
                            n1085 = Bundle(cluster=w1865, "STATUS"="T-RISE PASS") -> (w1867:T4)  [unwired: 2 in]
                            n1086 = local write "RESULT LAB02-1"(TRUE) -> ()
                            n1087 = local write "DISP LAB02-1"(w1867) -> ()
                          }
                        }
                      }
                      frame False {
                      }
                    }
                  }
                }
              }
              frame #3 {
                # "LAB02-2"
                n1088 = Equal?(x=w1870, y=2) -> (x = y?=w1873:bool)
                n1089 = local read "DISP LAB02-2"() -> (w1875:T4)
                n1090 = Unbundle(w1875) -> ("STATUS"=w1876:string)  [unwired: 2 out]
                n1091 = Equal?(x=w1876, y="RUN") -> (x = y?=w1872:bool)
                n1092 = And(x=w1872, y=w1873) -> (x .and. y?=w1871:bool)
                n1093 = case shown="True" w1871 {
                  tunnel: w1875 -> [_ w1879]
                  tunnel: w1869 -> [_ w1882]
                  frame False {
                  }
                  frame True {
                    n1094 = local read "SET LAB02-2"() -> (w1881:T5)
                    n1095 = local read "TDMS LAB02-2"() -> (w1878:refnum<k34>)
                    n1096 = Unbundle(w1879) -> ("CYCLE"=w1883:dbl)  [unwired: 2 out]
                    n1097 = Unbundle(w1881) -> ("T-RISE mins"=w1880:dbl)  [unwired: 4 out]
                    n1098 = Greater Or Equal?(x=w1883, y=w1882) -> (x >= y?=w1884:bool)
                    n1099 = case shown="True" w1884 {
                      tunnel: w1880 -> [w1887 _]
                      tunnel: w1879 -> [w1886 _]
                      tunnel: w1878 -> [w1885 _]
                      frame True {
                        n1100 = stacked-sequence {
                          tunnel: w1887 -> [w1890 _]
                          tunnel: w1886 -> [_ w1895]
                          tunnel: w1885 -> [w1888 _]
                          frame #0 {
                            n1101 = Build Array("T-RISE") -> (w1892:string[])
                            n1102 = Build Array(w1890) -> (w1891:dbl[])
                            n1103 = TDMS Write(0:w1888, 5:"TEST PASS", 7:w1892, 9:w1891) -> (15:w1894:errorcluster)  [unwired: 2 in, 3 out]
                            n1104 = local write "data file error"(w1894) -> ()
                          }
                          frame #1 {
                            n1105 = Bundle(cluster=w1895, "STATUS"="T-RISE PASS") -> (w1897:T4)  [unwired: 2 in]
                            n1106 = local write "RESULT LAB02-2"(TRUE) -> ()
                            n1107 = local write "DISP LAB02-2"(w1897) -> ()
                          }
                        }
                      }
                      frame False {
                      }
                    }
                  }
                }
              }
              frame #4 {
                # "LAB03-1"
                n1108 = Equal?(x=w1900, y=2) -> (x = y?=w1903:bool)
                n1109 = local read "DISP LAB03-1"() -> (w1905:T4)
                n1110 = Unbundle(w1905) -> ("STATUS"=w1906:string)  [unwired: 2 out]
                n1111 = Equal?(x=w1906, y="RUN") -> (x = y?=w1902:bool)
                n1112 = And(x=w1902, y=w1903) -> (x .and. y?=w1901:bool)
                n1113 = case shown="True" w1901 {
                  tunnel: w1905 -> [_ w1909]
                  tunnel: w1899 -> [_ w1912]
                  frame False {
                  }
                  frame True {
                    n1114 = local read "SET LAB03-1"() -> (w1911:T5)
                    n1115 = local read "TDMS LAB03-1"() -> (w1908:refnum<k34>)
                    n1116 = Unbundle(w1909) -> ("CYCLE"=w1913:dbl)  [unwired: 2 out]
                    n1117 = Unbundle(w1911) -> ("T-RISE mins"=w1910:dbl)  [unwired: 4 out]
                    n1118 = Greater Or Equal?(x=w1913, y=w1912) -> (x >= y?=w1914:bool)
                    n1119 = case shown="True" w1914 {
                      tunnel: w1910 -> [w1917 _]
                      tunnel: w1909 -> [w1916 _]
                      tunnel: w1908 -> [w1915 _]
                      frame True {
                        n1120 = stacked-sequence {
                          tunnel: w1917 -> [w1920 _]
                          tunnel: w1916 -> [_ w1925]
                          tunnel: w1915 -> [w1918 _]
                          frame #0 {
                            n1121 = Build Array("T-RISE") -> (w1922:string[])
                            n1122 = Build Array(w1920) -> (w1921:dbl[])
                            n1123 = TDMS Write(0:w1918, 5:"TEST PASS", 7:w1922, 9:w1921) -> (15:w1924:errorcluster)  [unwired: 2 in, 3 out]
                            n1124 = local write "data file error"(w1924) -> ()
                          }
                          frame #1 {
                            n1125 = Bundle(cluster=w1925, "STATUS"="T-RISE PASS") -> (w1927:T4)  [unwired: 2 in]
                            n1126 = local write "RESULT LAB03-1"(TRUE) -> ()
                            n1127 = local write "DISP LAB03-1"(w1927) -> ()
                          }
                        }
                      }
                      frame False {
                      }
                    }
                  }
                }
              }
              frame #5 {
                # "LAB03-2"
                n1128 = Equal?(x=w1930, y=2) -> (x = y?=w1933:bool)
                n1129 = local read "DISP LAB03-2"() -> (w1935:T4)
                n1130 = Unbundle(w1935) -> ("STATUS"=w1936:string)  [unwired: 2 out]
                n1131 = Equal?(x=w1936, y="RUN") -> (x = y?=w1932:bool)
                n1132 = And(x=w1932, y=w1933) -> (x .and. y?=w1931:bool)
                n1133 = case shown="True" w1931 {
                  tunnel: w1935 -> [_ w1939]
                  tunnel: w1929 -> [_ w1942]
                  frame False {
                  }
                  frame True {
                    n1134 = local read "SET LAB03-2"() -> (w1941:T5)
                    n1135 = local read "TDMS LAB03-2"() -> (w1938:refnum<k34>)
                    n1136 = Unbundle(w1939) -> ("CYCLE"=w1943:dbl)  [unwired: 2 out]
                    n1137 = Unbundle(w1941) -> ("T-RISE mins"=w1940:dbl)  [unwired: 4 out]
                    n1138 = Greater Or Equal?(x=w1943, y=w1942) -> (x >= y?=w1944:bool)
                    n1139 = case shown="True" w1944 {
                      tunnel: w1940 -> [w1947 _]
                      tunnel: w1939 -> [w1946 _]
                      tunnel: w1938 -> [w1945 _]
                      frame True {
                        n1140 = stacked-sequence {
                          tunnel: w1947 -> [w1950 _]
                          tunnel: w1946 -> [_ w1955]
                          tunnel: w1945 -> [w1948 _]
                          frame #0 {
                            n1141 = Build Array("T-RISE") -> (w1952:string[])
                            n1142 = Build Array(w1950) -> (w1951:dbl[])
                            n1143 = TDMS Write(0:w1948, 5:"TEST PASS", 7:w1952, 9:w1951) -> (15:w1954:errorcluster)  [unwired: 2 in, 3 out]
                            n1144 = local write "data file error"(w1954) -> ()
                          }
                          frame #1 {
                            n1145 = Bundle(cluster=w1955, "STATUS"="T-RISE PASS") -> (w1957:T4)  [unwired: 2 in]
                            n1146 = local write "RESULT LAB03-2"(TRUE) -> ()
                            n1147 = local write "DISP LAB03-2"(w1957) -> ()
                          }
                        }
                      }
                      frame False {
                      }
                    }
                  }
                }
              }
              frame #6 {
                # "LAB04-1"
                n1148 = Equal?(x=w1960, y=2) -> (x = y?=w1963:bool)
                n1149 = local read "DISP LAB04-1"() -> (w1965:T4)
                n1150 = Unbundle(w1965) -> ("STATUS"=w1966:string)  [unwired: 2 out]
                n1151 = Equal?(x=w1966, y="RUN") -> (x = y?=w1962:bool)
                n1152 = And(x=w1962, y=w1963) -> (x .and. y?=w1961:bool)
                n1153 = case shown="True" w1961 {
                  tunnel: w1965 -> [_ w1969]
                  tunnel: w1959 -> [_ w1972]
                  frame False {
                  }
                  frame True {
                    n1154 = local read "SET LAB04-1"() -> (w1971:T5)
                    n1155 = local read "TDMS LAB04-1"() -> (w1968:refnum<k34>)
                    n1156 = Unbundle(w1969) -> ("CYCLE"=w1973:dbl)  [unwired: 2 out]
                    n1157 = Unbundle(w1971) -> ("T-RISE mins"=w1970:dbl)  [unwired: 4 out]
                    n1158 = Greater Or Equal?(x=w1973, y=w1972) -> (x >= y?=w1974:bool)
                    n1159 = case shown="True" w1974 {
                      tunnel: w1970 -> [w1977 _]
                      tunnel: w1969 -> [w1976 _]
                      tunnel: w1968 -> [w1975 _]
                      frame True {
                        n1160 = stacked-sequence {
                          tunnel: w1977 -> [w1980 _]
                          tunnel: w1976 -> [_ w1985]
                          tunnel: w1975 -> [w1978 _]
                          frame #0 {
                            n1161 = Build Array("T-RISE") -> (w1982:string[])
                            n1162 = Build Array(w1980) -> (w1981:dbl[])
                            n1163 = TDMS Write(0:w1978, 5:"TEST PASS", 7:w1982, 9:w1981) -> (15:w1984:errorcluster)  [unwired: 2 in, 3 out]
                            n1164 = local write "data file error"(w1984) -> ()
                          }
                          frame #1 {
                            n1165 = Bundle(cluster=w1985, "STATUS"="T-RISE PASS") -> (w1987:T4)  [unwired: 2 in]
                            n1166 = local write "RESULT LAB04-1"(TRUE) -> ()
                            n1167 = local write "DISP LAB04-1"(w1987) -> ()
                          }
                        }
                      }
                      frame False {
                      }
                    }
                  }
                }
              }
              frame #7 {
                # "LAB04-2"
                n1168 = Equal?(x=w1990, y=2) -> (x = y?=w1993:bool)
                n1169 = local read "DISP LAB04-2"() -> (w1995:T4)
                n1170 = Unbundle(w1995) -> ("STATUS"=w1996:string)  [unwired: 2 out]
                n1171 = Equal?(x=w1996, y="RUN") -> (x = y?=w1992:bool)
                n1172 = And(x=w1992, y=w1993) -> (x .and. y?=w1991:bool)
                n1173 = case shown="True" w1991 {
                  tunnel: w1995 -> [_ w1999]
                  tunnel: w1989 -> [_ w2002]
                  frame False {
                  }
                  frame True {
                    n1174 = local read "SET LAB04-2"() -> (w2001:T5)
                    n1175 = local read "TDMS LAB04-2"() -> (w1998:refnum<k34>)
                    n1176 = Unbundle(w1999) -> ("CYCLE"=w2003:dbl)  [unwired: 2 out]
                    n1177 = Unbundle(w2001) -> ("T-RISE mins"=w2000:dbl)  [unwired: 4 out]
                    n1178 = Greater Or Equal?(x=w2003, y=w2002) -> (x >= y?=w2004:bool)
                    n1179 = case shown="True" w2004 {
                      tunnel: w2000 -> [w2007 _]
                      tunnel: w1999 -> [w2006 _]
                      tunnel: w1998 -> [w2005 _]
                      frame True {
                        n1180 = stacked-sequence {
                          tunnel: w2007 -> [w2010 _]
                          tunnel: w2006 -> [_ w2015]
                          tunnel: w2005 -> [w2008 _]
                          frame #0 {
                            n1181 = Build Array("T-RISE") -> (w2012:string[])
                            n1182 = Build Array(w2010) -> (w2011:dbl[])
                            n1183 = TDMS Write(0:w2008, 5:"TEST PASS", 7:w2012, 9:w2011) -> (15:w2014:errorcluster)  [unwired: 2 in, 3 out]
                            n1184 = local write "data file error"(w2014) -> ()
                          }
                          frame #1 {
                            n1185 = Bundle(cluster=w2015, "STATUS"="T-RISE PASS") -> (w2017:T4)  [unwired: 2 in]
                            n1186 = local write "RESULT LAB04-2"(TRUE) -> ()
                            n1187 = local write "DISP LAB04-2"(w2017) -> ()
                          }
                        }
                      }
                      frame False {
                      }
                    }
                  }
                }
              }
              frame #8 {
                # "LAB05-1"
                n1188 = Equal?(x=w2020, y=2) -> (x = y?=w2023:bool)
                n1189 = local read "DISP LAB05-1"() -> (w2025:T4)
                n1190 = Unbundle(w2025) -> ("STATUS"=w2026:string)  [unwired: 2 out]
                n1191 = Equal?(x=w2026, y="RUN") -> (x = y?=w2022:bool)
                n1192 = And(x=w2022, y=w2023) -> (x .and. y?=w2021:bool)
                n1193 = case shown="True" w2021 {
                  tunnel: w2025 -> [_ w2029]
                  tunnel: w2019 -> [_ w2032]
                  frame False {
                  }
                  frame True {
                    n1194 = local read "SET LAB05-1"() -> (w2031:T5)
                    n1195 = local read "TDMS LAB05-1"() -> (w2028:refnum<k34>)
                    n1196 = Unbundle(w2029) -> ("CYCLE"=w2033:dbl)  [unwired: 2 out]
                    n1197 = Unbundle(w2031) -> ("T-RISE mins"=w2030:dbl)  [unwired: 4 out]
                    n1198 = Greater Or Equal?(x=w2033, y=w2032) -> (x >= y?=w2034:bool)
                    n1199 = case shown="True" w2034 {
                      tunnel: w2030 -> [w2037 _]
                      tunnel: w2029 -> [w2036 _]
                      tunnel: w2028 -> [w2035 _]
                      frame True {
                        n1200 = stacked-sequence {
                          tunnel: w2037 -> [w2040 _]
                          tunnel: w2036 -> [_ w2045]
                          tunnel: w2035 -> [w2038 _]
                          frame #0 {
                            n1201 = Build Array("T-RISE") -> (w2042:string[])
                            n1202 = Build Array(w2040) -> (w2041:dbl[])
                            n1203 = TDMS Write(0:w2038, 5:"TEST PASS", 7:w2042, 9:w2041) -> (15:w2044:errorcluster)  [unwired: 2 in, 3 out]
                            n1204 = local write "data file error"(w2044) -> ()
                          }
                          frame #1 {
                            n1205 = Bundle(cluster=w2045, "STATUS"="T-RISE PASS") -> (w2047:T4)  [unwired: 2 in]
                            n1206 = local write "RESULT LAB05-1"(TRUE) -> ()
                            n1207 = local write "DISP LAB05-1"(w2047) -> ()
                          }
                        }
                      }
                      frame False {
                      }
                    }
                  }
                }
              }
              frame #9 {
                # "LAB05-2"
                n1208 = Equal?(x=w2050, y=2) -> (x = y?=w2053:bool)
                n1209 = local read "DISP LAB05-2"() -> (w2055:T4)
                n1210 = Unbundle(w2055) -> ("STATUS"=w2056:string)  [unwired: 2 out]
                n1211 = Equal?(x=w2056, y="RUN") -> (x = y?=w2052:bool)
                n1212 = And(x=w2052, y=w2053) -> (x .and. y?=w2051:bool)
                n1213 = case shown="True" w2051 {
                  tunnel: w2055 -> [_ w2059]
                  tunnel: w2049 -> [_ w2062]
                  frame False {
                  }
                  frame True {
                    n1214 = local read "SET LAB05-2"() -> (w2061:T5)
                    n1215 = local read "TDMS LAB05-2"() -> (w2058:refnum<k34>)
                    n1216 = Unbundle(w2059) -> ("CYCLE"=w2063:dbl)  [unwired: 2 out]
                    n1217 = Unbundle(w2061) -> ("T-RISE mins"=w2060:dbl)  [unwired: 4 out]
                    n1218 = Greater Or Equal?(x=w2063, y=w2062) -> (x >= y?=w2064:bool)
                    n1219 = case shown="True" w2064 {
                      tunnel: w2060 -> [w2067 _]
                      tunnel: w2059 -> [w2066 _]
                      tunnel: w2058 -> [w2065 _]
                      frame True {
                        n1220 = stacked-sequence {
                          tunnel: w2067 -> [w2070 _]
                          tunnel: w2066 -> [_ w2075]
                          tunnel: w2065 -> [w2068 _]
                          frame #0 {
                            n1221 = Build Array("T-RISE") -> (w2072:string[])
                            n1222 = Build Array(w2070) -> (w2071:dbl[])
                            n1223 = TDMS Write(0:w2068, 5:"TEST PASS", 7:w2072, 9:w2071) -> (15:w2074:errorcluster)  [unwired: 2 in, 3 out]
                            n1224 = local write "data file error"(w2074) -> ()
                          }
                          frame #1 {
                            n1225 = Bundle(cluster=w2075, "STATUS"="T-RISE PASS") -> (w2077:T4)  [unwired: 2 in]
                            n1226 = local write "RESULT LAB05-2"(TRUE) -> ()
                            n1227 = local write "DISP LAB05-2"(w2077) -> ()
                          }
                        }
                      }
                      frame False {
                      }
                    }
                  }
                }
              }
            }
          }
          frame #6 {
            # "end test & close test files"
            n1228 = stacked-sequence {
              tunnel: w2088 -> [_ _ _ _ _ _ _ _ _ _]
              tunnel: w2089 -> [_ _ _ _ _ _ _ _ _ _]
              tunnel: w2087 -> [_ _ _ _ _ _ _ _ _ _]
              tunnel: w2086 -> [_ _ _ _ _ _ _ _ _ _]
              tunnel: w2085 -> [_ _ _ _ _ _ _ _ _ _]
              tunnel: w2084 -> [_ _ _ _ _ _ _ _ _ _]
              tunnel: w2083 -> [_ _ _ _ _ _ _ _ _ _]
              tunnel: w2082 -> [_ _ _ _ _ _ _ _ _ _]
              tunnel: w2081 -> [_ _ _ _ _ _ _ _ _ _]
              tunnel: w2080 -> [_ _ _ _ _ _ _ _ _ _]
              frame #0 {
                # "LAB01-1"
                n1229 = local read "DISP LAB01-1"() -> (w2093:T4)
                n1230 = local read "run lab01-1"() -> (w2090:bool)
                n1231 = local read "TDMS LAB01-1"() -> (w2091:refnum<k34>)
                n1232 = Unbundle(w2093) -> ("CYCLE"=w2094:dbl, "STATUS"=w2092:string)  [unwired: 1 out]
                n1233 = case shown="True" w2090 {
                  tunnel: w2094 -> [_ w2098]
                  tunnel: w2093 -> [_ w2097]
                  tunnel: w2092 -> [_ w2096]
                  tunnel: w2091 -> [_ w2095]
                  frame False {
                  }
                  frame True {
                    n1234 = Not Equal?(x=w2096, y="RUN") -> (x != y?=w2099:bool)
                    n1235 = Greater?(x=w2098, y=2.0) -> (0:w2101:bool)
                    n1236 = And(x=w2101, y=w2099) -> (x .and. y?=w2100:bool)
                    n1237 = case shown="True" w2100 {
                      tunnel: w2097 -> [_ w2105]
                      tunnel: w2095 -> [_ w2104]
                      frame False {
                      }
                      frame True {
                        n1238 = stacked-sequence {
                          tunnel: w2105 -> [w2109 _ _]
                          tunnel: w2104 -> [_ w2111 _]
                          frame #0 {
                            w2106 = FALSE
                            n1239 = local write "mail control"("END") -> ()
                            n1240 = Bundle(cluster=w2109) -> (w2108:T4)  [unwired: 3 in]
                            n1241 = local write "DISP LAB01-1"(w2108) -> ()
                            n1242 = local write "O/I  LAB01-1"(w2106) -> ()
                            n1243 = local write "run lab01-1"(w2106) -> ()
                            n1244 = local write "RUN LAB01-1"(w2106) -> ()
                          }
                          frame #1 {
                            n1245 = TDMS Close(11:w2111) -> (0:w2110:errorcluster)  [unwired: 1 in, 1 out]
                            n1246 = local write "data file error"(w2110) -> ()
                          }
                          frame #2 {
                            n1247 = stacked-sequence {
                              tunnel: "LAB01-1" -> [w2114 w2116]
                              frame #0 {
                                n1248 = call "sub vi - defrag tdms v1.vi"("panel id"=w2114) -> ("error out"=w2113:errorcluster)  [unwired: 10 in]
                                n1249 = local write "data file error"(w2113) -> ()
                              }
                              frame #1 {
                                n1250 = call "Save data file to network drive v1.vi"("panel id"=w2116) -> ("network file save error"=w2115:errorcluster)  [unwired: 9 in, 1 out]
                                n1251 = local write "data file error"(w2115) -> ()
                              }
                            }
                          }
                        }
                      }
                    }
                  }
                }
              }
              frame #1 {
                # "LAB01-2"
                n1252 = local read "run lab01-2"() -> (w2117:bool)
                n1253 = case shown="True" w2117 {
                  frame False {
                  }
                  frame True {
                    n1254 = local read "DISP LAB01-2"() -> (w2124:T4)
                    n1255 = local read "TDMS LAB01-2"() -> (w2123:refnum<k34>)
                    n1256 = Unbundle(w2124) -> ("CYCLE"=w2120:dbl, "STATUS"=w2125:string)  [unwired: 1 out]
                    n1257 = Not Equal?(x=w2125, y="RUN") -> (x != y?=w2119:bool)
                    n1258 = Greater?(x=w2120, y=2.0) -> (0:w2121:bool)
                    n1259 = And(x=w2121, y=w2119) -> (x .and. y?=w2118:bool)
                    n1260 = case shown="True" w2118 {
                      tunnel: w2124 -> [_ w2128]
                      tunnel: w2123 -> [_ w2127]
                      frame False {
                      }
                      frame True {
                        n1261 = stacked-sequence {
                          tunnel: w2128 -> [w2131 _ _]
                          tunnel: w2127 -> [_ w2133 _]
                          frame #0 {
                            w2129 = FALSE
                            n1262 = local write "mail control"("END") -> ()
                            n1263 = Bundle(cluster=w2131) -> (w2132:T4)  [unwired: 3 in]
                            n1264 = local write "RUN LAB01-2"(w2129) -> ()
                            n1265 = local write "run lab01-2"(w2129) -> ()
                            n1266 = local write "O/I  LAB01-2"(w2129) -> ()
                            n1267 = local write "DISP LAB01-2"(w2132) -> ()
                          }
                          frame #1 {
                            n1268 = TDMS Close(11:w2133) -> (0:w2134:errorcluster)  [unwired: 1 in, 1 out]
                            n1269 = local write "data file error"(w2134) -> ()
                          }
                          frame #2 {
                            n1270 = stacked-sequence {
                              tunnel: "LAB01-2" -> [w2137 w2139]
                              frame #0 {
                                n1271 = call "sub vi - defrag tdms v1.vi"("panel id"=w2137) -> ("error out"=w2136:errorcluster)  [unwired: 10 in]
                                n1272 = local write "data file error"(w2136) -> ()
                              }
                              frame #1 {
                                n1273 = call "Save data file to network drive v1.vi"("panel id"=w2139) -> ("network file save error"=w2138:errorcluster)  [unwired: 9 in, 1 out]
                                n1274 = local write "data file error"(w2138) -> ()
                              }
                            }
                          }
                        }
                      }
                    }
                  }
                }
              }
              frame #2 {
                # "LAB02-1"
                n1275 = local read "run lab02-1"() -> (w2140:bool)
                n1276 = case shown="True" w2140 {
                  frame False {
                  }
                  frame True {
                    n1277 = local read "DISP LAB02-1"() -> (w2147:T4)
                    n1278 = Unbundle(w2147) -> ("CYCLE"=w2143:dbl, "STATUS"=w2148:string)  [unwired: 1 out]
                    n1279 = local read "TDMS LAB02-1"() -> (w2146:refnum<k34>)
                    n1280 = Not Equal?(x=w2148, y="RUN") -> (x != y?=w2142:bool)
                    n1281 = Greater?(x=w2143, y=2.0) -> (0:w2144:bool)
                    n1282 = And(x=w2144, y=w2142) -> (x .and. y?=w2141:bool)
                    n1283 = case shown="True" w2141 {
                      tunnel: w2147 -> [_ w2151]
                      tunnel: w2146 -> [_ w2150]
                      frame False {
                      }
                      frame True {
                        n1284 = stacked-sequence {
                          tunnel: w2151 -> [w2154 _ _]
                          tunnel: w2150 -> [_ w2156 _]
                          frame #0 {
                            w2152 = FALSE
                            n1285 = local write "mail control"("END") -> ()
                            n1286 = Bundle(cluster=w2154) -> (w2155:T4)  [unwired: 3 in]
                            n1287 = local write "O/I  LAB02-1"(w2152) -> ()
                            n1288 = local write "RUN LAB02-1"(w2152) -> ()
                            n1289 = local write "run lab02-1"(w2152) -> ()
                            n1290 = local write "DISP LAB02-1"(w2155) -> ()
                          }
                          frame #1 {
                            n1291 = TDMS Close(11:w2156) -> (0:w2157:errorcluster)  [unwired: 1 in, 1 out]
                            n1292 = local write "data file error"(w2157) -> ()
                          }
                          frame #2 {
                            n1293 = stacked-sequence {
                              tunnel: "LAB02-1" -> [w2160 w2162]
                              frame #0 {
                                n1294 = call "sub vi - defrag tdms v1.vi"("panel id"=w2160) -> ("error out"=w2159:errorcluster)  [unwired: 10 in]
                                n1295 = local write "data file error"(w2159) -> ()
                              }
                              frame #1 {
                                n1296 = call "Save data file to network drive v1.vi"("panel id"=w2162) -> ("network file save error"=w2161:errorcluster)  [unwired: 9 in, 1 out]
                                n1297 = local write "data file error"(w2161) -> ()
                              }
                            }
                          }
                        }
                      }
                    }
                  }
                }
              }
              frame #3 {
                # "LAB02-2"
                n1298 = local read "run lab02-2"() -> (w2163:bool)
                n1299 = case shown="True" w2163 {
                  frame False {
                  }
                  frame True {
                    n1300 = local read "DISP LAB02-2"() -> (w2170:T4)
                    n1301 = local read "TDMS LAB02-2"() -> (w2169:refnum<k34>)
                    n1302 = Unbundle(w2170) -> ("CYCLE"=w2166:dbl, "STATUS"=w2171:string)  [unwired: 1 out]
                    n1303 = Not Equal?(x=w2171, y="RUN") -> (x != y?=w2165:bool)
                    n1304 = Greater?(x=w2166, y=2.0) -> (0:w2167:bool)
                    n1305 = And(x=w2167, y=w2165) -> (x .and. y?=w2164:bool)
                    n1306 = case shown="True" w2164 {
                      tunnel: w2170 -> [_ w2174]
                      tunnel: w2169 -> [_ w2173]
                      frame False {
                      }
                      frame True {
                        n1307 = stacked-sequence {
                          tunnel: w2174 -> [w2177 _ _]
                          tunnel: w2173 -> [_ w2179 _]
                          frame #0 {
                            w2175 = FALSE
                            n1308 = local write "mail control"("END") -> ()
                            n1309 = Bundle(cluster=w2177) -> (w2178:T4)  [unwired: 3 in]
                            n1310 = local write "O/I  LAB02-2"(w2175) -> ()
                            n1311 = local write "run lab02-2"(w2175) -> ()
                            n1312 = local write "RUN LAB02-2"(w2175) -> ()
                            n1313 = local write "DISP LAB02-2"(w2178) -> ()
                          }
                          frame #1 {
                            n1314 = TDMS Close(11:w2179) -> (0:w2180:errorcluster)  [unwired: 1 in, 1 out]
                            n1315 = local write "data file error"(w2180) -> ()
                          }
                          frame #2 {
                            n1316 = stacked-sequence {
                              tunnel: "LAB02-2" -> [w2183 w2185]
                              frame #0 {
                                n1317 = call "sub vi - defrag tdms v1.vi"("panel id"=w2183) -> ("error out"=w2182:errorcluster)  [unwired: 10 in]
                                n1318 = local write "data file error"(w2182) -> ()
                              }
                              frame #1 {
                                n1319 = call "Save data file to network drive v1.vi"("panel id"=w2185) -> ("network file save error"=w2184:errorcluster)  [unwired: 9 in, 1 out]
                                n1320 = local write "data file error"(w2184) -> ()
                              }
                            }
                          }
                        }
                      }
                    }
                  }
                }
              }
              frame #4 {
                # "LAB03-1"
                n1321 = local read "run lab03-1"() -> (w2186:bool)
                n1322 = case shown="True" w2186 {
                  frame False {
                  }
                  frame True {
                    n1323 = local read "DISP LAB03-1"() -> (w2193:T4)
                    n1324 = local read "TDMS LAB03-1"() -> (w2192:refnum<k34>)
                    n1325 = Unbundle(w2193) -> ("CYCLE"=w2189:dbl, "STATUS"=w2194:string)  [unwired: 1 out]
                    n1326 = Not Equal?(x=w2194, y="RUN") -> (x != y?=w2188:bool)
                    n1327 = Greater?(x=w2189, y=2.0) -> (0:w2190:bool)
                    n1328 = And(x=w2190, y=w2188) -> (x .and. y?=w2187:bool)
                    n1329 = case shown="True" w2187 {
                      tunnel: w2193 -> [_ w2197]
                      tunnel: w2192 -> [_ w2196]
                      frame False {
                      }
                      frame True {
                        n1330 = stacked-sequence {
                          tunnel: w2197 -> [w2200 _ _]
                          tunnel: w2196 -> [_ w2202 _]
                          frame #0 {
                            w2198 = FALSE
                            n1331 = local write "mail control"("END") -> ()
                            n1332 = Bundle(cluster=w2200) -> (w2201:T4)  [unwired: 3 in]
                            n1333 = local write "O/I  LAB03-1"(w2198) -> ()
                            n1334 = local write "run lab03-1"(w2198) -> ()
                            n1335 = local write "RUN LAB03-1"(w2198) -> ()
                            n1336 = local write "DISP LAB03-1"(w2201) -> ()
                          }
                          frame #1 {
                            n1337 = TDMS Close(11:w2202) -> (0:w2203:errorcluster)  [unwired: 1 in, 1 out]
                            n1338 = local write "data file error"(w2203) -> ()
                          }
                          frame #2 {
                            n1339 = stacked-sequence {
                              tunnel: "LAB03-1" -> [w2206 w2208]
                              frame #0 {
                                n1340 = call "sub vi - defrag tdms v1.vi"("panel id"=w2206) -> ("error out"=w2205:errorcluster)  [unwired: 10 in]
                                n1341 = local write "data file error"(w2205) -> ()
                              }
                              frame #1 {
                                n1342 = call "Save data file to network drive v1.vi"("panel id"=w2208) -> ("network file save error"=w2207:errorcluster)  [unwired: 9 in, 1 out]
                                n1343 = local write "data file error"(w2207) -> ()
                              }
                            }
                          }
                        }
                      }
                    }
                  }
                }
              }
              frame #5 {
                # "LAB03-2"
                n1344 = local read "run lab03-2"() -> (w2209:bool)
                n1345 = case shown="True" w2209 {
                  frame False {
                  }
                  frame True {
                    n1346 = local read "DISP LAB03-2"() -> (w2216:T4)
                    n1347 = Unbundle(w2216) -> ("CYCLE"=w2212:dbl, "STATUS"=w2217:string)  [unwired: 1 out]
                    n1348 = local read "TDMS LAB03-2"() -> (w2215:refnum<k34>)
                    n1349 = Not Equal?(x=w2217, y="RUN") -> (x != y?=w2211:bool)
                    n1350 = Greater?(x=w2212, y=2.0) -> (0:w2213:bool)
                    n1351 = And(x=w2213, y=w2211) -> (x .and. y?=w2210:bool)
                    n1352 = case shown="True" w2210 {
                      tunnel: w2216 -> [_ w2220]
                      tunnel: w2215 -> [_ w2219]
                      frame False {
                      }
                      frame True {
                        n1353 = stacked-sequence {
                          tunnel: w2220 -> [w2223 _ _]
                          tunnel: w2219 -> [_ w2225 _]
                          frame #0 {
                            w2221 = FALSE
                            n1354 = local write "mail control"("END") -> ()
                            n1355 = Bundle(cluster=w2223) -> (w2224:T4)  [unwired: 3 in]
                            n1356 = local write "RUN LAB03-2"(w2221) -> ()
                            n1357 = local write "O/I  LAB03-2"(w2221) -> ()
                            n1358 = local write "DISP LAB03-2"(w2224) -> ()
                            n1359 = local write "run lab03-2"(w2221) -> ()
                          }
                          frame #1 {
                            n1360 = TDMS Close(11:w2225) -> (0:w2226:errorcluster)  [unwired: 1 in, 1 out]
                            n1361 = local write "data file error"(w2226) -> ()
                          }
                          frame #2 {
                            n1362 = stacked-sequence {
                              tunnel: "LAB03-2" -> [w2229 w2231]
                              frame #0 {
                                n1363 = call "sub vi - defrag tdms v1.vi"("panel id"=w2229) -> ("error out"=w2228:errorcluster)  [unwired: 10 in]
                                n1364 = local write "data file error"(w2228) -> ()
                              }
                              frame #1 {
                                n1365 = call "Save data file to network drive v1.vi"("panel id"=w2231) -> ("network file save error"=w2230:errorcluster)  [unwired: 9 in, 1 out]
                                n1366 = local write "data file error"(w2230) -> ()
                              }
                            }
                          }
                        }
                      }
                    }
                  }
                }
              }
              frame #6 {
                # "LAB04-1"
                n1367 = local read "run lab04-1"() -> (w2232:bool)
                n1368 = case shown="True" w2232 {
                  frame False {
                  }
                  frame True {
                    n1369 = local read "DISP LAB04-1"() -> (w2239:T4)
                    n1370 = Unbundle(w2239) -> ("CYCLE"=w2235:dbl, "STATUS"=w2240:string)  [unwired: 1 out]
                    n1371 = local read "TDMS LAB04-1"() -> (w2238:refnum<k34>)
                    n1372 = Not Equal?(x=w2240, y="RUN") -> (x != y?=w2234:bool)
                    n1373 = Greater?(x=w2235, y=2.0) -> (0:w2236:bool)
                    n1374 = And(x=w2236, y=w2234) -> (x .and. y?=w2233:bool)
                    n1375 = case shown="True" w2233 {
                      tunnel: w2239 -> [_ w2243]
                      tunnel: w2238 -> [_ w2242]
                      frame False {
                      }
                      frame True {
                        n1376 = stacked-sequence {
                          tunnel: w2243 -> [w2246 _ _]
                          tunnel: w2242 -> [_ w2248 _]
                          frame #0 {
                            w2244 = FALSE
                            n1377 = local write "mail control"("END") -> ()
                            n1378 = Bundle(cluster=w2246) -> (w2247:T4)  [unwired: 3 in]
                            n1379 = local write "RUN LAB04-1"(w2244) -> ()
                            n1380 = local write "O/I  LAB04-1"(w2244) -> ()
                            n1381 = local write "run lab04-1"(w2244) -> ()
                            n1382 = local write "DISP LAB04-1"(w2247) -> ()
                          }
                          frame #1 {
                            n1383 = TDMS Close(11:w2248) -> (0:w2249:errorcluster)  [unwired: 1 in, 1 out]
                            n1384 = local write "data file error"(w2249) -> ()
                          }
                          frame #2 {
                            n1385 = stacked-sequence {
                              tunnel: "LAB04-1" -> [w2252 w2254]
                              frame #0 {
                                n1386 = call "sub vi - defrag tdms v1.vi"("panel id"=w2252) -> ("error out"=w2251:errorcluster)  [unwired: 10 in]
                                n1387 = local write "data file error"(w2251) -> ()
                              }
                              frame #1 {
                                n1388 = call "Save data file to network drive v1.vi"("panel id"=w2254) -> ("network file save error"=w2253:errorcluster)  [unwired: 9 in, 1 out]
                                n1389 = local write "data file error"(w2253) -> ()
                              }
                            }
                          }
                        }
                      }
                    }
                  }
                }
              }
              frame #7 {
                # "LAB04-2"
                n1390 = local read "run lab04-2"() -> (w2255:bool)
                n1391 = case shown="True" w2255 {
                  frame False {
                  }
                  frame True {
                    n1392 = local read "DISP LAB04-2"() -> (w2262:T4)
                    n1393 = Unbundle(w2262) -> ("CYCLE"=w2258:dbl, "STATUS"=w2263:string)  [unwired: 1 out]
                    n1394 = Not Equal?(x=w2263, y="RUN") -> (x != y?=w2257:bool)
                    n1395 = local read "TDMS LAB04-2"() -> (w2261:refnum<k34>)
                    n1396 = Greater?(x=w2258, y=2.0) -> (0:w2259:bool)
                    n1397 = And(x=w2259, y=w2257) -> (x .and. y?=w2256:bool)
                    n1398 = case shown="True" w2256 {
                      tunnel: w2262 -> [_ w2266]
                      tunnel: w2261 -> [_ w2265]
                      frame False {
                      }
                      frame True {
                        n1399 = stacked-sequence {
                          tunnel: w2266 -> [w2269 _ _]
                          tunnel: w2265 -> [_ w2271 _]
                          frame #0 {
                            w2267 = FALSE
                            n1400 = local write "mail control"("END") -> ()
                            n1401 = Bundle(cluster=w2269) -> (w2270:T4)  [unwired: 3 in]
                            n1402 = local write "O/I  LAB04-2"(w2267) -> ()
                            n1403 = local write "RUN LAB04-2"(w2267) -> ()
                            n1404 = local write "run lab04-2"(w2267) -> ()
                            n1405 = local write "DISP LAB04-2"(w2270) -> ()
                          }
                          frame #1 {
                            n1406 = TDMS Close(11:w2271) -> (0:w2272:errorcluster)  [unwired: 1 in, 1 out]
                            n1407 = local write "data file error"(w2272) -> ()
                          }
                          frame #2 {
                            n1408 = stacked-sequence {
                              tunnel: "LAB04-2" -> [w2275 w2277]
                              frame #0 {
                                n1409 = call "sub vi - defrag tdms v1.vi"("panel id"=w2275) -> ("error out"=w2274:errorcluster)  [unwired: 10 in]
                                n1410 = local write "data file error"(w2274) -> ()
                              }
                              frame #1 {
                                n1411 = call "Save data file to network drive v1.vi"("panel id"=w2277) -> ("network file save error"=w2276:errorcluster)  [unwired: 9 in, 1 out]
                                n1412 = local write "data file error"(w2276) -> ()
                              }
                            }
                          }
                        }
                      }
                    }
                  }
                }
              }
              frame #8 {
                # "LAB05-1"
                n1413 = local read "run lab05-1"() -> (w2278:bool)
                n1414 = case shown="True" w2278 {
                  frame False {
                  }
                  frame True {
                    n1415 = local read "DISP LAB05-1"() -> (w2285:T4)
                    n1416 = Unbundle(w2285) -> ("CYCLE"=w2281:dbl, "STATUS"=w2286:string)  [unwired: 1 out]
                    n1417 = Not Equal?(x=w2286, y="RUN") -> (x != y?=w2280:bool)
                    n1418 = local read "TDMS LAB05-1"() -> (w2284:refnum<k34>)
                    n1419 = Greater?(x=w2281, y=2.0) -> (0:w2282:bool)
                    n1420 = And(x=w2282, y=w2280) -> (x .and. y?=w2279:bool)
                    n1421 = case shown="True" w2279 {
                      tunnel: w2285 -> [_ w2289]
                      tunnel: w2284 -> [_ w2288]
                      frame False {
                      }
                      frame True {
                        n1422 = stacked-sequence {
                          tunnel: w2289 -> [w2292 _ _]
                          tunnel: w2288 -> [_ w2294 _]
                          frame #0 {
                            w2290 = FALSE
                            n1423 = local write "mail control"("END") -> ()
                            n1424 = Bundle(cluster=w2292) -> (w2293:T4)  [unwired: 3 in]
                            n1425 = local write "O/I  LAB05-1"(w2290) -> ()
                            n1426 = local write "RUN LAB05-1"(w2290) -> ()
                            n1427 = local write "run lab05-1"(w2290) -> ()
                            n1428 = local write "DISP LAB05-1"(w2293) -> ()
                          }
                          frame #1 {
                            n1429 = TDMS Close(11:w2294) -> (0:w2295:errorcluster)  [unwired: 1 in, 1 out]
                            n1430 = local write "data file error"(w2295) -> ()
                          }
                          frame #2 {
                            n1431 = stacked-sequence {
                              tunnel: "LAB05-1" -> [w2298 w2300]
                              frame #0 {
                                n1432 = call "sub vi - defrag tdms v1.vi"("panel id"=w2298) -> ("error out"=w2297:errorcluster)  [unwired: 10 in]
                                n1433 = local write "data file error"(w2297) -> ()
                              }
                              frame #1 {
                                n1434 = call "Save data file to network drive v1.vi"("panel id"=w2300) -> ("network file save error"=w2299:errorcluster)  [unwired: 9 in, 1 out]
                                n1435 = local write "data file error"(w2299) -> ()
                              }
                            }
                          }
                        }
                      }
                    }
                  }
                }
              }
              frame #9 {
                # "LAB05-2"
                n1436 = local read "run lab05-2"() -> (w2301:bool)
                n1437 = case shown="True" w2301 {
                  frame False {
                  }
                  frame True {
                    n1438 = local read "DISP LAB05-2"() -> (w2308:T4)
                    n1439 = Unbundle(w2308) -> ("CYCLE"=w2304:dbl, "STATUS"=w2309:string)  [unwired: 1 out]
                    n1440 = Not Equal?(x=w2309, y="RUN") -> (x != y?=w2303:bool)
                    n1441 = local read "TDMS LAB05-2"() -> (w2307:refnum<k34>)
                    n1442 = Greater?(x=w2304, y=2.0) -> (0:w2305:bool)
                    n1443 = And(x=w2305, y=w2303) -> (x .and. y?=w2302:bool)
                    n1444 = case shown="True" w2302 {
                      tunnel: w2308 -> [_ w2312]
                      tunnel: w2307 -> [_ w2311]
                      frame False {
                      }
                      frame True {
                        n1445 = stacked-sequence {
                          tunnel: w2312 -> [w2315 _ _]
                          tunnel: w2311 -> [_ w2317 _]
                          frame #0 {
                            w2313 = FALSE
                            n1446 = local write "mail control"("END") -> ()
                            n1447 = Bundle(cluster=w2315) -> (w2316:T4)  [unwired: 3 in]
                            n1448 = local write "RUN LAB05-2"(w2313) -> ()
                            n1449 = local write "O/I  LAB05-2"(w2313) -> ()
                            n1450 = local write "run lab05-2"(w2313) -> ()
                            n1451 = local write "DISP LAB05-2"(w2316) -> ()
                          }
                          frame #1 {
                            n1452 = TDMS Close(11:w2317) -> (0:w2318:errorcluster)  [unwired: 1 in, 1 out]
                            n1453 = local write "data file error"(w2318) -> ()
                          }
                          frame #2 {
                            n1454 = stacked-sequence {
                              tunnel: "LAB05-2" -> [w2321 w2323]
                              frame #0 {
                                n1455 = call "sub vi - defrag tdms v1.vi"("panel id"=w2321) -> ("error out"=w2320:errorcluster)  [unwired: 10 in]
                                n1456 = local write "data file error"(w2320) -> ()
                              }
                              frame #1 {
                                n1457 = call "Save data file to network drive v1.vi"("panel id"=w2323) -> ("network file save error"=w2322:errorcluster)  [unwired: 9 in, 1 out]
                                n1458 = local write "data file error"(w2322) -> ()
                              }
                            }
                          }
                        }
                      }
                    }
                  }
                }
              }
            }
            n1459 = local read "Network Directory"() -> (w2079:path)
            n1460 = global write "Global 1.vi" "Network Drive"(w2079) -> ()
          }
          frame #7 {
            # "disable functions"
            n1461 = stacked-sequence {
              tunnel: w2333 -> [w2347 _ w2403]
              tunnel: w2332 -> [w2342 _ w2402]
              tunnel: w2331 -> [w2341 _ w2401]
              tunnel: w2330 -> [w2339 _ w2400]
              tunnel: w2329 -> [w2340 _ w2399]
              tunnel: w2328 -> [_ w2364 w2398]
              tunnel: w2327 -> [_ w2365 w2397]
              tunnel: w2326 -> [_ w2366 w2396]
              tunnel: w2325 -> [_ w2367 w2395]
              tunnel: w2324 -> [_ w2368 w2394]
              frame #0 {
                n1462 = Select(t=2, s=w2339, f=0) -> (s? t:f=w2335:i32)
                n1463 = Select(t=2, s=w2341, f=0) -> (s? t:f=w2336:i32)
                n1464 = Select(t=2, s=w2340, f=0) -> (s? t:f=w2334:i32)
                n1465 = Select(t=2, s=w2347, f=0) -> (s? t:f=w2338:i32)
                n1466 = Select(t=2, s=w2342, f=0) -> (s? t:f=w2337:i32)
                n1467 = property on="SELECT LAB02-2" class="RadioBtnsControl (strict)"("DisabledEnum"=w2335) -> ()  [unwired: 2 in, 2 out]
                n1468 = property on="SELECT LAB02-1" class="RadioBtnsControl (strict)"("DisabledEnum"=w2336) -> ()  [unwired: 2 in, 2 out]
                n1469 = property on="SELECT LAB03-1" class="RadioBtnsControl (strict)"("DisabledEnum"=w2334) -> ()  [unwired: 2 in, 2 out]
                n1470 = property on="SELECT LAB01-1" class="RadioBtnsControl (strict)"("DisabledEnum"=w2338) -> ()  [unwired: 2 in, 2 out]
                n1471 = property on="SELECT LAB01-2" class="RadioBtnsControl (strict)"("DisabledEnum"=w2337) -> ()  [unwired: 2 in, 2 out]
                n1472 = Not(x=w2347) -> (.not. x?=w2348:bool)
                n1473 = property on="RESULT LAB01-1" class="Bool (strict)"("Visible"=w2348) -> ()  [unwired: 2 in, 2 out]
                n1474 = Not(x=w2342) -> (.not. x?=w2346:bool)
                n1475 = Not(x=w2341) -> (.not. x?=w2345:bool)
                n1476 = Not(x=w2339) -> (.not. x?=w2344:bool)
                n1477 = property on="RESULT LAB01-2" class="Bool (strict)"("Visible"=w2346) -> ()  [unwired: 2 in, 2 out]
                n1478 = Not(x=w2340) -> (.not. x?=w2343:bool)
                n1479 = property on="RESULT LAB02-1" class="Bool (strict)"("Visible"=w2345) -> ()  [unwired: 2 in, 2 out]
                n1480 = property on="RESULT LAB02-2" class="Bool (strict)"("Visible"=w2344) -> ()  [unwired: 2 in, 2 out]
                n1481 = property on="RESULT LAB03-1" class="Bool (strict)"("Visible"=w2343) -> ()  [unwired: 2 in, 2 out]
                n1482 = property on="SET LAB01-1" class="Clust (strict)"("DisabledEnum"=w2338) -> ()  [unwired: 2 in, 2 out]
                n1483 = property on="SET LAB01-2" class="Clust (strict)"("DisabledEnum"=w2337) -> ()  [unwired: 2 in, 2 out]
                n1484 = property on="SET LAB02-1" class="Clust (strict)"("DisabledEnum"=w2336) -> ()  [unwired: 2 in, 2 out]
                n1485 = property on="SET LAB02-2" class="Clust (strict)"("DisabledEnum"=w2335) -> ()  [unwired: 2 in, 2 out]
                n1486 = property on="SET LAB03-1" class="Clust (strict)"("DisabledEnum"=w2334) -> ()  [unwired: 2 in, 2 out]
                n1487 = property on="O/I  LAB01-1" class="Bool (strict)"("DisabledEnum"=w2338) -> ()  [unwired: 2 in, 2 out]
                n1488 = property on="O/I  LAB01-2" class="Bool (strict)"("DisabledEnum"=w2337) -> ()  [unwired: 2 in, 2 out]
                n1489 = property on="O/I  LAB02-1" class="Bool (strict)"("DisabledEnum"=w2336) -> ()  [unwired: 2 in, 2 out]
                n1490 = property on="O/I  LAB02-2" class="Bool (strict)"("DisabledEnum"=w2335) -> ()  [unwired: 2 in, 2 out]
                n1491 = property on="O/I  LAB03-1" class="Bool (strict)"("DisabledEnum"=w2334) -> ()  [unwired: 2 in, 2 out]
              }
              frame #1 {
                n1492 = Select(t=2, s=w2368, f=0) -> (s? t:f=w2359:i32)
                n1493 = Select(t=2, s=w2367, f=0) -> (s? t:f=w2360:i32)
                n1494 = Select(t=2, s=w2364, f=0) -> (s? t:f=w2363:i32)
                n1495 = Select(t=2, s=w2365, f=0) -> (s? t:f=w2362:i32)
                n1496 = Select(t=2, s=w2366, f=0) -> (s? t:f=w2361:i32)
                n1497 = property on="SELECT LAB05-2" class="RadioBtnsControl (strict)"("DisabledEnum"=w2359) -> ()  [unwired: 2 in, 2 out]
                n1498 = property on="SELECT LAB05-1" class="RadioBtnsControl (strict)"("DisabledEnum"=w2360) -> ()  [unwired: 2 in, 2 out]
                n1499 = property on="SELECT LAB03-2" class="RadioBtnsControl (strict)"("DisabledEnum"=w2363) -> ()  [unwired: 2 in, 2 out]
                n1500 = property on="SELECT LAB04-1" class="RadioBtnsControl (strict)"("DisabledEnum"=w2362) -> ()  [unwired: 2 in, 2 out]
                n1501 = property on="SELECT LAB04-2" class="RadioBtnsControl (strict)"("DisabledEnum"=w2361) -> ()  [unwired: 2 in, 2 out]
                n1502 = property on="SET LAB05-2" class="Clust (strict)"("DisabledEnum"=w2359) -> ()  [unwired: 2 in, 2 out]
                n1503 = property on="SET LAB05-1" class="Clust (strict)"("DisabledEnum"=w2360) -> ()  [unwired: 2 in, 2 out]
                n1504 = property on="SET LAB03-2" class="Clust (strict)"("DisabledEnum"=w2363) -> ()  [unwired: 2 in, 2 out]
                n1505 = property on="SET LAB04-1" class="Clust (strict)"("DisabledEnum"=w2362) -> ()  [unwired: 2 in, 2 out]
                n1506 = property on="SET LAB04-2" class="Clust (strict)"("DisabledEnum"=w2361) -> ()  [unwired: 2 in, 2 out]
                n1507 = property on="O/I  LAB05-2" class="Bool (strict)"("DisabledEnum"=w2359) -> ()  [unwired: 2 in, 2 out]
                n1508 = property on="O/I  LAB05-1" class="Bool (strict)"("DisabledEnum"=w2360) -> ()  [unwired: 2 in, 2 out]
                n1509 = property on="O/I  LAB04-1" class="Bool (strict)"("DisabledEnum"=w2362) -> ()  [unwired: 2 in, 2 out]
                n1510 = property on="O/I  LAB04-2" class="Bool (strict)"("DisabledEnum"=w2361) -> ()  [unwired: 2 in, 2 out]
                n1511 = property on="O/I  LAB03-2" class="Bool (strict)"("DisabledEnum"=w2363) -> ()  [unwired: 2 in, 2 out]
                n1512 = Not(x=w2368) -> (.not. x?=w2369:bool)
                n1513 = Not(x=w2367) -> (.not. x?=w2370:bool)
                n1514 = Not(x=w2366) -> (.not. x?=w2371:bool)
                n1515 = property on="RESULT LAB05-2" class="Bool (strict)"("Visible"=w2369) -> ()  [unwired: 2 in, 2 out]
                n1516 = property on="RESULT LAB05-1" class="Bool (strict)"("Visible"=w2370) -> ()  [unwired: 2 in, 2 out]
                n1517 = Not(x=w2365) -> (.not. x?=w2372:bool)
                n1518 = property on="RESULT LAB04-2" class="Bool (strict)"("Visible"=w2371) -> ()  [unwired: 2 in, 2 out]
                n1519 = Not(x=w2364) -> (.not. x?=w2373:bool)
                n1520 = property on="RESULT LAB04-1" class="Bool (strict)"("Visible"=w2372) -> ()  [unwired: 2 in, 2 out]
                n1521 = property on="RESULT LAB03-2" class="Bool (strict)"("Visible"=w2373) -> ()  [unwired: 2 in, 2 out]
              }
              frame #2 {
                # "disable calibrate if any test running"
                n1522 = Or(x=w2395, y=w2394) -> (x .or. y?=w2388:bool)
                n1523 = Or(x=w2397, y=w2396) -> (x .or. y?=w2390:bool)
                n1524 = Or(x=w2401, y=w2400) -> (x .or. y?=w2392:bool)
                n1525 = Or(x=w2399, y=w2398) -> (x .or. y?=w2391:bool)
                n1526 = Or(x=w2403, y=w2402) -> (x .or. y?=w2393:bool)
                n1527 = Or(x=w2391, y=w2390) -> (x .or. y?=w2389:bool)
                n1528 = Or(x=w2393, y=w2392) -> (x .or. y?=w2387:bool)
                n1529 = Or(x=w2389, y=w2388) -> (x .or. y?=w2386:bool)
                n1530 = Or(x=w2387, y=w2386) -> (x .or. y?=w2385:bool)
                n1531 = case shown="True" w2385 {
                  tunnel: [0 2] -> w2384
                  frame False {
                  }
                  frame True {
                  }
                }
                n1532 = property on="JIG TEST" class="Clust (strict)"("DisabledEnum"=w2384) -> ()  [unwired: 2 in, 2 out]
                n1533 = property on="Network Directory" class="Path"("DisabledEnum"=w2384) -> ()  [unwired: 2 in, 2 out]
                n1534 = property on="MAIL SETTINGS" class="Clust (strict)"("DisabledEnum"=w2384) -> ()  [unwired: 2 in, 2 out]
                n1535 = property on="CALIBRATE" class="Bool (strict)"("DisabledEnum"=w2384) -> ()  [unwired: 2 in, 2 out]
                n1536 = property on="ADMIN PAGE" class="Bool (strict)"("DisabledEnum"=w2384) -> ()  [unwired: 2 in, 2 out]
              }
            }
          }
          frame #8 {
            # "drive jigs"
            n1537 = stacked-sequence {
              frame #0 {
                # "jig on"
                n1538 = local read "jig cycle"() -> (w2411:dbl)
                n1539 = property on="JIG TEST" class="Clust (strict)"() -> ("DisabledEnum"=w2408:T13)  [unwired: 2 in, 2 out]
                n1540 = Equal?(x=w2408, y=2) -> (x = y?=w2407:bool)
                n1541 = Equal?(x=w2411, y=0) -> (x = y?=w2409:bool)
                n1542 = And(x=w2409, y=w2407) -> (x .and. y?=w2406:bool)
                n1543 = case shown="True" w2406 {
                  frame False {
                  }
                  frame True {
                    n1544 = local read "run lab01-1"() -> (w2422:bool)
                    n1545 = local read "run lab01-2"() -> (w2421:bool)
                    n1546 = local read "run lab02-1"() -> (w2420:bool)
                    n1547 = local read "run lab02-2"() -> (w2419:bool)
                    n1548 = local read "run lab03-1"() -> (w2418:bool)
                    n1549 = local read "run lab03-2"() -> (w2417:bool)
                    n1550 = local read "run lab04-1"() -> (w2416:bool)
                    n1551 = local read "run lab04-2"() -> (w2415:bool)
                    n1552 = local read "run lab05-1"() -> (w2414:bool)
                    n1553 = local read "run lab05-2"() -> (w2413:bool)
                    n1554 = local write "JIG LAB03-2"(w2417) -> ()
                    n1555 = local write "JIG LAB01-1"(w2422) -> ()
                    n1556 = local write "JIG LAB01-2"(w2421) -> ()
                    n1557 = local write "JIG LAB02-1"(w2420) -> ()
                    n1558 = local write "JIG LAB02-2"(w2419) -> ()
                    n1559 = local write "JIG LAB03-1"(w2418) -> ()
                    n1560 = local write "JIG LAB04-1"(w2416) -> ()
                    n1561 = local write "JIG LAB04-2"(w2415) -> ()
                    n1562 = local write "JIG LAB05-1"(w2414) -> ()
                    n1563 = local write "JIG LAB05-2"(w2413) -> ()
                  }
                }
              }
              frame #1 {
                # "jig off"
                n1564 = local read "jig cycle"() -> (w2429:dbl)
                n1565 = local read "on loops"() -> (w2428:dbl)
                n1566 = property on="JIG TEST" class="Clust (strict)"() -> ("DisabledEnum"=w2427:T13)  [unwired: 2 in, 2 out]
                n1567 = Equal?(x=w2427, y=2) -> (x = y?=w2425:bool)
                n1568 = Equal?(x=w2429, y=w2428) -> (x = y?=w2424:bool)
                n1569 = And(x=w2424, y=w2425) -> (x .and. y?=w2423:bool)
                n1570 = case shown="True" w2423 {
                  frame False {
                  }
                  frame True {
                    w2480 = FALSE
                    w2481 = TRUE
                    w2479 = 2
                    n1571 = local read "SELECT LAB05-2"() -> (w2470:T3)
                    n1572 = local read "SELECT LAB04-2"() -> (w2472:T3)
                    n1573 = local read "SELECT LAB04-1"() -> (w2473:T3)
                    n1574 = local read "SELECT LAB05-1"() -> (w2471:T3)
                    n1575 = local read "SELECT LAB03-2"() -> (w2474:T3)
                    n1576 = local read "SELECT LAB02-1"() -> (w2477:T3)
                    n1577 = local read "SELECT LAB03-1"() -> (w2475:T3)
                    n1578 = local read "SELECT LAB02-2"() -> (w2476:T3)
                    n1579 = local read "SELECT LAB01-2"() -> (w2478:T3)
                    n1580 = local read "run lab05-1"() -> (w2440:bool)
                    n1581 = local read "run lab05-2"() -> (w2439:bool)
                    n1582 = local read "SELECT LAB01-1"() -> (w2482:T3)
                    n1583 = local read "run lab04-2"() -> (w2441:bool)
                    n1584 = local read "run lab04-1"() -> (w2442:bool)
                    n1585 = local read "run lab01-1"() -> (w2458:bool)
                    n1586 = local read "run lab01-2"() -> (w2447:bool)
                    n1587 = local read "run lab03-2"() -> (w2443:bool)
                    n1588 = local read "run lab03-1"() -> (w2444:bool)
                    n1589 = local read "run lab02-1"() -> (w2446:bool)
                    n1590 = local read "run lab02-2"() -> (w2445:bool)
                    n1591 = Equal?(x=w2479, y=w2475) -> (x = y?=w2453:bool)
                    n1592 = Equal?(x=w2479, y=w2474) -> (x = y?=w2452:bool)
                    n1593 = Equal?(x=w2479, y=w2473) -> (x = y?=w2451:bool)
                    n1594 = Equal?(x=w2479, y=w2472) -> (x = y?=w2450:bool)
                    n1595 = Equal?(x=w2479, y=w2471) -> (x = y?=w2449:bool)
                    n1596 = Equal?(x=w2479, y=w2470) -> (x = y?=w2448:bool)
                    n1597 = Equal?(x=w2479, y=w2482) -> (x = y?=w2459:bool)
                    n1598 = Equal?(x=w2479, y=w2477) -> (x = y?=w2455:bool)
                    n1599 = Equal?(x=w2479, y=w2476) -> (x = y?=w2454:bool)
                    n1600 = Equal?(x=w2479, y=w2478) -> (x = y?=w2456:bool)
                    n1601 = And(x=w2450, y=w2441) -> (x .and. y?=w2432:bool)
                    n1602 = And(x=w2453, y=w2444) -> (x .and. y?=w2435:bool)
                    n1603 = And(x=w2451, y=w2442) -> (x .and. y?=w2433:bool)
                    n1604 = And(x=w2448, y=w2439) -> (x .and. y?=w2430:bool)
                    n1605 = And(x=w2454, y=w2445) -> (x .and. y?=w2436:bool)
                    n1606 = And(x=w2452, y=w2443) -> (x .and. y?=w2434:bool)
                    n1607 = And(x=w2449, y=w2440) -> (x .and. y?=w2431:bool)
                    n1608 = And(x=w2456, y=w2447) -> (x .and. y?=w2438:bool)
                    n1609 = And(x=w2459, y=w2458) -> (x .and. y?=w2457:bool)
                    n1610 = And(x=w2455, y=w2446) -> (x .and. y?=w2437:bool)
                    n1611 = Select(t=w2481, s=w2457, f=w2480) -> (s? t:f=w2460:bool)
                    n1612 = Select(t=w2481, s=w2438, f=w2480) -> (s? t:f=w2461:bool)
                    n1613 = Select(t=w2481, s=w2437, f=w2480) -> (s? t:f=w2462:bool)
                    n1614 = Select(t=w2481, s=w2436, f=w2480) -> (s? t:f=w2463:bool)
                    n1615 = Select(t=w2481, s=w2435, f=w2480) -> (s? t:f=w2464:bool)
                    n1616 = Select(t=w2481, s=w2434, f=w2480) -> (s? t:f=w2465:bool)
                    n1617 = Select(t=w2481, s=w2433, f=w2480) -> (s? t:f=w2466:bool)
                    n1618 = Select(t=w2481, s=w2432, f=w2480) -> (s? t:f=w2467:bool)
                    n1619 = Select(t=w2481, s=w2431, f=w2480) -> (s? t:f=w2468:bool)
                    n1620 = Select(t=w2481, s=w2430, f=w2480) -> (s? t:f=w2469:bool)
                    n1621 = local write "JIG LAB03-2"(w2465) -> ()
                    n1622 = local write "JIG LAB02-1"(w2462) -> ()
                    n1623 = local write "JIG LAB02-2"(w2463) -> ()
                    n1624 = local write "JIG LAB01-2"(w2461) -> ()
                    n1625 = local write "JIG LAB03-1"(w2464) -> ()
                    n1626 = local write "JIG LAB01-1"(w2460) -> ()
                    n1627 = local write "JIG LAB05-2"(w2469) -> ()
                    n1628 = local write "JIG LAB04-1"(w2466) -> ()
                    n1629 = local write "JIG LAB05-1"(w2468) -> ()
                    n1630 = local write "JIG LAB04-2"(w2467) -> ()
                  }
                }
              }
            }
          }
          frame #9 {
            # "enable  jig test output if no test busy"
            n1631 = property on="JIG TEST" class="Clust (strict)"() -> ("DisabledEnum"=w2485:T13)  [unwired: 2 in, 2 out]
            n1632 = Equal?(x=w2485, y=0) -> (x = y?=w2483:bool)
            n1633 = case shown="True" w2483 {
              frame False {
              }
              frame True {
                n1634 = local read "JIG TEST"() -> (w2496:T10)
                n1635 = Unbundle(w2496) -> ("LAB01-1"=w2495:bool, "LAB01-2"=w2494:bool, "LAB02-1"=w2493:bool, "LAB02-2"=w2492:bool, "LAB03-1"=w2491:bool, "LAB03-2"=w2490:bool, "LAB04-1"=w2489:bool, "LAB04-2"=w2488:bool, "LAB05-1"=w2487:bool, "LAB05-2"=w2486:bool)
                n1636 = local write "JIG LAB05-1"(w2487) -> ()
                n1637 = local write "JIG LAB05-2"(w2486) -> ()
                n1638 = local write "JIG LAB04-1"(w2489) -> ()
                n1639 = local write "JIG LAB04-2"(w2488) -> ()
                n1640 = local write "JIG LAB03-2"(w2490) -> ()
                n1641 = local write "JIG LAB01-1"(w2495) -> ()
                n1642 = local write "JIG LAB02-1"(w2493) -> ()
                n1643 = local write "JIG LAB03-1"(w2491) -> ()
                n1644 = local write "JIG LAB01-2"(w2494) -> ()
                n1645 = local write "JIG LAB02-2"(w2492) -> ()
              }
            }
          }
          frame #10 {
            # "drive digital output"
            n1646 = local read "O/I  LAB05-2"() -> (w2502:bool)
            n1647 = local read "O/I  LAB05-1"() -> (w2504:bool)
            n1648 = local read "JIG LAB05-2"() -> (w2501:bool)
            n1649 = local read "O/I  LAB04-2"() -> (w2506:bool)
            n1650 = local read "JIG LAB05-1"() -> (w2503:bool)
            n1651 = local read "JIG LAB04-2"() -> (w2505:bool)
            n1652 = local read "O/I  LAB03-1"() -> (w2511:bool)
            n1653 = local read "O/I  LAB04-1"() -> (w2507:bool)
            n1654 = local read "O/I  LAB02-1"() -> (w2515:bool)
            n1655 = local read "O/I  LAB02-2"() -> (w2513:bool)
            n1656 = local read "O/I  LAB03-2"() -> (w2509:bool)
            n1657 = local read "JIG LAB04-1"() -> (w2500:bool)
            n1658 = local read "JIG LAB03-2"() -> (w2508:bool)
            n1659 = local read "O/I  LAB01-2"() -> (w2517:bool)
            n1660 = local read "JIG LAB02-1"() -> (w2514:bool)
            n1661 = local read "JIG LAB02-2"() -> (w2512:bool)
            n1662 = local read "JIG LAB03-1"() -> (w2510:bool)
            n1663 = local read "O/I  LAB01-1"() -> (w2519:bool)
            n1664 = local read "JIG LAB01-2"() -> (w2516:bool)
            n1665 = local read "JIG LAB01-1"() -> (w2518:bool)
            n1666 = Build Array(w2506, w2505, w2504, w2503, w2502, w2501) -> (w2497:bool[])
            n1667 = Build Array(w2512, w2511, w2510, w2509, w2508, w2507, w2500) -> (w2498:bool[])
            n1668 = Build Array(w2519, w2518, w2517, w2516, w2515, w2514, w2513) -> (w2499:bool[])
            n1669 = call "sub vi - Drive Relays All v6.vi"("Array #2"=w2497, "Array #1"=w2498, "Array #0"=w2499) -> ()  [unwired: 8 in, 1 out]
          }
          frame #11 {
            # "get temperature values"
            n1670 = stacked-sequence {
              frame #0 {
                n1671 = local read "jig cycle"() -> (w2520:dbl)
                n1672 = local read "on loops"() -> (w2523:dbl)
                n1673 = local read "jig cycle"() -> (w2525:dbl)
                n1674 = Add(x=w2523, y=2) -> (x+y=w2524:dbl)
                n1675 = Equal?(x=w2525, y=0) -> (x = y?=w2526:bool)
                n1676 = Equal?(x=w2520, y=w2524) -> (x = y?=w2521:bool)
                n1677 = case shown="True" w2526 {
                  frame False {
                  }
                  frame True {
                    w2538 = FALSE
                    w2539 = TRUE
                    n1678 = local write "TEMP update"(TRUE) -> ()
                    n1679 = call "sub vi - GET ALL TEMP v3.vi"("LA01-EN"=w2539, "LA02-EN"=w2539, "LA03-EN"=w2539, "LA04-EN"=w2538, "LA05-EN"=w2538, "Gen Cal Value"=1.0) -> ("LA01 TEMP"=w2537:T21, "LA02 TEMP"=w2535:T21, "LA03 TEMP"=w2534:T21)  [unwired: 4 in, 3 out]
                    n1680 = local write "LAB03 TEMP"(w2534) -> ()
                    n1681 = local write "LAB02 TEMP"(w2535) -> ()
                    n1682 = local write "LAB01 TEMP"(w2537) -> ()
                  }
                }
                n1683 = case shown="True" w2521 {
                  frame False {
                  }
                  frame True {
                    w2531 = TRUE
                    w2532 = FALSE
                    n1684 = local write "TEMP update"(TRUE) -> ()
                    n1685 = call "sub vi - GET ALL TEMP v3.vi"("LA01-EN"=w2532, "LA02-EN"=w2532, "LA03-EN"=w2532, "LA04-EN"=w2531, "LA05-EN"=w2531, "Gen Cal Value"=1.0) -> ("LA04 TEMP"=w2529:T21, "LA05 TEMP"=w2528:T21)  [unwired: 4 in, 4 out]
                    n1686 = local write "LAB04 TEMP"(w2529) -> ()
                    n1687 = local write "LAB05 TEMP"(w2528) -> ()
                  }
                }
              }
              frame #1 {
                n1688 = local read "CAL LAB01"() -> (w2557:T7)
                n1689 = local read "LAB01 TEMP"() -> (w2558:T12)
                n1690 = Unbundle By Name(w2558) -> ("T1 Live"=w2548:dbl, "T1 Neut"=w2547:dbl, "T2 Live"=w2546:dbl, "T2 Neut"=w2545:dbl)  [unwired: 2 out]
                n1691 = Unbundle By Name(w2557) -> ("1 (TL) cal"=w2544:dbl, "1 (TN) cal"=w2543:dbl, "2 (TL) cal"=w2542:dbl, "2 (TN) cal"=w2541:dbl)  [unwired: 6 out]
                n1692 = Multiply(x=w2548, y=w2544) -> (x*y=w2554:dbl)
                n1693 = Multiply(x=w2547, y=w2543) -> (x*y=w2553:dbl)
                n1694 = Multiply(x=w2546, y=w2542) -> (x*y=w2550:dbl)
                n1695 = Multiply(x=w2545, y=w2541) -> (x*y=w2549:dbl)
                n1696 = local read "SIG LAB01-2"() -> (w2552:T2)
                n1697 = local read "SIG LAB01-1"() -> (w2556:T2)
                n1698 = Bundle By Name(cluster=w2556, "Tmp Live"=w2554, "Tmp Neut"=w2553) -> (w2555:T2)
                n1699 = Bundle By Name(cluster=w2552, "Tmp Live"=w2550, "Tmp Neut"=w2549) -> (w2551:T2)
                n1700 = local write "SIG LAB01-1"(w2555) -> ()
                n1701 = local write "SIG LAB01-2"(w2551) -> ()
              }
              frame #2 {
                n1702 = local read "CAL LAB02"() -> (w2575:T8)
                n1703 = local read "LAB02 TEMP"() -> (w2576:T12)
                n1704 = Unbundle By Name(w2576) -> ("T1 Live"=w2566:dbl, "T1 Neut"=w2565:dbl, "T2 Live"=w2564:dbl, "T2 Neut"=w2563:dbl)  [unwired: 2 out]
                n1705 = Unbundle By Name(w2575) -> ("1 (TL) cal"=w2562:dbl, "1 (TN) cal"=w2561:dbl, "2 (TL) cal"=w2560:dbl, "2 (TN) cal"=w2559:dbl)  [unwired: 6 out]
                n1706 = Multiply(x=w2566, y=w2562) -> (x*y=w2572:dbl)
                n1707 = Multiply(x=w2565, y=w2561) -> (x*y=w2571:dbl)
                n1708 = Multiply(x=w2564, y=w2560) -> (x*y=w2568:dbl)
                n1709 = Multiply(x=w2563, y=w2559) -> (x*y=w2567:dbl)
                n1710 = local read "SIG LAB02-2"() -> (w2570:T2)
                n1711 = local read "SIG LAB02-1"() -> (w2574:T2)
                n1712 = Bundle By Name(cluster=w2574, "Tmp Live"=w2572, "Tmp Neut"=w2571) -> (w2573:T2)
                n1713 = Bundle By Name(cluster=w2570, "Tmp Live"=w2568, "Tmp Neut"=w2567) -> (w2569:T2)
                n1714 = local write "SIG LAB02-1"(w2573) -> ()
                n1715 = local write "SIG LAB02-2"(w2569) -> ()
              }
              frame #3 {
                n1716 = local read "CAL LAB03"() -> (w2593:T7)
                n1717 = local read "LAB03 TEMP"() -> (w2594:T12)
                n1718 = Unbundle By Name(w2594) -> ("T1 Live"=w2584:dbl, "T1 Neut"=w2583:dbl, "T2 Live"=w2582:dbl, "T2 Neut"=w2581:dbl)  [unwired: 2 out]
                n1719 = Unbundle By Name(w2593) -> ("1 (TL) cal"=w2580:dbl, "1 (TN) cal"=w2579:dbl, "2 (TL) cal"=w2578:dbl, "2 (TN) cal"=w2577:dbl)  [unwired: 6 out]
                n1720 = Multiply(x=w2584, y=w2580) -> (x*y=w2590:dbl)
                n1721 = Multiply(x=w2583, y=w2579) -> (x*y=w2589:dbl)
                n1722 = Multiply(x=w2582, y=w2578) -> (x*y=w2586:dbl)
                n1723 = Multiply(x=w2581, y=w2577) -> (x*y=w2585:dbl)
                n1724 = local read "SIG LAB03-2"() -> (w2588:T2)
                n1725 = local read "SIG LAB03-1"() -> (w2592:T2)
                n1726 = Bundle By Name(cluster=w2592, "Tmp Live"=w2590, "Tmp Neut"=w2589) -> (w2591:T2)
                n1727 = Bundle By Name(cluster=w2588, "Tmp Live"=w2586, "Tmp Neut"=w2585) -> (w2587:T2)
                n1728 = local write "SIG LAB03-1"(w2591) -> ()
                n1729 = local write "SIG LAB03-2"(w2587) -> ()
              }
              frame #4 {
                n1730 = local read "CAL LAB04"() -> (w2611:T7)
                n1731 = local read "LAB04 TEMP"() -> (w2612:T12)
                n1732 = Unbundle By Name(w2612) -> ("T1 Live"=w2602:dbl, "T1 Neut"=w2601:dbl, "T2 Live"=w2600:dbl, "T2 Neut"=w2599:dbl)  [unwired: 2 out]
                n1733 = Unbundle By Name(w2611) -> ("1 (TL) cal"=w2598:dbl, "1 (TN) cal"=w2597:dbl, "2 (TL) cal"=w2596:dbl, "2 (TN) cal"=w2595:dbl)  [unwired: 6 out]
                n1734 = Multiply(x=w2602, y=w2598) -> (x*y=w2608:dbl)
                n1735 = Multiply(x=w2601, y=w2597) -> (x*y=w2607:dbl)
                n1736 = Multiply(x=w2600, y=w2596) -> (x*y=w2604:dbl)
                n1737 = Multiply(x=w2599, y=w2595) -> (x*y=w2603:dbl)
                n1738 = local read "SIG LAB04-2"() -> (w2606:T2)
                n1739 = local read "SIG LAB04-1"() -> (w2610:T2)
                n1740 = Bundle By Name(cluster=w2610, "Tmp Live"=w2608, "Tmp Neut"=w2607) -> (w2609:T2)
                n1741 = Bundle By Name(cluster=w2606, "Tmp Live"=w2604, "Tmp Neut"=w2603) -> (w2605:T2)
                n1742 = local write "SIG LAB04-1"(w2609) -> ()
                n1743 = local write "SIG LAB04-2"(w2605) -> ()
              }
              frame #5 {
                n1744 = local read "CAL LAB05"() -> (w2629:T7)
                n1745 = local read "LAB05 TEMP"() -> (w2630:T12)
                n1746 = Unbundle By Name(w2630) -> ("T1 Live"=w2620:dbl, "T1 Neut"=w2619:dbl, "T2 Live"=w2618:dbl, "T2 Neut"=w2617:dbl)  [unwired: 2 out]
                n1747 = Unbundle By Name(w2629) -> ("1 (TL) cal"=w2616:dbl, "1 (TN) cal"=w2615:dbl, "2 (TL) cal"=w2614:dbl, "2 (TN) cal"=w2613:dbl)  [unwired: 6 out]
                n1748 = Multiply(x=w2620, y=w2616) -> (x*y=w2626:dbl)
                n1749 = Multiply(x=w2619, y=w2615) -> (x*y=w2625:dbl)
                n1750 = Multiply(x=w2618, y=w2614) -> (x*y=w2622:dbl)
                n1751 = Multiply(x=w2617, y=w2613) -> (x*y=w2621:dbl)
                n1752 = local read "SIG LAB05-2"() -> (w2624:T2)
                n1753 = local read "SIG LAB05-1"() -> (w2628:T2)
                n1754 = Bundle By Name(cluster=w2628, "Tmp Live"=w2626, "Tmp Neut"=w2625) -> (w2627:T2)
                n1755 = Bundle By Name(cluster=w2624, "Tmp Live"=w2622, "Tmp Neut"=w2621) -> (w2623:T2)
                n1756 = local write "SIG LAB05-1"(w2627) -> ()
                n1757 = local write "SIG LAB05-2"(w2623) -> ()
              }
            }
          }
          frame #12 {
            # "get analog values"
            n1758 = local read "on loops"() -> (w2637:dbl)
            n1759 = local read "jig cycle"() -> (w2634:dbl)
            n1760 = Add(x=w2637, y=1) -> (x+y=w2635:dbl)
            n1761 = Equal?(x=w2634, y=1) -> (x = y?=w2632:bool)
            n1762 = Equal?(x=w2634, y=w2635) -> (x = y?=w2633:bool)
            n1763 = Or(x=w2632, y=w2633) -> (x .or. y?=w2631:bool)
            n1764 = case shown="True" w2631 {
              frame False {
              }
              frame True {
                n1765 = call "sub vi - Read Analog All v8.vi"() -> ("Analog loop time"=w2645:dbl, "array GRAPH"=w2644:dynamicdata[], "LAB01"=w2643:T22, "LAB02"=w2642:T23, "LAB03"=w2641:T24, "LAB04"=w2640:T25, "array ERROR"=w2646:errorcluster[], "LAB05"=w2639:T26)  [unwired: 8 in]
                n1766 = stacked-sequence {
                  tunnel: w2646 -> [w2649 _ _ _ _ _]
                  tunnel: w2645 -> [w2648 _ _ _ _ _]
                  tunnel: w2644 -> [w2647 _ _ _ _ _]
                  tunnel: w2643 -> [_ w2694 _ _ _ _]
                  tunnel: w2642 -> [_ _ w2695 _ _ _]
                  tunnel: w2641 -> [_ _ _ w2720 _ _]
                  tunnel: w2640 -> [_ _ _ _ w2743 _]
                  tunnel: w2639 -> [_ _ _ _ _ w2768]
                  frame #0 {
                    n1767 = local write "AI update"(TRUE) -> ()
                    n1768 = Index Array(array=w2647, index=6) -> (element=→"LAB04-1 (GRAPH)":dynamicdata)
                    n1769 = Index Array(array=w2647, index=7) -> (element=→"LAB04-2 (GRAPH)":dynamicdata)
                    n1770 = Index Array(array=w2647, index=9) -> (element=→"LAB05-2 (GRAPH)":dynamicdata)
                    n1771 = Index Array(array=w2647, index=8) -> (element=→"LAB05-1 (GRAPH)":dynamicdata)
                    n1772 = Index Array(array=w2647, index=5) -> (element=→"LAB03-2 (GRAPH)":dynamicdata)
                    n1773 = Index Array(array=w2647, index=0) -> (element=→"LAB01-1 (GRAPH)":dynamicdata)
                    n1774 = Index Array(array=w2647, index=1) -> (element=→"LAB01-2 (GRAPH)":dynamicdata)
                    n1775 = Index Array(array=w2647, index=2) -> (element=→"LAB02-1 (GRAPH)":dynamicdata)
                    n1776 = Index Array(array=w2647, index=3) -> (element=→"LAB02-2 (GRAPH)":dynamicdata)
                    n1777 = Index Array(array=w2647, index=4) -> (element=→"LAB03-1 (GRAPH)":dynamicdata)
                    "AI loop time" <- w2648
                    "Analog Error Array" <- w2649
                  }
                  frame #1 {
                    n1778 = local read "CAL LAB01"() -> (w2693:T7)
                    n1779 = Unbundle By Name(w2694) -> ("LAB01-1 (A)"=w2692:dbl, "LAB01-1 (V)"=w2691:dbl, "LAB01-1 (PF)"=w2690:dbl, "LAB01-2 (A)"=w2689:dbl, "LAB01-2 (V)"=w2688:dbl, "LAB01-2 (PF)"=w2687:dbl)
                    n1780 = Unbundle By Name(w2693) -> ("1  (A) cal"=w2686:dbl, "1 (V) cal"=w2685:dbl, "1 (PF) cal"=w2684:dbl, "2 (A) cal"=w2683:dbl, "2 (V) cal"=w2682:dbl, "2 (PF) cal"=w2681:dbl)  [unwired: 4 out]
                    n1781 = Multiply(x=w2692, y=w2686) -> (x*y=w2679:dbl)
                    n1782 = Multiply(x=w2691, y=w2685) -> (x*y=w2678:dbl)
                    n1783 = Multiply(x=w2690, y=w2684) -> (x*y=w2677:dbl)
                    n1784 = Multiply(x=w2689, y=w2683) -> (x*y=w2673:dbl)
                    n1785 = Multiply(x=w2688, y=w2682) -> (x*y=w2672:dbl)
                    n1786 = Multiply(x=w2687, y=w2681) -> (x*y=w2671:dbl)
                    n1787 = local read "SIG LAB01-1"() -> (w2680:T2)
                    n1788 = local read "SIG LAB01-2"() -> (w2675:T2)
                    n1789 = Bundle By Name(cluster=w2680, "AMPS"=w2679, "VOLTS"=w2678, "PF"=w2677) -> (w2676:T2)
                    n1790 = Bundle By Name(cluster=w2675, "AMPS"=w2673, "VOLTS"=w2672, "PF"=w2671) -> (w2674:T2)
                    n1791 = local write "SIG LAB01-2"(w2674) -> ()
                    n1792 = local write "SIG LAB01-1"(w2676) -> ()
                  }
                  frame #2 {
                    n1793 = local read "CAL LAB02"() -> (w2718:T8)
                    n1794 = Unbundle By Name(w2695) -> ("LAB02-1 (A)"=w2717:dbl, "LAB02-1 (V)"=w2716:dbl, "LAB02-1 (PF)"=w2715:dbl, "LAB02-2 (A)"=w2714:dbl, "LAB02-2 (V)"=w2713:dbl, "LAB02-2 (PF)"=w2712:dbl)
                    n1795 = Unbundle By Name(w2718) -> ("1 (A) cal"=w2711:dbl, "1 (V) cal"=w2710:dbl, "1 (PF) cal"=w2709:dbl, "2 (A) cal"=w2708:dbl, "2 (V) cal"=w2707:dbl, "2 (PF) cal"=w2706:dbl)  [unwired: 4 out]
                    n1796 = Multiply(x=w2717, y=w2711) -> (x*y=w2704:dbl)
                    n1797 = Multiply(x=w2716, y=w2710) -> (x*y=w2703:dbl)
                    n1798 = Multiply(x=w2715, y=w2709) -> (x*y=w2702:dbl)
                    n1799 = Multiply(x=w2714, y=w2708) -> (x*y=w2698:dbl)
                    n1800 = Multiply(x=w2713, y=w2707) -> (x*y=w2697:dbl)
                    n1801 = Multiply(x=w2712, y=w2706) -> (x*y=w2696:dbl)
                    n1802 = local read "SIG LAB02-1"() -> (w2705:T2)
                    n1803 = local read "SIG LAB02-2"() -> (w2700:T2)
                    n1804 = Bundle By Name(cluster=w2705, "AMPS"=w2704, "VOLTS"=w2703, "PF"=w2702) -> (w2701:T2)
                    n1805 = Bundle By Name(cluster=w2700, "AMPS"=w2698, "VOLTS"=w2697, "PF"=w2696) -> (w2699:T2)
                    n1806 = local write "SIG LAB02-2"(w2699) -> ()
                    n1807 = local write "SIG LAB02-1"(w2701) -> ()
                  }
                  frame #3 {
                    n1808 = local read "CAL LAB03"() -> (w2742:T7)
                    n1809 = Unbundle By Name(w2720) -> ("LAB03-1 (A)"=w2741:dbl, "LAB03-1 (V)"=w2740:dbl, "LAB03-1 (PF)"=w2739:dbl, "LAB03-2 (A)"=w2738:dbl, "LAB03-2 (V)"=w2737:dbl, "LAB03-2 (PF)"=w2736:dbl)
                    n1810 = Unbundle By Name(w2742) -> ("1  (A) cal"=w2735:dbl, "1 (V) cal"=w2734:dbl, "1 (PF) cal"=w2733:dbl, "2 (A) cal"=w2732:dbl, "2 (V) cal"=w2731:dbl, "2 (PF) cal"=w2730:dbl)  [unwired: 4 out]
                    n1811 = Multiply(x=w2741, y=w2735) -> (x*y=w2728:dbl)
                    n1812 = Multiply(x=w2740, y=w2734) -> (x*y=w2719:dbl)
                    n1813 = Multiply(x=w2739, y=w2733) -> (x*y=w2727:dbl)
                    n1814 = Multiply(x=w2738, y=w2732) -> (x*y=w2723:dbl)
                    n1815 = Multiply(x=w2737, y=w2731) -> (x*y=w2722:dbl)
                    n1816 = Multiply(x=w2736, y=w2730) -> (x*y=w2721:dbl)
                    n1817 = local read "SIG LAB03-1"() -> (w2729:T2)
                    n1818 = local read "SIG LAB03-2"() -> (w2725:T2)
                    n1819 = Bundle By Name(cluster=w2729, "AMPS"=w2728, "VOLTS"=w2719, "PF"=w2727) -> (w2726:T2)
                    n1820 = Bundle By Name(cluster=w2725, "AMPS"=w2723, "VOLTS"=w2722, "PF"=w2721) -> (w2724:T2)
                    n1821 = local write "SIG LAB03-2"(w2724) -> ()
                    n1822 = local write "SIG LAB03-1"(w2726) -> ()
                  }
                  frame #4 {
                    n1823 = local read "CAL LAB04"() -> (w2766:T7)
                    n1824 = Unbundle By Name(w2743) -> ("LAB04-1 (A)"=w2765:dbl, "LAB04-1 (V)"=w2764:dbl, "LAB04-1 (PF)"=w2763:dbl, "LAB04-2 (A)"=w2762:dbl, "LAB04-2 (V)"=w2761:dbl, "LAB04-2 (PF)"=w2760:dbl)
                    n1825 = Unbundle By Name(w2766) -> ("1  (A) cal"=w2759:dbl, "1 (V) cal"=w2758:dbl, "1 (PF) cal"=w2757:dbl, "2 (A) cal"=w2756:dbl, "2 (V) cal"=w2755:dbl, "2 (PF) cal"=w2754:dbl)  [unwired: 4 out]
                    n1826 = Multiply(x=w2765, y=w2759) -> (x*y=w2752:dbl)
                    n1827 = Multiply(x=w2764, y=w2758) -> (x*y=w2751:dbl)
                    n1828 = Multiply(x=w2763, y=w2757) -> (x*y=w2750:dbl)
                    n1829 = Multiply(x=w2762, y=w2756) -> (x*y=w2746:dbl)
                    n1830 = Multiply(x=w2761, y=w2755) -> (x*y=w2745:dbl)
                    n1831 = Multiply(x=w2760, y=w2754) -> (x*y=w2744:dbl)
                    n1832 = local read "SIG LAB04-1"() -> (w2753:T2)
                    n1833 = local read "SIG LAB04-2"() -> (w2748:T2)
                    n1834 = Bundle By Name(cluster=w2753, "AMPS"=w2752, "VOLTS"=w2751, "PF"=w2750) -> (w2749:T2)
                    n1835 = Bundle By Name(cluster=w2748, "AMPS"=w2746, "VOLTS"=w2745, "PF"=w2744) -> (w2747:T2)
                    n1836 = local write "SIG LAB04-2"(w2747) -> ()
                    n1837 = local write "SIG LAB04-1"(w2749) -> ()
                  }
                  frame #5 {
                    n1838 = local read "CAL LAB05"() -> (w2790:T7)
                    n1839 = Unbundle By Name(w2768) -> ("LAB05-1 (A)"=w2789:dbl, "LAB05-1 (V)"=w2767:dbl, "LAB05-1 (PF)"=w2788:dbl, "LAB05-2 (A)"=w2787:dbl, "LAB05-2 (V)"=w2786:dbl, "LAB05-2 (PF)"=w2785:dbl)
                    n1840 = Unbundle By Name(w2790) -> ("1  (A) cal"=w2784:dbl, "1 (V) cal"=w2783:dbl, "1 (PF) cal"=w2782:dbl, "2 (A) cal"=w2781:dbl, "2 (V) cal"=w2780:dbl, "2 (PF) cal"=w2779:dbl)  [unwired: 4 out]
                    n1841 = Multiply(x=w2789, y=w2784) -> (x*y=w2777:dbl)
                    n1842 = Multiply(x=w2767, y=w2783) -> (x*y=w2776:dbl)
                    n1843 = Multiply(x=w2788, y=w2782) -> (x*y=w2775:dbl)
                    n1844 = Multiply(x=w2787, y=w2781) -> (x*y=w2771:dbl)
                    n1845 = Multiply(x=w2786, y=w2780) -> (x*y=w2770:dbl)
                    n1846 = Multiply(x=w2785, y=w2779) -> (x*y=w2769:dbl)
                    n1847 = local read "SIG LAB05-1"() -> (w2778:T2)
                    n1848 = local read "SIG LAB05-2"() -> (w2773:T2)
                    n1849 = Bundle By Name(cluster=w2778, "AMPS"=w2777, "VOLTS"=w2776, "PF"=w2775) -> (w2774:T2)
                    n1850 = Bundle By Name(cluster=w2773, "AMPS"=w2771, "VOLTS"=w2770, "PF"=w2769) -> (w2772:T2)
                    n1851 = local write "SIG LAB05-2"(w2772) -> ()
                    n1852 = local write "SIG LAB05-1"(w2774) -> ()
                  }
                }
              }
            }
          }
          frame #13 {
            # "save test data to file"
            n1853 = Get Date/Time In Seconds() -> (seconds since 1Jan1904=w2791:timestamp)
            "File Time Stamp" <- w2791
            n1854 = local read "on loops"() -> (w2810:dbl)
            n1855 = local read "jig cycle"() -> (w2807:dbl)
            n1856 = Format Date/Time String(time format string (%c)="%H:%M%:%S", seconds (now)=w2791) -> (date/time string=w2795:string)  [unwired: 1 in]
            n1857 = Add(x=w2810, y=2) -> (x+y=w2808:dbl)
            n1858 = Build Array(w2795) -> (w2794:string[])
            n1859 = Equal?(x=w2807, y=1) -> (x = y?=w2793:bool)
            n1860 = Equal?(x=w2807, y=w2808) -> (x = y?=w2792:bool)
            n1861 = stacked-sequence {
              tunnel: w2806 -> [w2816 _ _ _ _ _ _ _ _ _]
              tunnel: w2805 -> [_ w2892 _ _ _ _ _ _ _ _]
              tunnel: w2804 -> [_ _ w2972 _ _ _ _ _ _ _]
              tunnel: w2803 -> [_ _ _ w3052 _ _ _ _ _ _]
              tunnel: w2802 -> [_ _ _ _ w3132 _ _ _ _ _]
              tunnel: w2801 -> [_ _ _ _ _ w3212 _ _ _ _]
              tunnel: w2800 -> [_ _ _ _ _ _ w3292 _ _ _]
              tunnel: w2799 -> [_ _ _ _ _ _ _ w3372 _ _]
              tunnel: w2798 -> [_ _ _ _ _ _ _ _ w3452 _]
              tunnel: w2797 -> [_ _ _ _ _ _ _ _ _ w3532]
              tunnel: w2794 -> [w2815 w2896 w2976 w3056 w3136 w3216 w3296 w3376 w3456 w3536]
              tunnel: w2793 -> [w2814 w2895 w2975 w3055 w3135 w3215 w3295 w3375 w3455 w3535]
              tunnel: w2792 -> [w2813 w2894 w2974 w3054 w3134 w3214 w3294 w3374 w3454 w3534]
              tunnel: w2791 -> [w2812 w2893 w2973 w3053 w3133 w3213 w3293 w3373 w3453 w3533]
              frame #0 {
                n1862 = case shown="True" w2816 {
                  tunnel: w2815 -> [_ w2821]
                  tunnel: w2814 -> [_ w2820]
                  tunnel: w2813 -> [_ w2818]
                  tunnel: w2812 -> [_ w2817]
                  frame False {
                  }
                  frame True {
                    n1863 = local read "DISP LAB01-1"() -> (w2822:T4)
                    n1864 = local read "SIG LAB01-1"() -> (w2823:T2)
                    n1865 = local read "ON L01-1"() -> (w2819:cluster{"amps":dbl, "volts":dbl, "pf":dbl})
                    n1866 = Unbundle(w2823) -> ("AMPS"=w2829:dbl, "VOLTS"=w2827:dbl, "PF"=w2826:dbl, "Tmp Live"=w2825:dbl, "Tmp Neut"=w2828:dbl)
                    n1867 = Unbundle(w2822) -> ("CYCLE"=w2824:dbl)  [unwired: 2 out]
                    n1868 = stacked-sequence {
                      tunnel: w2829 -> [w2833 w2852]
                      tunnel: w2828 -> [_ w2851]
                      tunnel: w2827 -> [w2832 w2850]
                      tunnel: w2826 -> [w2831 w2849]
                      tunnel: w2825 -> [_ w2848]
                      tunnel: w2824 -> [_ w2847]
                      tunnel: w2821 -> [_ w2846]
                      tunnel: w2820 -> [w2834 _]
                      tunnel: w2819 -> [w2830 w2844]
                      tunnel: w2818 -> [_ w2845]
                      tunnel: w2817 -> [_ w2840]
                      frame #0 {
                        n1869 = case shown="True" w2834 {
                          tunnel: w2833 -> [_ w2839]
                          tunnel: w2832 -> [_ w2838]
                          tunnel: w2831 -> [_ w2837]
                          tunnel: w2830 -> [_ w2835]
                          frame False {
                          }
                          frame True {
                            n1870 = Bundle(cluster=w2835, "amps"=w2839, "volts"=w2838, "pf"=w2837) -> (w2836:cluster{"amps":dbl, "volts":dbl, "pf":dbl})
                            n1871 = local write "ON L01-1"(w2836) -> ()
                          }
                        }
                      }
                      frame #1 {
                        n1872 = Unbundle(w2844) -> ("amps"=w2843:dbl, "volts"=w2842:dbl, "pf"=w2841:dbl)
                        n1873 = case shown="True" w2845 {
                          tunnel: w2852 -> [_ w2853]
                          tunnel: w2851 -> [_ w2891]
                          tunnel: w2850 -> [_ _]
                          tunnel: w2849 -> [_ _]
                          tunnel: w2848 -> [_ w2890]
                          tunnel: w2847 -> [_ w2889]
                          tunnel: w2846 -> [_ w2857]
                          tunnel: w2843 -> [_ w2854]
                          tunnel: w2842 -> [_ w2886]
                          tunnel: w2841 -> [_ w2885]
                          tunnel: w2840 -> [_ w2855]
                          frame False {
                          }
                          frame True {
                            n1874 = local read "TDMS LAB01-1"() -> (w2888:refnum<k34>)
                            n1875 = Build Array(w2886) -> (w2882:dbl[])
                            n1876 = Build Array(w2885) -> (w2881:dbl[])
                            n1877 = Build Array(w2890) -> (w2880:dbl[])
                            n1878 = Build Array(w2891) -> (w2879:dbl[])
                            n1879 = Build Array(w2854) -> (w2884:dbl[])
                            n1880 = Build Array(w2853) -> (w2883:dbl[])
                            n1881 = Build Array(w2889) -> (w2878:dbl[])
                            n1882 = Build Array("AMPS ON", "AMPS OFF", "VOLTS", "PF", "TEMP Live", "TEMP Neut", "CYCLE") -> (w2862:string[])
                            n1883 = Bundle By Name("Y"=w2884, "t0"=w2855) -> (w2877:waveform(dbl))  [unwired: 1 in]
                            n1884 = Bundle By Name("Y"=w2883, "t0"=w2855) -> (w2876:waveform(dbl))  [unwired: 1 in]
                            n1885 = Bundle By Name("Y"=w2882, "t0"=w2855) -> (w2875:waveform(dbl))  [unwired: 1 in]
                            n1886 = Bundle By Name("Y"=w2881, "t0"=w2855) -> (w2874:waveform(dbl))  [unwired: 1 in]
                            n1887 = Bundle By Name("Y"=w2880, "t0"=w2855) -> (w2873:waveform(dbl))  [unwired: 1 in]
                            n1888 = Bundle By Name("Y"=w2879, "t0"=w2855) -> (w2872:waveform(dbl))  [unwired: 1 in]
                            n1889 = Bundle By Name("Y"=w2878, "t0"=w2855) -> (w2871:waveform(dbl))  [unwired: 1 in]
                            n1890 = Build Array(w2877, w2876, w2875, w2874, w2873, w2872, w2871) -> (w2870:waveform(dbl)[])
                            n1891 = TDMS Write(0:w2888, 5:"TEST VALUES", 7:w2862, 9:w2870) -> (4:w2861:refnum<k34>, 6:w2860:string, 15:w2859:errorcluster)  [unwired: 2 in, 1 out]
                            n1892 = TDMS Write(0:w2861, 5:w2860, 7:"TIME", 9:w2857, 11:w2859) -> (15:w2856:errorcluster)  [unwired: 1 in, 3 out]
                            n1893 = local write "data file error"(w2856) -> ()
                          }
                        }
                      }
                    }
                  }
                }
              }
              frame #1 {
                n1894 = case shown="True" w2892 {
                  tunnel: w2896 -> [_ w2901]
                  tunnel: w2895 -> [_ w2900]
                  tunnel: w2894 -> [_ w2898]
                  tunnel: w2893 -> [_ w2897]
                  frame False {
                  }
                  frame True {
                    n1895 = local read "DISP LAB01-2"() -> (w2902:T4)
                    n1896 = local read "SIG LAB01-2"() -> (w2903:T2)
                    n1897 = local read "ON L01-2"() -> (w2899:cluster{"amps":dbl, "volts":dbl, "pf":dbl})
                    n1898 = Unbundle(w2903) -> ("AMPS"=w2909:dbl, "VOLTS"=w2907:dbl, "PF"=w2906:dbl, "Tmp Live"=w2905:dbl, "Tmp Neut"=w2908:dbl)
                    n1899 = Unbundle(w2902) -> ("CYCLE"=w2904:dbl)  [unwired: 2 out]
                    n1900 = stacked-sequence {
                      tunnel: w2909 -> [w2913 w2932]
                      tunnel: w2908 -> [_ w2931]
                      tunnel: w2907 -> [w2912 w2930]
                      tunnel: w2906 -> [w2911 w2929]
                      tunnel: w2905 -> [_ w2928]
                      tunnel: w2904 -> [_ w2927]
                      tunnel: w2901 -> [_ w2926]
                      tunnel: w2900 -> [w2914 _]
                      tunnel: w2899 -> [w2910 w2924]
                      tunnel: w2898 -> [_ w2925]
                      tunnel: w2897 -> [_ w2920]
                      frame #0 {
                        n1901 = case shown="True" w2914 {
                          tunnel: w2913 -> [_ w2919]
                          tunnel: w2912 -> [_ w2918]
                          tunnel: w2911 -> [_ w2917]
                          tunnel: w2910 -> [_ w2915]
                          frame False {
                          }
                          frame True {
                            n1902 = Bundle(cluster=w2915, "amps"=w2919, "volts"=w2918, "pf"=w2917) -> (w2916:cluster{"amps":dbl, "volts":dbl, "pf":dbl})
                            n1903 = local write "ON L01-2"(w2916) -> ()
                          }
                        }
                      }
                      frame #1 {
                        n1904 = Unbundle(w2924) -> ("amps"=w2923:dbl, "volts"=w2922:dbl, "pf"=w2921:dbl)
                        n1905 = case shown="True" w2925 {
                          tunnel: w2932 -> [_ w2964]
                          tunnel: w2931 -> [_ w2971]
                          tunnel: w2930 -> [_ _]
                          tunnel: w2929 -> [_ _]
                          tunnel: w2928 -> [_ w2970]
                          tunnel: w2927 -> [_ w2969]
                          tunnel: w2926 -> [_ w2934]
                          tunnel: w2923 -> [_ w2966]
                          tunnel: w2922 -> [_ w2965]
                          tunnel: w2921 -> [_ w2963]
                          tunnel: w2920 -> [_ w2955]
                          frame False {
                          }
                          frame True {
                            n1906 = local read "TDMS LAB01-2"() -> (w2968:refnum<k34>)
                            n1907 = Build Array(w2965) -> (w2960:dbl[])
                            n1908 = Build Array(w2963) -> (w2959:dbl[])
                            n1909 = Build Array(w2970) -> (w2958:dbl[])
                            n1910 = Build Array(w2971) -> (w2957:dbl[])
                            n1911 = Build Array(w2966) -> (w2962:dbl[])
                            n1912 = Build Array(w2964) -> (w2961:dbl[])
                            n1913 = Build Array(w2969) -> (w2956:dbl[])
                            n1914 = Build Array("AMPS ON", "AMPS OFF", "VOLTS", "PF", "TEMP Live", "TEMP Neut", "CYCLE") -> (w2939:string[])
                            n1915 = Bundle By Name("Y"=w2962, "t0"=w2955) -> (w2954:waveform(dbl))  [unwired: 1 in]
                            n1916 = Bundle By Name("Y"=w2961, "t0"=w2955) -> (w2953:waveform(dbl))  [unwired: 1 in]
                            n1917 = Bundle By Name("Y"=w2960, "t0"=w2955) -> (w2952:waveform(dbl))  [unwired: 1 in]
                            n1918 = Bundle By Name("Y"=w2959, "t0"=w2955) -> (w2951:waveform(dbl))  [unwired: 1 in]
                            n1919 = Bundle By Name("Y"=w2958, "t0"=w2955) -> (w2950:waveform(dbl))  [unwired: 1 in]
                            n1920 = Bundle By Name("Y"=w2957, "t0"=w2955) -> (w2949:waveform(dbl))  [unwired: 1 in]
                            n1921 = Bundle By Name("Y"=w2956, "t0"=w2955) -> (w2948:waveform(dbl))  [unwired: 1 in]
                            n1922 = Build Array(w2954, w2953, w2952, w2951, w2950, w2949, w2948) -> (w2947:waveform(dbl)[])
                            n1923 = TDMS Write(0:w2968, 5:"TEST VALUES", 7:w2939, 9:w2947) -> (4:w2938:refnum<k34>, 6:w2937:string, 15:w2936:errorcluster)  [unwired: 2 in, 1 out]
                            n1924 = TDMS Write(0:w2938, 5:w2937, 7:"TIME", 9:w2934, 11:w2936) -> (15:w2933:errorcluster)  [unwired: 1 in, 3 out]
                            n1925 = local write "data file error"(w2933) -> ()
                          }
                        }
                      }
                    }
                  }
                }
              }
              frame #2 {
                n1926 = case shown="True" w2972 {
                  tunnel: w2976 -> [_ w2981]
                  tunnel: w2975 -> [_ w2980]
                  tunnel: w2974 -> [_ w2978]
                  tunnel: w2973 -> [_ w2977]
                  frame False {
                  }
                  frame True {
                    n1927 = local read "DISP LAB02-1"() -> (w2982:T4)
                    n1928 = local read "SIG LAB02-1"() -> (w2983:T2)
                    n1929 = local read "ON L02-1"() -> (w2979:cluster{"amps":dbl, "volts":dbl, "pf":dbl})
                    n1930 = Unbundle(w2983) -> ("AMPS"=w2989:dbl, "VOLTS"=w2987:dbl, "PF"=w2986:dbl, "Tmp Live"=w2985:dbl, "Tmp Neut"=w2988:dbl)
                    n1931 = Unbundle(w2982) -> ("CYCLE"=w2984:dbl)  [unwired: 2 out]
                    n1932 = stacked-sequence {
                      tunnel: w2989 -> [w2993 w3012]
                      tunnel: w2988 -> [_ w3011]
                      tunnel: w2987 -> [w2992 w3010]
                      tunnel: w2986 -> [w2991 w3009]
                      tunnel: w2985 -> [_ w3008]
                      tunnel: w2984 -> [_ w3007]
                      tunnel: w2981 -> [_ w3006]
                      tunnel: w2980 -> [w2994 _]
                      tunnel: w2979 -> [w2990 w3004]
                      tunnel: w2978 -> [_ w3005]
                      tunnel: w2977 -> [_ w3000]
                      frame #0 {
                        n1933 = case shown="True" w2994 {
                          tunnel: w2993 -> [_ w2999]
                          tunnel: w2992 -> [_ w2998]
                          tunnel: w2991 -> [_ w2997]
                          tunnel: w2990 -> [_ w2995]
                          frame False {
                          }
                          frame True {
                            n1934 = Bundle(cluster=w2995, "amps"=w2999, "volts"=w2998, "pf"=w2997) -> (w2996:cluster{"amps":dbl, "volts":dbl, "pf":dbl})
                            n1935 = local write "ON L02-1"(w2996) -> ()
                          }
                        }
                      }
                      frame #1 {
                        n1936 = Unbundle(w3004) -> ("amps"=w3003:dbl, "volts"=w3002:dbl, "pf"=w3001:dbl)
                        n1937 = case shown="True" w3005 {
                          tunnel: w3012 -> [_ w3044]
                          tunnel: w3011 -> [_ w3051]
                          tunnel: w3010 -> [_ _]
                          tunnel: w3009 -> [_ _]
                          tunnel: w3008 -> [_ w3050]
                          tunnel: w3007 -> [_ w3049]
                          tunnel: w3006 -> [_ w3014]
                          tunnel: w3003 -> [_ w3046]
                          tunnel: w3002 -> [_ w3045]
                          tunnel: w3001 -> [_ w3043]
                          tunnel: w3000 -> [_ w3035]
                          frame False {
                          }
                          frame True {
                            n1938 = local read "TDMS LAB02-1"() -> (w3048:refnum<k34>)
                            n1939 = Build Array(w3045) -> (w3040:dbl[])
                            n1940 = Build Array(w3043) -> (w3039:dbl[])
                            n1941 = Build Array(w3050) -> (w3038:dbl[])
                            n1942 = Build Array(w3051) -> (w3037:dbl[])
                            n1943 = Build Array(w3046) -> (w3042:dbl[])
                            n1944 = Build Array(w3044) -> (w3041:dbl[])
                            n1945 = Build Array(w3049) -> (w3036:dbl[])
                            n1946 = Build Array("AMPS ON", "AMPS OFF", "VOLTS", "PF", "TEMP Live", "TEMP Neut", "CYCLE") -> (w3019:string[])
                            n1947 = Bundle By Name("Y"=w3042, "t0"=w3035) -> (w3034:waveform(dbl))  [unwired: 1 in]
                            n1948 = Bundle By Name("Y"=w3041, "t0"=w3035) -> (w3033:waveform(dbl))  [unwired: 1 in]
                            n1949 = Bundle By Name("Y"=w3040, "t0"=w3035) -> (w3032:waveform(dbl))  [unwired: 1 in]
                            n1950 = Bundle By Name("Y"=w3039, "t0"=w3035) -> (w3031:waveform(dbl))  [unwired: 1 in]
                            n1951 = Bundle By Name("Y"=w3038, "t0"=w3035) -> (w3030:waveform(dbl))  [unwired: 1 in]
                            n1952 = Bundle By Name("Y"=w3037, "t0"=w3035) -> (w3029:waveform(dbl))  [unwired: 1 in]
                            n1953 = Bundle By Name("Y"=w3036, "t0"=w3035) -> (w3028:waveform(dbl))  [unwired: 1 in]
                            n1954 = Build Array(w3034, w3033, w3032, w3031, w3030, w3029, w3028) -> (w3027:waveform(dbl)[])
                            n1955 = TDMS Write(0:w3048, 5:"TEST VALUES", 7:w3019, 9:w3027) -> (4:w3018:refnum<k34>, 6:w3017:string, 15:w3016:errorcluster)  [unwired: 2 in, 1 out]
                            n1956 = TDMS Write(0:w3018, 5:w3017, 7:"TIME", 9:w3014, 11:w3016) -> (15:w3013:errorcluster)  [unwired: 1 in, 3 out]
                            n1957 = local write "data file error"(w3013) -> ()
                          }
                        }
                      }
                    }
                  }
                }
              }
              frame #3 {
                n1958 = case shown="True" w3052 {
                  tunnel: w3056 -> [_ w3061]
                  tunnel: w3055 -> [_ w3060]
                  tunnel: w3054 -> [_ w3058]
                  tunnel: w3053 -> [_ w3057]
                  frame False {
                  }
                  frame True {
                    n1959 = local read "DISP LAB02-2"() -> (w3062:T4)
                    n1960 = local read "SIG LAB02-2"() -> (w3063:T2)
                    n1961 = local read "ON L02-2"() -> (w3059:cluster{"amps":dbl, "volts":dbl, "pf":dbl})
                    n1962 = Unbundle(w3063) -> ("AMPS"=w3069:dbl, "VOLTS"=w3067:dbl, "PF"=w3066:dbl, "Tmp Live"=w3065:dbl, "Tmp Neut"=w3068:dbl)
                    n1963 = Unbundle(w3062) -> ("CYCLE"=w3064:dbl)  [unwired: 2 out]
                    n1964 = stacked-sequence {
                      tunnel: w3069 -> [w3073 w3092]
                      tunnel: w3068 -> [_ w3091]
                      tunnel: w3067 -> [w3072 w3090]
                      tunnel: w3066 -> [w3071 w3089]
                      tunnel: w3065 -> [_ w3088]
                      tunnel: w3064 -> [_ w3087]
                      tunnel: w3061 -> [_ w3086]
                      tunnel: w3060 -> [w3074 _]
                      tunnel: w3059 -> [w3070 w3084]
                      tunnel: w3058 -> [_ w3085]
                      tunnel: w3057 -> [_ w3080]
                      frame #0 {
                        n1965 = case shown="True" w3074 {
                          tunnel: w3073 -> [_ w3079]
                          tunnel: w3072 -> [_ w3078]
                          tunnel: w3071 -> [_ w3077]
                          tunnel: w3070 -> [_ w3075]
                          frame False {
                          }
                          frame True {
                            n1966 = Bundle(cluster=w3075, "amps"=w3079, "volts"=w3078, "pf"=w3077) -> (w3076:cluster{"amps":dbl, "volts":dbl, "pf":dbl})
                            n1967 = local write "ON L02-2"(w3076) -> ()
                          }
                        }
                      }
                      frame #1 {
                        n1968 = Unbundle(w3084) -> ("amps"=w3083:dbl, "volts"=w3082:dbl, "pf"=w3081:dbl)
                        n1969 = case shown="True" w3085 {
                          tunnel: w3092 -> [_ w3124]
                          tunnel: w3091 -> [_ w3131]
                          tunnel: w3090 -> [_ _]
                          tunnel: w3089 -> [_ _]
                          tunnel: w3088 -> [_ w3130]
                          tunnel: w3087 -> [_ w3129]
                          tunnel: w3086 -> [_ w3094]
                          tunnel: w3083 -> [_ w3126]
                          tunnel: w3082 -> [_ w3125]
                          tunnel: w3081 -> [_ w3123]
                          tunnel: w3080 -> [_ w3115]
                          frame False {
                          }
                          frame True {
                            n1970 = local read "TDMS LAB02-2"() -> (w3128:refnum<k34>)
                            n1971 = Build Array(w3125) -> (w3120:dbl[])
                            n1972 = Build Array(w3123) -> (w3119:dbl[])
                            n1973 = Build Array(w3130) -> (w3118:dbl[])
                            n1974 = Build Array(w3131) -> (w3117:dbl[])
                            n1975 = Build Array(w3126) -> (w3122:dbl[])
                            n1976 = Build Array(w3124) -> (w3121:dbl[])
                            n1977 = Build Array(w3129) -> (w3116:dbl[])
                            n1978 = Build Array("AMPS ON", "AMPS OFF", "VOLTS", "PF", "TEMP Live", "TEMP Neut", "CYCLE") -> (w3099:string[])
                            n1979 = Bundle By Name("Y"=w3122, "t0"=w3115) -> (w3114:waveform(dbl))  [unwired: 1 in]
                            n1980 = Bundle By Name("Y"=w3121, "t0"=w3115) -> (w3113:waveform(dbl))  [unwired: 1 in]
                            n1981 = Bundle By Name("Y"=w3120, "t0"=w3115) -> (w3112:waveform(dbl))  [unwired: 1 in]
                            n1982 = Bundle By Name("Y"=w3119, "t0"=w3115) -> (w3111:waveform(dbl))  [unwired: 1 in]
                            n1983 = Bundle By Name("Y"=w3118, "t0"=w3115) -> (w3110:waveform(dbl))  [unwired: 1 in]
                            n1984 = Bundle By Name("Y"=w3117, "t0"=w3115) -> (w3109:waveform(dbl))  [unwired: 1 in]
                            n1985 = Bundle By Name("Y"=w3116, "t0"=w3115) -> (w3108:waveform(dbl))  [unwired: 1 in]
                            n1986 = Build Array(w3114, w3113, w3112, w3111, w3110, w3109, w3108) -> (w3107:waveform(dbl)[])
                            n1987 = TDMS Write(0:w3128, 5:"TEST VALUES", 7:w3099, 9:w3107) -> (4:w3098:refnum<k34>, 6:w3097:string, 15:w3096:errorcluster)  [unwired: 2 in, 1 out]
                            n1988 = TDMS Write(0:w3098, 5:w3097, 7:"TIME", 9:w3094, 11:w3096) -> (15:w3093:errorcluster)  [unwired: 1 in, 3 out]
                            n1989 = local write "data file error"(w3093) -> ()
                          }
                        }
                      }
                    }
                  }
                }
              }
              frame #4 {
                n1990 = case shown="True" w3132 {
                  tunnel: w3136 -> [_ w3141]
                  tunnel: w3135 -> [_ w3140]
                  tunnel: w3134 -> [_ w3138]
                  tunnel: w3133 -> [_ w3137]
                  frame False {
                  }
                  frame True {
                    n1991 = local read "DISP LAB03-1"() -> (w3142:T4)
                    n1992 = local read "SIG LAB03-1"() -> (w3143:T2)
                    n1993 = local read "ON L03-1"() -> (w3139:cluster{"amps":dbl, "volts":dbl, "pf":dbl})
                    n1994 = Unbundle(w3143) -> ("AMPS"=w3149:dbl, "VOLTS"=w3147:dbl, "PF"=w3146:dbl, "Tmp Live"=w3145:dbl, "Tmp Neut"=w3148:dbl)
                    n1995 = Unbundle(w3142) -> ("CYCLE"=w3144:dbl)  [unwired: 2 out]
                    n1996 = stacked-sequence {
                      tunnel: w3149 -> [w3153 w3172]
                      tunnel: w3148 -> [_ w3171]
                      tunnel: w3147 -> [w3152 w3170]
                      tunnel: w3146 -> [w3151 w3169]
                      tunnel: w3145 -> [_ w3168]
                      tunnel: w3144 -> [_ w3167]
                      tunnel: w3141 -> [_ w3166]
                      tunnel: w3140 -> [w3154 _]
                      tunnel: w3139 -> [w3150 w3164]
                      tunnel: w3138 -> [_ w3165]
                      tunnel: w3137 -> [_ w3160]
                      frame #0 {
                        n1997 = case shown="True" w3154 {
                          tunnel: w3153 -> [_ w3159]
                          tunnel: w3152 -> [_ w3158]
                          tunnel: w3151 -> [_ w3157]
                          tunnel: w3150 -> [_ w3155]
                          frame False {
                          }
                          frame True {
                            n1998 = Bundle(cluster=w3155, "amps"=w3159, "volts"=w3158, "pf"=w3157) -> (w3156:cluster{"amps":dbl, "volts":dbl, "pf":dbl})
                            n1999 = local write "ON L03-1"(w3156) -> ()
                          }
                        }
                      }
                      frame #1 {
                        n2000 = Unbundle(w3164) -> ("amps"=w3163:dbl, "volts"=w3162:dbl, "pf"=w3161:dbl)
                        n2001 = case shown="True" w3165 {
                          tunnel: w3172 -> [_ w3204]
                          tunnel: w3171 -> [_ w3211]
                          tunnel: w3170 -> [_ _]
                          tunnel: w3169 -> [_ _]
                          tunnel: w3168 -> [_ w3210]
                          tunnel: w3167 -> [_ w3209]
                          tunnel: w3166 -> [_ w3174]
                          tunnel: w3163 -> [_ w3206]
                          tunnel: w3162 -> [_ w3205]
                          tunnel: w3161 -> [_ w3203]
                          tunnel: w3160 -> [_ w3195]
                          frame False {
                          }
                          frame True {
                            n2002 = local read "TDMS LAB03-1"() -> (w3208:refnum<k34>)
                            n2003 = Build Array(w3205) -> (w3200:dbl[])
                            n2004 = Build Array(w3203) -> (w3199:dbl[])
                            n2005 = Build Array(w3210) -> (w3198:dbl[])
                            n2006 = Build Array(w3211) -> (w3197:dbl[])
                            n2007 = Build Array(w3206) -> (w3202:dbl[])
                            n2008 = Build Array(w3204) -> (w3201:dbl[])
                            n2009 = Build Array(w3209) -> (w3196:dbl[])
                            n2010 = Build Array("AMPS ON", "AMPS OFF", "VOLTS", "PF", "TEMP Live", "TEMP Neut", "CYCLE") -> (w3179:string[])
                            n2011 = Bundle By Name("Y"=w3202, "t0"=w3195) -> (w3194:waveform(dbl))  [unwired: 1 in]
                            n2012 = Bundle By Name("Y"=w3201, "t0"=w3195) -> (w3193:waveform(dbl))  [unwired: 1 in]
                            n2013 = Bundle By Name("Y"=w3200, "t0"=w3195) -> (w3192:waveform(dbl))  [unwired: 1 in]
                            n2014 = Bundle By Name("Y"=w3199, "t0"=w3195) -> (w3191:waveform(dbl))  [unwired: 1 in]
                            n2015 = Bundle By Name("Y"=w3198, "t0"=w3195) -> (w3190:waveform(dbl))  [unwired: 1 in]
                            n2016 = Bundle By Name("Y"=w3197, "t0"=w3195) -> (w3189:waveform(dbl))  [unwired: 1 in]
                            n2017 = Bundle By Name("Y"=w3196, "t0"=w3195) -> (w3188:waveform(dbl))  [unwired: 1 in]
                            n2018 = Build Array(w3194, w3193, w3192, w3191, w3190, w3189, w3188) -> (w3187:waveform(dbl)[])
                            n2019 = TDMS Write(0:w3208, 5:"TEST VALUES", 7:w3179, 9:w3187) -> (4:w3178:refnum<k34>, 6:w3177:string, 15:w3176:errorcluster)  [unwired: 2 in, 1 out]
                            n2020 = TDMS Write(0:w3178, 5:w3177, 7:"TIME", 9:w3174, 11:w3176) -> (15:w3173:errorcluster)  [unwired: 1 in, 3 out]
                            n2021 = local write "data file error"(w3173) -> ()
                          }
                        }
                      }
                    }
                  }
                }
              }
              frame #5 {
                n2022 = case shown="True" w3212 {
                  tunnel: w3216 -> [_ w3221]
                  tunnel: w3215 -> [_ w3220]
                  tunnel: w3214 -> [_ w3218]
                  tunnel: w3213 -> [_ w3217]
                  frame False {
                  }
                  frame True {
                    n2023 = local read "DISP LAB03-2"() -> (w3222:T4)
                    n2024 = local read "SIG LAB03-2"() -> (w3223:T2)
                    n2025 = local read "ON L03-2"() -> (w3219:cluster{"amps":dbl, "volts":dbl, "pf":dbl})
                    n2026 = Unbundle(w3223) -> ("AMPS"=w3229:dbl, "VOLTS"=w3227:dbl, "PF"=w3226:dbl, "Tmp Live"=w3225:dbl, "Tmp Neut"=w3228:dbl)
                    n2027 = Unbundle(w3222) -> ("CYCLE"=w3224:dbl)  [unwired: 2 out]
                    n2028 = stacked-sequence {
                      tunnel: w3229 -> [w3233 w3252]
                      tunnel: w3228 -> [_ w3251]
                      tunnel: w3227 -> [w3232 w3250]
                      tunnel: w3226 -> [w3231 w3249]
                      tunnel: w3225 -> [_ w3248]
                      tunnel: w3224 -> [_ w3247]
                      tunnel: w3221 -> [_ w3246]
                      tunnel: w3220 -> [w3234 _]
                      tunnel: w3219 -> [w3230 w3244]
                      tunnel: w3218 -> [_ w3245]
                      tunnel: w3217 -> [_ w3240]
                      frame #0 {
                        n2029 = case shown="True" w3234 {
                          tunnel: w3233 -> [_ w3239]
                          tunnel: w3232 -> [_ w3238]
                          tunnel: w3231 -> [_ w3237]
                          tunnel: w3230 -> [_ w3235]
                          frame False {
                          }
                          frame True {
                            n2030 = Bundle(cluster=w3235, "amps"=w3239, "volts"=w3238, "pf"=w3237) -> (w3236:cluster{"amps":dbl, "volts":dbl, "pf":dbl})
                            n2031 = local write "ON L03-2"(w3236) -> ()
                          }
                        }
                      }
                      frame #1 {
                        n2032 = Unbundle(w3244) -> ("amps"=w3243:dbl, "volts"=w3242:dbl, "pf"=w3241:dbl)
                        n2033 = case shown="True" w3245 {
                          tunnel: w3252 -> [_ w3284]
                          tunnel: w3251 -> [_ w3291]
                          tunnel: w3250 -> [_ _]
                          tunnel: w3249 -> [_ _]
                          tunnel: w3248 -> [_ w3290]
                          tunnel: w3247 -> [_ w3289]
                          tunnel: w3246 -> [_ w3254]
                          tunnel: w3243 -> [_ w3286]
                          tunnel: w3242 -> [_ w3285]
                          tunnel: w3241 -> [_ w3283]
                          tunnel: w3240 -> [_ w3275]
                          frame False {
                          }
                          frame True {
                            n2034 = local read "TDMS LAB03-2"() -> (w3288:refnum<k34>)
                            n2035 = Build Array(w3285) -> (w3280:dbl[])
                            n2036 = Build Array(w3283) -> (w3279:dbl[])
                            n2037 = Build Array(w3290) -> (w3278:dbl[])
                            n2038 = Build Array(w3291) -> (w3277:dbl[])
                            n2039 = Build Array(w3286) -> (w3282:dbl[])
                            n2040 = Build Array(w3284) -> (w3281:dbl[])
                            n2041 = Build Array(w3289) -> (w3276:dbl[])
                            n2042 = Build Array("AMPS ON", "AMPS OFF", "VOLTS", "PF", "TEMP Live", "TEMP Neut", "CYCLE") -> (w3259:string[])
                            n2043 = Bundle By Name("Y"=w3282, "t0"=w3275) -> (w3274:waveform(dbl))  [unwired: 1 in]
                            n2044 = Bundle By Name("Y"=w3281, "t0"=w3275) -> (w3273:waveform(dbl))  [unwired: 1 in]
                            n2045 = Bundle By Name("Y"=w3280, "t0"=w3275) -> (w3272:waveform(dbl))  [unwired: 1 in]
                            n2046 = Bundle By Name("Y"=w3279, "t0"=w3275) -> (w3271:waveform(dbl))  [unwired: 1 in]
                            n2047 = Bundle By Name("Y"=w3278, "t0"=w3275) -> (w3270:waveform(dbl))  [unwired: 1 in]
                            n2048 = Bundle By Name("Y"=w3277, "t0"=w3275) -> (w3269:waveform(dbl))  [unwired: 1 in]
                            n2049 = Bundle By Name("Y"=w3276, "t0"=w3275) -> (w3268:waveform(dbl))  [unwired: 1 in]
                            n2050 = Build Array(w3274, w3273, w3272, w3271, w3270, w3269, w3268) -> (w3267:waveform(dbl)[])
                            n2051 = TDMS Write(0:w3288, 5:"TEST VALUES", 7:w3259, 9:w3267) -> (4:w3258:refnum<k34>, 6:w3257:string, 15:w3256:errorcluster)  [unwired: 2 in, 1 out]
                            n2052 = TDMS Write(0:w3258, 5:w3257, 7:"TIME", 9:w3254, 11:w3256) -> (15:w3253:errorcluster)  [unwired: 1 in, 3 out]
                            n2053 = local write "data file error"(w3253) -> ()
                          }
                        }
                      }
                    }
                  }
                }
              }
              frame #6 {
                n2054 = case shown="True" w3292 {
                  tunnel: w3296 -> [_ w3301]
                  tunnel: w3295 -> [_ w3300]
                  tunnel: w3294 -> [_ w3298]
                  tunnel: w3293 -> [_ w3297]
                  frame False {
                  }
                  frame True {
                    n2055 = local read "DISP LAB04-1"() -> (w3302:T4)
                    n2056 = local read "SIG LAB04-1"() -> (w3303:T2)
                    n2057 = local read "ON L04-1"() -> (w3299:cluster{"amps":dbl, "volts":dbl, "pf":dbl})
                    n2058 = Unbundle(w3303) -> ("AMPS"=w3309:dbl, "VOLTS"=w3307:dbl, "PF"=w3306:dbl, "Tmp Live"=w3305:dbl, "Tmp Neut"=w3308:dbl)
                    n2059 = Unbundle(w3302) -> ("CYCLE"=w3304:dbl)  [unwired: 2 out]
                    n2060 = stacked-sequence {
                      tunnel: w3309 -> [w3313 w3332]
                      tunnel: w3308 -> [_ w3331]
                      tunnel: w3307 -> [w3312 w3330]
                      tunnel: w3306 -> [w3311 w3329]
                      tunnel: w3305 -> [_ w3328]
                      tunnel: w3304 -> [_ w3327]
                      tunnel: w3301 -> [_ w3326]
                      tunnel: w3300 -> [w3314 _]
                      tunnel: w3299 -> [w3310 w3324]
                      tunnel: w3298 -> [_ w3325]
                      tunnel: w3297 -> [_ w3320]
                      frame #0 {
                        n2061 = case shown="True" w3314 {
                          tunnel: w3313 -> [_ w3319]
                          tunnel: w3312 -> [_ w3318]
                          tunnel: w3311 -> [_ w3317]
                          tunnel: w3310 -> [_ w3315]
                          frame False {
                          }
                          frame True {
                            n2062 = Bundle(cluster=w3315, "amps"=w3319, "volts"=w3318, "pf"=w3317) -> (w3316:cluster{"amps":dbl, "volts":dbl, "pf":dbl})
                            n2063 = local write "ON L04-1"(w3316) -> ()
                          }
                        }
                      }
                      frame #1 {
                        n2064 = Unbundle(w3324) -> ("amps"=w3323:dbl, "volts"=w3322:dbl, "pf"=w3321:dbl)
                        n2065 = case shown="True" w3325 {
                          tunnel: w3332 -> [_ w3364]
                          tunnel: w3331 -> [_ w3371]
                          tunnel: w3330 -> [_ _]
                          tunnel: w3329 -> [_ _]
                          tunnel: w3328 -> [_ w3370]
                          tunnel: w3327 -> [_ w3369]
                          tunnel: w3326 -> [_ w3334]
                          tunnel: w3323 -> [_ w3366]
                          tunnel: w3322 -> [_ w3365]
                          tunnel: w3321 -> [_ w3363]
                          tunnel: w3320 -> [_ w3355]
                          frame False {
                          }
                          frame True {
                            n2066 = local read "TDMS LAB04-1"() -> (w3368:refnum<k34>)
                            n2067 = Build Array(w3365) -> (w3360:dbl[])
                            n2068 = Build Array(w3363) -> (w3359:dbl[])
                            n2069 = Build Array(w3370) -> (w3358:dbl[])
                            n2070 = Build Array(w3371) -> (w3357:dbl[])
                            n2071 = Build Array(w3366) -> (w3362:dbl[])
                            n2072 = Build Array(w3364) -> (w3361:dbl[])
                            n2073 = Build Array(w3369) -> (w3356:dbl[])
                            n2074 = Build Array("AMPS ON", "AMPS OFF", "VOLTS", "PF", "TEMP Live", "TEMP Neut", "CYCLE") -> (w3339:string[])
                            n2075 = Bundle By Name("Y"=w3362, "t0"=w3355) -> (w3354:waveform(dbl))  [unwired: 1 in]
                            n2076 = Bundle By Name("Y"=w3361, "t0"=w3355) -> (w3353:waveform(dbl))  [unwired: 1 in]
                            n2077 = Bundle By Name("Y"=w3360, "t0"=w3355) -> (w3352:waveform(dbl))  [unwired: 1 in]
                            n2078 = Bundle By Name("Y"=w3359, "t0"=w3355) -> (w3351:waveform(dbl))  [unwired: 1 in]
                            n2079 = Bundle By Name("Y"=w3358, "t0"=w3355) -> (w3350:waveform(dbl))  [unwired: 1 in]
                            n2080 = Bundle By Name("Y"=w3357, "t0"=w3355) -> (w3349:waveform(dbl))  [unwired: 1 in]
                            n2081 = Bundle By Name("Y"=w3356, "t0"=w3355) -> (w3348:waveform(dbl))  [unwired: 1 in]
                            n2082 = Build Array(w3354, w3353, w3352, w3351, w3350, w3349, w3348) -> (w3347:waveform(dbl)[])
                            n2083 = TDMS Write(0:w3368, 5:"TEST VALUES", 7:w3339, 9:w3347) -> (4:w3338:refnum<k34>, 6:w3337:string, 15:w3336:errorcluster)  [unwired: 2 in, 1 out]
                            n2084 = TDMS Write(0:w3338, 5:w3337, 7:"TIME", 9:w3334, 11:w3336) -> (15:w3333:errorcluster)  [unwired: 1 in, 3 out]
                            n2085 = local write "data file error"(w3333) -> ()
                          }
                        }
                      }
                    }
                  }
                }
              }
              frame #7 {
                n2086 = case shown="True" w3372 {
                  tunnel: w3376 -> [_ w3381]
                  tunnel: w3375 -> [_ w3380]
                  tunnel: w3374 -> [_ w3378]
                  tunnel: w3373 -> [_ w3377]
                  frame False {
                  }
                  frame True {
                    n2087 = local read "DISP LAB04-2"() -> (w3382:T4)
                    n2088 = local read "SIG LAB04-2"() -> (w3383:T2)
                    n2089 = local read "ON L04-2"() -> (w3379:cluster{"amps":dbl, "volts":dbl, "pf":dbl})
                    n2090 = Unbundle(w3383) -> ("AMPS"=w3389:dbl, "VOLTS"=w3387:dbl, "PF"=w3386:dbl, "Tmp Live"=w3385:dbl, "Tmp Neut"=w3388:dbl)
                    n2091 = Unbundle(w3382) -> ("CYCLE"=w3384:dbl)  [unwired: 2 out]
                    n2092 = stacked-sequence {
                      tunnel: w3389 -> [w3393 w3412]
                      tunnel: w3388 -> [_ w3411]
                      tunnel: w3387 -> [w3392 w3410]
                      tunnel: w3386 -> [w3391 w3409]
                      tunnel: w3385 -> [_ w3408]
                      tunnel: w3384 -> [_ w3407]
                      tunnel: w3381 -> [_ w3406]
                      tunnel: w3380 -> [w3394 _]
                      tunnel: w3379 -> [w3390 w3404]
                      tunnel: w3378 -> [_ w3405]
                      tunnel: w3377 -> [_ w3400]
                      frame #0 {
                        n2093 = case shown="True" w3394 {
                          tunnel: w3393 -> [_ w3399]
                          tunnel: w3392 -> [_ w3398]
                          tunnel: w3391 -> [_ w3397]
                          tunnel: w3390 -> [_ w3395]
                          frame False {
                          }
                          frame True {
                            n2094 = Bundle(cluster=w3395, "amps"=w3399, "volts"=w3398, "pf"=w3397) -> (w3396:cluster{"amps":dbl, "volts":dbl, "pf":dbl})
                            n2095 = local write "ON L04-2"(w3396) -> ()
                          }
                        }
                      }
                      frame #1 {
                        n2096 = Unbundle(w3404) -> ("amps"=w3403:dbl, "volts"=w3402:dbl, "pf"=w3401:dbl)
                        n2097 = case shown="True" w3405 {
                          tunnel: w3412 -> [_ w3444]
                          tunnel: w3411 -> [_ w3451]
                          tunnel: w3410 -> [_ _]
                          tunnel: w3409 -> [_ _]
                          tunnel: w3408 -> [_ w3450]
                          tunnel: w3407 -> [_ w3449]
                          tunnel: w3406 -> [_ w3414]
                          tunnel: w3403 -> [_ w3446]
                          tunnel: w3402 -> [_ w3445]
                          tunnel: w3401 -> [_ w3443]
                          tunnel: w3400 -> [_ w3435]
                          frame False {
                          }
                          frame True {
                            n2098 = local read "TDMS LAB04-2"() -> (w3448:refnum<k34>)
                            n2099 = Build Array(w3445) -> (w3440:dbl[])
                            n2100 = Build Array(w3443) -> (w3439:dbl[])
                            n2101 = Build Array(w3450) -> (w3438:dbl[])
                            n2102 = Build Array(w3451) -> (w3437:dbl[])
                            n2103 = Build Array(w3446) -> (w3442:dbl[])
                            n2104 = Build Array(w3444) -> (w3441:dbl[])
                            n2105 = Build Array(w3449) -> (w3436:dbl[])
                            n2106 = Build Array("AMPS ON", "AMPS OFF", "VOLTS", "PF", "TEMP Live", "TEMP Neut", "CYCLE") -> (w3419:string[])
                            n2107 = Bundle By Name("Y"=w3442, "t0"=w3435) -> (w3434:waveform(dbl))  [unwired: 1 in]
                            n2108 = Bundle By Name("Y"=w3441, "t0"=w3435) -> (w3433:waveform(dbl))  [unwired: 1 in]
                            n2109 = Bundle By Name("Y"=w3440, "t0"=w3435) -> (w3432:waveform(dbl))  [unwired: 1 in]
                            n2110 = Bundle By Name("Y"=w3439, "t0"=w3435) -> (w3431:waveform(dbl))  [unwired: 1 in]
                            n2111 = Bundle By Name("Y"=w3438, "t0"=w3435) -> (w3430:waveform(dbl))  [unwired: 1 in]
                            n2112 = Bundle By Name("Y"=w3437, "t0"=w3435) -> (w3429:waveform(dbl))  [unwired: 1 in]
                            n2113 = Bundle By Name("Y"=w3436, "t0"=w3435) -> (w3428:waveform(dbl))  [unwired: 1 in]
                            n2114 = Build Array(w3434, w3433, w3432, w3431, w3430, w3429, w3428) -> (w3427:waveform(dbl)[])
                            n2115 = TDMS Write(0:w3448, 5:"TEST VALUES", 7:w3419, 9:w3427) -> (4:w3418:refnum<k34>, 6:w3417:string, 15:w3416:errorcluster)  [unwired: 2 in, 1 out]
                            n2116 = TDMS Write(0:w3418, 5:w3417, 7:"TIME", 9:w3414, 11:w3416) -> (15:w3413:errorcluster)  [unwired: 1 in, 3 out]
                            n2117 = local write "data file error"(w3413) -> ()
                          }
                        }
                      }
                    }
                  }
                }
              }
              frame #8 {
                n2118 = case shown="True" w3452 {
                  tunnel: w3456 -> [_ w3461]
                  tunnel: w3455 -> [_ w3460]
                  tunnel: w3454 -> [_ w3458]
                  tunnel: w3453 -> [_ w3457]
                  frame False {
                  }
                  frame True {
                    n2119 = local read "DISP LAB05-1"() -> (w3462:T4)
                    n2120 = local read "SIG LAB05-1"() -> (w3463:T2)
                    n2121 = local read "ON L05-1"() -> (w3459:cluster{"amps":dbl, "volts":dbl, "pf":dbl})
                    n2122 = Unbundle(w3463) -> ("AMPS"=w3469:dbl, "VOLTS"=w3467:dbl, "PF"=w3466:dbl, "Tmp Live"=w3465:dbl, "Tmp Neut"=w3468:dbl)
                    n2123 = Unbundle(w3462) -> ("CYCLE"=w3464:dbl)  [unwired: 2 out]
                    n2124 = stacked-sequence {
                      tunnel: w3469 -> [w3473 w3492]
                      tunnel: w3468 -> [_ w3491]
                      tunnel: w3467 -> [w3472 w3490]
                      tunnel: w3466 -> [w3471 w3489]
                      tunnel: w3465 -> [_ w3488]
                      tunnel: w3464 -> [_ w3487]
                      tunnel: w3461 -> [_ w3486]
                      tunnel: w3460 -> [w3474 _]
                      tunnel: w3459 -> [w3470 w3484]
                      tunnel: w3458 -> [_ w3485]
                      tunnel: w3457 -> [_ w3480]
                      frame #0 {
                        n2125 = case shown="True" w3474 {
                          tunnel: w3473 -> [_ w3479]
                          tunnel: w3472 -> [_ w3478]
                          tunnel: w3471 -> [_ w3477]
                          tunnel: w3470 -> [_ w3475]
                          frame False {
                          }
                          frame True {
                            n2126 = Bundle(cluster=w3475, "amps"=w3479, "volts"=w3478, "pf"=w3477) -> (w3476:cluster{"amps":dbl, "volts":dbl, "pf":dbl})
                            n2127 = local write "ON L05-1"(w3476) -> ()
                          }
                        }
                      }
                      frame #1 {
                        n2128 = Unbundle(w3484) -> ("amps"=w3483:dbl, "volts"=w3482:dbl, "pf"=w3481:dbl)
                        n2129 = case shown="True" w3485 {
                          tunnel: w3492 -> [_ w3524]
                          tunnel: w3491 -> [_ w3531]
                          tunnel: w3490 -> [_ _]
                          tunnel: w3489 -> [_ _]
                          tunnel: w3488 -> [_ w3530]
                          tunnel: w3487 -> [_ w3529]
                          tunnel: w3486 -> [_ w3494]
                          tunnel: w3483 -> [_ w3526]
                          tunnel: w3482 -> [_ w3525]
                          tunnel: w3481 -> [_ w3523]
                          tunnel: w3480 -> [_ w3515]
                          frame False {
                          }
                          frame True {
                            n2130 = local read "TDMS LAB05-1"() -> (w3528:refnum<k34>)
                            n2131 = Build Array(w3525) -> (w3520:dbl[])
                            n2132 = Build Array(w3523) -> (w3519:dbl[])
                            n2133 = Build Array(w3530) -> (w3518:dbl[])
                            n2134 = Build Array(w3531) -> (w3517:dbl[])
                            n2135 = Build Array(w3526) -> (w3522:dbl[])
                            n2136 = Build Array(w3524) -> (w3521:dbl[])
                            n2137 = Build Array(w3529) -> (w3516:dbl[])
                            n2138 = Build Array("AMPS ON", "AMPS OFF", "VOLTS", "PF", "TEMP Live", "TEMP Neut", "CYCLE") -> (w3499:string[])
                            n2139 = Bundle By Name("Y"=w3522, "t0"=w3515) -> (w3514:waveform(dbl))  [unwired: 1 in]
                            n2140 = Bundle By Name("Y"=w3521, "t0"=w3515) -> (w3513:waveform(dbl))  [unwired: 1 in]
                            n2141 = Bundle By Name("Y"=w3520, "t0"=w3515) -> (w3512:waveform(dbl))  [unwired: 1 in]
                            n2142 = Bundle By Name("Y"=w3519, "t0"=w3515) -> (w3511:waveform(dbl))  [unwired: 1 in]
                            n2143 = Bundle By Name("Y"=w3518, "t0"=w3515) -> (w3510:waveform(dbl))  [unwired: 1 in]
                            n2144 = Bundle By Name("Y"=w3517, "t0"=w3515) -> (w3509:waveform(dbl))  [unwired: 1 in]
                            n2145 = Bundle By Name("Y"=w3516, "t0"=w3515) -> (w3508:waveform(dbl))  [unwired: 1 in]
                            n2146 = Build Array(w3514, w3513, w3512, w3511, w3510, w3509, w3508) -> (w3507:waveform(dbl)[])
                            n2147 = TDMS Write(0:w3528, 5:"TEST VALUES", 7:w3499, 9:w3507) -> (4:w3498:refnum<k34>, 6:w3497:string, 15:w3496:errorcluster)  [unwired: 2 in, 1 out]
                            n2148 = TDMS Write(0:w3498, 5:w3497, 7:"TIME", 9:w3494, 11:w3496) -> (15:w3493:errorcluster)  [unwired: 1 in, 3 out]
                            n2149 = local write "data file error"(w3493) -> ()
                          }
                        }
                      }
                    }
                  }
                }
              }
              frame #9 {
                n2150 = case shown="True" w3532 {
                  tunnel: w3536 -> [_ w3541]
                  tunnel: w3535 -> [_ w3540]
                  tunnel: w3534 -> [_ w3538]
                  tunnel: w3533 -> [_ w3537]
                  frame False {
                  }
                  frame True {
                    n2151 = local read "DISP LAB05-2"() -> (w3542:T4)
                    n2152 = local read "SIG LAB05-2"() -> (w3543:T2)
                    n2153 = local read "ON L05-2"() -> (w3539:cluster{"amps":dbl, "volts":dbl, "pf":dbl})
                    n2154 = Unbundle(w3543) -> ("AMPS"=w3549:dbl, "VOLTS"=w3547:dbl, "PF"=w3546:dbl, "Tmp Live"=w3545:dbl, "Tmp Neut"=w3548:dbl)
                    n2155 = Unbundle(w3542) -> ("CYCLE"=w3544:dbl)  [unwired: 2 out]
                    n2156 = stacked-sequence {
                      tunnel: w3549 -> [w3553 w3572]
                      tunnel: w3548 -> [_ w3571]
                      tunnel: w3547 -> [w3552 w3570]
                      tunnel: w3546 -> [w3551 w3569]
                      tunnel: w3545 -> [_ w3568]
                      tunnel: w3544 -> [_ w3567]
                      tunnel: w3541 -> [_ w3566]
                      tunnel: w3540 -> [w3554 _]
                      tunnel: w3539 -> [w3550 w3564]
                      tunnel: w3538 -> [_ w3565]
                      tunnel: w3537 -> [_ w3560]
                      frame #0 {
                        n2157 = case shown="True" w3554 {
                          tunnel: w3553 -> [_ w3559]
                          tunnel: w3552 -> [_ w3558]
                          tunnel: w3551 -> [_ w3557]
                          tunnel: w3550 -> [_ w3555]
                          frame False {
                          }
                          frame True {
                            n2158 = Bundle(cluster=w3555, "amps"=w3559, "volts"=w3558, "pf"=w3557) -> (w3556:cluster{"amps":dbl, "volts":dbl, "pf":dbl})
                            n2159 = local write "ON L05-2"(w3556) -> ()
                          }
                        }
                      }
                      frame #1 {
                        n2160 = Unbundle(w3564) -> ("amps"=w3563:dbl, "volts"=w3562:dbl, "pf"=w3561:dbl)
                        n2161 = case shown="True" w3565 {
                          tunnel: w3572 -> [_ w3604]
                          tunnel: w3571 -> [_ w3611]
                          tunnel: w3570 -> [_ _]
                          tunnel: w3569 -> [_ _]
                          tunnel: w3568 -> [_ w3610]
                          tunnel: w3567 -> [_ w3609]
                          tunnel: w3566 -> [_ w3574]
                          tunnel: w3563 -> [_ w3606]
                          tunnel: w3562 -> [_ w3605]
                          tunnel: w3561 -> [_ w3603]
                          tunnel: w3560 -> [_ w3595]
                          frame False {
                          }
                          frame True {
                            n2162 = local read "TDMS LAB05-2"() -> (w3608:refnum<k34>)
                            n2163 = Build Array(w3605) -> (w3600:dbl[])
                            n2164 = Build Array(w3603) -> (w3599:dbl[])
                            n2165 = Build Array(w3610) -> (w3598:dbl[])
                            n2166 = Build Array(w3611) -> (w3597:dbl[])
                            n2167 = Build Array(w3606) -> (w3602:dbl[])
                            n2168 = Build Array(w3604) -> (w3601:dbl[])
                            n2169 = Build Array(w3609) -> (w3596:dbl[])
                            n2170 = Build Array("AMPS ON", "AMPS OFF", "VOLTS", "PF", "TEMP Live", "TEMP Neut", "CYCLE") -> (w3579:string[])
                            n2171 = Bundle By Name("Y"=w3602, "t0"=w3595) -> (w3594:waveform(dbl))  [unwired: 1 in]
                            n2172 = Bundle By Name("Y"=w3601, "t0"=w3595) -> (w3593:waveform(dbl))  [unwired: 1 in]
                            n2173 = Bundle By Name("Y"=w3600, "t0"=w3595) -> (w3592:waveform(dbl))  [unwired: 1 in]
                            n2174 = Bundle By Name("Y"=w3599, "t0"=w3595) -> (w3591:waveform(dbl))  [unwired: 1 in]
                            n2175 = Bundle By Name("Y"=w3598, "t0"=w3595) -> (w3590:waveform(dbl))  [unwired: 1 in]
                            n2176 = Bundle By Name("Y"=w3597, "t0"=w3595) -> (w3589:waveform(dbl))  [unwired: 1 in]
                            n2177 = Bundle By Name("Y"=w3596, "t0"=w3595) -> (w3588:waveform(dbl))  [unwired: 1 in]
                            n2178 = Build Array(w3594, w3593, w3592, w3591, w3590, w3589, w3588) -> (w3587:waveform(dbl)[])
                            n2179 = TDMS Write(0:w3608, 5:"TEST VALUES", 7:w3579, 9:w3587) -> (4:w3578:refnum<k34>, 6:w3577:string, 15:w3576:errorcluster)  [unwired: 2 in, 1 out]
                            n2180 = TDMS Write(0:w3578, 5:w3577, 7:"TIME", 9:w3574, 11:w3576) -> (15:w3573:errorcluster)  [unwired: 1 in, 3 out]
                            n2181 = local write "data file error"(w3573) -> ()
                          }
                        }
                      }
                    }
                  }
                }
              }
            }
          }
          frame #14 {
            # "display test values on chart"
            n2182 = case shown="\"OFF CYCLE\"" "Select  Cycle" {
              tunnel: [1 w3617] -> w3612
              frame "ON CYCLE", Default {
              }
              frame "OFF CYCLE" {
                n2183 = local read "on loops"() -> (w3619:dbl)
                n2184 = Add(x=w3619, y=2) -> (x+y=w3617:dbl)
              }
            }
            n2185 = local read "jig cycle"() -> (w3614:dbl)
            n2186 = Equal?(x=w3614, y=w3612) -> (x = y?=w3615:bool)
            n2187 = case shown="True" w3615 {
              frame False {
              }
              frame True {
                n2188 = local read "SIG LAB05-1"() -> (w3643:T2)
                n2189 = local read "SIG LAB05-2"() -> (w3642:T2)
                n2190 = local read "SIG LAB04-2"() -> (w3644:T2)
                n2191 = local read "SIG LAB02-2"() -> (w3648:T2)
                n2192 = local read "SIG LAB04-1"() -> (w3645:T2)
                n2193 = local read "SIG LAB02-1"() -> (w3649:T2)
                n2194 = local read "SIG LAB01-1"() -> (w3651:T2)
                n2195 = local read "SIG LAB03-2"() -> (w3646:T2)
                n2196 = local read "SIG LAB01-2"() -> (w3650:T2)
                n2197 = local read "SIG LAB03-1"() -> (w3647:T2)
                n2198 = Unbundle(w3642) -> ("AMPS"=w3636:dbl, "VOLTS"=w3621:dbl)  [unwired: 3 out]
                n2199 = Unbundle(w3644) -> ("AMPS"=w3634:dbl, "VOLTS"=w3623:dbl)  [unwired: 3 out]
                n2200 = Unbundle(w3643) -> ("AMPS"=w3635:dbl, "VOLTS"=w3622:dbl)  [unwired: 3 out]
                n2201 = Unbundle(w3645) -> ("AMPS"=w3633:dbl, "VOLTS"=w3624:dbl)  [unwired: 3 out]
                n2202 = Unbundle(w3647) -> ("AMPS"=w3637:dbl, "VOLTS"=w3626:dbl)  [unwired: 3 out]
                n2203 = Unbundle(w3646) -> ("AMPS"=w3632:dbl, "VOLTS"=w3625:dbl)  [unwired: 3 out]
                n2204 = Unbundle(w3649) -> ("AMPS"=w3639:dbl, "VOLTS"=w3628:dbl)  [unwired: 3 out]
                n2205 = Unbundle(w3648) -> ("AMPS"=w3638:dbl, "VOLTS"=w3627:dbl)  [unwired: 3 out]
                n2206 = Unbundle(w3650) -> ("AMPS"=w3640:dbl, "VOLTS"=w3629:dbl)  [unwired: 3 out]
                n2207 = Unbundle(w3651) -> ("AMPS"=w3641:dbl, "VOLTS"=w3630:dbl)  [unwired: 3 out]
                n2208 = Bundle("AMPS"=w3641, "AMPS"=w3640, "AMPS"=w3639, "AMPS"=w3638, "AMPS"=w3637, "AMPS"=w3632, "AMPS"=w3633, "AMPS"=w3634, "AMPS"=w3635, "AMPS"=w3636) -> (→"TEST AMPS CHART":T9)  [unwired: 1 in]
                n2209 = Bundle("VOLTS"=w3630, "VOLTS"=w3629, "VOLTS"=w3628, "VOLTS"=w3627, "VOLTS"=w3626, "VOLTS"=w3625, "VOLTS"=w3624, "VOLTS"=w3623, "VOLTS"=w3622, "VOLTS"=w3621) -> (→"TEST VOLTS CHART":T27)  [unwired: 1 in]
              }
            }
          }
          frame #15 {
            # "check for amps fail"
            # "check for cycle test & temperature rise fail conditions"
            n2210 = local read "on loops"() -> (w3677:dbl)
            n2211 = local read "jig cycle"() -> (w3674:dbl)
            n2212 = local read "jig cycle"() -> (w3679:dbl)
            n2213 = Add(x=w3677, y=3.0) -> (x+y=w3675:dbl)
            n2214 = Equal?(x=w3674, y=w3675) -> (x = y?=w3670:bool)
            n2215 = Equal?(x=w3679, y=1.0) -> (x = y?=w3672:bool)
            n2216 = stacked-sequence {
              tunnel: w3673 -> [w3682 _ _ _ _ _ _ _ _ _]
              tunnel: w3672 -> [w3683 w3703 w3723 w3743 w3763 w3783 w3803 w3823 w3843 w3863]
              tunnel: w3671 -> [w3680 _ _ _ _ _ _ _ _ _]
              tunnel: w3670 -> [w3681 w3702 w3722 w3742 w3762 w3782 w3802 w3822 w3842 w3862]
              tunnel: w3669 -> [_ w3701 _ _ _ _ _ _ _ _]
              tunnel: w3668 -> [_ w3700 _ _ _ _ _ _ _ _]
              tunnel: w3667 -> [_ _ w3721 _ _ _ _ _ _ _]
              tunnel: w3666 -> [_ _ w3720 _ _ _ _ _ _ _]
              tunnel: w3665 -> [_ _ _ w3741 _ _ _ _ _ _]
              tunnel: w3664 -> [_ _ _ w3740 _ _ _ _ _ _]
              tunnel: w3663 -> [_ _ _ _ w3761 _ _ _ _ _]
              tunnel: w3662 -> [_ _ _ _ w3760 _ _ _ _ _]
              tunnel: w3661 -> [_ _ _ _ _ w3781 _ _ _ _]
              tunnel: w3660 -> [_ _ _ _ _ w3780 _ _ _ _]
              tunnel: w3659 -> [_ _ _ _ _ _ w3801 _ _ _]
              tunnel: w3658 -> [_ _ _ _ _ _ w3800 _ _ _]
              tunnel: w3657 -> [_ _ _ _ _ _ _ w3821 _ _]
              tunnel: w3656 -> [_ _ _ _ _ _ _ w3820 _ _]
              tunnel: w3655 -> [_ _ _ _ _ _ _ _ w3841 _]
              tunnel: w3654 -> [_ _ _ _ _ _ _ _ w3840 _]
              tunnel: w3653 -> [_ _ _ _ _ _ _ _ _ w3861]
              tunnel: w3652 -> [_ _ _ _ _ _ _ _ _ w3860]
              frame #0 {
                # "LAB01-1"
                n2217 = case shown="True" w3680 {
                  tunnel: w3683 -> [_ w3696]
                  tunnel: w3682 -> [_ w3693]
                  tunnel: w3681 -> [_ w3692]
                  frame False {
                  }
                  frame True {
                    n2218 = local read "TEMP START LAB01-1"() -> (w3698:cluster{"TL":dbl, "TN":dbl})
                    n2219 = local read "RESULT LAB01-1"() -> (w3687:bool)
                    n2220 = local read "FAIL LAB01-1"() -> (w3690:cluster{"LO":dbl, "HI":dbl})
                    n2221 = local read "TDMS LAB01-1"() -> (w3697:refnum<k34>)
                    n2222 = local read "SET LAB01-1"() -> (w3694:T5)
                    n2223 = local read "DISP LAB01-1"() -> (w3695:T4)
                    n2224 = local read "SIG LAB01-1"() -> (w3699:T2)
                    n2225 = Bundle("FAIL LAB01-1"=w3690, "SIG LAB01-1"=w3699, "TEMP START LAB01-1"=w3698, "DISP LAB01-1"=w3695, "SET LAB01-1"=w3694, "TDMS LAB01-1"=w3697) -> (w3684:T28)  [unwired: 1 in]
                    n2226 = call "sub vi - cycle&temp fail v6.vi"("Amps Lo?"=w3696, "Input Cluster"=w3684, "SELECT"=w3693, "Amps Hi?"=w3692, "Result In"=w3687) -> ("(FAIL) out"=w3689:cluster{"FAIL LO":dbl, "FAIL HI":dbl}, "(DISP) out"=w3685:T4, "T-RISE"=w3686:cluster{"T-RISE (L)":dbl, "T-RISE (N)":dbl}, "Result Out"=w3688:bool, "file error"=w3691:errorcluster)  [unwired: 10 in]
                    n2227 = local write "TEMP RISE LAB01-1"(w3686) -> ()
                    n2228 = local write "FAIL LAB01-1"(w3689) -> ()
                    n2229 = local write "DISP LAB01-1"(w3685) -> ()
                    n2230 = local write "RESULT LAB01-1"(w3688) -> ()
                    n2231 = local write "data file error"(w3691) -> ()
                  }
                }
              }
              frame #1 {
                # "LAB01-2"
                n2232 = case shown="True" w3701 {
                  tunnel: w3703 -> [_ w3716]
                  tunnel: w3700 -> [_ w3713]
                  tunnel: w3702 -> [_ w3712]
                  frame False {
                  }
                  frame True {
                    n2233 = local read "TEMP START LAB01-2"() -> (w3718:cluster{"TL":dbl, "TN":dbl})
                    n2234 = local read "FAIL LAB01-2"() -> (w3709:cluster{"LO":dbl, "HI":dbl})
                    n2235 = local read "TDMS LAB01-2"() -> (w3717:refnum<k34>)
                    n2236 = local read "SET LAB01-2"() -> (w3714:T5)
                    n2237 = local read "DISP LAB01-2"() -> (w3715:T4)
                    n2238 = local read "RESULT LAB01-2"() -> (w3706:bool)
                    n2239 = local read "SIG LAB01-2"() -> (w3719:T2)
                    n2240 = Bundle("FAIL LAB01-2"=w3709, "SIG LAB01-2"=w3719, "TEMP START LAB01-2"=w3718, "DISP LAB01-2"=w3715, "SET LAB01-2"=w3714, "TDMS LAB01-2"=w3717) -> (w3704:T29)  [unwired: 1 in]
                    n2241 = call "sub vi - cycle&temp fail v6.vi"("Amps Lo?"=w3716, "Input Cluster"=w3704, "SELECT"=w3713, "Amps Hi?"=w3712, "Result In"=w3706) -> ("(FAIL) out"=w3708:cluster{"FAIL LO":dbl, "FAIL HI":dbl}, "(DISP) out"=w3711:T4, "T-RISE"=w3705:cluster{"T-RISE (L)":dbl, "T-RISE (N)":dbl}, "Result Out"=w3707:bool, "file error"=w3710:errorcluster)  [unwired: 10 in]
                    n2242 = local write "TEMP RISE LAB01-2"(w3705) -> ()
                    n2243 = local write "FAIL LAB01-2"(w3708) -> ()
                    n2244 = local write "DISP LAB01-2"(w3711) -> ()
                    n2245 = local write "RESULT LAB01-2"(w3707) -> ()
                    n2246 = local write "data file error"(w3710) -> ()
                  }
                }
              }
              frame #2 {
                # "LAB02-1"
                n2247 = case shown="True" w3721 {
                  tunnel: w3723 -> [_ w3736]
                  tunnel: w3720 -> [_ w3733]
                  tunnel: w3722 -> [_ w3732]
                  frame False {
                  }
                  frame True {
                    n2248 = local read "TEMP START LAB02-1"() -> (w3738:cluster{"TL":dbl, "TN":dbl})
                    n2249 = local read "FAIL LAB02-1"() -> (w3729:cluster{"LO":dbl, "HI":dbl})
                    n2250 = local read "TDMS LAB02-1"() -> (w3737:refnum<k34>)
                    n2251 = local read "SET LAB02-1"() -> (w3734:T5)
                    n2252 = local read "DISP LAB02-1"() -> (w3735:T4)
                    n2253 = local read "SIG LAB02-1"() -> (w3739:T2)
                    n2254 = local read "RESULT LAB02-1"() -> (w3726:bool)
                    n2255 = Bundle("FAIL LAB02-1"=w3729, "SIG LAB02-1"=w3739, "TEMP START LAB02-1"=w3738, "DISP LAB02-1"=w3735, "SET LAB02-1"=w3734, "TDMS LAB02-1"=w3737) -> (w3724:T30)  [unwired: 1 in]
                    n2256 = call "sub vi - cycle&temp fail v6.vi"("Amps Lo?"=w3736, "Input Cluster"=w3724, "SELECT"=w3733, "Amps Hi?"=w3732, "Result In"=w3726) -> ("(FAIL) out"=w3728:cluster{"FAIL LO":dbl, "FAIL HI":dbl}, "(DISP) out"=w3731:T4, "T-RISE"=w3725:cluster{"T-RISE (L)":dbl, "T-RISE (N)":dbl}, "Result Out"=w3727:bool, "file error"=w3730:errorcluster)  [unwired: 10 in]
                    n2257 = local write "TEMP RISE LAB02-1"(w3725) -> ()
                    n2258 = local write "FAIL LAB02-1"(w3728) -> ()
                    n2259 = local write "DISP LAB02-1"(w3731) -> ()
                    n2260 = local write "RESULT LAB02-1"(w3727) -> ()
                    n2261 = local write "data file error"(w3730) -> ()
                  }
                }
              }
              frame #3 {
                # "LAB02-2"
                n2262 = case shown="True" w3741 {
                  tunnel: w3743 -> [_ w3756]
                  tunnel: w3740 -> [_ w3753]
                  tunnel: w3742 -> [_ w3752]
                  frame False {
                  }
                  frame True {
                    n2263 = local read "TEMP START LAB02-2"() -> (w3758:cluster{"TL":dbl, "TN":dbl})
                    n2264 = local read "FAIL LAB02-2"() -> (w3749:cluster{"LO":dbl, "HI":dbl})
                    n2265 = local read "TDMS LAB02-2"() -> (w3757:refnum<k34>)
                    n2266 = local read "SET LAB02-2"() -> (w3754:T5)
                    n2267 = local read "DISP LAB02-2"() -> (w3755:T4)
                    n2268 = local read "SIG LAB02-2"() -> (w3759:T2)
                    n2269 = local read "RESULT LAB02-2"() -> (w3746:bool)
                    n2270 = Bundle("FAIL LAB02-2"=w3749, "SIG LAB02-2"=w3759, "TEMP START LAB02-2"=w3758, "DISP LAB02-2"=w3755, "SET LAB02-2"=w3754, "TDMS LAB02-2"=w3757) -> (w3744:T31)  [unwired: 1 in]
                    n2271 = call "sub vi - cycle&temp fail v6.vi"("Amps Lo?"=w3756, "Input Cluster"=w3744, "SELECT"=w3753, "Amps Hi?"=w3752, "Result In"=w3746) -> ("(FAIL) out"=w3748:cluster{"FAIL LO":dbl, "FAIL HI":dbl}, "(DISP) out"=w3751:T4, "T-RISE"=w3745:cluster{"T-RISE (L)":dbl, "T-RISE (N)":dbl}, "Result Out"=w3747:bool, "file error"=w3750:errorcluster)  [unwired: 10 in]
                    n2272 = local write "TEMP RISE LAB02-2"(w3745) -> ()
                    n2273 = local write "FAIL LAB02-2"(w3748) -> ()
                    n2274 = local write "DISP LAB02-2"(w3751) -> ()
                    n2275 = local write "RESULT LAB02-2"(w3747) -> ()
                    n2276 = local write "data file error"(w3750) -> ()
                  }
                }
              }
              frame #4 {
                # "LAB03-1"
                n2277 = case shown="True" w3761 {
                  tunnel: w3763 -> [_ w3776]
                  tunnel: w3760 -> [_ w3773]
                  tunnel: w3762 -> [_ w3772]
                  frame False {
                  }
                  frame True {
                    n2278 = local read "TEMP START LAB03-1"() -> (w3778:cluster{"TL":dbl, "TN":dbl})
                    n2279 = local read "FAIL LAB03-1"() -> (w3769:cluster{"LO":dbl, "HI":dbl})
                    n2280 = local read "TDMS LAB03-1"() -> (w3777:refnum<k34>)
                    n2281 = local read "SET LAB03-1"() -> (w3774:T5)
                    n2282 = local read "DISP LAB03-1"() -> (w3775:T4)
                    n2283 = local read "SIG LAB03-1"() -> (w3779:T2)
                    n2284 = local read "RESULT LAB03-1"() -> (w3766:bool)
                    n2285 = Bundle("FAIL LAB03-1"=w3769, "SIG LAB03-1"=w3779, "TEMP START LAB03-1"=w3778, "DISP LAB03-1"=w3775, "SET LAB03-1"=w3774, "TDMS LAB03-1"=w3777) -> (w3764:T32)  [unwired: 1 in]
                    n2286 = call "sub vi - cycle&temp fail v6.vi"("Amps Lo?"=w3776, "Input Cluster"=w3764, "SELECT"=w3773, "Amps Hi?"=w3772, "Result In"=w3766) -> ("(FAIL) out"=w3768:cluster{"FAIL LO":dbl, "FAIL HI":dbl}, "(DISP) out"=w3771:T4, "T-RISE"=w3765:cluster{"T-RISE (L)":dbl, "T-RISE (N)":dbl}, "Result Out"=w3767:bool, "file error"=w3770:errorcluster)  [unwired: 10 in]
                    n2287 = local write "TEMP RISE LAB03-1"(w3765) -> ()
                    n2288 = local write "FAIL LAB03-1"(w3768) -> ()
                    n2289 = local write "DISP LAB03-1"(w3771) -> ()
                    n2290 = local write "RESULT LAB03-1"(w3767) -> ()
                    n2291 = local write "data file error"(w3770) -> ()
                  }
                }
              }
              frame #5 {
                # "LAB03-2"
                n2292 = case shown="True" w3781 {
                  tunnel: w3783 -> [_ w3796]
                  tunnel: w3780 -> [_ w3793]
                  tunnel: w3782 -> [_ w3792]
                  frame False {
                  }
                  frame True {
                    n2293 = local read "TEMP START LAB03-2"() -> (w3798:cluster{"TL":dbl, "TN":dbl})
                    n2294 = local read "FAIL LAB03-2"() -> (w3789:cluster{"LO":dbl, "HI":dbl})
                    n2295 = local read "TDMS LAB03-2"() -> (w3797:refnum<k34>)
                    n2296 = local read "SET LAB03-2"() -> (w3794:T5)
                    n2297 = local read "DISP LAB03-2"() -> (w3795:T4)
                    n2298 = local read "RESULT LAB03-2"() -> (w3786:bool)
                    n2299 = local read "SIG LAB03-2"() -> (w3799:T2)
                    n2300 = Bundle("FAIL LAB03-2"=w3789, "SIG LAB03-2"=w3799, "TEMP START LAB03-2"=w3798, "DISP LAB03-2"=w3795, "SET LAB03-2"=w3794, "TDMS LAB03-2"=w3797) -> (w3784:T33)  [unwired: 1 in]
                    n2301 = call "sub vi - cycle&temp fail v6.vi"("Amps Lo?"=w3796, "Input Cluster"=w3784, "SELECT"=w3793, "Amps Hi?"=w3792, "Result In"=w3786) -> ("(FAIL) out"=w3788:cluster{"FAIL LO":dbl, "FAIL HI":dbl}, "(DISP) out"=w3791:T4, "T-RISE"=w3785:cluster{"T-RISE (L)":dbl, "T-RISE (N)":dbl}, "Result Out"=w3787:bool, "file error"=w3790:errorcluster)  [unwired: 10 in]
                    n2302 = local write "FAIL LAB03-2"(w3788) -> ()
                    n2303 = local write "TEMP RISE LAB03-2"(w3785) -> ()
                    n2304 = local write "DISP LAB03-2"(w3791) -> ()
                    n2305 = local write "RESULT LAB03-2"(w3787) -> ()
                    n2306 = local write "data file error"(w3790) -> ()
                  }
                }
              }
              frame #6 {
                # "LAB04-1"
                n2307 = case shown="True" w3801 {
                  tunnel: w3803 -> [_ w3816]
                  tunnel: w3800 -> [_ w3813]
                  tunnel: w3802 -> [_ w3812]
                  frame False {
                  }
                  frame True {
                    n2308 = local read "TEMP START LAB04-1"() -> (w3818:cluster{"TL":dbl, "TN":dbl})
                    n2309 = local read "FAIL LAB04-1"() -> (w3809:cluster{"LO":dbl, "HI":dbl})
                    n2310 = local read "TDMS LAB04-1"() -> (w3817:refnum<k34>)
                    n2311 = local read "SET LAB04-1"() -> (w3814:T5)
                    n2312 = local read "DISP LAB04-1"() -> (w3815:T4)
                    n2313 = local read "SIG LAB04-1"() -> (w3819:T2)
                    n2314 = local read "RESULT LAB04-1"() -> (w3806:bool)
                    n2315 = Bundle("FAIL LAB04-1"=w3809, "SIG LAB04-1"=w3819, "TEMP START LAB04-1"=w3818, "DISP LAB04-1"=w3815, "SET LAB04-1"=w3814, "TDMS LAB04-1"=w3817) -> (w3804:T34)  [unwired: 1 in]
                    n2316 = call "sub vi - cycle&temp fail v6.vi"("Amps Lo?"=w3816, "Input Cluster"=w3804, "SELECT"=w3813, "Amps Hi?"=w3812, "Result In"=w3806) -> ("(FAIL) out"=w3808:cluster{"FAIL LO":dbl, "FAIL HI":dbl}, "(DISP) out"=w3811:T4, "T-RISE"=w3805:cluster{"T-RISE (L)":dbl, "T-RISE (N)":dbl}, "Result Out"=w3807:bool, "file error"=w3810:errorcluster)  [unwired: 10 in]
                    n2317 = local write "TEMP RISE LAB04-1"(w3805) -> ()
                    n2318 = local write "FAIL LAB04-1"(w3808) -> ()
                    n2319 = local write "DISP LAB04-1"(w3811) -> ()
                    n2320 = local write "RESULT LAB04-1"(w3807) -> ()
                    n2321 = local write "data file error"(w3810) -> ()
                  }
                }
              }
              frame #7 {
                # "LAB04-2"
                n2322 = case shown="True" w3821 {
                  tunnel: w3823 -> [_ w3836]
                  tunnel: w3820 -> [_ w3833]
                  tunnel: w3822 -> [_ w3832]
                  frame False {
                  }
                  frame True {
                    n2323 = local read "TEMP START LAB04-2"() -> (w3838:cluster{"TL":dbl, "TN":dbl})
                    n2324 = local read "FAIL LAB04-2"() -> (w3829:cluster{"LO":dbl, "HI":dbl})
                    n2325 = local read "TDMS LAB04-2"() -> (w3837:refnum<k34>)
                    n2326 = local read "SET LAB04-2"() -> (w3834:T5)
                    n2327 = local read "DISP LAB04-2"() -> (w3835:T4)
                    n2328 = local read "SIG LAB04-2"() -> (w3839:T2)
                    n2329 = local read "RESULT LAB04-2"() -> (w3826:bool)
                    n2330 = Bundle("FAIL LAB04-2"=w3829, "SIG LAB04-2"=w3839, "TEMP START LAB04-2"=w3838, "DISP LAB04-2"=w3835, "SET LAB04-2"=w3834, "TDMS LAB04-2"=w3837) -> (w3824:T35)  [unwired: 1 in]
                    n2331 = call "sub vi - cycle&temp fail v6.vi"("Amps Lo?"=w3836, "Input Cluster"=w3824, "SELECT"=w3833, "Amps Hi?"=w3832, "Result In"=w3826) -> ("(FAIL) out"=w3828:cluster{"FAIL LO":dbl, "FAIL HI":dbl}, "(DISP) out"=w3831:T4, "T-RISE"=w3825:cluster{"T-RISE (L)":dbl, "T-RISE (N)":dbl}, "Result Out"=w3827:bool, "file error"=w3830:errorcluster)  [unwired: 10 in]
                    n2332 = local write "TEMP RISE LAB04-2"(w3825) -> ()
                    n2333 = local write "FAIL LAB04-2"(w3828) -> ()
                    n2334 = local write "DISP LAB04-2"(w3831) -> ()
                    n2335 = local write "RESULT LAB04-2"(w3827) -> ()
                    n2336 = local write "data file error"(w3830) -> ()
                  }
                }
              }
              frame #8 {
                # "LAB05-1"
                n2337 = case shown="True" w3841 {
                  tunnel: w3843 -> [_ w3856]
                  tunnel: w3840 -> [_ w3853]
                  tunnel: w3842 -> [_ w3852]
                  frame False {
                  }
                  frame True {
                    n2338 = local read "TEMP START LAB05-1"() -> (w3858:cluster{"TL":dbl, "TN":dbl})
                    n2339 = local read "FAIL LAB05-1"() -> (w3849:cluster{"LO":dbl, "HI":dbl})
                    n2340 = local read "TDMS LAB05-1"() -> (w3857:refnum<k34>)
                    n2341 = local read "SET LAB05-1"() -> (w3854:T5)
                    n2342 = local read "DISP LAB05-1"() -> (w3855:T4)
                    n2343 = local read "SIG LAB05-1"() -> (w3859:T2)
                    n2344 = local read "RESULT LAB05-1"() -> (w3846:bool)
                    n2345 = Bundle("FAIL LAB05-1"=w3849, "SIG LAB05-1"=w3859, "TEMP START LAB05-1"=w3858, "DISP LAB05-1"=w3855, "SET LAB05-1"=w3854, "TDMS LAB05-1"=w3857) -> (w3844:T36)  [unwired: 1 in]
                    n2346 = call "sub vi - cycle&temp fail v6.vi"("Amps Lo?"=w3856, "Input Cluster"=w3844, "SELECT"=w3853, "Amps Hi?"=w3852, "Result In"=w3846) -> ("(FAIL) out"=w3848:cluster{"FAIL LO":dbl, "FAIL HI":dbl}, "(DISP) out"=w3851:T4, "T-RISE"=w3845:cluster{"T-RISE (L)":dbl, "T-RISE (N)":dbl}, "Result Out"=w3847:bool, "file error"=w3850:errorcluster)  [unwired: 10 in]
                    n2347 = local write "TEMP RISE LAB05-1"(w3845) -> ()
                    n2348 = local write "FAIL LAB05-1"(w3848) -> ()
                    n2349 = local write "DISP LAB05-1"(w3851) -> ()
                    n2350 = local write "RESULT LAB05-1"(w3847) -> ()
                    n2351 = local write "data file error"(w3850) -> ()
                  }
                }
              }
              frame #9 {
                # "LAB05-2"
                n2352 = case shown="True" w3861 {
                  tunnel: w3863 -> [_ w3876]
                  tunnel: w3860 -> [_ w3873]
                  tunnel: w3862 -> [_ w3872]
                  frame False {
                  }
                  frame True {
                    n2353 = local read "TEMP START LAB05-2"() -> (w3878:cluster{"TL":dbl, "TN":dbl})
                    n2354 = local read "FAIL LAB05-2"() -> (w3869:cluster{"LO":dbl, "HI":dbl})
                    n2355 = local read "TDMS LAB05-2"() -> (w3877:refnum<k34>)
                    n2356 = local read "SET LAB05-2"() -> (w3874:T5)
                    n2357 = local read "DISP LAB05-2"() -> (w3875:T4)
                    n2358 = local read "SIG LAB05-2"() -> (w3879:T2)
                    n2359 = local read "RESULT LAB05-2"() -> (w3866:bool)
                    n2360 = Bundle("FAIL LAB05-2"=w3869, "SIG LAB05-2"=w3879, "TEMP START LAB05-2"=w3878, "DISP LAB05-2"=w3875, "SET LAB05-2"=w3874, "TDMS LAB05-2"=w3877) -> (w3864:T37)  [unwired: 1 in]
                    n2361 = call "sub vi - cycle&temp fail v6.vi"("Amps Lo?"=w3876, "Input Cluster"=w3864, "SELECT"=w3873, "Amps Hi?"=w3872, "Result In"=w3866) -> ("(FAIL) out"=w3868:cluster{"FAIL LO":dbl, "FAIL HI":dbl}, "(DISP) out"=w3871:T4, "T-RISE"=w3865:cluster{"T-RISE (L)":dbl, "T-RISE (N)":dbl}, "Result Out"=w3867:bool, "file error"=w3870:errorcluster)  [unwired: 10 in]
                    n2362 = local write "TEMP RISE LAB05-2"(w3865) -> ()
                    n2363 = local write "FAIL LAB05-2"(w3868) -> ()
                    n2364 = local write "DISP LAB05-2"(w3871) -> ()
                    n2365 = local write "RESULT LAB05-2"(w3867) -> ()
                    n2366 = local write "data file error"(w3870) -> ()
                  }
                }
              }
            }
          }
          frame #16 {
            # "run calibration routine"
            n2367 = local read "CALIBRATE"() -> (w3880:bool)
            n2368 = case shown="True" w3880 {
              frame False {
              }
              frame True {
                n2369 = stacked-sequence {
                  seq-local: [w3881 _ _] -> [_ w3883 _]
                  frame #0 {
                    n2370 = call "CALIBRATION PASSWORD"() -> ("PASSWORD"=w3881:string)  [unwired: 17 in, 2 out]
                  }
                  frame #1 {
                    n2371 = Equal?(x=w3883, y="7777") -> (x = y?=w3882:bool)
                    n2372 = case shown="True" w3882 {
                      frame False {
                      }
                      frame True {
                        n2373 = stacked-sequence {
                          frame #0 {
                            n2374 = call "sub vi - calibration v1.vi"() -> ()  [unwired: 12 in]
                          }
                          frame #1 {
                            n2375 = call "sub vi - get calibration values v1.vi"() -> ("LAB01 (CAL)"=w3889:T7, "LAB02 (CAL)"=w3888:T8, "LAB03 (CAL)"=w3887:T7, "LAB04 (CAL)"=w3886:T7, "calibration file error out"=w3890:errorcluster, "LAB05 (CAL)"=w3885:T7)  [unwired: 10 in]
                            n2376 = local write "calibration file error out"(w3890) -> ()
                            n2377 = local write "CAL LAB04"(w3886) -> ()
                            n2378 = local write "CAL LAB05"(w3885) -> ()
                            n2379 = local write "CAL LAB01"(w3889) -> ()
                            n2380 = local write "CAL LAB02"(w3888) -> ()
                            n2381 = local write "CAL LAB03"(w3887) -> ()
                          }
                        }
                      }
                    }
                  }
                  frame #2 {
                    n2382 = local write "CALIBRATE"(FALSE) -> ()
                  }
                }
              }
            }
          }
          frame #17 {
            # "save certain settings to file"
            n2383 = String To Path(string="c:\\crabtree\\Set Up\\") -> (path=w3893:path)
            n2384 = Build Path(base path=w3893, name or relative path="settings.bin") -> (appended path=w3895:path)
            n2385 = Build Path(base path=w3893, name or relative path="mail.bin") -> (appended path=w3892:path)
            n2386 = Create Folder(path (use dialog)=w3893) -> (error out=w3898:errorcluster)  [unwired: 2 in, 2 out]
            n2387 = call <vilib>:"Clear Errors.vi"("error in (no error)"=w3898) -> ()  [unwired: 6 in, 1 out]
            n2388 = stacked-sequence {
              seq-local: [w3900 _] -> [_ w3913]
              tunnel: w3895 -> [_ w3914]
              tunnel: w3892 -> [_ w3912]
              frame #0 {
                n2389 = local read "C drive data root dir"() -> (w3899:path)
                n2390 = local read "Network Directory"() -> (w3905:path)
                n2391 = local read "SET LAB05-2"() -> (w3904:T5)
                n2392 = local read "SET LAB05-1"() -> (w3903:T5)
                n2393 = local read "SET LAB04-2"() -> (w3902:T5)
                n2394 = local read "SET LAB03-2"() -> (w3906:T5)
                n2395 = local read "SET LAB04-1"() -> (w3901:T5)
                n2396 = local read "SET LAB03-1"() -> (w3907:T5)
                n2397 = local read "SET LAB02-2"() -> (w3908:T5)
                n2398 = local read "SET LAB02-1"() -> (w3909:T5)
                n2399 = local read "SET LAB01-2"() -> (w3910:T5)
                n2400 = local read "SET LAB01-1"() -> (w3911:T5)
                n2401 = Bundle("SET LAB01-1"=w3911, "SET LAB01-2"=w3910, "SET LAB02-1"=w3909, "SET LAB02-2"=w3908, "SET LAB03-1"=w3907, "SET LAB03-2"=w3906, "SET LAB04-1"=w3901, "SET LAB04-2"=w3902, "SET LAB05-1"=w3903, "SET LAB05-2"=w3904, "Network Directory"=w3905, "C drive data root dir"=w3899) -> (w3900:T19)  [unwired: 1 in]
              }
              frame #1 {
                n2402 = event shown="[1] \"SET LAB01-1\", \"SET LAB01-2\", \"SET LAB02-1\", \"SET LAB02-2\", \"SET LAB03-1\", \"SET LAB03-2\", \"SET LAB04-1\", \"SET LAB04-2\", \"SET LAB05-1\", \"SET LAB05-2\", \"Network Directory\", \"C drive data root dir\": Value Change" {
                  selector: _ -> [_ _ _]
                  dyn-events: _ -> [_ _ _]
                  timeout: 10.0 -> [_ _ _]
                  tunnel: w3914 -> [_ w3916 _]
                  tunnel: w3913 -> [_ w3917 _]
                  tunnel: w3912 -> [_ _ w3928]
                  event Timeout {
                    n2403 = event-data() -> ()  [unwired: 1 in, 3 out]
                  }
                  event "SET LAB01-1", "SET LAB01-2", "SET LAB02-1", "SET LAB02-2", "SET LAB03-1", "SET LAB03-2", "SET LAB04-1", "SET LAB04-2", "SET LAB05-1", "SET LAB05-2", "Network Directory", "C drive data root dir": Value Change {
                    n2404 = event-data() -> ()  [unwired: 1 in, 6 out]
                    n2405 = Open/Create/Replace File(file path (use dialog)=w3916, operation (0:open)=T18."replace or create") -> (refnum out=w3922:refnum<file>, error out=w3921:errorcluster)  [unwired: 4 in, 1 out]
                    n2406 = Write to Binary File(file (use dialog)=w3922, data=w3917, error in=w3921) -> (refnum out=w3920:refnum<file>, error out=w3919:errorcluster)  [unwired: 3 in, 1 out]
                    n2407 = Close File(refnum=w3920, error in=w3919) -> (error out=w3918:errorcluster)  [unwired: 1 out]
                    n2408 = local write "data file error"(w3918) -> ()
                  }
                  event "MAIL SETTINGS.OUT SERVER ADDRESS", "MAIL SETTINGS.FROM ACCOUNT", "MAIL SETTINGS.USER NAME", "MAIL SETTINGS.PASSWORD", "Auto Mail Send", "TO (string):": Value Change {
                    n2409 = event-data() -> ()  [unwired: 1 in, 6 out]
                    n2410 = local read "MAIL SETTINGS"() -> (w3927:T6)
                    n2411 = local read "Auto Mail Send"() -> (w3925:bool)
                    n2412 = local read "TO (string):"() -> (w3924:string)
                    n2413 = Open/Create/Replace File(file path (use dialog)=w3928, operation (0:open)=T18."replace or create") -> (refnum out=w3933:refnum<file>, error out=w3932:errorcluster)  [unwired: 4 in, 1 out]
                    n2414 = Bundle("MAIL SETTINGS"=w3927, "Auto Mail Send"=w3925, "TO (string):"=w3924) -> (w3926:T38)  [unwired: 1 in]
                    n2415 = Write to Binary File(file (use dialog)=w3933, data=w3926, error in=w3932) -> (refnum out=w3931:refnum<file>, error out=w3930:errorcluster)  [unwired: 3 in, 1 out]
                    n2416 = Close File(refnum=w3931, error in=w3930) -> (error out=w3929:errorcluster)  [unwired: 1 out]
                    n2417 = local write "data file error"(w3929) -> ()
                  }
                }
              }
            }
          }
          frame #18 {
            # "mail control"
            n2418 = local read "MAIL SETTINGS"() -> (w3950:T6)
            n2419 = local read "Auto Mail Send"() -> (w3936:bool)
            n2420 = Unbundle(w3950) -> ("OUT SERVER ADDRESS"=w3949:string, "FROM ACCOUNT"=w3948:string, "TEST MAIL"=w3947:bool)  [unwired: 4 out]
            n2421 = stacked-sequence {
              tunnel: "TO (string):" -> [_ w3989]
              tunnel: w3950 -> [w3955 w3988]
              tunnel: w3949 -> [w3954 w3987]
              tunnel: w3948 -> [w3953 w3986]
              tunnel: w3947 -> [w3952 _]
              tunnel: w3936 -> [_ w3985]
              tunnel: w3946 -> [_ w3984]
              tunnel: w3945 -> [_ w3983]
              tunnel: w3944 -> [_ w3982]
              tunnel: w3943 -> [_ w3981]
              tunnel: w3942 -> [_ w3980]
              tunnel: w3941 -> [_ w3979]
              tunnel: w3940 -> [_ w3978]
              tunnel: w3939 -> [_ w3977]
              tunnel: w3938 -> [_ w3976]
              tunnel: w3937 -> [_ w3975]
              tunnel: "TO (string):" -> [w3951 _]
              frame #0 {
                # "mail test"
                n2422 = case shown="True" w3952 {
                  tunnel: w3955 -> [_ w3959]
                  tunnel: w3951 -> [_ w3958]
                  tunnel: w3954 -> [_ w3957]
                  tunnel: w3953 -> [_ w3956]
                  frame False {
                  }
                  frame True {
                    n2423 = stacked-sequence {
                      seq-local: [_ _ w3969 _] -> [_ _ _ w3970]
                      tunnel: w3959 -> [w3962 _ _ w3974]
                      tunnel: w3958 -> [_ _ w3967 _]
                      tunnel: w3957 -> [_ _ w3965 _]
                      tunnel: w3956 -> [_ _ w3966 _]
                      frame #0 {
                        n2424 = Bundle(cluster=w3962, "TEST MAIL STATUS"="TEST START") -> (w3960:T6)  [unwired: 6 in]
                        n2425 = local write "MAIL SETTINGS"(w3960) -> ()
                      }
                      frame #1 {
                        n2426 = Wait (ms)(milliseconds to wait=500) -> ()  [unwired: 1 out]
                      }
                      frame #2 {
                        n2427 = call "sub vi - send mail with attach v5.vi"("TO:"=w3967, "subject"="MAIL TEST FROM LAB PANEL", "from"=w3966, "out going server"=w3965, "message"="TEST MESSAGE") -> ("error out"=w3969:errorcluster)  [unwired: 10 in]
                      }
                      frame #3 {
                        n2428 = Bundle(cluster=w3974, "TEST MAIL"=FALSE, "TEST MAIL STATUS"="TEST END", "mail error"=w3970) -> (w3972:T6)  [unwired: 4 in]
                        n2429 = local write "MAIL SETTINGS"(w3972) -> ()
                      }
                    }
                  }
                }
              }
              frame #1 {
                # "mail report"
                n2430 = stacked-sequence {
                  seq-local: [_ w4054 _ _] -> [_ _ _ w4222]
                  seq-local: [_ _ w4135 _] -> [_ _ _ w4212]
                  seq-local: [w3999 _ _ _] -> [_ w4048 _ _]
                  seq-local: [w3998 _ _ _] -> [_ w4047 _ _]
                  seq-local: [w3996 _ _ _] -> [_ w4045 _ _]
                  seq-local: [w3997 _ _ _] -> [_ w4046 _ _]
                  seq-local: [w3995 _ _ _] -> [_ w4044 _ _]
                  seq-local: [w3994 _ _ _] -> [_ w4039 _ _]
                  seq-local: [w3993 _ _ _] -> [_ w4040 _ _]
                  seq-local: [w3992 _ _ _] -> [_ w4041 _ _]
                  seq-local: [w3991 _ _ _] -> [_ w4042 _ _]
                  seq-local: [w3990 _ _ _] -> [_ w4043 _ _]
                  tunnel: w3989 -> [_ _ _ w4223]
                  tunnel: w3988 -> [_ _ _ w4206]
                  tunnel: w3987 -> [_ _ _ w4220]
                  tunnel: w3986 -> [_ _ _ w4219]
                  tunnel: w3985 -> [w4030 _ _ w4214]
                  tunnel: w3984 -> [_ _ w4165 _]
                  tunnel: w3983 -> [_ _ w4162 _]
                  tunnel: w3982 -> [_ _ w4161 _]
                  tunnel: w3981 -> [_ _ w4160 _]
                  tunnel: w3980 -> [_ _ w4159 _]
                  tunnel: w3979 -> [_ _ w4158 _]
                  tunnel: w3978 -> [_ _ w4157 _]
                  tunnel: w3977 -> [_ _ w4156 _]
                  tunnel: w3976 -> [_ _ w4155 _]
                  tunnel: w3975 -> [_ _ w4154 _]
                  frame #0 {
                    n2431 = case shown="False" w4030 {
                      frame False {
                        n2432 = local write "mail control"("") -> ()
                      }
                      frame True {
                      }
                    }
                    n2433 = local read "SET LAB01-1"() -> (w4029:T5)
                    n2434 = local read "SET LAB01-2"() -> (w4028:T5)
                    n2435 = local read "SET LAB02-1"() -> (w4027:T5)
                    n2436 = local read "SET LAB02-2"() -> (w4026:T5)
                    n2437 = local read "SET LAB03-1"() -> (w4025:T5)
                    n2438 = local read "SET LAB04-1"() -> (w4023:T5)
                    n2439 = local read "SET LAB05-1"() -> (w4021:T5)
                    n2440 = local read "SET LAB03-2"() -> (w4024:T5)
                    n2441 = local read "SET LAB04-2"() -> (w4022:T5)
                    n2442 = local read "SET LAB05-2"() -> (w4020:T5)
                    n2443 = Unbundle(w4025) -> ("DESCRIPTION"=w4005:string)  [unwired: 4 out]
                    n2444 = Unbundle(w4024) -> ("DESCRIPTION"=w4004:string)  [unwired: 4 out]
                    n2445 = Unbundle(w4023) -> ("DESCRIPTION"=w4003:string)  [unwired: 4 out]
                    n2446 = Unbundle(w4020) -> ("DESCRIPTION"=w4000:string)  [unwired: 4 out]
                    n2447 = Unbundle(w4026) -> ("DESCRIPTION"=w4006:string)  [unwired: 4 out]
                    n2448 = Unbundle(w4022) -> ("DESCRIPTION"=w4002:string)  [unwired: 4 out]
                    n2449 = Unbundle(w4029) -> ("DESCRIPTION"=w4018:string)  [unwired: 4 out]
                    n2450 = Unbundle(w4027) -> ("DESCRIPTION"=w4007:string)  [unwired: 4 out]
                    n2451 = Unbundle(w4021) -> ("DESCRIPTION"=w4001:string)  [unwired: 4 out]
                    n2452 = Unbundle(w4028) -> ("DESCRIPTION"=w4008:string)  [unwired: 4 out]
                    n2453 = Concatenate Strings("[LAB05-1/", w4000) -> (w3990:string)
                    n2454 = Concatenate Strings("[LAB05-2/", w4001) -> (w3991:string)
                    n2455 = Concatenate Strings("[LAB04-2/", w4002) -> (w3992:string)
                    n2456 = Concatenate Strings("[LAB03-2/", w4004) -> (w3994:string)
                    n2457 = Concatenate Strings("[LAB04-1/", w4003) -> (w3993:string)
                    n2458 = Concatenate Strings("[LAB03-1/", w4005) -> (w3995:string)
                    n2459 = Concatenate Strings("[LAB01-2/", w4008) -> (w3998:string)
                    n2460 = Concatenate Strings("[LAB02-2/", w4006) -> (w3996:string)
                    n2461 = Concatenate Strings("[LAB01-1/", w4018) -> (w3999:string)
                    n2462 = Concatenate Strings("[LAB02-1/", w4007) -> (w3997:string)
                  }
                  frame #1 {
                    w4052 = "/"
                    w4053 = 2.0
                    n2463 = local read "DISP LAB01-2"() -> (w4133:T4)
                    n2464 = local read "DISP LAB01-1"() -> (w4134:T4)
                    n2465 = local read "DISP LAB02-1"() -> (w4132:T4)
                    n2466 = local read "DISP LAB03-2"() -> (w4129:T4)
                    n2467 = local read "DISP LAB02-2"() -> (w4131:T4)
                    n2468 = local read "DISP LAB03-1"() -> (w4130:T4)
                    n2469 = local read "DISP LAB04-2"() -> (w4127:T4)
                    n2470 = local read "DISP LAB04-1"() -> (w4128:T4)
                    n2471 = local read "DISP LAB05-1"() -> (w4126:T4)
                    n2472 = local read "DISP LAB05-2"() -> (w4125:T4)
                    n2473 = Unbundle(w4133) -> ("CYCLE"=w4117:dbl, "MINS"=w4116:dbl, "STATUS"=w4113:string)
                    n2474 = Unbundle(w4134) -> ("CYCLE"=w4122:dbl, "MINS"=w4121:dbl, "STATUS"=w4118:string)
                    n2475 = Unbundle(w4132) -> ("CYCLE"=w4110:dbl, "MINS"=w4109:dbl, "STATUS"=w4108:string)
                    n2476 = Unbundle(w4129) -> ("CYCLE"=w4097:dbl, "MINS"=w4096:dbl, "STATUS"=w4093:string)
                    n2477 = Unbundle(w4130) -> ("CYCLE"=w4102:dbl, "MINS"=w4101:dbl, "STATUS"=w4098:string)
                    n2478 = Unbundle(w4131) -> ("CYCLE"=w4107:dbl, "MINS"=w4106:dbl, "STATUS"=w4103:string)
                    n2479 = Unbundle(w4128) -> ("CYCLE"=w4092:dbl, "MINS"=w4091:dbl, "STATUS"=w4088:string)
                    n2480 = Unbundle(w4127) -> ("CYCLE"=w4087:dbl, "MINS"=w4086:dbl, "STATUS"=w4083:string)
                    n2481 = Unbundle(w4126) -> ("CYCLE"=w4082:dbl, "MINS"=w4081:dbl, "STATUS"=w4078:string)
                    n2482 = Unbundle(w4125) -> ("CYCLE"=w4124:dbl, "MINS"=w4123:dbl, "STATUS"=w4075:string)
                    n2483 = Number To Decimal String(number=w4110) -> (decimal integer string=w4112:string)  [unwired: 1 in]
                    n2484 = Number To Decimal String(number=w4107) -> (decimal integer string=w4105:string)  [unwired: 1 in]
                    n2485 = Number To Decimal String(number=w4102) -> (decimal integer string=w4100:string)  [unwired: 1 in]
                    n2486 = Number To Decimal String(number=w4117) -> (decimal integer string=w4115:string)  [unwired: 1 in]
                    n2487 = Number To Decimal String(number=w4097) -> (decimal integer string=w4095:string)  [unwired: 1 in]
                    n2488 = Number To Decimal String(number=w4122) -> (decimal integer string=w4120:string)  [unwired: 1 in]
                    n2489 = Number To Decimal String(number=w4124) -> (decimal integer string=w4077:string)  [unwired: 1 in]
                    n2490 = Number To Decimal String(number=w4092) -> (decimal integer string=w4090:string)  [unwired: 1 in]
                    n2491 = Number To Decimal String(number=w4087) -> (decimal integer string=w4085:string)  [unwired: 1 in]
                    n2492 = Number To Decimal String(number=w4082) -> (decimal integer string=w4080:string)  [unwired: 1 in]
                    n2493 = Number To Fractional String(number=w4109, precision (6)=w4053) -> (F-format string=w4111:string)  [unwired: 2 in]
                    n2494 = Number To Fractional String(number=w4096, precision (6)=w4053) -> (F-format string=w4094:string)  [unwired: 2 in]
                    n2495 = Number To Fractional String(number=w4106, precision (6)=w4053) -> (F-format string=w4104:string)  [unwired: 2 in]
                    n2496 = Number To Fractional String(number=w4101, precision (6)=w4053) -> (F-format string=w4099:string)  [unwired: 2 in]
                    n2497 = Number To Fractional String(number=w4086, precision (6)=w4053) -> (F-format string=w4084:string)  [unwired: 2 in]
                    n2498 = Number To Fractional String(number=w4091, precision (6)=w4053) -> (F-format string=w4089:string)  [unwired: 2 in]
                    n2499 = Number To Fractional String(number=w4116, precision (6)=w4053) -> (F-format string=w4114:string)  [unwired: 2 in]
                    n2500 = Number To Fractional String(number=w4081, precision (6)=w4053) -> (F-format string=w4079:string)  [unwired: 2 in]
                    n2501 = Number To Fractional String(number=w4121, precision (6)=w4053) -> (F-format string=w4119:string)  [unwired: 2 in]
                    n2502 = Number To Fractional String(number=w4123, precision (6)=w4053) -> (F-format string=w4076:string)  [unwired: 2 in]
                    n2503 = Concatenate Strings(w4052, w4095, w4052, w4094, w4052, w4093) -> (w4069:string)
                    n2504 = Concatenate Strings(w4052, w4090, w4052, w4089, w4052, w4088) -> (w4068:string)
                    n2505 = Concatenate Strings(w4052, w4085, w4052, w4084, w4052, w4083) -> (w4067:string)
                    n2506 = Concatenate Strings(w4052, w4080, w4052, w4079, w4052, w4078) -> (w4066:string)
                    n2507 = Concatenate Strings(w4052, w4077, w4052, w4076, w4052, w4075) -> (w4065:string)
                    n2508 = Concatenate Strings(w4052, w4120, w4052, w4119, w4052, w4118) -> (w4074:string)
                    n2509 = Concatenate Strings(w4052, w4100, w4052, w4099, w4052, w4098) -> (w4070:string)
                    n2510 = Concatenate Strings(w4052, w4115, w4052, w4114, w4052, w4113) -> (w4073:string)
                    n2511 = Concatenate Strings(w4052, w4112, w4052, w4111, w4052, w4108) -> (w4072:string)
                    n2512 = Concatenate Strings(w4052, w4105, w4052, w4104, w4052, w4103) -> (w4071:string)
                    n2513 = Concatenate Strings("]", "\r") -> (w4049:string)
                    n2514 = Concatenate Strings(w4044, w4070, w4049) -> (w4060:string)
                    n2515 = Concatenate Strings(w4046, w4072, w4049) -> (w4062:string)
                    n2516 = Concatenate Strings(w4045, w4071, w4049) -> (w4061:string)
                    n2517 = Concatenate Strings(w4041, w4067, w4049) -> (w4057:string)
                    n2518 = Concatenate Strings(w4042, w4066, w4049) -> (w4058:string)
                    n2519 = Concatenate Strings(w4040, w4068, w4049) -> (w4056:string)
                    n2520 = Concatenate Strings(w4039, w4069, w4049) -> (w4055:string)
                    n2521 = Concatenate Strings(w4043, w4065, w4049) -> (w4059:string)
                    n2522 = Concatenate Strings(w4047, w4073, w4049) -> (w4063:string)
                    n2523 = Concatenate Strings(w4048, w4074, w4049) -> (w4064:string)
                    n2524 = Concatenate Strings(w4064, w4063, w4062, w4061, w4060, w4055, w4056, w4057, w4058, w4059) -> (w4032:string)
                    n2525 = Concatenate Strings("[PANEL/", "DESC/", "CYCLES/", "MINS/", "STATUS]", "\r", w4032) -> (w4054:string)
                    "MAIL REPORT" <- w4054
                  }
                  frame #2 {
                    w4163 = "END"
                    n2526 = local read "mail control"() -> (w4164:string)
                    n2527 = case shown="False" w4159 {
                      tunnel: w4164 -> [w4188 _]
                      tunnel: w4163 -> [w4187 _]
                      tunnel: [w4186 FALSE] -> w4149
                      frame False {
                        n2528 = Equal?(x=w4188, y=w4187) -> (x = y?=w4186:bool)
                      }
                      frame True {
                      }
                    }
                    n2529 = case shown="False" w4165 {
                      tunnel: w4164 -> [w4204 _]
                      tunnel: w4163 -> [w4203 _]
                      tunnel: [w4202 FALSE] -> w4153
                      frame False {
                        n2530 = Equal?(x=w4204, y=w4203) -> (x = y?=w4202:bool)
                      }
                      frame True {
                      }
                    }
                    n2531 = case shown="False" w4162 {
                      tunnel: w4164 -> [w4200 _]
                      tunnel: w4163 -> [w4199 _]
                      tunnel: [w4198 FALSE] -> w4152
                      frame False {
                        n2532 = Equal?(x=w4200, y=w4199) -> (x = y?=w4198:bool)
                      }
                      frame True {
                      }
                    }
                    n2533 = case shown="False" w4160 {
                      tunnel: w4164 -> [w4192 _]
                      tunnel: w4163 -> [w4191 _]
                      tunnel: [w4190 FALSE] -> w4150
                      frame False {
                        n2534 = Equal?(x=w4192, y=w4191) -> (x = y?=w4190:bool)
                      }
                      frame True {
                      }
                    }
                    n2535 = case shown="False" w4161 {
                      tunnel: w4164 -> [w4196 _]
                      tunnel: w4163 -> [w4195 _]
                      tunnel: [w4194 FALSE] -> w4151
                      frame False {
                        n2536 = Equal?(x=w4196, y=w4195) -> (x = y?=w4194:bool)
                      }
                      frame True {
                      }
                    }
                    n2537 = Or(x=w4151, y=w4150) -> (x .or. y?=w4142:bool)
                    n2538 = Or(x=w4153, y=w4152) -> (x .or. y?=w4143:bool)
                    n2539 = Or(x=w4143, y=w4142) -> (x .or. y?=w4138:bool)
                    n2540 = case shown="False" w4155 {
                      tunnel: w4164 -> [w4172 _]
                      tunnel: w4163 -> [w4171 _]
                      tunnel: [w4170 FALSE] -> w4144
                      frame False {
                        n2541 = Equal?(x=w4172, y=w4171) -> (x = y?=w4170:bool)
                      }
                      frame True {
                      }
                    }
                    n2542 = case shown="False" w4154 {
                      tunnel: w4164 -> [w4168 _]
                      tunnel: w4163 -> [w4167 _]
                      tunnel: [w4166 FALSE] -> w4148
                      frame False {
                        n2543 = Equal?(x=w4168, y=w4167) -> (x = y?=w4166:bool)
                      }
                      frame True {
                      }
                    }
                    n2544 = case shown="False" w4156 {
                      tunnel: w4164 -> [w4176 _]
                      tunnel: w4163 -> [w4175 _]
                      tunnel: [w4174 FALSE] -> w4145
                      frame False {
                        n2545 = Equal?(x=w4176, y=w4175) -> (x = y?=w4174:bool)
                      }
                      frame True {
                      }
                    }
                    n2546 = case shown="False" w4158 {
                      tunnel: w4164 -> [w4184 _]
                      tunnel: w4163 -> [w4183 _]
                      tunnel: [w4182 FALSE] -> w4147
                      frame False {
                        n2547 = Equal?(x=w4184, y=w4183) -> (x = y?=w4182:bool)
                      }
                      frame True {
                      }
                    }
                    n2548 = case shown="False" w4157 {
                      tunnel: w4164 -> [w4180 _]
                      tunnel: w4163 -> [w4179 _]
                      tunnel: [w4178 FALSE] -> w4146
                      frame False {
                        n2549 = Equal?(x=w4180, y=w4179) -> (x = y?=w4178:bool)
                      }
                      frame True {
                      }
                    }
                    n2550 = Or(x=w4147, y=w4146) -> (x .or. y?=w4141:bool)
                    n2551 = Or(x=w4145, y=w4144) -> (x .or. y?=w4140:bool)
                    n2552 = Or(x=w4148, y=w4149) -> (x .or. y?=w4136:bool)
                    n2553 = Or(x=w4141, y=w4140) -> (x .or. y?=w4139:bool)
                    n2554 = Or(x=w4138, y=w4139) -> (x .or. y?=w4137:bool)
                    n2555 = Or(x=w4137, y=w4136) -> (x .or. y?=w4135:bool)
                  }
                  frame #3 {
                    n2556 = local read "on loops"() -> (w4218:dbl)
                    n2557 = local read "jig cycle"() -> (w4215:dbl)
                    n2558 = local read "Send Mail Now"() -> (w4209:bool)
                    n2559 = Add(x=w4218, y=3.0) -> (x+y=w4216:dbl)
                    n2560 = Equal?(x=w4215, y=w4216) -> (x = y?=w4210:bool)
                    n2561 = And(x=w4210, y=w4209) -> (x .and. y?=w4208:bool)
                    n2562 = And(x=w4214, y=w4210) -> (x .and. y?=w4213:bool)
                    n2563 = And(x=w4213, y=w4212) -> (x .and. y?=w4211:bool)
                    n2564 = Or(x=w4211, y=w4208) -> (x .or. y?=w4207:bool)
                    n2565 = case shown="True" w4207 {
                      tunnel: w4223 -> [_ w4229]
                      tunnel: w4222 -> [_ w4228]
                      tunnel: "Lab Panel Test Status" -> [_ w4227]
                      tunnel: w4220 -> [_ w4226]
                      tunnel: w4219 -> [_ w4225]
                      tunnel: w4206 -> [_ w4224]
                      frame False {
                      }
                      frame True {
                        n2566 = stacked-sequence {
                          tunnel: w4229 -> [w4237 _]
                          tunnel: w4228 -> [w4236 _]
                          tunnel: w4227 -> [w4235 _]
                          tunnel: w4226 -> [w4234 _]
                          tunnel: w4225 -> [w4233 _]
                          tunnel: w4224 -> [w4232 _]
                          frame #0 {
                            n2567 = call "sub vi - send mail with attach v5.vi"("TO:"=w4237, "subject"=w4235, "from"=w4233, "out going server"=w4234, "message"=w4236) -> ("error out"=w4231:errorcluster)  [unwired: 10 in]
                            n2568 = Bundle(cluster=w4232, "mail error"=w4231) -> (w4230:T6)  [unwired: 6 in]
                            n2569 = local write "MAIL SETTINGS"(w4230) -> ()
                          }
                          frame #1 {
                            n2570 = local write "mail control"("") -> ()
                            n2571 = local write "Send Mail Now"(FALSE) -> ()
                          }
                        }
                      }
                    }
                  }
                }
              }
            }
          }
        }
        n2572 = node-c288() -> ()  [unwired: 1 in, 1 out]
        "loops" <- w161
        "stop2" <- "stop"
      }
      n2573 = node-c288(w138) -> ()  [unwired: 1 out]
    }
  }
